vi "Lab Panel V4.3.vi"() -> ()   [LabVIEW 2013]
uses:
  <vilib>/Platform/TimedLoop/XDataNode/timing_clust.ctl
  <vilib>/Platform/TimedLoop/XDataNode/nitl_modes.ctl
  <vilib>/Platform/TimedLoop/XDataNode/wakeup.ctl
  Global 1.vi
  <vilib>/platform/TimedLoop/XDataNode/XDataNode.xnode
  <vilib>/Platform/TimedLoop/XDataNode/XDNodeRunTimeDep.lvlib
panel:
  out "TEMP update":bool
  out "AI update":bool
  in  "stop":bool
  in  "Tab Control 2":T1(tab)
  out "SIG LAB05-2":T2 {"PF" format="%.2f"; "AMPS" format="%.1f"}
  out "SIG LAB05-1":T2 {"PF" format="%.2f"; "AMPS" format="%.1f"}
  out "SIG LAB04-2":T2 {"PF" format="%.2f"; "AMPS" format="%.1f"}
  out "SIG LAB04-1":T2 {"PF" format="%.2f"; "AMPS" format="%.1f"}
  out "SIG LAB03-2":T2 {"PF" format="%.2f"; "AMPS" format="%.1f"}
  out "SIG LAB03-1":T2 {"PF" format="%.2f"; "AMPS" format="%.1f"}
  out "SIG LAB02-2":T2 {"PF" format="%.2f"; "AMPS" format="%.1f"}
  in  "RUN LAB01-1":bool
  in  "O/I  LAB05-1":bool
  in  "O/I  LAB05-2":bool
  in  "O/I  LAB04-1":bool
  in  "O/I  LAB04-2":bool
  in  "O/I  LAB02-1":bool
  in  "O/I  LAB02-2":bool
  in  "O/I  LAB01-2":bool
  in  "O/I  LAB01-1":bool
  in  "O/I  LAB03-1":bool
  in  "RUN LAB05-2":bool
  in  "RUN LAB05-1":bool
  in  "RUN LAB04-2":bool
  in  "RUN LAB04-1":bool
  in  "RUN LAB03-2":bool
  in  "RUN LAB03-1":bool
  in  "RUN LAB02-2":bool
  in  "RUN LAB02-1":bool
  in  "RUN LAB01-2":bool
  in  "SELECT LAB05-2":T3(radio)
  in  "SELECT LAB05-1":T3(radio)
  in  "SELECT LAB04-2":T3(radio)
  in  "SELECT LAB04-1":T3(radio)
  in  "SELECT LAB03-2":T3(radio)
  in  "SELECT LAB03-1":T3(radio)
  in  "SELECT LAB02-2":T3(radio)
  in  "SELECT LAB02-1":T3(radio)
  in  "SELECT LAB01-2":T3(radio)
  in  "SELECT LAB01-1":T3(radio)
  in  "O/I  LAB03-2":bool
  out "SIG LAB01-1":T2 {"PF" format="%.2f"; "AMPS" format="%.1f"}
  out "SIG LAB01-2":T2 {"PF" format="%.2f"; "AMPS" format="%.1f"}
  out "SIG LAB02-1":T2 {"PF" format="%.2f"; "AMPS" format="%.1f"}
  out "DISP LAB05-2":T4 {"MINS" format="%.2g"}
  out "DISP LAB05-1":T4 {"MINS" format="%.2g"}
  out "DISP LAB04-2":T4 {"MINS" format="%.2g"}
  out "DISP LAB04-1":T4 {"MINS" format="%.2g"}
  out "DISP LAB03-2":T4 {"MINS" format="%.2g"}
  out "DISP LAB03-1":T4 {"MINS" format="%.2g"}
  in  "SET LAB05-2":T5={"NAME"="", "DESCRIPTION"="", "CYCLES"=5.0, "T-RISE mins"=0.0, "T-RISE deg C"=0.0} {"CYCLES" min=5.0 step=1.0}
  in  "SET LAB05-1":T5={"NAME"="", "DESCRIPTION"="", "CYCLES"=5.0, "T-RISE mins"=0.0, "T-RISE deg C"=0.0} {"CYCLES" min=5.0 step=1.0}
  in  "SET LAB04-2":T5={"NAME"="", "DESCRIPTION"="", "CYCLES"=5.0, "T-RISE mins"=0.0, "T-RISE deg C"=0.0} {"CYCLES" min=5.0 step=1.0}
  in  "SET LAB04-1":T5={"NAME"="", "DESCRIPTION"="", "CYCLES"=5.0, "T-RISE mins"=0.0, "T-RISE deg C"=0.0} {"CYCLES" min=5.0 step=1.0}
  in  "SET LAB03-2":T5={"NAME"="", "DESCRIPTION"="", "CYCLES"=5.0, "T-RISE mins"=0.0, "T-RISE deg C"=0.0} {"CYCLES" min=5.0 step=1.0}
  in  "SET LAB03-1":T5={"NAME"="", "DESCRIPTION"="", "CYCLES"=5.0, "T-RISE mins"=0.0, "T-RISE deg C"=0.0} {"CYCLES" min=5.0 step=1.0}
  out "DISP LAB02-2":T4 {"MINS" format="%.2g"}
  out "DISP LAB02-1":T4 {"MINS" format="%.2g"}
  in  "SET LAB02-2":T5={"NAME"="", "DESCRIPTION"="", "CYCLES"=5.0, "T-RISE mins"=0.0, "T-RISE deg C"=0.0} {"CYCLES" min=5.0 step=1.0}
  in  "SET LAB02-1":T5={"NAME"="", "DESCRIPTION"="", "CYCLES"=5.0, "T-RISE mins"=0.0, "T-RISE deg C"=0.0} {"CYCLES" min=5.0 step=1.0}
  out "RESULT LAB05-2":bool
  out "RESULT LAB05-1":bool
  out "RESULT LAB04-2":bool
  out "RESULT LAB04-1":bool
  out "RESULT LAB03-2":bool
  out "RESULT LAB03-1":bool
  out "RESULT LAB02-2":bool
  out "RESULT LAB02-1":bool
  out "RESULT LAB01-2":bool
  out "RESULT LAB01-1":bool
  in  "SET LAB01-1":T5={"NAME"="", "DESCRIPTION"="", "CYCLES"=5.0, "T-RISE mins"=0.0, "T-RISE deg C"=0.0} {"CYCLES" min=5.0 step=1.0}
  in  "SET LAB01-2":T5={"NAME"="", "DESCRIPTION"="", "CYCLES"=5.0, "T-RISE mins"=0.0, "T-RISE deg C"=0.0} {"CYCLES" min=5.0 step=1.0}
  out "DISP LAB01-1":T4 {"MINS" format="%.2g"}
  out "DISP LAB01-2":T4 {"MINS" format="%.2f"}
  out "TEMP RISE LAB05-2":cluster{"TL":dbl, "TN":dbl}
  out "TEMP RISE LAB05-1":cluster{"TL":dbl, "TN":dbl}
  out "TEMP RISE LAB04-2":cluster{"TL":dbl, "TN":dbl}
  out "TEMP RISE LAB04-1":cluster{"TL":dbl, "TN":dbl}
  out "TEMP RISE LAB03-2":cluster{"TL":dbl, "TN":dbl}
  out "TEMP RISE LAB03-1":cluster{"TL":dbl, "TN":dbl}
  out "TEMP RISE LAB02-2":cluster{"TL":dbl, "TN":dbl}
  out "TEMP RISE LAB02-1":cluster{"TL":dbl, "TN":dbl}
  out "TEMP RISE LAB01-2":cluster{"TL":dbl, "TN":dbl}
  out "TEMP RISE LAB01-1":cluster{"TL":dbl, "TN":dbl}
  in  "JIG OFF TIME (S)":dbl=2.0 min=2.0 max=10.0 step=0.5 format="%.1g"
  in  "JIG ON TIME (S)":dbl=1.0 min=1.0 max=10.0 step=0.5 format="%.1g"
  out "JIG LAB05-2":bool
  out "JIG LAB05-1":bool
  out "JIG LAB04-2":bool
  out "JIG LAB04-1":bool
  out "JIG LAB03-2":bool
  out "JIG LAB03-1":bool
  out "JIG LAB02-2":bool
  out "JIG LAB02-1":bool
  out "JIG LAB01-2":bool
  out "JIG LAB01-1":bool
  out "TEMP START LAB01-1":cluster{"TL":dbl, "TN":dbl}
  out "TEMP START LAB02-1":cluster{"TL":dbl, "TN":dbl}
  out "TEMP START LAB03-1":cluster{"TL":dbl, "TN":dbl}
  out "TEMP START LAB04-1":cluster{"TL":dbl, "TN":dbl}
  out "TEMP START LAB01-2":cluster{"TL":dbl, "TN":dbl}
  out "TEMP START LAB02-2":cluster{"TL":dbl, "TN":dbl}
  out "TEMP START LAB03-2":cluster{"TL":dbl, "TN":dbl}
  out "TEMP START LAB04-2":cluster{"TL":dbl, "TN":dbl}
  out "TEMP START LAB05-2":cluster{"TL":dbl, "TN":dbl}
  out "TEMP START LAB05-1":cluster{"TL":dbl, "TN":dbl}
  in  "MAIL SETTINGS":T6
  out "MAIL REPORT":string
  in  "TO (string):":string
  in  "Send Mail Now":bool
  in  "Auto Mail Send":bool
  in  "Network Directory":path
  out "CAL LAB01":T7 {"2 (TN) cal" min=0.0 step=0.01 format="%.2f"; "2 (TL) cal" min=0.0 step=0.01 format="%.2f"; "2 (PF) cal" min=0.0 step=0.01 format="%.2f"; "2 (V) cal" min=0.0 step=0.01 format="%.2f"; "2 (A) cal" min=0.0 step=0.01 format="%.2f"; "1 (TN) cal" min=0.0 step=0.01 format="%.2f"; "1 (TL) cal" min=0.0 step=0.01 format="%.2f"; "1 (PF) cal" min=0.0 step=0.01 format="%.2f"; "1 (V) cal" min=0.0 step=0.01 format="%.2f"; "1  (A) cal" min=0.0 step=0.01 format="%.2f"}
  out "CAL LAB03":T7 {"2 (TN) cal" min=0.0 step=0.01 format="%.2f"; "2 (TL) cal" min=0.0 step=0.01 format="%.2f"; "2 (PF) cal" min=0.0 step=0.01 format="%.2f"; "2 (V) cal" min=0.0 step=0.01 format="%.2f"; "2 (A) cal" min=0.0 step=0.01 format="%.2f"; "1 (TN) cal" min=0.0 step=0.01 format="%.2f"; "1 (TL) cal" min=0.0 step=0.01 format="%.2f"; "1 (PF) cal" min=0.0 step=0.01 format="%.2f"; "1 (V) cal" min=0.0 step=0.01 format="%.2f"; "1  (A) cal" min=0.0 step=0.01 format="%.2f"}
  out "CAL LAB02":T8 {"2 (TN) cal" min=0.0 step=0.01 format="%.2f"; "2 (TL) cal" min=0.0 step=0.01 format="%.2f"; "2 (PF) cal" min=0.0 step=0.01 format="%.2f"; "2 (V) cal" min=0.0 step=0.01 format="%.2f"; "2 (A) cal" min=0.0 step=0.01 format="%.2f"; "1 (TN) cal" min=0.0 step=0.01 format="%.2f"; "1 (TL) cal" min=0.0 step=0.01 format="%.2f"; "1 (PF) cal" min=0.0 step=0.01 format="%.2f"; "1 (V) cal" min=0.0 step=0.01 format="%.2f"; "1 (A) cal" min=0.0 step=0.01 format="%.2f"}
  out "CAL LAB05":T7 {"2 (TN) cal" min=0.0 step=0.01 format="%.2f"; "2 (TL) cal" min=0.0 step=0.01 format="%.2f"; "2 (PF) cal" min=0.0 step=0.01 format="%.2f"; "2 (V) cal" min=0.0 step=0.01 format="%.2f"; "2 (A) cal" min=0.0 step=0.01 format="%.2f"; "1 (TN) cal" min=0.0 step=0.01 format="%.2f"; "1 (TL) cal" min=0.0 step=0.01 format="%.2f"; "1 (PF) cal" min=0.0 step=0.01 format="%.2f"; "1 (V) cal" min=0.0 step=0.01 format="%.2f"; "1  (A) cal" min=0.0 step=0.01 format="%.2f"}
  out "CAL LAB04":T7 {"2 (TN) cal" min=0.0 step=0.01 format="%.2f"; "2 (TL) cal" min=0.0 step=0.01 format="%.2f"; "2 (PF) cal" min=0.0 step=0.01 format="%.2f"; "2 (V) cal" min=0.0 step=0.01 format="%.2f"; "2 (A) cal" min=0.0 step=0.01 format="%.2f"; "1 (TN) cal" min=0.0 step=0.01 format="%.2f"; "1 (TL) cal" min=0.0 step=0.01 format="%.2f"; "1 (PF) cal" min=0.0 step=0.01 format="%.2f"; "1 (V) cal" min=0.0 step=0.01 format="%.2f"; "1  (A) cal" min=0.0 step=0.01 format="%.2f"}
  out "calibration file error out":errorcluster
  in  "CALIBRATE":bool
  in  "SHOW ADMIN PAGE":bool
  out "ON L05-2":cluster{"amps":dbl, "volts":dbl, "pf":dbl}
  out "ON L05-1":cluster{"amps":dbl, "volts":dbl, "pf":dbl}
  out "FAIL LAB05-2":cluster{"LO":dbl, "HI":dbl}
  out "FAIL LAB05-1":cluster{"LO":dbl, "HI":dbl}
  out "FAIL LAB04-2":cluster{"LO":dbl, "HI":dbl}
  out "FAIL LAB04-1":cluster{"LO":dbl, "HI":dbl}
  out "FAIL LAB03-2":cluster{"LO":dbl, "HI":dbl}
  out "FAIL LAB03-1":cluster{"LO":dbl, "HI":dbl}
  out "FAIL LAB02-2":cluster{"LO":dbl, "HI":dbl}
  out "FAIL LAB02-1":cluster{"LO":dbl, "HI":dbl}
  out "FAIL LAB01-2":cluster{"LO":dbl, "HI":dbl}
  out "FAIL LAB01-1":cluster{"LO":dbl, "HI":dbl}
  out "ON L01-1":cluster{"amps":dbl, "volts":dbl, "pf":dbl}
  out "ON L01-2":cluster{"amps":dbl, "volts":dbl, "pf":dbl}
  out "ON L02-1":cluster{"amps":dbl, "volts":dbl, "pf":dbl}
  out "ON L02-2":cluster{"amps":dbl, "volts":dbl, "pf":dbl}
  out "ON L03-1":cluster{"amps":dbl, "volts":dbl, "pf":dbl}
  out "ON L03-2":cluster{"amps":dbl, "volts":dbl, "pf":dbl}
  out "ON L04-1":cluster{"amps":dbl, "volts":dbl, "pf":dbl}
  out "ON L04-2":cluster{"amps":dbl, "volts":dbl, "pf":dbl}
  in  "JIG TEST":T9
  in  "C drive data root dir":path
  out "run lab05-2":bool
  out "run lab05-1":bool
  out "run lab04-2":bool
  out "run lab04-1":bool
  out "run lab03-2":bool
  out "run lab03-1":bool
  out "run lab02-2":bool
  out "run lab02-1":bool
  out "run lab01-2":bool
  out "run lab01-1":bool
  out "stop2":bool
  in  "Tab Control":T10(tab)
  out "LAB01-2 (GRAPH)":dynamicdata(graph)
  out "LAB01-1 (GRAPH)":dynamicdata(graph)
  out "LAB02-2 (GRAPH)":dynamicdata(graph)
  out "LAB02-1 (GRAPH)":dynamicdata(graph)
  out "LAB03-2 (GRAPH)":dynamicdata(graph)
  out "LAB03-1 (GRAPH)":dynamicdata(graph)
  out "LAB04-2 (GRAPH)":dynamicdata(graph)
  out "LAB04-1 (GRAPH)":dynamicdata(graph)
  out "LAB05-2 (GRAPH)":dynamicdata(graph)
  out "LAB05-1 (GRAPH)":dynamicdata(graph)
  out "LAB05 TEMP":T11
  out "LAB04 TEMP":T11
  out "LAB02 TEMP":T11
  out "LAB01 TEMP":T11
  out "LAB03 TEMP":T11
  out "Analog Error Array":errorcluster[](array[cluster])
  out "AI loop time":dbl format="%.6g"
  out "loops":dbl
  in  "loop  delay(mS)":dbl
  out "on loops":dbl
  out "off loops":dbl
  out "jig cycle":dbl
  out "TDMS LAB01-1":refnum<k34>
  out "data file error":errorcluster
  out "TDMS LAB02-1":refnum<k34>
  out "TDMS LAB01-2":refnum<k34>
  out "TDMS LAB02-2":refnum<k34>
  out "TDMS LAB03-1":refnum<k34>
  out "TDMS LAB03-2":refnum<k34>
  out "TDMS LAB04-1":refnum<k34>
  out "TDMS LAB04-2":refnum<k34>
  out "TDMS LAB05-1":refnum<k34>
  out "TDMS LAB05-2":refnum<k34>
  out "mail control":string
  # "LAB01"
  # "LAB02"
  # "LAB05"
  # "LAB03"
  # "LAB04"
  # "LAB01"
  # "LAB02"
  # "LAB03"
  # "LAB04"
  # "LAB05"
  # "JIG SET"
  # "(Enter recipients address seperated by comma)"
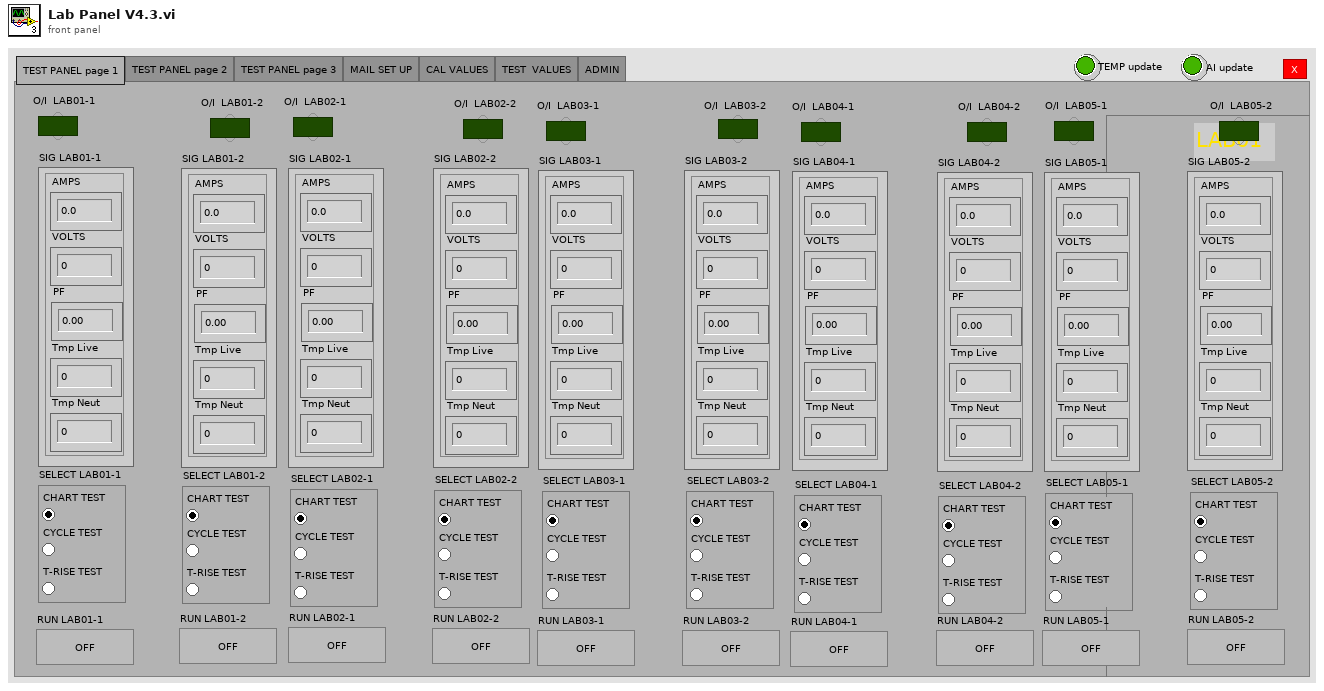
[diagram p1: front panel]
types:
  T1 = enum32{"TEST PANEL page 1", "TEST PANEL page 2", "TEST PANEL page 3", "MAIL SET UP", "CAL VALUES", "TEST  VALUES", "ADMIN"}
  T2 = cluster{"AMPS":dbl, "VOLTS":dbl, "PF":dbl, "Tmp Live":dbl, "Tmp Neut":dbl}
  T3 = enum32{"CHART TEST", "CYCLE TEST", "T-RISE TEST"}
  T4 = cluster{"CYCLE":dbl, "MINS":dbl, "STATUS":string}
  T5 = cluster{"NAME":string, "DESCRIPTION":string, "CYCLES":dbl, "T-RISE mins":dbl, "T-RISE deg C":dbl}
  T6 = cluster{"OUT SERVER ADDRESS":string, "FROM ACCOUNT":string, "USER NAME":string, "PASSWORD":string, "TEST MAIL":bool, "TEST MAIL STATUS":string, "mail error":errorcluster}
  T7 = cluster{"1  (A) cal":dbl, "1 (V) cal":dbl, "1 (PF) cal":dbl, "1 (TL) cal":dbl, "1 (TN) cal":dbl, "2 (A) cal":dbl, "2 (V) cal":dbl, "2 (PF) cal":dbl, "2 (TL) cal":dbl, "2 (TN) cal":dbl}
  T8 = cluster{"1 (A) cal":dbl, "1 (V) cal":dbl, "1 (PF) cal":dbl, "1 (TL) cal":dbl, "1 (TN) cal":dbl, "2 (A) cal":dbl, "2 (V) cal":dbl, "2 (PF) cal":dbl, "2 (TL) cal":dbl, "2 (TN) cal":dbl}
  T9 = cluster{" LAB01-1":bool, " LAB01-2":bool, "LAB02-1":bool, " LAB02-2":bool, "LAB03-1":bool, "LAB03-2":bool, "LAB04-1":bool, "LAB04-2":bool, "LAB05-1":bool, "LAB05-2":bool}
  T10 = enum32{"LAB01", "LAB02", "LAB03", "LAB04", "LAB05", "TEMPERATURE", "ERROR"}
  T11 = cluster{"T1 Live":dbl, "T1 Neut":dbl, "T2 Live":dbl, "T2 Neut":dbl, "ID":dbl, "ER":dbl}
  T12 = enum8{"Enabled", "Disabled", "Disabled and Grayed Out"}
  T13 = typedef "XDNodeRunTimeDep.lvlib/timing_clust.ctl" = cluster{"Expected End [f-1]":u64, "Actual End [f-1]":u64, "Finished Late? [f-1]":bool, "Expected End [i-1]":u64, "Actual End [i-1]":u64, "Finished Late? [i-1]":bool, "Expected Start [i]":u64, "Actual Start [i]":u64, "Expected Start [f]":u64, "Actual Start [f]":u64, "Source Name":string, "Structure Name":string, "Period":i64, "Deadline":i64, "Offset":i64, "Start":i64, "Priority":i32, "Timeout":i32, "Mode":T14, "Wakeup Reason":T15, "Error":errorcluster, "Source Type":string, "Secondary Source Type":string, "Global End Time":u64, "Global Start Time":u64, "Frame Duration":u64, "Iteration Duration":u64, "Assigned CPU":i32, "I/O Scan Engine Mode":u32}
  T14 = typedef "XDNodeRunTimeDep.lvlib/nitl_modes.ctl" = enum32{"No Change", "Process missed periods, maintain original phase", "Discard missed periods, maintain original phase", "Process missed periods, ignore original phase", "Discard missed periods, ignore original phase"}
  T15 = typedef "XDNodeRunTimeDep.lvlib/wakeup.ctl" = enum32{"Normal", "Aborted", "Asynchronous wakeup", "Timing source error", "Timed loop error", "Timeout"}
  T16 = enum16{"open", "open or create", "create or replace", "create", "open (read-only)"}
  T17 = enum16{"open", "replace", "create", "open or create", "replace or create", "replace or create with confirmation"}
  T18 = cluster{"SET LAB01-1":cluster{"NAME":string, "DESCRIPTION":string, "CYCLES":dbl, "T-RISE mins":dbl, "T-RISE deg C":dbl}, "SET LAB01-2":cluster{"NAME":string, "DESCRIPTION":string, "CYCLES":dbl, "T-RISE mins":dbl, "T-RISE deg C":dbl}, "SET LAB02-1":cluster{"NAME":string, "DESCRIPTION":string, "CYCLES":dbl, "T-RISE mins":dbl, "T-RISE deg C":dbl}, "SET LAB02-2":cluster{"NAME":string, "DESCRIPTION":string, "CYCLES":dbl, "T-RISE mins":dbl, "T-RISE deg C":dbl}, "SET LAB03-1":cluster{"NAME":string, "DESCRIPTION":string, "CYCLES":dbl, "T-RISE mins":dbl, "T-RISE deg C":dbl}, "SET LAB03-2":cluster{"NAME":string, "DESCRIPTION":string, "CYCLES":dbl, "T-RISE mins":dbl, "T-RISE deg C":dbl}, "SET LAB04-1":cluster{"NAME":string, "DESCRIPTION":string, "CYCLES":dbl, "T-RISE mins":dbl, "T-RISE deg C":dbl}, "SET LAB04-2":cluster{"NAME":string, "DESCRIPTION":string, "CYCLES":dbl, "T-RISE mins":dbl, "T-RISE deg C":dbl}, "SET LAB05-1":cluster{"NAME":string, "DESCRIPTION":string, "CYCLES":dbl, "T-RISE mins":dbl, "T-RISE deg C":dbl}, "SET LAB05-2":cluster{"NAME":string, "DESCRIPTION":string, "CYCLES":dbl, "T-RISE mins":dbl, "T-RISE deg C":dbl}, "Network Directory":path, "C drive data root dir":path}
  T19 = cluster{"MAIL SETTINGS":cluster{"OUT SERVER ADDRESS":string, "FROM ACCOUNT":string, "USER NAME":string, "PASSWORD":string, "TEST MAIL":bool, "TEST MAIL STATUS":string, "mail error":errorcluster}, "Auto Mail Send":bool, string}
  T20 = cluster{"T1":dbl, "T2":dbl, "T3":dbl, "T4":dbl, "ID":dbl, "ER":dbl}
  T21 = cluster{"LAB01-1 (A)":dbl, "LAB01-1 (V)":dbl, "LAB01-1 (PF)":dbl, "LAB01-2 (A)":dbl, "LAB01-2 (V)":dbl, "LAB01-2 (PF)":dbl}
  T22 = cluster{"LAB02-1 (A)":dbl, "LAB02-1 (V)":dbl, "LAB02-1 (PF)":dbl, "LAB02-2 (A)":dbl, "LAB02-2 (V)":dbl, "LAB02-2 (PF)":dbl}
  T23 = cluster{"LAB03-1 (A)":dbl, "LAB03-1 (V)":dbl, "LAB03-1 (PF)":dbl, "LAB03-2 (A)":dbl, "LAB03-2 (V)":dbl, "LAB03-2 (PF)":dbl}
  T24 = cluster{"LAB04-1 (A)":dbl, "LAB04-1 (V)":dbl, "LAB04-1 (PF)":dbl, "LAB04-2 (A)":dbl, "LAB04-2 (V)":dbl, "LAB04-2 (PF)":dbl}
  T25 = cluster{"LAB05-1 (A)":dbl, "LAB05-1 (V)":dbl, "LAB05-1 (PF)":dbl, "LAB05-2 (A)":dbl, "LAB05-2 (V)":dbl, "LAB05-2 (PF)":dbl}
  T26 = cluster{"FAIL LAB01-1":cluster{"LO":dbl, "HI":dbl}, "SIG LAB01-1":cluster{"AMPS":dbl, "VOLTS":dbl, "PF":dbl, "Tmp Live":dbl, "Tmp Neut":dbl}, "TEMP START LAB01-1":cluster{"TL":dbl, "TN":dbl}, "DISP LAB01-1":cluster{"CYCLE":dbl, "MINS":dbl, "STATUS":string}, "SET LAB01-1":cluster{"NAME":string, "DESCRIPTION":string, "CYCLES":dbl, "T-RISE mins":dbl, "T-RISE deg C":dbl}, "TDMS LAB01-1":refnum<k34>}
  T27 = cluster{"FAIL LAB01-2":cluster{"LO":dbl, "HI":dbl}, "SIG LAB01-2":cluster{"AMPS":dbl, "VOLTS":dbl, "PF":dbl, "Tmp Live":dbl, "Tmp Neut":dbl}, "TEMP START LAB01-2":cluster{"TL":dbl, "TN":dbl}, "DISP LAB01-2":cluster{"CYCLE":dbl, "MINS":dbl, "STATUS":string}, "SET LAB01-2":cluster{"NAME":string, "DESCRIPTION":string, "CYCLES":dbl, "T-RISE mins":dbl, "T-RISE deg C":dbl}, "TDMS LAB01-2":refnum<k34>}
  T28 = cluster{"FAIL LAB02-1":cluster{"LO":dbl, "HI":dbl}, "SIG LAB02-1":cluster{"AMPS":dbl, "VOLTS":dbl, "PF":dbl, "Tmp Live":dbl, "Tmp Neut":dbl}, "TEMP START LAB02-1":cluster{"TL":dbl, "TN":dbl}, "DISP LAB02-1":cluster{"CYCLE":dbl, "MINS":dbl, "STATUS":string}, "SET LAB02-1":cluster{"NAME":string, "DESCRIPTION":string, "CYCLES":dbl, "T-RISE mins":dbl, "T-RISE deg C":dbl}, "TDMS LAB02-1":refnum<k34>}
  T29 = cluster{"FAIL LAB02-2":cluster{"LO":dbl, "HI":dbl}, "SIG LAB02-2":cluster{"AMPS":dbl, "VOLTS":dbl, "PF":dbl, "Tmp Live":dbl, "Tmp Neut":dbl}, "TEMP START LAB02-2":cluster{"TL":dbl, "TN":dbl}, "DISP LAB02-2":cluster{"CYCLE":dbl, "MINS":dbl, "STATUS":string}, "SET LAB02-2":cluster{"NAME":string, "DESCRIPTION":string, "CYCLES":dbl, "T-RISE mins":dbl, "T-RISE deg C":dbl}, "TDMS LAB02-2":refnum<k34>}
  T30 = cluster{"FAIL LAB03-1":cluster{"LO":dbl, "HI":dbl}, "SIG LAB03-1":cluster{"AMPS":dbl, "VOLTS":dbl, "PF":dbl, "Tmp Live":dbl, "Tmp Neut":dbl}, "TEMP START LAB03-1":cluster{"TL":dbl, "TN":dbl}, "DISP LAB03-1":cluster{"CYCLE":dbl, "MINS":dbl, "STATUS":string}, "SET LAB03-1":cluster{"NAME":string, "DESCRIPTION":string, "CYCLES":dbl, "T-RISE mins":dbl, "T-RISE deg C":dbl}, "TDMS LAB03-1":refnum<k34>}
  T31 = cluster{"FAIL LAB03-2":cluster{"LO":dbl, "HI":dbl}, "SIG LAB03-2":cluster{"AMPS":dbl, "VOLTS":dbl, "PF":dbl, "Tmp Live":dbl, "Tmp Neut":dbl}, "TEMP START LAB03-2":cluster{"TL":dbl, "TN":dbl}, "DISP LAB03-2":cluster{"CYCLE":dbl, "MINS":dbl, "STATUS":string}, "SET LAB03-2":cluster{"NAME":string, "DESCRIPTION":string, "CYCLES":dbl, "T-RISE mins":dbl, "T-RISE deg C":dbl}, "TDMS LAB03-2":refnum<k34>}
  T32 = cluster{"FAIL LAB04-1":cluster{"LO":dbl, "HI":dbl}, "SIG LAB04-1":cluster{"AMPS":dbl, "VOLTS":dbl, "PF":dbl, "Tmp Live":dbl, "Tmp Neut":dbl}, "TEMP START LAB04-1":cluster{"TL":dbl, "TN":dbl}, "DISP LAB04-1":cluster{"CYCLE":dbl, "MINS":dbl, "STATUS":string}, "SET LAB04-1":cluster{"NAME":string, "DESCRIPTION":string, "CYCLES":dbl, "T-RISE mins":dbl, "T-RISE deg C":dbl}, "TDMS LAB04-1":refnum<k34>}
  T33 = cluster{"FAIL LAB04-2":cluster{"LO":dbl, "HI":dbl}, "SIG LAB04-2":cluster{"AMPS":dbl, "VOLTS":dbl, "PF":dbl, "Tmp Live":dbl, "Tmp Neut":dbl}, "TEMP START LAB04-2":cluster{"TL":dbl, "TN":dbl}, "DISP LAB04-2":cluster{"CYCLE":dbl, "MINS":dbl, "STATUS":string}, "SET LAB04-2":cluster{"NAME":string, "DESCRIPTION":string, "CYCLES":dbl, "T-RISE mins":dbl, "T-RISE deg C":dbl}, "TDMS LAB04-2":refnum<k34>}
  T34 = cluster{"FAIL LAB05-1":cluster{"LO":dbl, "HI":dbl}, "SIG LAB05-1":cluster{"AMPS":dbl, "VOLTS":dbl, "PF":dbl, "Tmp Live":dbl, "Tmp Neut":dbl}, "TEMP START LAB05-1":cluster{"TL":dbl, "TN":dbl}, "DISP LAB05-1":cluster{"CYCLE":dbl, "MINS":dbl, "STATUS":string}, "SET LAB05-1":cluster{"NAME":string, "DESCRIPTION":string, "CYCLES":dbl, "T-RISE mins":dbl, "T-RISE deg C":dbl}, "TDMS LAB05-1":refnum<k34>}
  T35 = cluster{"FAIL LAB05-2":cluster{"LO":dbl, "HI":dbl}, "SIG LAB05-2":cluster{"AMPS":dbl, "VOLTS":dbl, "PF":dbl, "Tmp Live":dbl, "Tmp Neut":dbl}, "TEMP START LAB05-2":cluster{"TL":dbl, "TN":dbl}, "DISP LAB05-2":cluster{"CYCLE":dbl, "MINS":dbl, "STATUS":string}, "SET LAB05-2":cluster{"NAME":string, "DESCRIPTION":string, "CYCLES":dbl, "T-RISE mins":dbl, "T-RISE deg C":dbl}, "TDMS LAB05-2":refnum<k34>}
  T36 = cluster{"MAIL SETTINGS":cluster{"OUT SERVER ADDRESS":string, "FROM ACCOUNT":string, "USER NAME":string, "PASSWORD":string, "TEST MAIL":bool, "TEST MAIL STATUS":string, "mail error":errorcluster}, "Auto Mail Send":bool, "TO (string):":string}
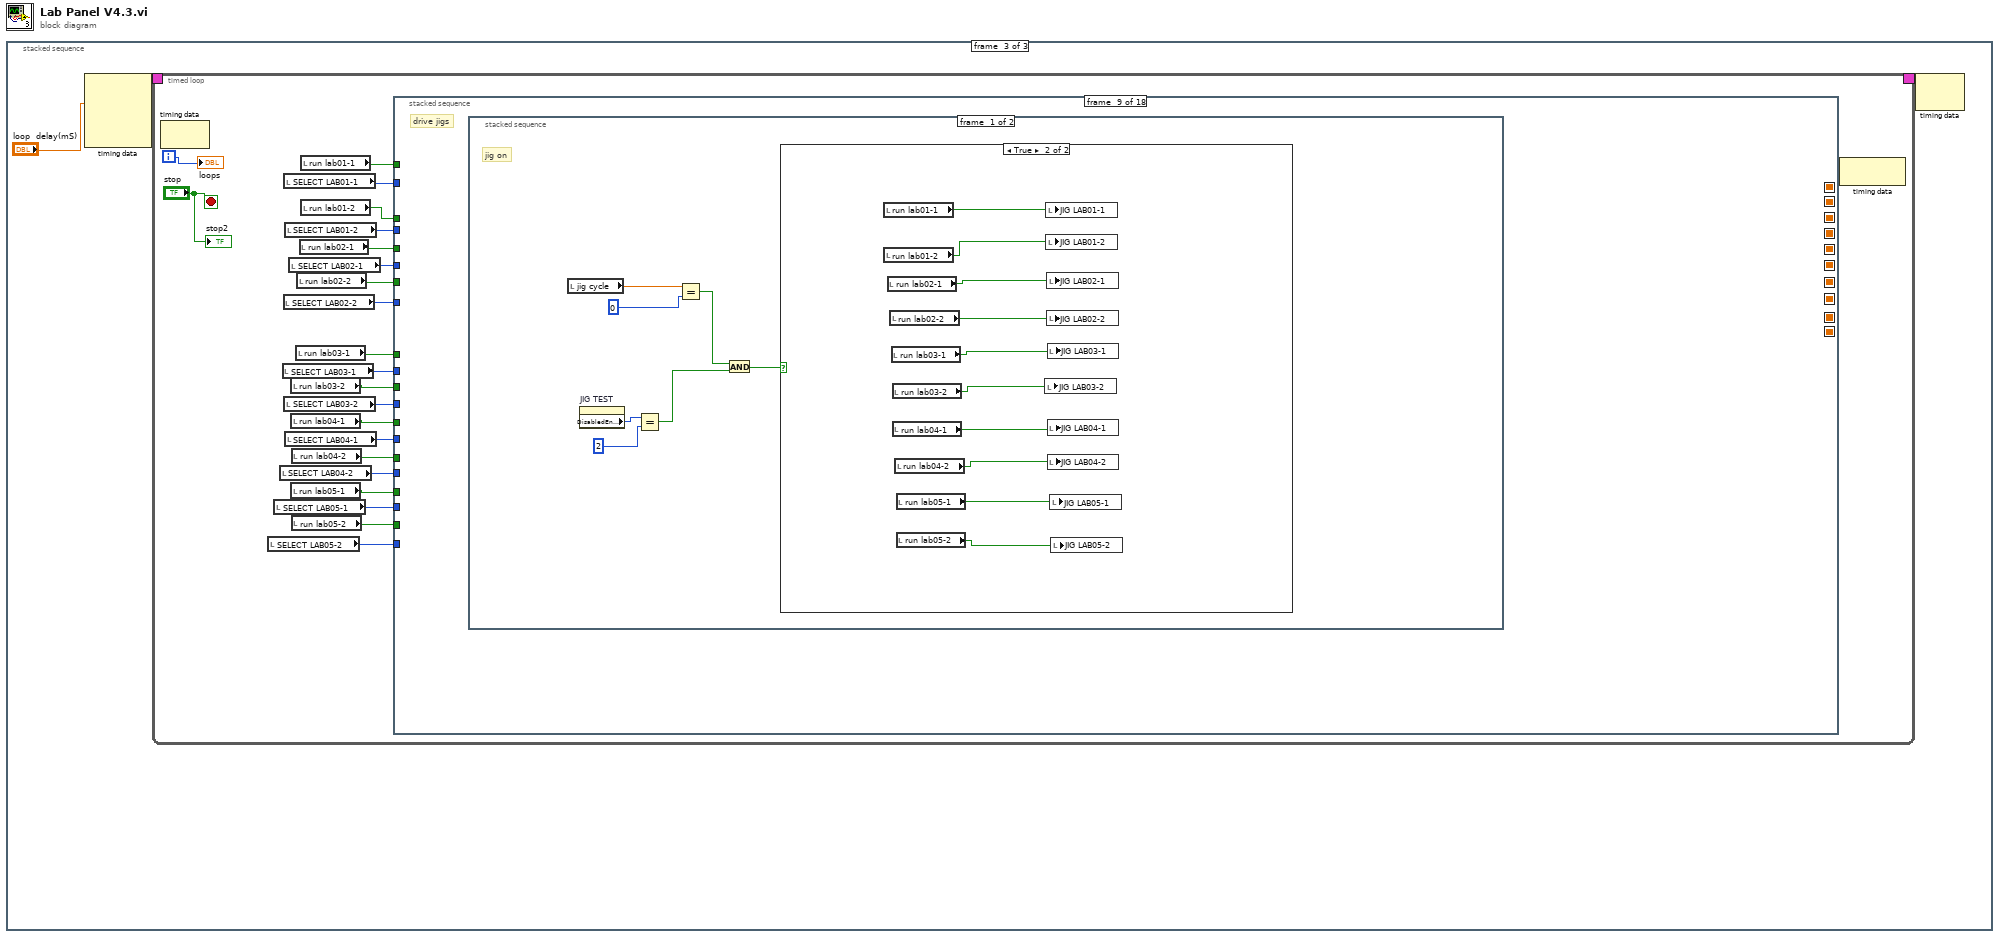
[diagram p0: block diagram]
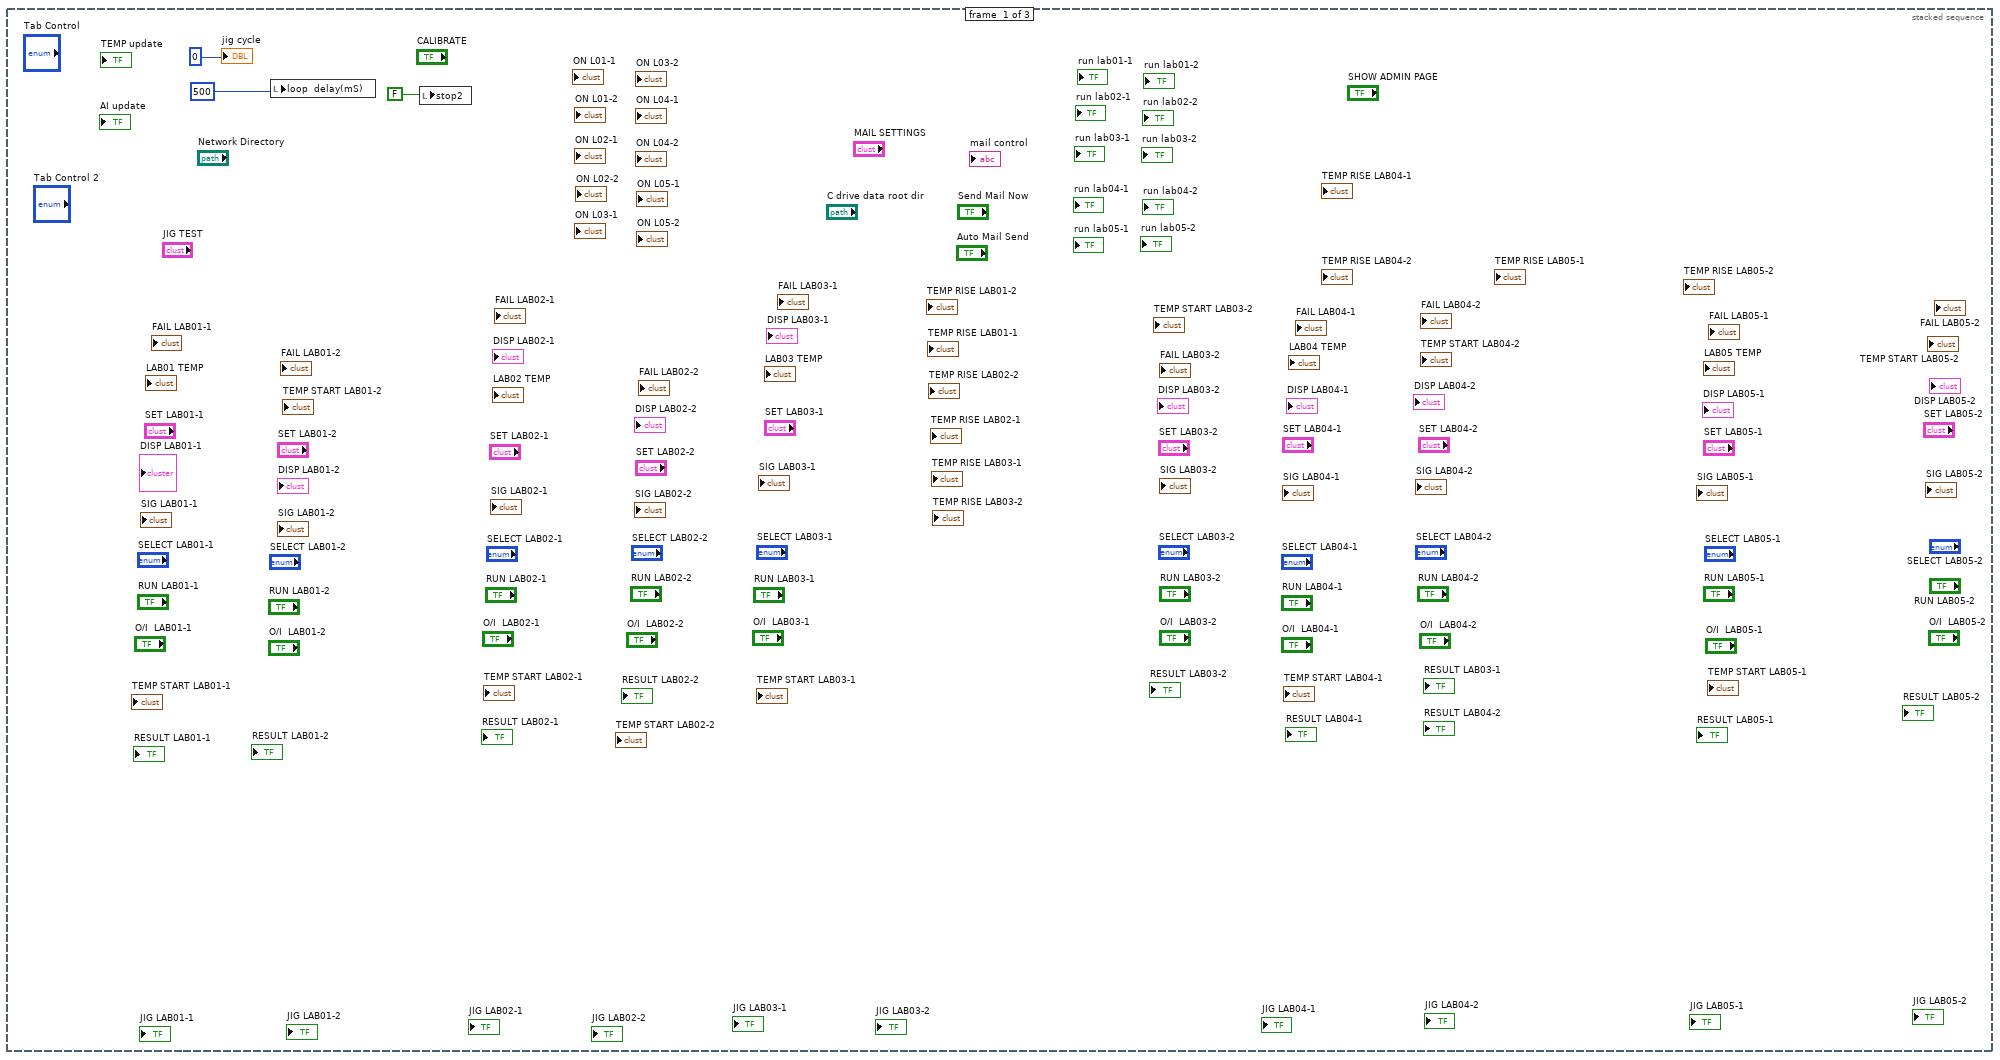
[diagram p2: hidden frame]
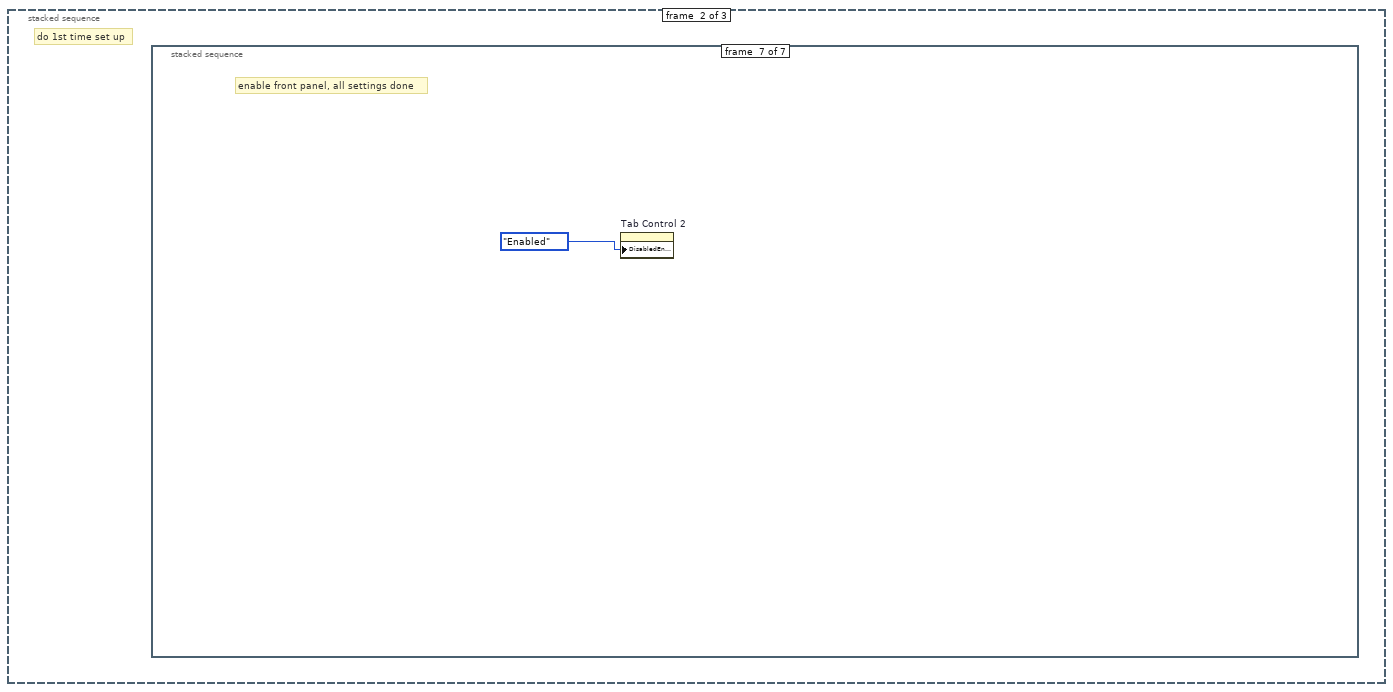
[diagram p3: hidden frame]
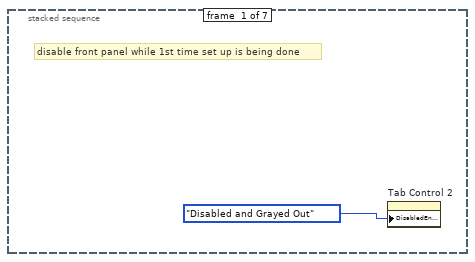
[diagram p4: hidden frame]
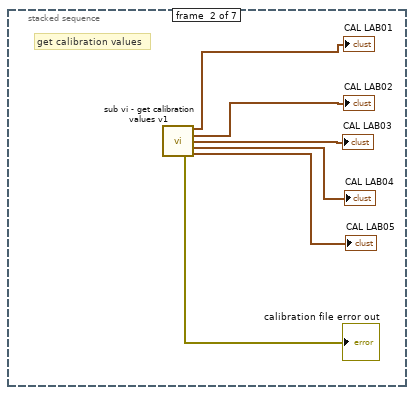
[diagram p5: hidden frame]
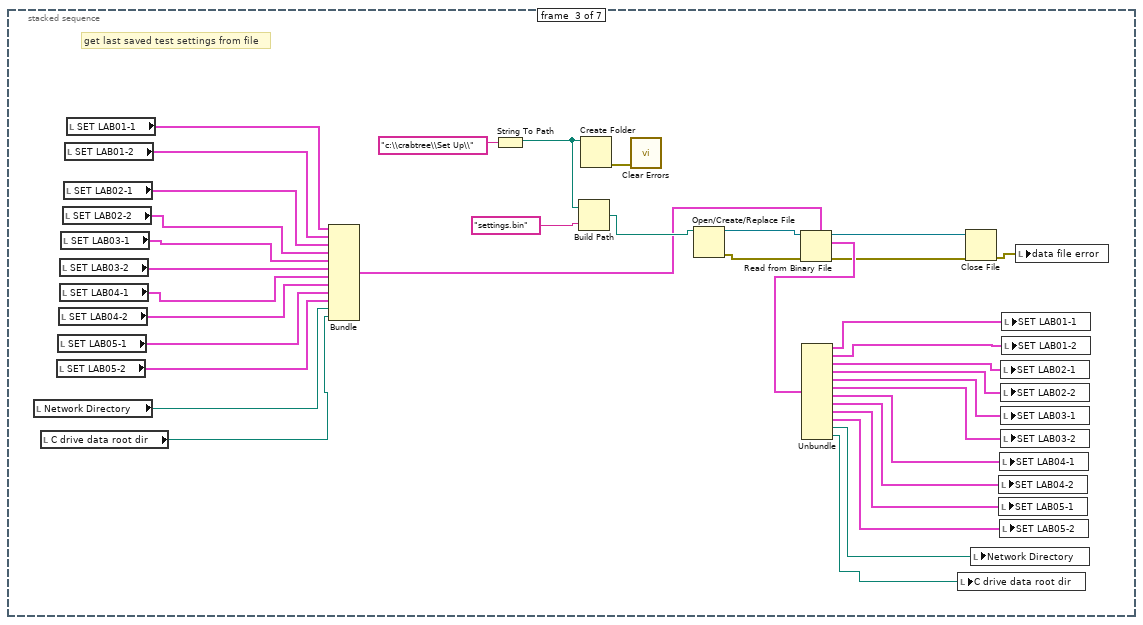
[diagram p6: hidden frame]
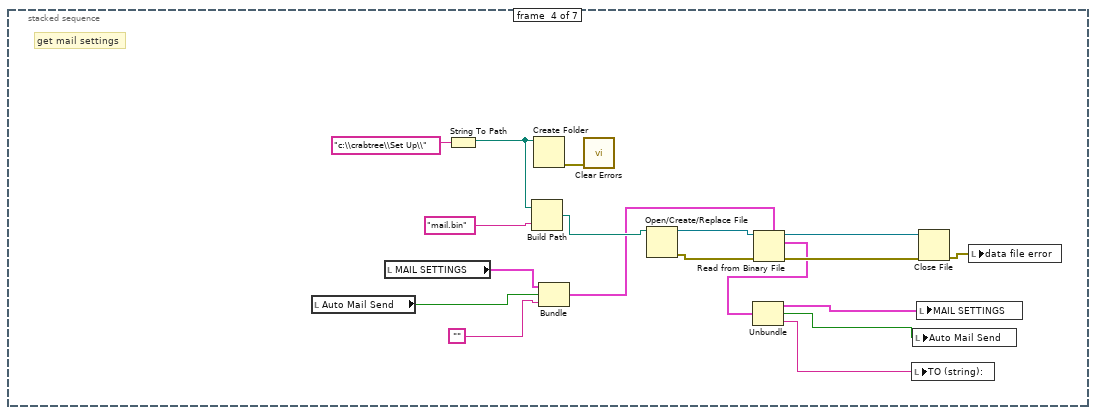
[diagram p7: hidden frame]
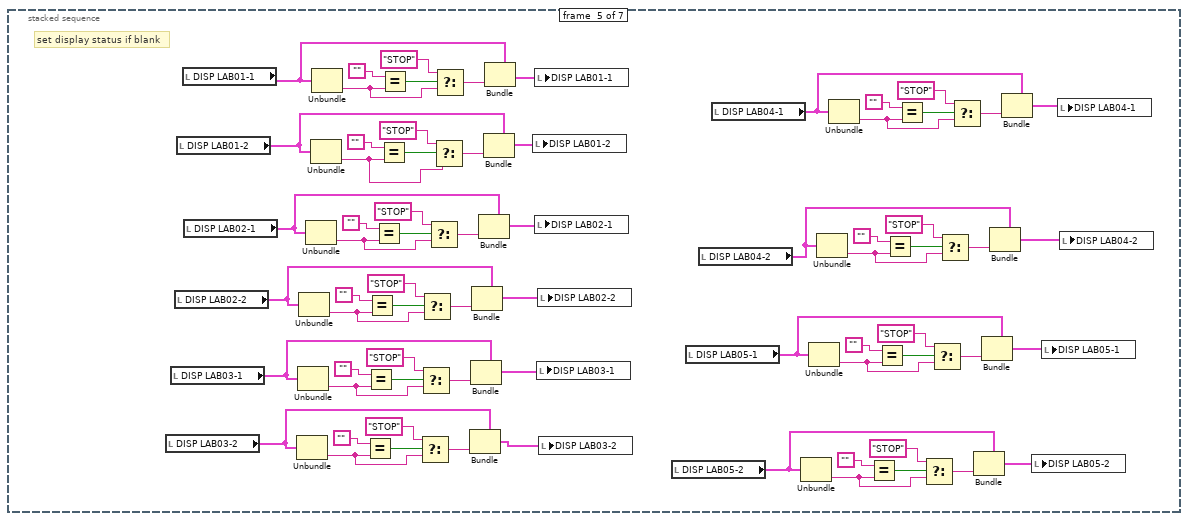
[diagram p8: hidden frame]
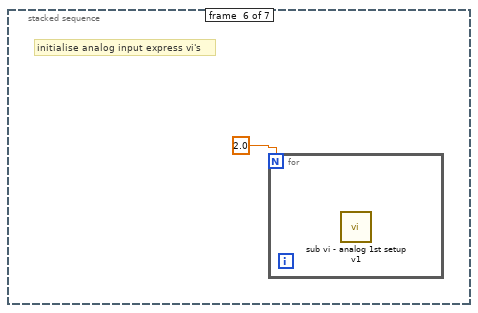
[diagram p9: hidden frame]
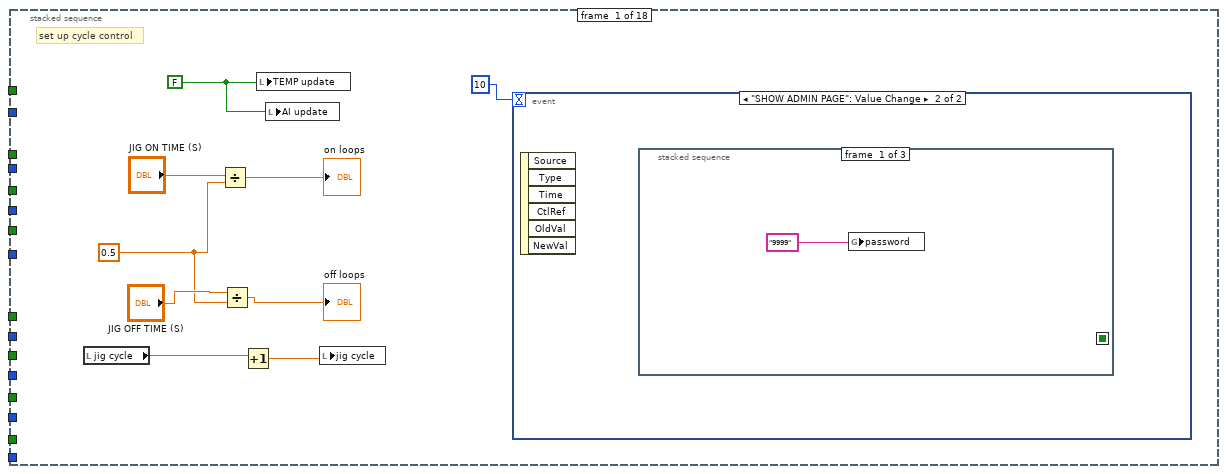
[diagram p10: hidden frame]
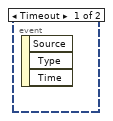
[diagram p11: hidden frame]
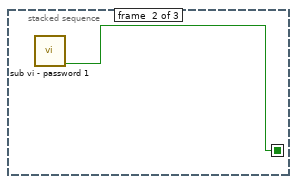
[diagram p12: hidden frame]
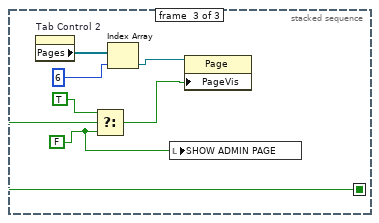
[diagram p13: hidden frame]
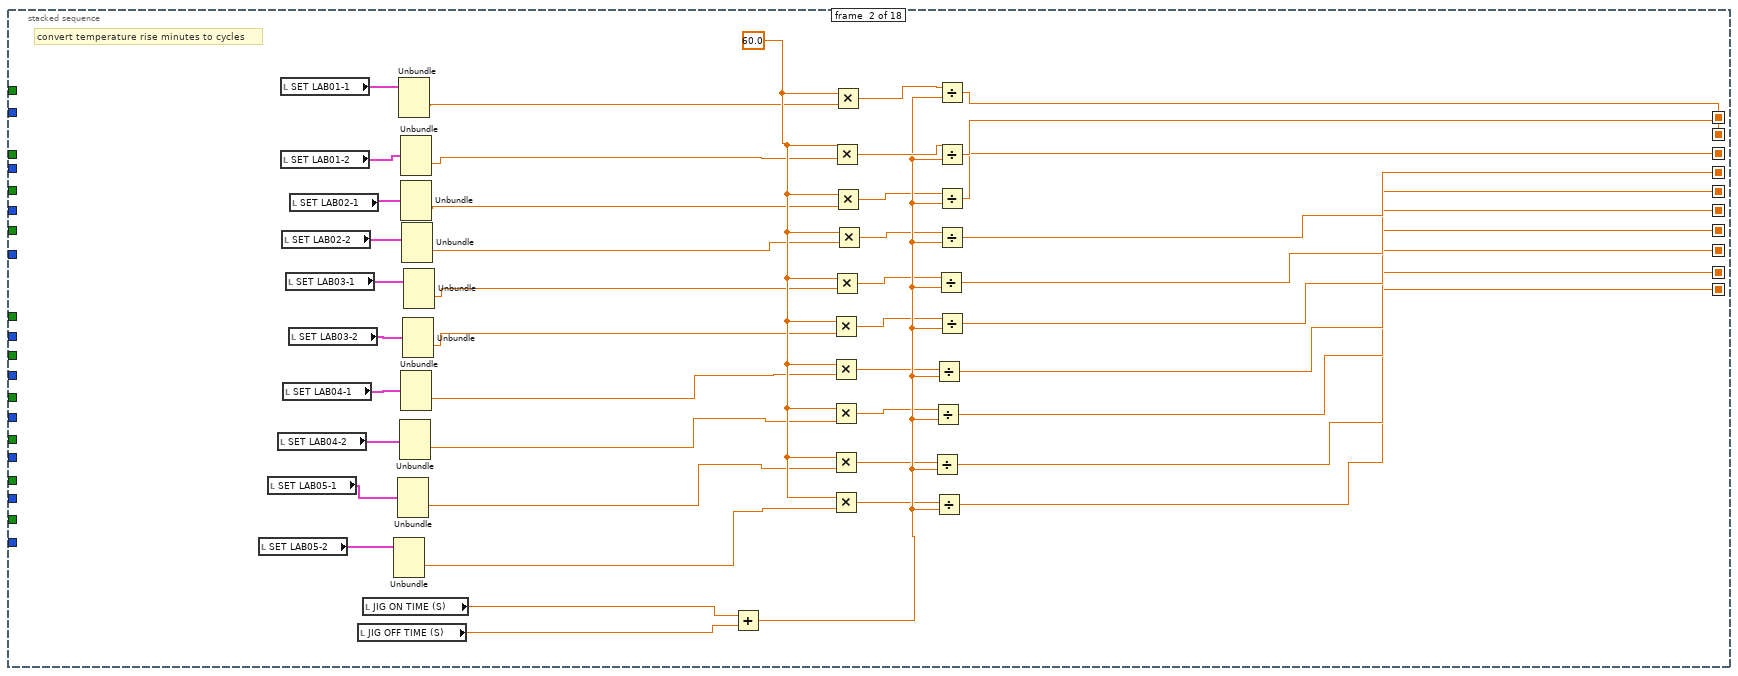
[diagram p14: hidden frame]
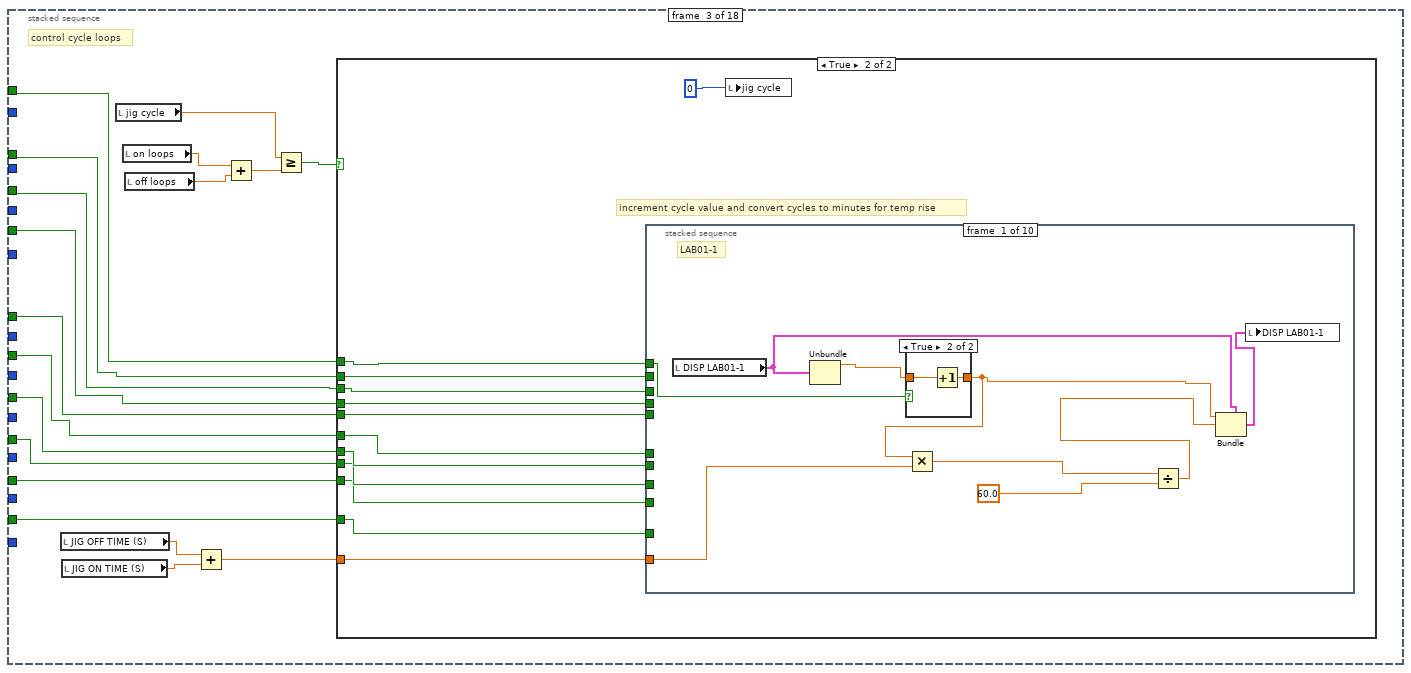
[diagram p15: hidden frame]
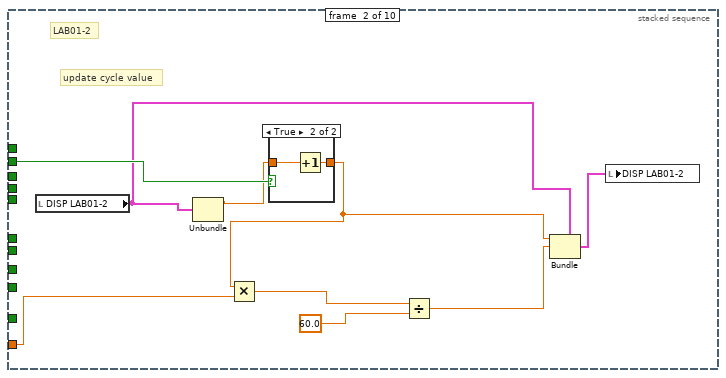
[diagram p18: hidden frame]
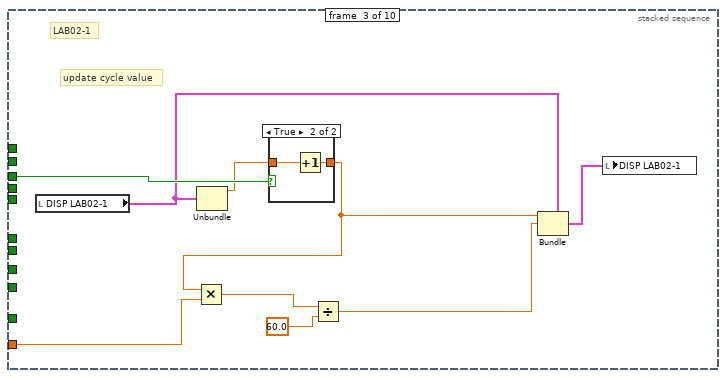
[diagram p20: hidden frame]
diagram:
  n1 = stacked-sequence {
    frame #0 {
      n2 = local write "loop  delay(mS)"(500) -> ()
      n3 = local write "stop2"(FALSE) -> ()
      "jig cycle" <- 0
    }
    frame #1 {
      # "do 1st time set up"
      n4 = stacked-sequence {
        frame #0 {
          # "disable front panel while 1st time set up is being done"
          n5 = property on="Tab Control 2" class="TabCtl (strict)"("DisabledEnum"=T12."Disabled and Grayed Out" ("Disabled")) -> ()  [unwired: 2 in, 2 out]
        }
        frame #1 {
          # "get calibration values"
          n6 = call "sub vi - get calibration values v1.vi"() -> ("LAB01 (CAL)"=→"CAL LAB01":T7, "LAB02 (CAL)"=→"CAL LAB02":T8, "LAB03 (CAL)"=→"CAL LAB03":T7, "LAB04 (CAL)"=→"CAL LAB04":T7, "calibration file error out"=→"calibration file error out":errorcluster, "LAB05 (CAL)"=→"CAL LAB05":T7)  [unwired: 10 in]
        }
        frame #2 {
          # "get last saved test settings from file"
          n7 = local read "Network Directory"() -> (w13:path)
          n8 = local read "C drive data root dir"() -> (w11:path)
          n9 = local read "SET LAB05-2"() -> (w43:T5)
          n10 = local read "SET LAB05-1"() -> (w44:T5)
          n11 = local read "SET LAB04-2"() -> (w45:T5)
          n12 = local read "SET LAB03-2"() -> (w42:T5)
          n13 = local read "SET LAB04-1"() -> (w46:T5)
          n14 = local read "SET LAB03-1"() -> (w41:T5)
          n15 = local read "SET LAB02-2"() -> (w40:T5)
          n16 = local read "SET LAB02-1"() -> (w39:T5)
          n17 = local read "SET LAB01-2"() -> (w38:T5)
          n18 = local read "SET LAB01-1"() -> (w37:T5)
          n19 = Bundle("SET LAB01-1"=w37, "SET LAB01-2"=w38, "SET LAB02-1"=w39, "SET LAB02-2"=w40, "SET LAB03-1"=w41, "SET LAB03-2"=w42, "SET LAB04-1"=w46, "SET LAB04-2"=w45, "SET LAB05-1"=w44, "SET LAB05-2"=w43, "Network Directory"=w13, "C drive data root dir"=w11) -> (w30:T18)  [unwired: 1 in]
          n20 = String To Path(string="c:\\crabtree\\Set Up\\") -> (path=w34:path)
          n21 = Build Path(base path=w34, name or relative path="settings.bin") -> (appended path=w32:path)
          n22 = Create Folder(path (use dialog)=w34) -> (error out=w36:errorcluster)  [unwired: 2 in, 2 out]
          n23 = call <vilib>:"Clear Errors.vi"("error in (no error)"=w36) -> ()  [unwired: 6 in, 1 out]
          n24 = Open/Create/Replace File(file path (use dialog)=w32) -> (refnum out=w29:refnum<file>, error out=w31:errorcluster)  [unwired: 5 in, 1 out]
          n25 = Read from Binary File(5:w30, 8:w31, 11:w29) -> (0:w26:errorcluster, 2:w28:T18, 3:w27:refnum<file>)  [unwired: 3 in, 1 out]
          n26 = Unbundle(w28) -> ("SET LAB01-1"=w24:T5, "SET LAB01-2"=w23:T5, "SET LAB02-1"=w22:T5, "SET LAB02-2"=w21:T5, "SET LAB03-1"=w20:T5, "SET LAB03-2"=w19:T5, "SET LAB04-1"=w18:T5, "SET LAB04-2"=w17:T5, "SET LAB05-1"=w16:T5, "SET LAB05-2"=w15:T5, "Network Directory"=w14:path, "C drive data root dir"=w12:path)
          n27 = local write "C drive data root dir"(w12) -> ()
          n28 = Close File(refnum=w27, error in=w26) -> (error out=w25:errorcluster)  [unwired: 1 out]
          n29 = local write "Network Directory"(w14) -> ()
          n30 = local write "SET LAB04-2"(w17) -> ()
          n31 = local write "SET LAB05-1"(w16) -> ()
          n32 = local write "SET LAB04-1"(w18) -> ()
          n33 = local write "SET LAB05-2"(w15) -> ()
          n34 = local write "SET LAB02-1"(w22) -> ()
          n35 = local write "SET LAB02-2"(w21) -> ()
          n36 = local write "SET LAB03-1"(w20) -> ()
          n37 = local write "SET LAB03-2"(w19) -> ()
          n38 = local write "SET LAB01-1"(w24) -> ()
          n39 = local write "SET LAB01-2"(w23) -> ()
          n40 = local write "data file error"(w25) -> ()
        }
        frame #3 {
          # "get mail settings"
          n41 = local read "Auto Mail Send"() -> (w50:bool)
          n42 = local read "MAIL SETTINGS"() -> (w54:T6)
          n43 = String To Path(string="c:\\crabtree\\Set Up\\") -> (path=w62:path)
          n44 = Build Path(base path=w62, name or relative path="mail.bin") -> (appended path=w60:path)
          n45 = Create Folder(path (use dialog)=w62) -> (error out=w64:errorcluster)  [unwired: 2 in, 2 out]
          n46 = Bundle("MAIL SETTINGS"=w54, "Auto Mail Send"=w50, "") -> (w53:T19)  [unwired: 1 in]
          n47 = call <vilib>:"Clear Errors.vi"("error in (no error)"=w64) -> ()  [unwired: 6 in, 1 out]
          n48 = Open/Create/Replace File(file path (use dialog)=w60) -> (refnum out=w58:refnum<file>, error out=w59:errorcluster)  [unwired: 5 in, 1 out]
          n49 = Read from Binary File(5:w53, 8:w59, 11:w58) -> (0:w56:errorcluster, 2:w52:T19, 3:w57:refnum<file>)  [unwired: 3 in, 1 out]
          n50 = Unbundle(w52) -> ("MAIL SETTINGS"=w51:T6, "Auto Mail Send"=w49:bool, w48:string)
          n51 = local write "TO (string):"(w48) -> ()
          n52 = local write "Auto Mail Send"(w49) -> ()
          n53 = local write "MAIL SETTINGS"(w51) -> ()
          n54 = Close File(refnum=w57, error in=w56) -> (error out=w55:errorcluster)  [unwired: 1 out]
          n55 = local write "data file error"(w55) -> ()
        }
        frame #4 {
          # "set display status if blank"
          n56 = local read "DISP LAB03-2"() -> (w94:T4)
          n57 = local read "DISP LAB03-1"() -> (w101:T4)
          n58 = local read "DISP LAB02-2"() -> (w108:T4)
          n59 = local read "DISP LAB01-2"() -> (w121:T4)
          n60 = local read "DISP LAB01-1"() -> (w130:T4)
          n61 = local read "DISP LAB02-1"() -> (w115:T4)
          n62 = Unbundle(w94) -> ("STATUS"=w96:string)  [unwired: 2 out]
          n63 = Unbundle(w101) -> ("STATUS"=w103:string)  [unwired: 2 out]
          n64 = Unbundle(w108) -> ("STATUS"=w110:string)  [unwired: 2 out]
          n65 = Unbundle(w115) -> ("STATUS"=w117:string)  [unwired: 2 out]
          n66 = Unbundle(w121) -> ("STATUS"=w124:string)  [unwired: 2 out]
          n67 = Unbundle(w130) -> ("STATUS"=w131:string)  [unwired: 2 out]
          n68 = Equal?(x="", y=w96) -> (x = y?=w98:bool)
          n69 = Equal?(x="", y=w103) -> (x = y?=w105:bool)
          n70 = Equal?(x="", y=w110) -> (x = y?=w112:bool)
          n71 = Equal?(x="", y=w117) -> (x = y?=w119:bool)
          n72 = Equal?(x="", y=w124) -> (x = y?=w126:bool)
          n73 = Equal?(x="", y=w131) -> (x = y?=w133:bool)
          n74 = Select(t="STOP", s=w98, f=w96) -> (s? t:f=w95:string)
          n75 = Select(t="STOP", s=w105, f=w103) -> (s? t:f=w102:string)
          n76 = Select(t="STOP", s=w112, f=w110) -> (s? t:f=w109:string)
          n77 = Select(t="STOP", s=w119, f=w117) -> (s? t:f=w116:string)
          n78 = Select(t="STOP", s=w126, f=w124) -> (s? t:f=w123:string)
          n79 = Select(t="STOP", s=w133, f=w131) -> (s? t:f=w129:string)
          n80 = Bundle(cluster=w94, "STATUS"=w95) -> (w93:T4)  [unwired: 2 in]
          n81 = Bundle(cluster=w101, "STATUS"=w102) -> (w100:T4)  [unwired: 2 in]
          n82 = Bundle(cluster=w108, "STATUS"=w109) -> (w107:T4)  [unwired: 2 in]
          n83 = Bundle(cluster=w115, "STATUS"=w116) -> (w114:T4)  [unwired: 2 in]
          n84 = Bundle(cluster=w121, "STATUS"=w123) -> (w122:T4)  [unwired: 2 in]
          n85 = Bundle(cluster=w130, "STATUS"=w129) -> (w128:T4)  [unwired: 2 in]
          n86 = local write "DISP LAB01-2"(w122) -> ()
          n87 = local write "DISP LAB01-1"(w128) -> ()
          n88 = local write "DISP LAB02-1"(w114) -> ()
          n89 = local write "DISP LAB03-1"(w100) -> ()
          n90 = local write "DISP LAB02-2"(w107) -> ()
          n91 = local write "DISP LAB03-2"(w93) -> ()
          n92 = local read "DISP LAB05-2"() -> (w66:T4)
          n93 = local read "DISP LAB05-1"() -> (w73:T4)
          n94 = local read "DISP LAB04-2"() -> (w75:T4)
          n95 = local read "DISP LAB04-1"() -> (w77:T4)
          n96 = Unbundle(w66) -> ("STATUS"=w68:string)  [unwired: 2 out]
          n97 = Unbundle(w73) -> ("STATUS"=w79:string)  [unwired: 2 out]
          n98 = Unbundle(w75) -> ("STATUS"=w84:string)  [unwired: 2 out]
          n99 = Unbundle(w77) -> ("STATUS"=w89:string)  [unwired: 2 out]
          n100 = Equal?(x="", y=w68) -> (x = y?=w70:bool)
          n101 = Equal?(x="", y=w79) -> (x = y?=w81:bool)
          n102 = Equal?(x="", y=w84) -> (x = y?=w86:bool)
          n103 = Equal?(x="", y=w89) -> (x = y?=w91:bool)
          n104 = Select(t="STOP", s=w70, f=w68) -> (s? t:f=w67:string)
          n105 = Select(t="STOP", s=w81, f=w79) -> (s? t:f=w78:string)
          n106 = Select(t="STOP", s=w86, f=w84) -> (s? t:f=w83:string)
          n107 = Select(t="STOP", s=w91, f=w89) -> (s? t:f=w88:string)
          n108 = Bundle(cluster=w66, "STATUS"=w67) -> (w65:T4)  [unwired: 2 in]
          n109 = Bundle(cluster=w73, "STATUS"=w78) -> (w72:T4)  [unwired: 2 in]
          n110 = Bundle(cluster=w75, "STATUS"=w83) -> (w74:T4)  [unwired: 2 in]
          n111 = Bundle(cluster=w77, "STATUS"=w88) -> (w76:T4)  [unwired: 2 in]
          n112 = local write "DISP LAB05-2"(w65) -> ()
          n113 = local write "DISP LAB05-1"(w72) -> ()
          n114 = local write "DISP LAB04-1"(w76) -> ()
          n115 = local write "DISP LAB04-2"(w74) -> ()
        }
        frame #5 {
          # "initialise analog input express vi's"
          n116 = for {
            N: 2.0 -> [_]
            n117 = call "sub vi - analog 1st setup v1.vi"() -> ()  [unwired: 11 in, 5 out]
          }
        }
        frame #6 {
          # "enable front panel, all settings done"
          n118 = property on="Tab Control 2" class="TabCtl (strict)"("DisabledEnum"=T12."Enabled" ("Disabled")) -> ()  [unwired: 2 in, 2 out]
        }
      }
    }
    frame #2 {
      n119 = node-c288("loop  delay(mS)") -> (w139:T13)  [unwired: 3 in]
      n120 = timed-loop {
        timing: w139 -> [_]
        timing-out: [_] -> w138
        i -> [w161]
        stop <- "stop" stop-if-true
        n121 = node-c288() -> ()  [unwired: 1 in, 1 out]
        n122 = local read "SELECT LAB05-2"() -> (w141:T3)
        n123 = local read "SELECT LAB05-1"() -> (w142:T3)
        n124 = local read "SELECT LAB04-2"() -> (w143:T3)
        n125 = local read "SELECT LAB03-1"() -> (w146:T3)
        n126 = local read "SELECT LAB02-2"() -> (w147:T3)
        n127 = local read "SELECT LAB01-1"() -> (w150:T3)
        n128 = local read "SELECT LAB03-2"() -> (w145:T3)
        n129 = local read "SELECT LAB01-2"() -> (w149:T3)
        n130 = local read "SELECT LAB04-1"() -> (w144:T3)
        n131 = local read "SELECT LAB02-1"() -> (w148:T3)
        n132 = local read "run lab03-2"() -> (w155:bool)
        n133 = local read "run lab04-1"() -> (w154:bool)
        n134 = local read "run lab05-1"() -> (w152:bool)
        n135 = local read "run lab04-2"() -> (w153:bool)
        n136 = local read "run lab05-2"() -> (w151:bool)
        n137 = local read "run lab03-1"() -> (w156:bool)
        n138 = local read "run lab02-2"() -> (w157:bool)
        n139 = local read "run lab02-1"() -> (w158:bool)
        n140 = local read "run lab01-1"() -> (w160:bool)
        n141 = local read "run lab01-2"() -> (w159:bool)
        n142 = stacked-sequence {
          seq-local: [_ w223 _ _ _ _ _ _ _ _ _ _ _ _ _ _ _ _] -> [_ _ _ _ _ w1758 _ _ _ _ _ _ _ _ _ _ _ _]
          seq-local: [_ w222 _ _ _ _ _ _ _ _ _ _ _ _ _ _ _ _] -> [_ _ _ _ _ w1757 _ _ _ _ _ _ _ _ _ _ _ _]
          seq-local: [_ w209 _ _ _ _ _ _ _ _ _ _ _ _ _ _ _ _] -> [_ _ _ _ _ w1756 _ _ _ _ _ _ _ _ _ _ _ _]
          seq-local: [_ w208 _ _ _ _ _ _ _ _ _ _ _ _ _ _ _ _] -> [_ _ _ _ _ w1755 _ _ _ _ _ _ _ _ _ _ _ _]
          seq-local: [_ w207 _ _ _ _ _ _ _ _ _ _ _ _ _ _ _ _] -> [_ _ _ _ _ w1754 _ _ _ _ _ _ _ _ _ _ _ _]
          seq-local: [_ w206 _ _ _ _ _ _ _ _ _ _ _ _ _ _ _ _] -> [_ _ _ _ _ w1753 _ _ _ _ _ _ _ _ _ _ _ _]
          seq-local: [_ w205 _ _ _ _ _ _ _ _ _ _ _ _ _ _ _ _] -> [_ _ _ _ _ w1752 _ _ _ _ _ _ _ _ _ _ _ _]
          seq-local: [_ w204 _ _ _ _ _ _ _ _ _ _ _ _ _ _ _ _] -> [_ _ _ _ _ w1751 _ _ _ _ _ _ _ _ _ _ _ _]
          seq-local: [_ w203 _ _ _ _ _ _ _ _ _ _ _ _ _ _ _ _] -> [_ _ _ _ _ w1750 _ _ _ _ _ _ _ _ _ _ _ _]
          seq-local: [_ w202 _ _ _ _ _ _ _ _ _ _ _ _ _ _ _ _] -> [_ _ _ _ _ w1749 _ _ _ _ _ _ _ _ _ _ _ _]
          tunnel: w160 -> [_ _ w239 w404 w1348 w1778 w2088 w2333 _ _ _ _ _ w2806 w3751 _ _ w4026]
          tunnel: w159 -> [_ _ w238 w402 w1347 w1777 w2089 w2332 _ _ _ _ _ w2805 w3749 _ _ w4025]
          tunnel: w158 -> [_ _ w237 w400 w1346 w1776 w2087 w2331 _ _ _ _ _ w2804 w3747 _ _ w4024]
          tunnel: w157 -> [_ _ w236 w398 w1345 w1775 w2086 w2330 _ _ _ _ _ w2803 w3745 _ _ w4023]
          tunnel: w156 -> [_ _ w235 w396 w1344 w1774 w2085 w2329 _ _ _ _ _ w2802 w3743 _ _ w4022]
          tunnel: w155 -> [_ _ w234 w394 w1343 w1773 w2084 w2328 _ _ _ _ _ w2801 w3741 _ _ w4021]
          tunnel: w154 -> [_ _ w233 w392 w1342 w1772 w2083 w2327 _ _ _ _ _ w2800 w3739 _ _ w4020]
          tunnel: w153 -> [_ _ w232 w390 w1341 w1771 w2082 w2326 _ _ _ _ _ w2799 w3737 _ _ w4019]
          tunnel: w152 -> [_ _ w231 w388 w1340 w1770 w2081 w2325 _ _ _ _ _ w2798 w3735 _ _ w4018]
          tunnel: w151 -> [_ _ w230 w386 w1339 w1769 w2080 w2324 _ _ _ _ _ w2797 w3733 _ _ w4017]
          tunnel: w150 -> [_ _ _ w403 w1338 w1768 _ _ _ _ _ _ _ _ w3753 _ _ _]
          tunnel: w149 -> [_ _ _ w401 w1337 w1767 _ _ _ _ _ _ _ _ w3748 _ _ _]
          tunnel: w148 -> [_ _ _ w399 w1336 w1766 _ _ _ _ _ _ _ _ w3746 _ _ _]
          tunnel: w147 -> [_ _ _ w397 w1335 w1765 _ _ _ _ _ _ _ _ w3744 _ _ _]
          tunnel: w146 -> [_ _ _ w395 w1334 w1764 _ _ _ _ _ _ _ _ w3742 _ _ _]
          tunnel: w145 -> [_ _ _ w393 w1333 w1763 _ _ _ _ _ _ _ _ w3740 _ _ _]
          tunnel: w144 -> [_ _ _ w391 w1332 w1762 _ _ _ _ _ _ _ _ w3738 _ _ _]
          tunnel: w143 -> [_ _ _ w389 w1331 w1761 _ _ _ _ _ _ _ _ w3736 _ _ _]
          tunnel: w142 -> [_ _ _ w387 w1330 w1760 _ _ _ _ _ _ _ _ w3734 _ _ _]
          tunnel: w141 -> [_ _ _ w385 w1329 w1759 _ _ _ _ _ _ _ _ w3732 _ _ _]
          frame #0 {
            w165 = FALSE
            w170 = 0.5
            # "set up cycle control"
            n143 = local read "jig cycle"() -> (w169:dbl)
            n144 = Divide(x="JIG ON TIME (S)", y=w170) -> (x/y=→"on loops":dbl)
            n145 = Divide(x="JIG OFF TIME (S)", y=w170) -> (x/y=→"off loops":dbl)
            n146 = Increment(x=w169) -> (x+1=w168:dbl)
            n147 = local write "TEMP update"(w165) -> ()
            n148 = local write "AI update"(w165) -> ()
            n149 = local write "jig cycle"(w168) -> ()
            n150 = event shown="[1] \"SHOW ADMIN PAGE\": Value Change" {
              selector: _ -> [_ _]
              dyn-events: _ -> [_ _]
              timeout: 10 -> [_ _]
              event Timeout {
                n151 = event-data() -> ()  [unwired: 1 in, 3 out]
              }
              event "SHOW ADMIN PAGE": Value Change {
                n152 = event-data() -> ()  [unwired: 1 in, 6 out]
                n153 = stacked-sequence {
                  seq-local: [_ w174 _] -> [_ _ w175]
                  frame #0 {
                    n154 = global write "Global 1.vi" "password"("9999") -> ()
                  }
                  frame #1 {
                    n155 = call "sub vi - password 1.vi"() -> ("RESULT"=w174:bool)  [unwired: 11 in]
                  }
                  frame #2 {
                    w177 = FALSE
                    n156 = property on="Tab Control 2" class="TabCtl (strict)"() -> ("Pages"=w181:refnum<vi>[])  [unwired: 2 in, 2 out]
                    n157 = Select(t=TRUE, s=w175, f=w177) -> (s? t:f=w176:bool)
                    n158 = Index Array(array=w181, index=6) -> (element=w179:refnum<vi>)
                    n159 = local write "SHOW ADMIN PAGE"(w177) -> ()
                    n160 = property class="Page"(reference=w179, "PageVis"=w176) -> ()  [unwired: 1 in, 2 out]
                  }
                }
              }
            }
          }
          frame #1 {
            w219 = 60.0
            # "convert temperature rise minutes to cycles"
            n161 = local read "SET LAB05-2"() -> (w183:T5)
            n162 = local read "SET LAB05-1"() -> (w185:T5)
            n163 = local read "SET LAB04-2"() -> (w187:T5)
            n164 = local read "SET LAB01-1"() -> (w201:T5)
            n165 = local read "SET LAB01-2"() -> (w199:T5)
            n166 = local read "SET LAB02-2"() -> (w195:T5)
            n167 = local read "SET LAB04-1"() -> (w189:T5)
            n168 = local read "SET LAB03-1"() -> (w193:T5)
            n169 = local read "SET LAB03-2"() -> (w191:T5)
            n170 = local read "SET LAB02-1"() -> (w197:T5)
            n171 = local read "JIG OFF TIME (S)"() -> (w224:dbl)
            n172 = local read "JIG ON TIME (S)"() -> (w225:dbl)
            n173 = Unbundle(w183) -> ("T-RISE mins"=w182:dbl)  [unwired: 4 out]
            n174 = Unbundle(w185) -> ("T-RISE mins"=w184:dbl)  [unwired: 4 out]
            n175 = Unbundle(w201) -> ("T-RISE mins"=w200:dbl)  [unwired: 4 out]
            n176 = Unbundle(w187) -> ("T-RISE mins"=w186:dbl)  [unwired: 4 out]
            n177 = Unbundle(w199) -> ("T-RISE mins"=w198:dbl)  [unwired: 4 out]
            n178 = Unbundle(w197) -> ("T-RISE mins"=w196:dbl)  [unwired: 4 out]
            n179 = Unbundle(w189) -> ("T-RISE mins"=w188:dbl)  [unwired: 4 out]
            n180 = Unbundle(w195) -> ("T-RISE mins"=w194:dbl)  [unwired: 4 out]
            n181 = Unbundle(w191) -> ("T-RISE mins"=w190:dbl)  [unwired: 4 out]
            n182 = Unbundle(w193) -> ("T-RISE mins"=w192:dbl)  [unwired: 4 out]
            n183 = Add(x=w225, y=w224) -> (x+y=w218:dbl)
            n184 = Multiply(x=w219, y=w190) -> (x*y=w214:dbl)
            n185 = Multiply(x=w219, y=w188) -> (x*y=w213:dbl)
            n186 = Multiply(x=w219, y=w186) -> (x*y=w212:dbl)
            n187 = Multiply(x=w219, y=w184) -> (x*y=w211:dbl)
            n188 = Multiply(x=w219, y=w182) -> (x*y=w210:dbl)
            n189 = Multiply(x=w219, y=w198) -> (x*y=w220:dbl)
            n190 = Multiply(x=w219, y=w192) -> (x*y=w215:dbl)
            n191 = Multiply(x=w219, y=w200) -> (x*y=w221:dbl)
            n192 = Multiply(x=w219, y=w196) -> (x*y=w217:dbl)
            n193 = Multiply(x=w219, y=w194) -> (x*y=w216:dbl)
            n194 = Divide(x=w211, y=w218) -> (x/y=w203:dbl)
            n195 = Divide(x=w212, y=w218) -> (x/y=w204:dbl)
            n196 = Divide(x=w213, y=w218) -> (x/y=w205:dbl)
            n197 = Divide(x=w210, y=w218) -> (x/y=w202:dbl)
            n198 = Divide(x=w215, y=w218) -> (x/y=w207:dbl)
            n199 = Divide(x=w221, y=w218) -> (x/y=w223:dbl)
            n200 = Divide(x=w220, y=w218) -> (x/y=w222:dbl)
            n201 = Divide(x=w217, y=w218) -> (x/y=w209:dbl)
            n202 = Divide(x=w216, y=w218) -> (x/y=w208:dbl)
            n203 = Divide(x=w214, y=w218) -> (x/y=w206:dbl)
          }
          frame #2 {
            # "control cycle loops"
            n204 = local read "JIG OFF TIME (S)"() -> (w228:dbl)
            n205 = local read "JIG ON TIME (S)"() -> (w227:dbl)
            n206 = local read "jig cycle"() -> (w241:dbl)
            n207 = local read "on loops"() -> (w243:dbl)
            n208 = local read "off loops"() -> (w242:dbl)
            n209 = Add(x=w228, y=w227) -> (x+y=w226:dbl)
            n210 = Add(x=w243, y=w242) -> (x+y=w229:dbl)
            n211 = Greater Or Equal?(x=w241, y=w229) -> (x >= y?=w240:bool)
            n212 = case shown="True" w240 {
              tunnel: w239 -> [_ w254]
              tunnel: w238 -> [_ w253]
              tunnel: w237 -> [_ w252]
              tunnel: w236 -> [_ w251]
              tunnel: w235 -> [_ w250]
              tunnel: w234 -> [_ w249]
              tunnel: w233 -> [_ w248]
              tunnel: w232 -> [_ w247]
              tunnel: w231 -> [_ w246]
              tunnel: w230 -> [_ w245]
              tunnel: w226 -> [_ w244]
              frame False {
              }
              frame True {
                # "increment cycle value and convert cycles to minutes for temp rise"
                n213 = stacked-sequence {
                  tunnel: w254 -> [w264 _ _ _ _ _ _ _ _ _]
                  tunnel: w253 -> [_ w276 _ _ _ _ _ _ _ _]
                  tunnel: w252 -> [_ _ w288 _ _ _ _ _ _ _]
                  tunnel: w251 -> [_ _ _ w300 _ _ _ _ _ _]
                  tunnel: w250 -> [_ _ _ _ w312 _ _ _ _ _]
                  tunnel: w249 -> [_ _ _ _ _ w324 _ _ _ _]
                  tunnel: w248 -> [_ _ _ _ _ _ w336 _ _ _]
                  tunnel: w247 -> [_ _ _ _ _ _ _ w348 _ _]
                  tunnel: w246 -> [_ _ _ _ _ _ _ _ w360 _]
                  tunnel: w245 -> [_ _ _ _ _ _ _ _ _ w372]
                  tunnel: w244 -> [w261 w273 w285 w297 w309 w321 w333 w345 w357 w369]
                  frame #0 {
                    # "LAB01-1"
                    n214 = local read "DISP LAB01-1"() -> (w259:T4)
                    n215 = Unbundle(w259) -> ("CYCLE"=w260:dbl)  [unwired: 2 out]
                    n216 = case shown="True" w264 {
                      tunnel: w260 -> [w265 w267]
                      tunnel: [w265 w266] -> w258
                      frame False {
                      }
                      frame True {
                        n217 = Increment(x=w267) -> (x+1=w266:dbl)
                      }
                    }
                    n218 = Multiply(x=w258, y=w261) -> (x*y=w262:dbl)
                    n219 = Divide(x=w262, y=60.0) -> (x/y=w257:dbl)
                    n220 = Bundle(cluster=w259, "CYCLE"=w258, "MINS"=w257) -> (w256:T4)  [unwired: 1 in]
                    n221 = local write "DISP LAB01-1"(w256) -> ()
                  }
                  frame #1 {
                    # "update cycle value"
                    # "LAB01-2"
                    n222 = local read "DISP LAB01-2"() -> (w271:T4)
                    n223 = Unbundle(w271) -> ("CYCLE"=w272:dbl)  [unwired: 2 out]
                    n224 = case shown="True" w276 {
                      tunnel: w272 -> [w277 w279]
                      tunnel: [w277 w278] -> w269
                      frame False {
                      }
                      frame True {
                        n225 = Increment(x=w279) -> (x+1=w278:dbl)
                      }
                    }
                    n226 = Multiply(x=w269, y=w273) -> (x*y=w274:dbl)
                    n227 = Divide(x=w274, y=60.0) -> (x/y=w268:dbl)
                    n228 = Bundle(cluster=w271, "CYCLE"=w269, "MINS"=w268) -> (w270:T4)  [unwired: 1 in]
                    n229 = local write "DISP LAB01-2"(w270) -> ()
                  }
                  frame #2 {
                    # "update cycle value"
                    # "LAB02-1"
                    n230 = local read "DISP LAB02-1"() -> (w283:T4)
                    n231 = Unbundle(w283) -> ("CYCLE"=w284:dbl)  [unwired: 2 out]
                    n232 = case shown="True" w288 {
                      tunnel: [w289 w291] -> w281
                      tunnel: w284 -> [w289 w290]
                      frame False {
                      }
                      frame True {
                        n233 = Increment(x=w290) -> (x+1=w291:dbl)
                      }
                    }
                    n234 = Multiply(x=w281, y=w285) -> (x*y=w286:dbl)
                    n235 = Divide(x=w286, y=60.0) -> (x/y=w280:dbl)
                    n236 = Bundle(cluster=w283, "CYCLE"=w281, "MINS"=w280) -> (w282:T4)  [unwired: 1 in]
                    n237 = local write "DISP LAB02-1"(w282) -> ()
                  }
                  frame #3 {
                    # "update cycle value"
                    # "LAB02-2"
                    n238 = local read "DISP LAB02-2"() -> (w295:T4)
                    n239 = Unbundle(w295) -> ("CYCLE"=w296:dbl)  [unwired: 2 out]
                    n240 = case shown="True" w300 {
                      tunnel: [w301 w303] -> w294
                      tunnel: w296 -> [w301 w302]
                      frame False {
                      }
                      frame True {
                        n241 = Increment(x=w302) -> (x+1=w303:dbl)
                      }
                    }
                    n242 = Multiply(x=w294, y=w297) -> (x*y=w298:dbl)
                    n243 = Divide(x=w298, y=60.0) -> (x/y=w293:dbl)
                    n244 = Bundle(cluster=w295, "CYCLE"=w294, "MINS"=w293) -> (w292:T4)  [unwired: 1 in]
                    n245 = local write "DISP LAB02-2"(w292) -> ()
                  }
                  frame #4 {
                    # "update cycle value"
                    # "LAB03-1"
                    n246 = local read "DISP LAB03-1"() -> (w307:T4)
                    n247 = Unbundle(w307) -> ("CYCLE"=w308:dbl)  [unwired: 2 out]
                    n248 = case shown="True" w312 {
                      tunnel: [w313 w315] -> w304
                      tunnel: w308 -> [w313 w314]
                      frame False {
                      }
                      frame True {
                        n249 = Increment(x=w314) -> (x+1=w315:dbl)
                      }
                    }
                    n250 = Multiply(x=w304, y=w309) -> (x*y=w310:dbl)
                    n251 = Divide(x=w310, y=60.0) -> (x/y=w305:dbl)
                    n252 = Bundle(cluster=w307, "CYCLE"=w304, "MINS"=w305) -> (w306:T4)  [unwired: 1 in]
                    n253 = local write "DISP LAB03-1"(w306) -> ()
                  }
                  frame #5 {
                    # "update cycle value"
                    # "LAB03-2"
                    n254 = local read "DISP LAB03-2"() -> (w319:T4)
                    n255 = Unbundle(w319) -> ("CYCLE"=w320:dbl)  [unwired: 2 out]
                    n256 = case shown="False" w324 {
                      tunnel: [w325 w327] -> w318
                      tunnel: w320 -> [w325 w326]
                      frame False {
                      }
                      frame True {
                        n257 = Increment(x=w326) -> (x+1=w327:dbl)
                      }
                    }
                    n258 = Multiply(x=w318, y=w321) -> (x*y=w322:dbl)
                    n259 = Divide(x=w322, y=60.0) -> (x/y=w317:dbl)
                    n260 = Bundle(cluster=w319, "CYCLE"=w318, "MINS"=w317) -> (w316:T4)  [unwired: 1 in]
                    n261 = local write "DISP LAB03-2"(w316) -> ()
                  }
                  frame #6 {
                    # "update cycle value"
                    # "LAB04-1"
                    n262 = local read "DISP LAB04-1"() -> (w331:T4)
                    n263 = Unbundle(w331) -> ("CYCLE"=w332:dbl)  [unwired: 2 out]
                    n264 = case shown="True" w336 {
                      tunnel: [w337 w339] -> w329
                      tunnel: w332 -> [w337 w338]
                      frame False {
                      }
                      frame True {
                        n265 = Increment(x=w338) -> (x+1=w339:dbl)
                      }
                    }
                    n266 = Multiply(x=w329, y=w333) -> (x*y=w334:dbl)
                    n267 = Divide(x=w334, y=60.0) -> (x/y=w328:dbl)
                    n268 = Bundle(cluster=w331, "CYCLE"=w329, "MINS"=w328) -> (w330:T4)  [unwired: 1 in]
                    n269 = local write "DISP LAB04-1"(w330) -> ()
                  }
                  frame #7 {
                    # "update cycle value"
                    # "LAB04-2"
                    n270 = local read "DISP LAB04-2"() -> (w343:T4)
                    n271 = Unbundle(w343) -> ("CYCLE"=w344:dbl)  [unwired: 2 out]
                    n272 = case shown="True" w348 {
                      tunnel: [w349 w351] -> w341
                      tunnel: w344 -> [w349 w350]
                      frame False {
                      }
                      frame True {
                        n273 = Increment(x=w350) -> (x+1=w351:dbl)
                      }
                    }
                    n274 = Multiply(x=w341, y=w345) -> (x*y=w347:dbl)
                    n275 = Divide(x=w347, y=60.0) -> (x/y=w340:dbl)
                    n276 = Bundle(cluster=w343, "CYCLE"=w341, "MINS"=w340) -> (w342:T4)  [unwired: 1 in]
                    n277 = local write "DISP LAB04-2"(w342) -> ()
                  }
                  frame #8 {
                    # "update cycle value"
                    # "LAB05-1"
                    n278 = local read "DISP LAB05-1"() -> (w355:T4)
                    n279 = Unbundle(w355) -> ("CYCLE"=w356:dbl)  [unwired: 2 out]
                    n280 = case shown="True" w360 {
                      tunnel: [w361 w363] -> w353
                      tunnel: w356 -> [w361 w362]
                      frame False {
                      }
                      frame True {
                        n281 = Increment(x=w362) -> (x+1=w363:dbl)
                      }
                    }
                    n282 = Multiply(x=w353, y=w357) -> (x*y=w358:dbl)
                    n283 = Divide(x=w358, y=60.0) -> (x/y=w352:dbl)
                    n284 = Bundle(cluster=w355, "CYCLE"=w353, "MINS"=w352) -> (w354:T4)  [unwired: 1 in]
                    n285 = local write "DISP LAB05-1"(w354) -> ()
                  }
                  frame #9 {
                    # "update cycle value"
                    # "LAB05-2"
                    n286 = local read "DISP LAB05-2"() -> (w368:T4)
                    n287 = Unbundle(w368) -> ("CYCLE"=w367:dbl)  [unwired: 2 out]
                    n288 = case shown="True" w372 {
                      tunnel: [w373 w375] -> w366
                      tunnel: w367 -> [w373 w374]
                      frame False {
                      }
                      frame True {
                        n289 = Increment(x=w374) -> (x+1=w375:dbl)
                      }
                    }
                    n290 = Multiply(x=w366, y=w369) -> (x*y=w370:dbl)
                    n291 = Divide(x=w370, y=60.0) -> (x/y=w365:dbl)
                    n292 = Bundle(cluster=w368, "CYCLE"=w366, "MINS"=w365) -> (w364:T4)  [unwired: 1 in]
                    n293 = local write "DISP LAB05-2"(w364) -> ()
                  }
                }
                n294 = local write "jig cycle"(0) -> ()
              }
            }
          }
          frame #3 {
            # "START & STOP test RUN switch change, start test if true and stop test if false"
            n295 = Get Date/Time In Seconds() -> (seconds since 1Jan1904=w383:timestamp)
            n296 = local read "C drive data root dir"() -> (w376:path)
            n297 = Format Date/Time String(time format string (%c)="%b\\%a%d", seconds (now)=w383) -> (date/time string=w407:string)  [unwired: 1 in]
            n298 = Format Date/Time String(time format string (%c)="%H%M", seconds (now)=w383) -> (date/time string=w405:string)  [unwired: 1 in]
            n299 = Format Date/Time String(time format string (%c)="LabPanel%Y", seconds (now)=w383) -> (date/time string=w382:string)  [unwired: 1 in]
            n300 = Path To String(path=w376) -> (string=w379:string)
            n301 = global write "Global 1.vi" "C drive root path"(w376) -> ()
            n302 = Concatenate Strings(w379, "\\") -> (w377:string)
            n303 = event shown="[2] \"RUN LAB01-2\": Value Change" {
              selector: _ -> [_ _ _ _ _ _ _ _ _ _ _]
              dyn-events: _ -> [_ _ _ _ _ _ _ _ _ _ _]
              timeout: 10 -> [_ _ _ _ _ _ _ _ _ _ _]
              tunnel: w377 -> [_ w415 w507 w599 w691 w783 w875 w967 w1059 w1151 w1243]
              tunnel: w407 -> [_ w414 w506 w598 w690 w782 w874 w966 w1058 w1150 w1242]
              tunnel: w405 -> [_ w412 w505 w597 w689 w781 w873 w965 w1057 w1149 w1241]
              tunnel: w403 -> [_ w413 _ _ _ _ _ _ _ _ _]
              tunnel: w404 -> [_ _ _ _ _ _ _ _ _ _ _]
              tunnel: w402 -> [_ _ _ _ _ _ _ _ _ _ _]
              tunnel: w401 -> [_ _ w504 _ _ _ _ _ _ _ _]
              tunnel: w400 -> [_ _ _ _ _ _ _ _ _ _ _]
              tunnel: w399 -> [_ _ _ w596 _ _ _ _ _ _ _]
              tunnel: w398 -> [_ _ _ _ _ _ _ _ _ _ _]
              tunnel: w397 -> [_ _ _ _ w688 _ _ _ _ _ _]
              tunnel: w396 -> [_ _ _ _ _ _ _ _ _ _ _]
              tunnel: w395 -> [_ _ _ _ _ w780 _ _ _ _ _]
              tunnel: w394 -> [_ _ _ _ _ _ _ _ _ _ _]
              tunnel: w393 -> [_ _ _ _ _ _ w872 _ _ _ _]
              tunnel: w392 -> [_ _ _ _ _ _ _ _ _ _ _]
              tunnel: w391 -> [_ _ _ _ _ _ _ w964 _ _ _]
              tunnel: w390 -> [_ _ _ _ _ _ _ _ _ _ _]
              tunnel: w389 -> [_ _ _ _ _ _ _ _ w1056 _ _]
              tunnel: w388 -> [_ _ _ _ _ _ _ _ _ _ _]
              tunnel: w387 -> [_ _ _ _ _ _ _ _ _ w1148 _]
              tunnel: w386 -> [_ _ _ _ _ _ _ _ _ _ _]
              tunnel: w385 -> [_ _ _ _ _ _ _ _ _ _ w1240]
              tunnel: w382 -> [_ w411 w503 w595 w687 w779 w871 w963 w1055 w1147 w1239]
              tunnel: [_ w410 w502 w594 w686 w778 w870 w962 w1054 w1146 w1238] -> w380
              event Timeout {
                n304 = event-data() -> ()  [unwired: 1 in, 3 out]
              }
              event "RUN LAB01-1": Value Change {
                n305 = event-data() -> ("NewVal"=w409:bool)  [unwired: 1 in, 5 out]
                n306 = local write "run lab01-1"(w409) -> ()
                n307 = case shown="True" w409 {
                  tunnel: w415 -> [_ w448]
                  tunnel: w414 -> [_ w447]
                  tunnel: w413 -> [w417 w446]
                  tunnel: w412 -> [_ w445]
                  tunnel: w411 -> [_ w444]
                  tunnel: [w416 w443] -> w410
                  frame False {
                    # "stop test"
                    n308 = stacked-sequence {
                      tunnel: w417 -> [_ w429 _ _]
                      tunnel: [_ w421 _ _] -> w416
                      frame #0 {
                        n309 = local read "DISP LAB01-1"() -> (w420:T4)
                        n310 = Bundle(cluster=w420, "STATUS"="STOP") -> (w418:T4)  [unwired: 2 in]
                        n311 = local write "DISP LAB01-1"(w418) -> ()
                      }
                      frame #1 {
                        n312 = local read "DISP LAB01-1"() -> (w428:T4)
                        n313 = Unbundle(w428) -> ("CYCLE"=w426:dbl, "MINS"=w427:dbl)  [unwired: 1 out]
                        n314 = case shown="\"CYCLE TEST\"" w429 {
                          tunnel: w427 -> [_ _ w436]
                          tunnel: w426 -> [w434 w435 _]
                          tunnel: [w434 w435 w436] -> w425
                          frame "CHART TEST", Default {
                          }
                          frame "CYCLE TEST" {
                          }
                          frame "T-RISE TEST" {
                          }
                        }
                        n315 = local read "TDMS LAB01-1"() -> (w433:refnum<k34>)
                        n316 = Build Array("STOPPED") -> (w430:string[])
                        n317 = Build Array(w425) -> (w424:dbl[])
                        n318 = TDMS Write(0:w433, 5:"TEST RESULT", 7:w430, 9:w424) -> (4:w422:refnum<k34>, 15:w423:errorcluster)  [unwired: 2 in, 2 out]
                        n319 = TDMS Close(8:w423, 11:w422) -> (0:w421:errorcluster)  [unwired: 1 out]
                      }
                      frame #2 {
                        n320 = stacked-sequence {
                          tunnel: "LAB01-1" -> [w439 w441]
                          frame #0 {
                            n321 = call "sub vi - defrag tdms v1.vi"("panel id"=w439) -> ("error out"=w438:errorcluster)  [unwired: 10 in]
                            n322 = local write "data file error"(w438) -> ()
                          }
                          frame #1 {
                            n323 = call "Save data file to network drive v1.vi"("panel id"=w441) -> ("network file save error"=w440:errorcluster)  [unwired: 9 in, 1 out]
                            n324 = local write "RESULT LAB01-1"(FALSE) -> ()
                            n325 = local write "data file error"(w440) -> ()
                          }
                        }
                      }
                      frame #3 {
                      }
                    }
                  }
                  frame True {
                    # "start new test and create test file"
                    n326 = stacked-sequence {
                      seq-local: [w449 _ _ _ _] -> [_ w470 _ _ _]
                      tunnel: w448 -> [w454 _ _ _ _]
                      tunnel: w447 -> [w450 _ _ _ _]
                      tunnel: w446 -> [w464 _ _ _ _]
                      tunnel: w445 -> [w457 _ _ _ _]
                      tunnel: w444 -> [w452 _ _ _ _]
                      tunnel: [_ w471 _ _ _] -> w443
                      frame #0 {
                        w451 = "\\"
                        n327 = case shown="\"CHART TEST\", Default" w464 {
                          tunnel: ["L01-1-CHART TEST-" "L01-1-CYCLE TEST-" "L01-1-T-RISE TEST-"] -> w460
                          frame "CHART TEST", Default {
                          }
                          frame "CYCLE TEST" {
                          }
                          frame "T-RISE TEST" {
                          }
                        }
                        n328 = local read "SET LAB01-1"() -> (w459:T5)
                        n329 = Unbundle(w459) -> ("DESCRIPTION"=w458:string)  [unwired: 4 out]
                        n330 = Concatenate Strings(w454, "\\", w452, w451, w450, w451) -> (w461:string)
                        n331 = String To Path(string=w461) -> (path=w463:path)
                        n332 = Concatenate Strings(w461, w460, w458, "-", w457, ".tdms") -> (w449:string)
                        n333 = Create Folder(path (use dialog)=w463) -> (error out=w462:errorcluster)  [unwired: 2 in, 2 out]
                        n334 = call <vilib>:"Clear Errors.vi"("error in (no error)"=w462) -> ()  [unwired: 6 in, 1 out]
                        n335 = global write "Global 1.vi" "LAB01-1 FILE"(w449) -> ()
                      }
                      frame #1 {
                        n336 = String To Path(string=w470) -> (path=w468:path)
                        n337 = TDMS Open(5:FALSE, 6:FALSE, 10:T16."create or replace" ("operation (0:open)"), 11:w468) -> (0:w471:errorcluster, 3:→"TDMS LAB01-1":refnum<k34>)  [unwired: 3 in]
                      }
                      frame #2 {
                        n338 = local read "TDMS LAB01-1"() -> (w491:refnum<k34>)
                        n339 = local read "SET LAB01-1"() -> (w480:T5)
                        n340 = Build Array("Testers Name", "Description", "Set Test Cycles", "T-Rise minutes", "T-Rise Deg C") -> (w481:string[])
                        n341 = Unbundle(w480) -> ("NAME"=w479:string, "DESCRIPTION"=w478:string, "CYCLES"=w477:dbl, "T-RISE mins"=w476:dbl, "T-RISE deg C"=w475:dbl)
                        n342 = Number To Decimal String(number=w477) -> (decimal integer string=w490:string)  [unwired: 1 in]
                        n343 = Number To Decimal String(number=w476) -> (decimal integer string=w489:string)  [unwired: 1 in]
                        n344 = Number To Decimal String(number=w475) -> (decimal integer string=w488:string)  [unwired: 1 in]
                        n345 = Build Array(w479, w478, w490, w489, w488) -> (w487:string[])
                        n346 = TDMS Set Properties(5:w487, 7:w481, 11:w491) -> ()  [unwired: 3 in, 4 out]
                      }
                      frame #3 {
                        w492 = 0.0
                        n347 = local read "DISP LAB01-1"() -> (w495:T4)
                        n348 = Bundle(cluster=w495, "CYCLE"=w492, "MINS"=w492, "STATUS"="RUN") -> (w494:T4)
                        n349 = local write "DISP LAB01-1"(w494) -> ()
                      }
                      frame #4 {
                        n350 = local read "SIG LAB01-1"() -> (w498:T2)
                        n351 = local read "TEMP START LAB01-1"() -> (w500:cluster{"TL":dbl, "TN":dbl})
                        n352 = Unbundle(w498) -> ("Tmp Live"=w497:dbl, "Tmp Neut"=w496:dbl)  [unwired: 3 out]
                        n353 = Bundle(cluster=w500, "TL"=w497, "TN"=w496) -> (w499:cluster{"TL":dbl, "TN":dbl})
                        n354 = local write "TEMP START LAB01-1"(w499) -> ()
                      }
                    }
                  }
                }
              }
              event "RUN LAB01-2": Value Change {
                n355 = event-data() -> ("NewVal"=w501:bool)  [unwired: 1 in, 5 out]
                n356 = local write "run lab01-2"(w501) -> ()
                n357 = case shown="True" w501 {
                  tunnel: w507 -> [_ w540]
                  tunnel: w506 -> [_ w539]
                  tunnel: w504 -> [w509 w538]
                  tunnel: w505 -> [_ w537]
                  tunnel: w503 -> [_ w536]
                  tunnel: [w508 w535] -> w502
                  frame False {
                    # "stop test"
                    n358 = stacked-sequence {
                      tunnel: w509 -> [w518 _]
                      tunnel: [w510 _] -> w508
                      frame #0 {
                        n359 = local read "DISP LAB01-2"() -> (w517:T4)
                        n360 = Unbundle(w517) -> ("CYCLE"=w515:dbl, "MINS"=w516:dbl)  [unwired: 1 out]
                        n361 = case shown="\"CHART TEST\", Default" w518 {
                          tunnel: w516 -> [_ _ w525]
                          tunnel: w515 -> [w523 w524 _]
                          tunnel: [w523 w524 w525] -> w514
                          frame "CHART TEST", Default {
                          }
                          frame "CYCLE TEST" {
                          }
                          frame "T-RISE TEST" {
                          }
                        }
                        n362 = local read "TDMS LAB01-2"() -> (w522:refnum<k34>)
                        n363 = Build Array("STOPPED") -> (w519:string[])
                        n364 = Build Array(w514) -> (w513:dbl[])
                        n365 = TDMS Write(0:w522, 5:"TEST RESULT", 7:w519, 9:w513) -> (4:w511:refnum<k34>, 15:w512:errorcluster)  [unwired: 2 in, 2 out]
                        n366 = TDMS Close(8:w512, 11:w511) -> (0:w510:errorcluster)  [unwired: 1 out]
                      }
                      frame #1 {
                        n367 = local read "DISP LAB01-2"() -> (w529:T4)
                        n368 = stacked-sequence {
                          tunnel: "LAB01-2" -> [w531 w533]
                          frame #0 {
                            n369 = call "sub vi - defrag tdms v1.vi"("panel id"=w531) -> ("error out"=w530:errorcluster)  [unwired: 10 in]
                            n370 = local write "data file error"(w530) -> ()
                          }
                          frame #1 {
                            n371 = call "Save data file to network drive v1.vi"("panel id"=w533) -> ("network file save error"=w532:errorcluster)  [unwired: 9 in, 1 out]
                            n372 = local write "RESULT LAB01-2"(FALSE) -> ()
                            n373 = local write "data file error"(w532) -> ()
                          }
                        }
                        n374 = Bundle(cluster=w529, "STATUS"="STOP") -> (w527:T4)  [unwired: 2 in]
                        n375 = local write "DISP LAB01-2"(w527) -> ()
                      }
                    }
                  }
                  frame True {
                    # "start new test and create test file"
                    n376 = stacked-sequence {
                      seq-local: [w541 _ _ _ _] -> [_ w566 _ _ _]
                      tunnel: w540 -> [w546 _ _ _ _]
                      tunnel: w539 -> [w543 _ _ _ _]
                      tunnel: w538 -> [w556 _ _ _ _]
                      tunnel: w537 -> [w549 _ _ _ _]
                      tunnel: w536 -> [w544 _ _ _ _]
                      tunnel: [_ w560 _ _ _] -> w535
                      frame #0 {
                        w542 = "\\"
                        n377 = local read "SET LAB01-2"() -> (w551:T5)
                        n378 = case shown="\"CYCLE TEST\"" w556 {
                          tunnel: ["L01-2-CHART TEST-" "L01-2-CYCLE TEST-" "L01-2-T-RISE TEST-"] -> w552
                          frame "CHART TEST", Default {
                          }
                          frame "CYCLE TEST" {
                          }
                          frame "T-RISE TEST" {
                          }
                        }
                        n379 = Unbundle(w551) -> ("DESCRIPTION"=w550:string)  [unwired: 4 out]
                        n380 = Concatenate Strings(w546, "\\", w544, w542, w543, w542) -> (w553:string)
                        n381 = String To Path(string=w553) -> (path=w555:path)
                        n382 = Concatenate Strings(w553, w552, w550, "-", w549, ".tdms") -> (w541:string)
                        n383 = Create Folder(path (use dialog)=w555) -> (error out=w554:errorcluster)  [unwired: 2 in, 2 out]
                        n384 = global write "Global 1.vi" "LAB01-2 FILE"(w541) -> ()
                        n385 = call <vilib>:"Clear Errors.vi"("error in (no error)"=w554) -> ()  [unwired: 6 in, 1 out]
                      }
                      frame #1 {
                        n386 = String To Path(string=w566) -> (path=w561:path)
                        n387 = TDMS Open(5:FALSE, 6:FALSE, 10:T16."create or replace" ("operation (0:open)"), 11:w561) -> (0:w560:errorcluster, 3:→"TDMS LAB01-2":refnum<k34>)  [unwired: 3 in]
                      }
                      frame #2 {
                        n388 = local read "SET LAB01-2"() -> (w572:T5)
                        n389 = local read "TDMS LAB01-2"() -> (w583:refnum<k34>)
                        n390 = Build Array("Testers Name", "Description", "Set Test Cycles", "T-Rise minutes", "T-Rise Deg C") -> (w573:string[])
                        n391 = Unbundle(w572) -> ("NAME"=w571:string, "DESCRIPTION"=w570:string, "CYCLES"=w569:dbl, "T-RISE mins"=w568:dbl, "T-RISE deg C"=w567:dbl)
                        n392 = Number To Decimal String(number=w569) -> (decimal integer string=w582:string)  [unwired: 1 in]
                        n393 = Number To Decimal String(number=w568) -> (decimal integer string=w581:string)  [unwired: 1 in]
                        n394 = Number To Decimal String(number=w567) -> (decimal integer string=w580:string)  [unwired: 1 in]
                        n395 = Build Array(w571, w570, w582, w581, w580) -> (w579:string[])
                        n396 = TDMS Set Properties(5:w579, 7:w573, 11:w583) -> ()  [unwired: 3 in, 4 out]
                      }
                      frame #3 {
                        w585 = 0.0
                        n397 = local read "DISP LAB01-2"() -> (w587:T4)
                        n398 = Bundle(cluster=w587, "CYCLE"=w585, "MINS"=w585, "STATUS"="RUN") -> (w586:T4)
                        n399 = local write "DISP LAB01-2"(w586) -> ()
                      }
                      frame #4 {
                        n400 = local read "SIG LAB01-2"() -> (w590:T2)
                        n401 = local read "TEMP START LAB01-2"() -> (w592:cluster{"TL":dbl, "TN":dbl})
                        n402 = Unbundle(w590) -> ("Tmp Live"=w589:dbl, "Tmp Neut"=w588:dbl)  [unwired: 3 out]
                        n403 = Bundle(cluster=w592, "TL"=w589, "TN"=w588) -> (w591:cluster{"TL":dbl, "TN":dbl})
                        n404 = local write "TEMP START LAB01-2"(w591) -> ()
                      }
                    }
                  }
                }
              }
              event "RUN LAB02-1": Value Change {
                n405 = event-data() -> ("NewVal"=w593:bool)  [unwired: 1 in, 5 out]
                n406 = local write "run lab02-1"(w593) -> ()
                n407 = case shown="True" w593 {
                  tunnel: w599 -> [_ w632]
                  tunnel: w598 -> [_ w631]
                  tunnel: w596 -> [w601 w630]
                  tunnel: w597 -> [_ w629]
                  tunnel: w595 -> [_ w628]
                  tunnel: [w600 w627] -> w594
                  frame False {
                    # "stop test"
                    n408 = stacked-sequence {
                      tunnel: w601 -> [w610 _]
                      tunnel: [w602 _] -> w600
                      frame #0 {
                        n409 = local read "DISP LAB02-1"() -> (w609:T4)
                        n410 = Unbundle(w609) -> ("CYCLE"=w607:dbl, "MINS"=w608:dbl)  [unwired: 1 out]
                        n411 = case shown="\"CYCLE TEST\"" w610 {
                          tunnel: w608 -> [_ _ w617]
                          tunnel: w607 -> [w615 w616 _]
                          tunnel: [w615 w616 w617] -> w606
                          frame "CHART TEST", Default {
                          }
                          frame "CYCLE TEST" {
                          }
                          frame "T-RISE TEST" {
                          }
                        }
                        n412 = local read "TDMS LAB02-1"() -> (w614:refnum<k34>)
                        n413 = Build Array("STOPPED") -> (w611:string[])
                        n414 = Build Array(w606) -> (w605:dbl[])
                        n415 = TDMS Write(0:w614, 5:"TEST RESULT", 7:w611, 9:w605) -> (4:w603:refnum<k34>, 15:w604:errorcluster)  [unwired: 2 in, 2 out]
                        n416 = TDMS Close(8:w604, 11:w603) -> (0:w602:errorcluster)  [unwired: 1 out]
                      }
                      frame #1 {
                        n417 = local read "DISP LAB02-1"() -> (w621:T4)
                        n418 = stacked-sequence {
                          tunnel: "LAB02-1" -> [w623 w625]
                          frame #0 {
                            n419 = call "sub vi - defrag tdms v1.vi"("panel id"=w623) -> ("error out"=w622:errorcluster)  [unwired: 10 in]
                            n420 = local write "data file error"(w622) -> ()
                          }
                          frame #1 {
                            n421 = local write "RESULT LAB02-1"(FALSE) -> ()
                            n422 = call "Save data file to network drive v1.vi"("panel id"=w625) -> ("network file save error"=w624:errorcluster)  [unwired: 9 in, 1 out]
                            n423 = local write "data file error"(w624) -> ()
                          }
                        }
                        n424 = Bundle(cluster=w621, "STATUS"="STOP") -> (w619:T4)  [unwired: 2 in]
                        n425 = local write "DISP LAB02-1"(w619) -> ()
                      }
                    }
                  }
                  frame True {
                    # "start new test and create test file"
                    n426 = stacked-sequence {
                      seq-local: [w633 _ _ _ _] -> [_ w658 _ _ _]
                      tunnel: w632 -> [w638 _ _ _ _]
                      tunnel: w631 -> [w635 _ _ _ _]
                      tunnel: w630 -> [w648 _ _ _ _]
                      tunnel: w629 -> [w641 _ _ _ _]
                      tunnel: w628 -> [w636 _ _ _ _]
                      tunnel: [_ w652 _ _ _] -> w627
                      frame #0 {
                        w634 = "\\"
                        n427 = local read "SET LAB02-1"() -> (w643:T5)
                        n428 = case shown="\"CYCLE TEST\"" w648 {
                          tunnel: ["L02-1-CHART TEST-" "L02-1-CYCLE TEST-" "L02-1-T-RISE TEST-"] -> w644
                          frame "CHART TEST", Default {
                          }
                          frame "CYCLE TEST" {
                          }
                          frame "T-RISE TEST" {
                          }
                        }
                        n429 = Unbundle(w643) -> ("DESCRIPTION"=w642:string)  [unwired: 4 out]
                        n430 = Concatenate Strings(w638, "\\", w636, w634, w635, w634) -> (w645:string)
                        n431 = String To Path(string=w645) -> (path=w647:path)
                        n432 = Concatenate Strings(w645, w644, w642, "-", w641, ".tdms") -> (w633:string)
                        n433 = Create Folder(path (use dialog)=w647) -> (error out=w646:errorcluster)  [unwired: 2 in, 2 out]
                        n434 = global write "Global 1.vi" "LAB02-1 FILE"(w633) -> ()
                        n435 = call <vilib>:"Clear Errors.vi"("error in (no error)"=w646) -> ()  [unwired: 6 in, 1 out]
                      }
                      frame #1 {
                        n436 = String To Path(string=w658) -> (path=w653:path)
                        n437 = TDMS Open(5:FALSE, 6:FALSE, 10:T16."create or replace" ("operation (0:open)"), 11:w653) -> (0:w652:errorcluster, 3:→"TDMS LAB02-1":refnum<k34>)  [unwired: 3 in]
                      }
                      frame #2 {
                        n438 = local read "SET LAB02-1"() -> (w664:T5)
                        n439 = local read "TDMS LAB02-1"() -> (w675:refnum<k34>)
                        n440 = Build Array("Testers Name", "Description", "Set Test Cycles", "T-Rise minutes", "T-Rise Deg C") -> (w665:string[])
                        n441 = Unbundle(w664) -> ("NAME"=w663:string, "DESCRIPTION"=w662:string, "CYCLES"=w661:dbl, "T-RISE mins"=w660:dbl, "T-RISE deg C"=w659:dbl)
                        n442 = Number To Decimal String(number=w661) -> (decimal integer string=w674:string)  [unwired: 1 in]
                        n443 = Number To Decimal String(number=w660) -> (decimal integer string=w673:string)  [unwired: 1 in]
                        n444 = Number To Decimal String(number=w659) -> (decimal integer string=w672:string)  [unwired: 1 in]
                        n445 = Build Array(w663, w662, w674, w673, w672) -> (w671:string[])
                        n446 = TDMS Set Properties(5:w671, 7:w665, 11:w675) -> ()  [unwired: 3 in, 4 out]
                      }
                      frame #3 {
                        w677 = 0.0
                        n447 = local read "DISP LAB02-1"() -> (w679:T4)
                        n448 = Bundle(cluster=w679, "CYCLE"=w677, "MINS"=w677, "STATUS"="RUN") -> (w678:T4)
                        n449 = local write "DISP LAB02-1"(w678) -> ()
                      }
                      frame #4 {
                        n450 = local read "SIG LAB02-1"() -> (w682:T2)
                        n451 = local read "TEMP START LAB02-1"() -> (w684:cluster{"TL":dbl, "TN":dbl})
                        n452 = Unbundle(w682) -> ("Tmp Live"=w681:dbl, "Tmp Neut"=w680:dbl)  [unwired: 3 out]
                        n453 = Bundle(cluster=w684, "TL"=w681, "TN"=w680) -> (w683:cluster{"TL":dbl, "TN":dbl})
                        n454 = local write "TEMP START LAB02-1"(w683) -> ()
                      }
                    }
                  }
                }
              }
              event "RUN LAB02-2": Value Change {
                n455 = event-data() -> ("NewVal"=w685:bool)  [unwired: 1 in, 5 out]
                n456 = local write "run lab02-2"(w685) -> ()
                n457 = case shown="True" w685 {
                  tunnel: w691 -> [_ w724]
                  tunnel: w690 -> [_ w723]
                  tunnel: w688 -> [w693 w722]
                  tunnel: w689 -> [_ w721]
                  tunnel: w687 -> [_ w720]
                  tunnel: [w692 w719] -> w686
                  frame False {
                    # "stop test"
                    n458 = stacked-sequence {
                      tunnel: w693 -> [w702 _]
                      tunnel: [w694 _] -> w692
                      frame #0 {
                        n459 = local read "DISP LAB02-2"() -> (w701:T4)
                        n460 = Unbundle(w701) -> ("CYCLE"=w699:dbl, "MINS"=w700:dbl)  [unwired: 1 out]
                        n461 = case shown="\"CYCLE TEST\"" w702 {
                          tunnel: w700 -> [_ _ w709]
                          tunnel: w699 -> [w707 w708 _]
                          tunnel: [w707 w708 w709] -> w698
                          frame "CHART TEST", Default {
                          }
                          frame "CYCLE TEST" {
                          }
                          frame "T-RISE TEST" {
                          }
                        }
                        n462 = local read "TDMS LAB02-2"() -> (w706:refnum<k34>)
                        n463 = Build Array("STOPPED") -> (w703:string[])
                        n464 = Build Array(w698) -> (w697:dbl[])
                        n465 = TDMS Write(0:w706, 5:"TEST RESULT", 7:w703, 9:w697) -> (4:w695:refnum<k34>, 15:w696:errorcluster)  [unwired: 2 in, 2 out]
                        n466 = TDMS Close(8:w696, 11:w695) -> (0:w694:errorcluster)  [unwired: 1 out]
                      }
                      frame #1 {
                        n467 = local read "DISP LAB02-2"() -> (w713:T4)
                        n468 = stacked-sequence {
                          tunnel: "LAB02-2" -> [w715 w717]
                          frame #0 {
                            n469 = call "sub vi - defrag tdms v1.vi"("panel id"=w715) -> ("error out"=w714:errorcluster)  [unwired: 10 in]
                            n470 = local write "data file error"(w714) -> ()
                          }
                          frame #1 {
                            n471 = call "Save data file to network drive v1.vi"("panel id"=w717) -> ("network file save error"=w716:errorcluster)  [unwired: 9 in, 1 out]
                            n472 = local write "RESULT LAB02-2"(FALSE) -> ()
                            n473 = local write "data file error"(w716) -> ()
                          }
                        }
                        n474 = Bundle(cluster=w713, "STATUS"="STOP") -> (w711:T4)  [unwired: 2 in]
                        n475 = local write "DISP LAB02-2"(w711) -> ()
                      }
                    }
                  }
                  frame True {
                    # "start new test and create test file"
                    n476 = stacked-sequence {
                      seq-local: [w725 _ _ _ _] -> [_ w750 _ _ _]
                      tunnel: w724 -> [w730 _ _ _ _]
                      tunnel: w723 -> [w727 _ _ _ _]
                      tunnel: w722 -> [w740 _ _ _ _]
                      tunnel: w721 -> [w733 _ _ _ _]
                      tunnel: w720 -> [w728 _ _ _ _]
                      tunnel: [_ w744 _ _ _] -> w719
                      frame #0 {
                        w726 = "\\"
                        n477 = local read "SET LAB02-2"() -> (w735:T5)
                        n478 = case shown="\"CYCLE TEST\"" w740 {
                          tunnel: ["L02-2-CHART TEST-" "L02-2-CYCLE TEST-" "L02-2-T-RISE TEST-"] -> w736
                          frame "CHART TEST", Default {
                          }
                          frame "CYCLE TEST" {
                          }
                          frame "T-RISE TEST" {
                          }
                        }
                        n479 = Unbundle(w735) -> ("DESCRIPTION"=w734:string)  [unwired: 4 out]
                        n480 = Concatenate Strings(w730, "\\", w728, w726, w727, w726) -> (w737:string)
                        n481 = String To Path(string=w737) -> (path=w739:path)
                        n482 = Concatenate Strings(w737, w736, w734, "-", w733, ".tdms") -> (w725:string)
                        n483 = Create Folder(path (use dialog)=w739) -> (error out=w738:errorcluster)  [unwired: 2 in, 2 out]
                        n484 = global write "Global 1.vi" "LAB02-2 FILE"(w725) -> ()
                        n485 = call <vilib>:"Clear Errors.vi"("error in (no error)"=w738) -> ()  [unwired: 6 in, 1 out]
                      }
                      frame #1 {
                        n486 = String To Path(string=w750) -> (path=w745:path)
                        n487 = TDMS Open(5:FALSE, 6:FALSE, 10:T16."create or replace" ("operation (0:open)"), 11:w745) -> (0:w744:errorcluster, 3:→"TDMS LAB02-2":refnum<k34>)  [unwired: 3 in]
                      }
                      frame #2 {
                        n488 = local read "SET LAB02-2"() -> (w756:T5)
                        n489 = local read "TDMS LAB02-2"() -> (w767:refnum<k34>)
                        n490 = Build Array("Testers Name", "Description", "Set Test Cycles", "T-Rise minutes", "T-Rise Deg C") -> (w757:string[])
                        n491 = Unbundle(w756) -> ("NAME"=w755:string, "DESCRIPTION"=w754:string, "CYCLES"=w753:dbl, "T-RISE mins"=w752:dbl, "T-RISE deg C"=w751:dbl)
                        n492 = Number To Decimal String(number=w753) -> (decimal integer string=w766:string)  [unwired: 1 in]
                        n493 = Number To Decimal String(number=w752) -> (decimal integer string=w765:string)  [unwired: 1 in]
                        n494 = Number To Decimal String(number=w751) -> (decimal integer string=w764:string)  [unwired: 1 in]
                        n495 = Build Array(w755, w754, w766, w765, w764) -> (w763:string[])
                        n496 = TDMS Set Properties(5:w763, 7:w757, 11:w767) -> ()  [unwired: 3 in, 4 out]
                      }
                      frame #3 {
                        w769 = 0.0
                        n497 = local read "DISP LAB02-2"() -> (w771:T4)
                        n498 = Bundle(cluster=w771, "CYCLE"=w769, "MINS"=w769, "STATUS"="RUN") -> (w770:T4)
                        n499 = local write "DISP LAB02-2"(w770) -> ()
                      }
                      frame #4 {
                        n500 = local read "SIG LAB02-2"() -> (w774:T2)
                        n501 = local read "TEMP START LAB02-2"() -> (w776:cluster{"TL":dbl, "TN":dbl})
                        n502 = Unbundle(w774) -> ("Tmp Live"=w773:dbl, "Tmp Neut"=w772:dbl)  [unwired: 3 out]
                        n503 = Bundle(cluster=w776, "TL"=w773, "TN"=w772) -> (w775:cluster{"TL":dbl, "TN":dbl})
                        n504 = local write "TEMP START LAB02-2"(w775) -> ()
                      }
                    }
                  }
                }
              }
              event "RUN LAB03-1": Value Change {
                n505 = event-data() -> ("NewVal"=w777:bool)  [unwired: 1 in, 5 out]
                n506 = local write "run lab03-1"(w777) -> ()
                n507 = case shown="True" w777 {
                  tunnel: w783 -> [_ w816]
                  tunnel: w782 -> [_ w815]
                  tunnel: w780 -> [w785 w814]
                  tunnel: w781 -> [_ w813]
                  tunnel: w779 -> [_ w812]
                  tunnel: [w784 w811] -> w778
                  frame False {
                    # "stop test"
                    n508 = stacked-sequence {
                      tunnel: w785 -> [w794 _]
                      tunnel: [w786 _] -> w784
                      frame #0 {
                        n509 = local read "DISP LAB03-1"() -> (w793:T4)
                        n510 = Unbundle(w793) -> ("CYCLE"=w791:dbl, "MINS"=w792:dbl)  [unwired: 1 out]
                        n511 = case shown="\"CYCLE TEST\"" w794 {
                          tunnel: w792 -> [_ _ w801]
                          tunnel: w791 -> [w799 w800 _]
                          tunnel: [w799 w800 w801] -> w790
                          frame "CHART TEST", Default {
                          }
                          frame "CYCLE TEST" {
                          }
                          frame "T-RISE TEST" {
                          }
                        }
                        n512 = local read "TDMS LAB03-1"() -> (w798:refnum<k34>)
                        n513 = Build Array("STOPPED") -> (w795:string[])
                        n514 = Build Array(w790) -> (w789:dbl[])
                        n515 = TDMS Write(0:w798, 5:"TEST RESULT", 7:w795, 9:w789) -> (4:w787:refnum<k34>, 15:w788:errorcluster)  [unwired: 2 in, 2 out]
                        n516 = TDMS Close(8:w788, 11:w787) -> (0:w786:errorcluster)  [unwired: 1 out]
                      }
                      frame #1 {
                        n517 = local read "DISP LAB03-1"() -> (w805:T4)
                        n518 = stacked-sequence {
                          tunnel: "LAB03-1" -> [w807 w809]
                          frame #0 {
                            n519 = call "sub vi - defrag tdms v1.vi"("panel id"=w807) -> ("error out"=w806:errorcluster)  [unwired: 10 in]
                            n520 = local write "data file error"(w806) -> ()
                          }
                          frame #1 {
                            n521 = call "Save data file to network drive v1.vi"("panel id"=w809) -> ("network file save error"=w808:errorcluster)  [unwired: 9 in, 1 out]
                            n522 = local write "RESULT LAB03-1"(FALSE) -> ()
                            n523 = local write "data file error"(w808) -> ()
                          }
                        }
                        n524 = Bundle(cluster=w805, "STATUS"="STOP") -> (w803:T4)  [unwired: 2 in]
                        n525 = local write "DISP LAB03-1"(w803) -> ()
                      }
                    }
                  }
                  frame True {
                    # "start new test and create test file"
                    n526 = stacked-sequence {
                      seq-local: [w817 _ _ _ _] -> [_ w842 _ _ _]
                      tunnel: w816 -> [w822 _ _ _ _]
                      tunnel: w815 -> [w819 _ _ _ _]
                      tunnel: w814 -> [w832 _ _ _ _]
                      tunnel: w813 -> [w825 _ _ _ _]
                      tunnel: w812 -> [w820 _ _ _ _]
                      tunnel: [_ w836 _ _ _] -> w811
                      frame #0 {
                        w818 = "\\"
                        n527 = local read "SET LAB03-1"() -> (w827:T5)
                        n528 = case shown="\"T-RISE TEST\"" w832 {
                          tunnel: ["L03-1-CHART TEST-" "L03-1-CYCLE TEST-" "L03-1-T-RISE TEST-"] -> w828
                          frame "CHART TEST", Default {
                          }
                          frame "CYCLE TEST" {
                          }
                          frame "T-RISE TEST" {
                          }
                        }
                        n529 = Unbundle(w827) -> ("DESCRIPTION"=w826:string)  [unwired: 4 out]
                        n530 = Concatenate Strings(w822, "\\", w820, w818, w819, w818) -> (w829:string)
                        n531 = String To Path(string=w829) -> (path=w831:path)
                        n532 = Concatenate Strings(w829, w828, w826, "-", w825, ".tdms") -> (w817:string)
                        n533 = Create Folder(path (use dialog)=w831) -> (error out=w830:errorcluster)  [unwired: 2 in, 2 out]
                        n534 = global write "Global 1.vi" "LAB03-1 FILE"(w817) -> ()
                        n535 = call <vilib>:"Clear Errors.vi"("error in (no error)"=w830) -> ()  [unwired: 6 in, 1 out]
                      }
                      frame #1 {
                        n536 = String To Path(string=w842) -> (path=w837:path)
                        n537 = TDMS Open(5:FALSE, 6:FALSE, 10:T16."create or replace" ("operation (0:open)"), 11:w837) -> (0:w836:errorcluster, 3:→"TDMS LAB03-1":refnum<k34>)  [unwired: 3 in]
                      }
                      frame #2 {
                        n538 = local read "SET LAB03-1"() -> (w848:T5)
                        n539 = local read "TDMS LAB03-1"() -> (w859:refnum<k34>)
                        n540 = Build Array("Testers Name", "Description", "Set Test Cycles", "T-Rise minutes", "T-Rise Deg C") -> (w849:string[])
                        n541 = Unbundle(w848) -> ("NAME"=w847:string, "DESCRIPTION"=w846:string, "CYCLES"=w845:dbl, "T-RISE mins"=w844:dbl, "T-RISE deg C"=w843:dbl)
                        n542 = Number To Decimal String(number=w845) -> (decimal integer string=w858:string)  [unwired: 1 in]
                        n543 = Number To Decimal String(number=w844) -> (decimal integer string=w857:string)  [unwired: 1 in]
                        n544 = Number To Decimal String(number=w843) -> (decimal integer string=w856:string)  [unwired: 1 in]
                        n545 = Build Array(w847, w846, w858, w857, w856) -> (w855:string[])
                        n546 = TDMS Set Properties(5:w855, 7:w849, 11:w859) -> ()  [unwired: 3 in, 4 out]
                      }
                      frame #3 {
                        w861 = 0.0
                        n547 = local read "DISP LAB03-1"() -> (w863:T4)
                        n548 = Bundle(cluster=w863, "CYCLE"=w861, "MINS"=w861, "STATUS"="RUN") -> (w862:T4)
                        n549 = local write "DISP LAB03-1"(w862) -> ()
                      }
                      frame #4 {
                        n550 = local read "SIG LAB03-1"() -> (w866:T2)
                        n551 = local read "TEMP START LAB03-1"() -> (w868:cluster{"TL":dbl, "TN":dbl})
                        n552 = Unbundle(w866) -> ("Tmp Live"=w865:dbl, "Tmp Neut"=w864:dbl)  [unwired: 3 out]
                        n553 = Bundle(cluster=w868, "TL"=w865, "TN"=w864) -> (w867:cluster{"TL":dbl, "TN":dbl})
                        n554 = local write "TEMP START LAB03-1"(w867) -> ()
                      }
                    }
                  }
                }
              }
              event "RUN LAB03-2": Value Change {
                n555 = event-data() -> ("NewVal"=w869:bool)  [unwired: 1 in, 5 out]
                n556 = local write "run lab03-2"(w869) -> ()
                n557 = case shown="True" w869 {
                  tunnel: w875 -> [_ w908]
                  tunnel: w874 -> [_ w907]
                  tunnel: w872 -> [w877 w906]
                  tunnel: w873 -> [_ w905]
                  tunnel: w871 -> [_ w904]
                  tunnel: [w876 w903] -> w870
                  frame False {
                    # "stop test"
                    n558 = stacked-sequence {
                      tunnel: w877 -> [w886 _]
                      tunnel: [w878 _] -> w876
                      frame #0 {
                        n559 = local read "DISP LAB03-2"() -> (w885:T4)
                        n560 = Unbundle(w885) -> ("CYCLE"=w883:dbl, "MINS"=w884:dbl)  [unwired: 1 out]
                        n561 = case shown="\"CYCLE TEST\"" w886 {
                          tunnel: w884 -> [_ _ w893]
                          tunnel: w883 -> [w891 w892 _]
                          tunnel: [w891 w892 w893] -> w882
                          frame "CHART TEST", Default {
                          }
                          frame "CYCLE TEST" {
                          }
                          frame "T-RISE TEST" {
                          }
                        }
                        n562 = local read "TDMS LAB03-2"() -> (w890:refnum<k34>)
                        n563 = Build Array("STOPPED") -> (w887:string[])
                        n564 = Build Array(w882) -> (w881:dbl[])
                        n565 = TDMS Write(0:w890, 5:"TEST RESULT", 7:w887, 9:w881) -> (4:w879:refnum<k34>, 15:w880:errorcluster)  [unwired: 2 in, 2 out]
                        n566 = TDMS Close(8:w880, 11:w879) -> (0:w878:errorcluster)  [unwired: 1 out]
                      }
                      frame #1 {
                        n567 = local read "DISP LAB03-2"() -> (w897:T4)
                        n568 = stacked-sequence {
                          tunnel: "LAB03-2" -> [w899 w901]
                          frame #0 {
                            n569 = call "sub vi - defrag tdms v1.vi"("panel id"=w899) -> ("error out"=w898:errorcluster)  [unwired: 10 in]
                            n570 = local write "data file error"(w898) -> ()
                          }
                          frame #1 {
                            n571 = call "Save data file to network drive v1.vi"("panel id"=w901) -> ("network file save error"=w900:errorcluster)  [unwired: 9 in, 1 out]
                            n572 = local write "RESULT LAB03-2"(FALSE) -> ()
                            n573 = local write "data file error"(w900) -> ()
                          }
                        }
                        n574 = Bundle(cluster=w897, "STATUS"="STOP") -> (w895:T4)  [unwired: 2 in]
                        n575 = local write "DISP LAB03-2"(w895) -> ()
                      }
                    }
                  }
                  frame True {
                    # "start new test and create test file"
                    n576 = stacked-sequence {
                      seq-local: [w909 _ _ _ _] -> [_ w934 _ _ _]
                      tunnel: w908 -> [w914 _ _ _ _]
                      tunnel: w907 -> [w911 _ _ _ _]
                      tunnel: w906 -> [w924 _ _ _ _]
                      tunnel: w905 -> [w917 _ _ _ _]
                      tunnel: w904 -> [w912 _ _ _ _]
                      tunnel: [_ w928 _ _ _] -> w903
                      frame #0 {
                        w910 = "\\"
                        n577 = local read "SET LAB03-2"() -> (w919:T5)
                        n578 = case shown="\"T-RISE TEST\"" w924 {
                          tunnel: ["L03-2-CHART TEST-" "L03-2-CYCLE TEST-" "L03-2-T-RISE TEST-"] -> w920
                          frame "CHART TEST", Default {
                          }
                          frame "CYCLE TEST" {
                          }
                          frame "T-RISE TEST" {
                          }
                        }
                        n579 = Unbundle(w919) -> ("DESCRIPTION"=w918:string)  [unwired: 4 out]
                        n580 = Concatenate Strings(w914, "\\", w912, w910, w911, w910) -> (w921:string)
                        n581 = String To Path(string=w921) -> (path=w923:path)
                        n582 = Concatenate Strings(w921, w920, w918, "-", w917, ".tdms") -> (w909:string)
                        n583 = Create Folder(path (use dialog)=w923) -> (error out=w922:errorcluster)  [unwired: 2 in, 2 out]
                        n584 = global write "Global 1.vi" "LAB03-2 FILE"(w909) -> ()
                        n585 = call <vilib>:"Clear Errors.vi"("error in (no error)"=w922) -> ()  [unwired: 6 in, 1 out]
                      }
                      frame #1 {
                        n586 = String To Path(string=w934) -> (path=w929:path)
                        n587 = TDMS Open(5:FALSE, 6:FALSE, 10:T16."create or replace" ("operation (0:open)"), 11:w929) -> (0:w928:errorcluster, 3:→"TDMS LAB03-2":refnum<k34>)  [unwired: 3 in]
                      }
                      frame #2 {
                        n588 = local read "SET LAB03-2"() -> (w940:T5)
                        n589 = local read "TDMS LAB03-2"() -> (w951:refnum<k34>)
                        n590 = Build Array("Testers Name", "Description", "Set Test Cycles", "T-Rise minutes", "T-Rise Deg C") -> (w941:string[])
                        n591 = Unbundle(w940) -> ("NAME"=w939:string, "DESCRIPTION"=w938:string, "CYCLES"=w937:dbl, "T-RISE mins"=w936:dbl, "T-RISE deg C"=w935:dbl)
                        n592 = Number To Decimal String(number=w937) -> (decimal integer string=w950:string)  [unwired: 1 in]
                        n593 = Number To Decimal String(number=w936) -> (decimal integer string=w949:string)  [unwired: 1 in]
                        n594 = Number To Decimal String(number=w935) -> (decimal integer string=w948:string)  [unwired: 1 in]
                        n595 = Build Array(w939, w938, w950, w949, w948) -> (w947:string[])
                        n596 = TDMS Set Properties(5:w947, 7:w941, 11:w951) -> ()  [unwired: 3 in, 4 out]
                      }
                      frame #3 {
                        w953 = 0.0
                        n597 = local read "DISP LAB03-2"() -> (w955:T4)
                        n598 = Bundle(cluster=w955, "CYCLE"=w953, "MINS"=w953, "STATUS"="RUN") -> (w954:T4)
                        n599 = local write "DISP LAB03-2"(w954) -> ()
                      }
                      frame #4 {
                        n600 = local read "SIG LAB03-2"() -> (w958:T2)
                        n601 = local read "TEMP START LAB03-2"() -> (w960:cluster{"TL":dbl, "TN":dbl})
                        n602 = Unbundle(w958) -> ("Tmp Live"=w957:dbl, "Tmp Neut"=w956:dbl)  [unwired: 3 out]
                        n603 = Bundle(cluster=w960, "TL"=w957, "TN"=w956) -> (w959:cluster{"TL":dbl, "TN":dbl})
                        n604 = local write "TEMP START LAB03-2"(w959) -> ()
                      }
                    }
                  }
                }
              }
              event "RUN LAB04-1": Value Change {
                n605 = event-data() -> ("NewVal"=w961:bool)  [unwired: 1 in, 5 out]
                n606 = local write "run lab04-1"(w961) -> ()
                n607 = case shown="True" w961 {
                  tunnel: w967 -> [_ w1000]
                  tunnel: w966 -> [_ w999]
                  tunnel: w964 -> [w969 w998]
                  tunnel: w965 -> [_ w997]
                  tunnel: w963 -> [_ w996]
                  tunnel: [w968 w995] -> w962
                  frame False {
                    # "stop test"
                    n608 = stacked-sequence {
                      tunnel: w969 -> [w978 _]
                      tunnel: [w970 _] -> w968
                      frame #0 {
                        n609 = local read "DISP LAB04-1"() -> (w977:T4)
                        n610 = Unbundle(w977) -> ("CYCLE"=w975:dbl, "MINS"=w976:dbl)  [unwired: 1 out]
                        n611 = case shown="\"CYCLE TEST\"" w978 {
                          tunnel: w976 -> [_ _ w985]
                          tunnel: w975 -> [w983 w984 _]
                          tunnel: [w983 w984 w985] -> w974
                          frame "CHART TEST", Default {
                          }
                          frame "CYCLE TEST" {
                          }
                          frame "T-RISE TEST" {
                          }
                        }
                        n612 = local read "TDMS LAB04-1"() -> (w982:refnum<k34>)
                        n613 = Build Array("STOPPED") -> (w979:string[])
                        n614 = Build Array(w974) -> (w973:dbl[])
                        n615 = TDMS Write(0:w982, 5:"TEST RESULT", 7:w979, 9:w973) -> (4:w971:refnum<k34>, 15:w972:errorcluster)  [unwired: 2 in, 2 out]
                        n616 = TDMS Close(8:w972, 11:w971) -> (0:w970:errorcluster)  [unwired: 1 out]
                      }
                      frame #1 {
                        n617 = local read "DISP LAB04-1"() -> (w989:T4)
                        n618 = stacked-sequence {
                          tunnel: "LAB04-1" -> [w991 w993]
                          frame #0 {
                            n619 = call "sub vi - defrag tdms v1.vi"("panel id"=w991) -> ("error out"=w990:errorcluster)  [unwired: 10 in]
                            n620 = local write "data file error"(w990) -> ()
                          }
                          frame #1 {
                            n621 = call "Save data file to network drive v1.vi"("panel id"=w993) -> ("network file save error"=w992:errorcluster)  [unwired: 9 in, 1 out]
                            n622 = local write "RESULT LAB04-1"(FALSE) -> ()
                            n623 = local write "data file error"(w992) -> ()
                          }
                        }
                        n624 = Bundle(cluster=w989, "STATUS"="STOP") -> (w987:T4)  [unwired: 2 in]
                        n625 = local write "DISP LAB04-1"(w987) -> ()
                      }
                    }
                  }
                  frame True {
                    # "start new test and create test file"
                    n626 = stacked-sequence {
                      seq-local: [w1001 _ _ _ _] -> [_ w1026 _ _ _]
                      tunnel: w1000 -> [w1006 _ _ _ _]
                      tunnel: w999 -> [w1002 _ _ _ _]
                      tunnel: w998 -> [w1016 _ _ _ _]
                      tunnel: w997 -> [w1009 _ _ _ _]
                      tunnel: w996 -> [w1004 _ _ _ _]
                      tunnel: [_ w1020 _ _ _] -> w995
                      frame #0 {
                        w1003 = "\\"
                        n627 = local read "SET LAB04-1"() -> (w1011:T5)
                        n628 = case shown="\"CYCLE TEST\"" w1016 {
                          tunnel: ["L04-1-CHART TEST-" "L04-1-CYCLE TEST-" "L04-1-T-RISE TEST-"] -> w1012
                          frame "CHART TEST", Default {
                          }
                          frame "CYCLE TEST" {
                          }
                          frame "T-RISE TEST" {
                          }
                        }
                        n629 = Unbundle(w1011) -> ("DESCRIPTION"=w1010:string)  [unwired: 4 out]
                        n630 = Concatenate Strings(w1006, "\\", w1004, w1003, w1002, w1003) -> (w1013:string)
                        n631 = String To Path(string=w1013) -> (path=w1015:path)
                        n632 = Concatenate Strings(w1013, w1012, w1010, "-", w1009, ".tdms") -> (w1001:string)
                        n633 = Create Folder(path (use dialog)=w1015) -> (error out=w1014:errorcluster)  [unwired: 2 in, 2 out]
                        n634 = global write "Global 1.vi" "LAB04-1 FILE"(w1001) -> ()
                        n635 = call <vilib>:"Clear Errors.vi"("error in (no error)"=w1014) -> ()  [unwired: 6 in, 1 out]
                      }
                      frame #1 {
                        n636 = String To Path(string=w1026) -> (path=w1021:path)
                        n637 = TDMS Open(5:FALSE, 6:FALSE, 10:T16."create or replace" ("operation (0:open)"), 11:w1021) -> (0:w1020:errorcluster, 3:→"TDMS LAB04-1":refnum<k34>)  [unwired: 3 in]
                      }
                      frame #2 {
                        n638 = local read "SET LAB04-1"() -> (w1032:T5)
                        n639 = local read "TDMS LAB04-1"() -> (w1043:refnum<k34>)
                        n640 = Build Array("Testers Name", "Description", "Set Test Cycles", "T-Rise minutes", "T-Rise Deg C") -> (w1033:string[])
                        n641 = Unbundle(w1032) -> ("NAME"=w1031:string, "DESCRIPTION"=w1030:string, "CYCLES"=w1029:dbl, "T-RISE mins"=w1028:dbl, "T-RISE deg C"=w1027:dbl)
                        n642 = Number To Decimal String(number=w1029) -> (decimal integer string=w1042:string)  [unwired: 1 in]
                        n643 = Number To Decimal String(number=w1028) -> (decimal integer string=w1041:string)  [unwired: 1 in]
                        n644 = Number To Decimal String(number=w1027) -> (decimal integer string=w1040:string)  [unwired: 1 in]
                        n645 = Build Array(w1031, w1030, w1042, w1041, w1040) -> (w1039:string[])
                        n646 = TDMS Set Properties(5:w1039, 7:w1033, 11:w1043) -> ()  [unwired: 3 in, 4 out]
                      }
                      frame #3 {
                        w1045 = 0.0
                        n647 = local read "DISP LAB04-1"() -> (w1047:T4)
                        n648 = Bundle(cluster=w1047, "CYCLE"=w1045, "MINS"=w1045, "STATUS"="RUN") -> (w1046:T4)
                        n649 = local write "DISP LAB04-1"(w1046) -> ()
                      }
                      frame #4 {
                        n650 = local read "SIG LAB04-1"() -> (w1050:T2)
                        n651 = local read "TEMP START LAB04-1"() -> (w1052:cluster{"TL":dbl, "TN":dbl})
                        n652 = Unbundle(w1050) -> ("Tmp Live"=w1049:dbl, "Tmp Neut"=w1048:dbl)  [unwired: 3 out]
                        n653 = Bundle(cluster=w1052, "TL"=w1049, "TN"=w1048) -> (w1051:cluster{"TL":dbl, "TN":dbl})
                        n654 = local write "TEMP START LAB04-1"(w1051) -> ()
                      }
                    }
                  }
                }
              }
              event "RUN LAB04-2": Value Change {
                n655 = event-data() -> ("NewVal"=w1053:bool)  [unwired: 1 in, 5 out]
                n656 = local write "run lab04-2"(w1053) -> ()
                n657 = case shown="True" w1053 {
                  tunnel: w1059 -> [_ w1092]
                  tunnel: w1058 -> [_ w1091]
                  tunnel: w1056 -> [w1061 w1090]
                  tunnel: w1057 -> [_ w1089]
                  tunnel: w1055 -> [_ w1088]
                  tunnel: [w1060 w1087] -> w1054
                  frame False {
                    # "stop test"
                    n658 = stacked-sequence {
                      tunnel: w1061 -> [w1070 _]
                      tunnel: [w1062 _] -> w1060
                      frame #0 {
                        n659 = local read "DISP LAB04-2"() -> (w1069:T4)
                        n660 = Unbundle(w1069) -> ("CYCLE"=w1067:dbl, "MINS"=w1068:dbl)  [unwired: 1 out]
                        n661 = case shown="\"CYCLE TEST\"" w1070 {
                          tunnel: w1068 -> [_ _ w1077]
                          tunnel: w1067 -> [w1075 w1076 _]
                          tunnel: [w1075 w1076 w1077] -> w1066
                          frame "CHART TEST", Default {
                          }
                          frame "CYCLE TEST" {
                          }
                          frame "T-RISE TEST" {
                          }
                        }
                        n662 = local read "TDMS LAB04-2"() -> (w1074:refnum<k34>)
                        n663 = Build Array("STOPPED") -> (w1071:string[])
                        n664 = Build Array(w1066) -> (w1065:dbl[])
                        n665 = TDMS Write(0:w1074, 5:"TEST RESULT", 7:w1071, 9:w1065) -> (4:w1063:refnum<k34>, 15:w1064:errorcluster)  [unwired: 2 in, 2 out]
                        n666 = TDMS Close(8:w1064, 11:w1063) -> (0:w1062:errorcluster)  [unwired: 1 out]
                      }
                      frame #1 {
                        n667 = local read "DISP LAB04-2"() -> (w1081:T4)
                        n668 = stacked-sequence {
                          tunnel: "LAB04-2" -> [w1083 w1085]
                          frame #0 {
                            n669 = call "sub vi - defrag tdms v1.vi"("panel id"=w1083) -> ("error out"=w1082:errorcluster)  [unwired: 10 in]
                            n670 = local write "data file error"(w1082) -> ()
                          }
                          frame #1 {
                            n671 = call "Save data file to network drive v1.vi"("panel id"=w1085) -> ("network file save error"=w1084:errorcluster)  [unwired: 9 in, 1 out]
                            n672 = local write "RESULT LAB04-2"(FALSE) -> ()
                            n673 = local write "data file error"(w1084) -> ()
                          }
                        }
                        n674 = Bundle(cluster=w1081, "STATUS"="STOP") -> (w1079:T4)  [unwired: 2 in]
                        n675 = local write "DISP LAB04-2"(w1079) -> ()
                      }
                    }
                  }
                  frame True {
                    # "start new test and create test file"
                    n676 = stacked-sequence {
                      seq-local: [w1093 _ _ _ _] -> [_ w1118 _ _ _]
                      tunnel: w1092 -> [w1098 _ _ _ _]
                      tunnel: w1091 -> [w1094 _ _ _ _]
                      tunnel: w1090 -> [w1108 _ _ _ _]
                      tunnel: w1089 -> [w1101 _ _ _ _]
                      tunnel: w1088 -> [w1096 _ _ _ _]
                      tunnel: [_ w1112 _ _ _] -> w1087
                      frame #0 {
                        w1095 = "\\"
                        n677 = local read "SET LAB04-2"() -> (w1103:T5)
                        n678 = case shown="\"CHART TEST\", Default" w1108 {
                          tunnel: ["L04-2-CHART TEST-" "L04-2-CYCLE TEST-" "L04-2-T-RISE TEST-"] -> w1104
                          frame "CHART TEST", Default {
                          }
                          frame "CYCLE TEST" {
                          }
                          frame "T-RISE TEST" {
                          }
                        }
                        n679 = Unbundle(w1103) -> ("DESCRIPTION"=w1102:string)  [unwired: 4 out]
                        n680 = Concatenate Strings(w1098, "\\", w1096, w1095, w1094, w1095) -> (w1105:string)
                        n681 = String To Path(string=w1105) -> (path=w1107:path)
                        n682 = Concatenate Strings(w1105, w1104, w1102, "-", w1101, ".tdms") -> (w1093:string)
                        n683 = Create Folder(path (use dialog)=w1107) -> (error out=w1106:errorcluster)  [unwired: 2 in, 2 out]
                        n684 = global write "Global 1.vi" "LAB04-2 FILE"(w1093) -> ()
                        n685 = call <vilib>:"Clear Errors.vi"("error in (no error)"=w1106) -> ()  [unwired: 6 in, 1 out]
                      }
                      frame #1 {
                        n686 = String To Path(string=w1118) -> (path=w1113:path)
                        n687 = TDMS Open(5:FALSE, 6:FALSE, 10:T16."create or replace" ("operation (0:open)"), 11:w1113) -> (0:w1112:errorcluster, 3:→"TDMS LAB04-2":refnum<k34>)  [unwired: 3 in]
                      }
                      frame #2 {
                        n688 = local read "SET LAB04-2"() -> (w1124:T5)
                        n689 = local read "TDMS LAB04-2"() -> (w1135:refnum<k34>)
                        n690 = Build Array("Testers Name", "Description", "Set Test Cycles", "T-Rise minutes", "T-Rise Deg C") -> (w1125:string[])
                        n691 = Unbundle(w1124) -> ("NAME"=w1123:string, "DESCRIPTION"=w1122:string, "CYCLES"=w1121:dbl, "T-RISE mins"=w1120:dbl, "T-RISE deg C"=w1119:dbl)
                        n692 = Number To Decimal String(number=w1121) -> (decimal integer string=w1134:string)  [unwired: 1 in]
                        n693 = Number To Decimal String(number=w1120) -> (decimal integer string=w1133:string)  [unwired: 1 in]
                        n694 = Number To Decimal String(number=w1119) -> (decimal integer string=w1132:string)  [unwired: 1 in]
                        n695 = Build Array(w1123, w1122, w1134, w1133, w1132) -> (w1131:string[])
                        n696 = TDMS Set Properties(5:w1131, 7:w1125, 11:w1135) -> ()  [unwired: 3 in, 4 out]
                      }
                      frame #3 {
                        w1137 = 0.0
                        n697 = local read "DISP LAB04-2"() -> (w1139:T4)
                        n698 = Bundle(cluster=w1139, "CYCLE"=w1137, "MINS"=w1137, "STATUS"="RUN") -> (w1138:T4)
                        n699 = local write "DISP LAB04-2"(w1138) -> ()
                      }
                      frame #4 {
                        n700 = local read "SIG LAB04-2"() -> (w1142:T2)
                        n701 = local read "TEMP START LAB04-2"() -> (w1144:cluster{"TL":dbl, "TN":dbl})
                        n702 = Unbundle(w1142) -> ("Tmp Live"=w1141:dbl, "Tmp Neut"=w1140:dbl)  [unwired: 3 out]
                        n703 = Bundle(cluster=w1144, "TL"=w1141, "TN"=w1140) -> (w1143:cluster{"TL":dbl, "TN":dbl})
                        n704 = local write "TEMP START LAB04-2"(w1143) -> ()
                      }
                    }
                  }
                }
              }
              event "RUN LAB05-1": Value Change {
                n705 = event-data() -> ("NewVal"=w1145:bool)  [unwired: 1 in, 5 out]
                n706 = local write "run lab05-1"(w1145) -> ()
                n707 = case shown="True" w1145 {
                  tunnel: w1151 -> [_ w1184]
                  tunnel: w1150 -> [_ w1183]
                  tunnel: w1148 -> [w1153 w1182]
                  tunnel: w1149 -> [_ w1181]
                  tunnel: w1147 -> [_ w1180]
                  tunnel: [w1152 w1179] -> w1146
                  frame False {
                    # "stop test"
                    n708 = stacked-sequence {
                      tunnel: w1153 -> [w1162 _]
                      tunnel: [w1154 _] -> w1152
                      frame #0 {
                        n709 = local read "DISP LAB05-1"() -> (w1161:T4)
                        n710 = Unbundle(w1161) -> ("CYCLE"=w1159:dbl, "MINS"=w1160:dbl)  [unwired: 1 out]
                        n711 = case shown="\"CYCLE TEST\"" w1162 {
                          tunnel: w1160 -> [_ _ w1169]
                          tunnel: w1159 -> [w1167 w1168 _]
                          tunnel: [w1167 w1168 w1169] -> w1158
                          frame "CHART TEST", Default {
                          }
                          frame "CYCLE TEST" {
                          }
                          frame "T-RISE TEST" {
                          }
                        }
                        n712 = local read "TDMS LAB05-1"() -> (w1166:refnum<k34>)
                        n713 = Build Array("STOPPED") -> (w1163:string[])
                        n714 = Build Array(w1158) -> (w1157:dbl[])
                        n715 = TDMS Write(0:w1166, 5:"TEST RESULT", 7:w1163, 9:w1157) -> (4:w1155:refnum<k34>, 15:w1156:errorcluster)  [unwired: 2 in, 2 out]
                        n716 = TDMS Close(8:w1156, 11:w1155) -> (0:w1154:errorcluster)  [unwired: 1 out]
                      }
                      frame #1 {
                        n717 = local read "DISP LAB05-1"() -> (w1173:T4)
                        n718 = stacked-sequence {
                          tunnel: "LAB05-1" -> [w1175 w1177]
                          frame #0 {
                            n719 = call "sub vi - defrag tdms v1.vi"("panel id"=w1175) -> ("error out"=w1174:errorcluster)  [unwired: 10 in]
                            n720 = local write "data file error"(w1174) -> ()
                          }
                          frame #1 {
                            n721 = call "Save data file to network drive v1.vi"("panel id"=w1177) -> ("network file save error"=w1176:errorcluster)  [unwired: 9 in, 1 out]
                            n722 = local write "RESULT LAB05-1"(FALSE) -> ()
                            n723 = local write "data file error"(w1176) -> ()
                          }
                        }
                        n724 = Bundle(cluster=w1173, "STATUS"="STOP") -> (w1171:T4)  [unwired: 2 in]
                        n725 = local write "DISP LAB05-1"(w1171) -> ()
                      }
                    }
                  }
                  frame True {
                    # "start new test and create test file"
                    n726 = stacked-sequence {
                      seq-local: [w1185 _ _ _ _] -> [_ w1210 _ _ _]
                      tunnel: w1184 -> [w1190 _ _ _ _]
                      tunnel: w1183 -> [w1186 _ _ _ _]
                      tunnel: w1182 -> [w1200 _ _ _ _]
                      tunnel: w1181 -> [w1193 _ _ _ _]
                      tunnel: w1180 -> [w1188 _ _ _ _]
                      tunnel: [_ w1204 _ _ _] -> w1179
                      frame #0 {
                        w1187 = "\\"
                        n727 = local read "SET LAB05-1"() -> (w1195:T5)
                        n728 = case shown="\"CYCLE TEST\"" w1200 {
                          tunnel: ["L05-1-CHART TEST-" "L05-1-CYCLE TEST-" "L05-1-T-RISE TEST-"] -> w1196
                          frame "CHART TEST", Default {
                          }
                          frame "CYCLE TEST" {
                          }
                          frame "T-RISE TEST" {
                          }
                        }
                        n729 = Unbundle(w1195) -> ("DESCRIPTION"=w1194:string)  [unwired: 4 out]
                        n730 = Concatenate Strings(w1190, "\\", w1188, w1187, w1186, w1187) -> (w1197:string)
                        n731 = String To Path(string=w1197) -> (path=w1199:path)
                        n732 = Concatenate Strings(w1197, w1196, w1194, "-", w1193, ".tdms") -> (w1185:string)
                        n733 = Create Folder(path (use dialog)=w1199) -> (error out=w1198:errorcluster)  [unwired: 2 in, 2 out]
                        n734 = global write "Global 1.vi" "LAB05-1 FILE"(w1185) -> ()
                        n735 = call <vilib>:"Clear Errors.vi"("error in (no error)"=w1198) -> ()  [unwired: 6 in, 1 out]
                      }
                      frame #1 {
                        n736 = String To Path(string=w1210) -> (path=w1205:path)
                        n737 = TDMS Open(5:FALSE, 6:FALSE, 10:T16."create or replace" ("operation (0:open)"), 11:w1205) -> (0:w1204:errorcluster, 3:→"TDMS LAB05-1":refnum<k34>)  [unwired: 3 in]
                      }
                      frame #2 {
                        n738 = local read "SET LAB05-1"() -> (w1216:T5)
                        n739 = local read "TDMS LAB05-1"() -> (w1227:refnum<k34>)
                        n740 = Build Array("Testers Name", "Description", "Set Test Cycles", "T-Rise minutes", "T-Rise Deg C") -> (w1217:string[])
                        n741 = Unbundle(w1216) -> ("NAME"=w1215:string, "DESCRIPTION"=w1214:string, "CYCLES"=w1213:dbl, "T-RISE mins"=w1212:dbl, "T-RISE deg C"=w1211:dbl)
                        n742 = Number To Decimal String(number=w1213) -> (decimal integer string=w1226:string)  [unwired: 1 in]
                        n743 = Number To Decimal String(number=w1212) -> (decimal integer string=w1225:string)  [unwired: 1 in]
                        n744 = Number To Decimal String(number=w1211) -> (decimal integer string=w1224:string)  [unwired: 1 in]
                        n745 = Build Array(w1215, w1214, w1226, w1225, w1224) -> (w1223:string[])
                        n746 = TDMS Set Properties(5:w1223, 7:w1217, 11:w1227) -> ()  [unwired: 3 in, 4 out]
                      }
                      frame #3 {
                        w1229 = 0.0
                        n747 = local read "DISP LAB05-1"() -> (w1231:T4)
                        n748 = Bundle(cluster=w1231, "CYCLE"=w1229, "MINS"=w1229, "STATUS"="RUN") -> (w1230:T4)
                        n749 = local write "DISP LAB05-1"(w1230) -> ()
                      }
                      frame #4 {
                        n750 = local read "SIG LAB05-1"() -> (w1234:T2)
                        n751 = local read "TEMP START LAB05-1"() -> (w1236:cluster{"TL":dbl, "TN":dbl})
                        n752 = Unbundle(w1234) -> ("Tmp Live"=w1233:dbl, "Tmp Neut"=w1232:dbl)  [unwired: 3 out]
                        n753 = Bundle(cluster=w1236, "TL"=w1233, "TN"=w1232) -> (w1235:cluster{"TL":dbl, "TN":dbl})
                        n754 = local write "TEMP START LAB05-1"(w1235) -> ()
                      }
                    }
                  }
                }
              }
              event "RUN LAB05-2": Value Change {
                n755 = event-data() -> ("NewVal"=w1237:bool)  [unwired: 1 in, 5 out]
                n756 = local write "run lab05-2"(w1237) -> ()
                n757 = case shown="True" w1237 {
                  tunnel: w1243 -> [_ w1276]
                  tunnel: w1242 -> [_ w1275]
                  tunnel: w1240 -> [w1245 w1274]
                  tunnel: w1241 -> [_ w1273]
                  tunnel: w1239 -> [_ w1272]
                  tunnel: [w1244 w1271] -> w1238
                  frame False {
                    # "stop test"
                    n758 = stacked-sequence {
                      tunnel: w1245 -> [w1254 _]
                      tunnel: [w1246 _] -> w1244
                      frame #0 {
                        n759 = local read "DISP LAB05-2"() -> (w1253:T4)
                        n760 = Unbundle(w1253) -> ("CYCLE"=w1251:dbl, "MINS"=w1252:dbl)  [unwired: 1 out]
                        n761 = case shown="\"CYCLE TEST\"" w1254 {
                          tunnel: w1252 -> [_ _ w1261]
                          tunnel: w1251 -> [w1259 w1260 _]
                          tunnel: [w1259 w1260 w1261] -> w1250
                          frame "CHART TEST", Default {
                          }
                          frame "CYCLE TEST" {
                          }
                          frame "T-RISE TEST" {
                          }
                        }
                        n762 = local read "TDMS LAB05-2"() -> (w1258:refnum<k34>)
                        n763 = Build Array("STOPPED") -> (w1255:string[])
                        n764 = Build Array(w1250) -> (w1249:dbl[])
                        n765 = TDMS Write(0:w1258, 5:"TEST RESULT", 7:w1255, 9:w1249) -> (4:w1247:refnum<k34>, 15:w1248:errorcluster)  [unwired: 2 in, 2 out]
                        n766 = TDMS Close(8:w1248, 11:w1247) -> (0:w1246:errorcluster)  [unwired: 1 out]
                      }
                      frame #1 {
                        n767 = local read "DISP LAB05-2"() -> (w1265:T4)
                        n768 = stacked-sequence {
                          tunnel: "LAB05-2" -> [w1267 w1269]
                          frame #0 {
                            n769 = call "sub vi - defrag tdms v1.vi"("panel id"=w1267) -> ("error out"=w1266:errorcluster)  [unwired: 10 in]
                            n770 = local write "data file error"(w1266) -> ()
                          }
                          frame #1 {
                            n771 = local write "RESULT LAB05-2"(FALSE) -> ()
                            n772 = call "Save data file to network drive v1.vi"("panel id"=w1269) -> ("network file save error"=w1268:errorcluster)  [unwired: 9 in, 1 out]
                            n773 = local write "data file error"(w1268) -> ()
                          }
                        }
                        n774 = Bundle(cluster=w1265, "STATUS"="STOP") -> (w1263:T4)  [unwired: 2 in]
                        n775 = local write "DISP LAB05-2"(w1263) -> ()
                      }
                    }
                  }
                  frame True {
                    # "start new test and create test file"
                    n776 = stacked-sequence {
                      seq-local: [w1277 _ _ _ _] -> [_ w1302 _ _ _]
                      tunnel: w1276 -> [w1282 _ _ _ _]
                      tunnel: w1275 -> [w1278 _ _ _ _]
                      tunnel: w1274 -> [w1292 _ _ _ _]
                      tunnel: w1273 -> [w1285 _ _ _ _]
                      tunnel: w1272 -> [w1280 _ _ _ _]
                      tunnel: [_ w1296 _ _ _] -> w1271
                      frame #0 {
                        w1279 = "\\"
                        n777 = local read "SET LAB05-2"() -> (w1287:T5)
                        n778 = case shown="\"CYCLE TEST\"" w1292 {
                          tunnel: ["L05-2-CHART TEST-" "L05-2-CYCLE TEST-" "L05-2-T-RISE TEST-"] -> w1288
                          frame "CHART TEST", Default {
                          }
                          frame "CYCLE TEST" {
                          }
                          frame "T-RISE TEST" {
                          }
                        }
                        n779 = Unbundle(w1287) -> ("DESCRIPTION"=w1286:string)  [unwired: 4 out]
                        n780 = Concatenate Strings(w1282, "\\", w1280, w1279, w1278, w1279) -> (w1289:string)
                        n781 = String To Path(string=w1289) -> (path=w1291:path)
                        n782 = Concatenate Strings(w1289, w1288, w1286, "-", w1285, ".tdms") -> (w1277:string)
                        n783 = Create Folder(path (use dialog)=w1291) -> (error out=w1290:errorcluster)  [unwired: 2 in, 2 out]
                        n784 = global write "Global 1.vi" "LAB05-2 FILE"(w1277) -> ()
                        n785 = call <vilib>:"Clear Errors.vi"("error in (no error)"=w1290) -> ()  [unwired: 6 in, 1 out]
                      }
                      frame #1 {
                        n786 = String To Path(string=w1302) -> (path=w1297:path)
                        n787 = TDMS Open(5:FALSE, 6:FALSE, 10:T16."create or replace" ("operation (0:open)"), 11:w1297) -> (0:w1296:errorcluster, 3:→"TDMS LAB05-2":refnum<k34>)  [unwired: 3 in]
                      }
                      frame #2 {
                        n788 = local read "SET LAB05-2"() -> (w1308:T5)
                        n789 = local read "TDMS LAB05-2"() -> (w1319:refnum<k34>)
                        n790 = Build Array("Testers Name", "Description", "Set Test Cycles", "T-Rise minutes", "T-Rise Deg C") -> (w1309:string[])
                        n791 = Unbundle(w1308) -> ("NAME"=w1307:string, "DESCRIPTION"=w1306:string, "CYCLES"=w1305:dbl, "T-RISE mins"=w1304:dbl, "T-RISE deg C"=w1303:dbl)
                        n792 = Number To Decimal String(number=w1305) -> (decimal integer string=w1318:string)  [unwired: 1 in]
                        n793 = Number To Decimal String(number=w1304) -> (decimal integer string=w1317:string)  [unwired: 1 in]
                        n794 = Number To Decimal String(number=w1303) -> (decimal integer string=w1316:string)  [unwired: 1 in]
                        n795 = Build Array(w1307, w1306, w1318, w1317, w1316) -> (w1315:string[])
                        n796 = TDMS Set Properties(5:w1315, 7:w1309, 11:w1319) -> ()  [unwired: 3 in, 4 out]
                      }
                      frame #3 {
                        w1321 = 0.0
                        n797 = local read "DISP LAB05-2"() -> (w1323:T4)
                        n798 = Bundle(cluster=w1323, "CYCLE"=w1321, "MINS"=w1321, "STATUS"="RUN") -> (w1322:T4)
                        n799 = local write "DISP LAB05-2"(w1322) -> ()
                      }
                      frame #4 {
                        n800 = local read "SIG LAB05-2"() -> (w1326:T2)
                        n801 = local read "TEMP START LAB05-2"() -> (w1328:cluster{"TL":dbl, "TN":dbl})
                        n802 = Unbundle(w1326) -> ("Tmp Live"=w1325:dbl, "Tmp Neut"=w1324:dbl)  [unwired: 3 out]
                        n803 = Bundle(cluster=w1328, "TL"=w1325, "TN"=w1324) -> (w1327:cluster{"TL":dbl, "TN":dbl})
                        n804 = local write "TEMP START LAB05-2"(w1327) -> ()
                      }
                    }
                  }
                }
              }
            }
            n805 = local write "data file error"(w380) -> ()
          }
          frame #4 {
            # "check if test cycles reached for cycle tests, if so then test pass"
            n806 = stacked-sequence {
              tunnel: w1348 -> [_ _ _ _ _ _ _ _ _ _]
              tunnel: w1347 -> [_ _ _ _ _ _ _ _ _ _]
              tunnel: w1346 -> [_ _ _ _ _ _ _ _ _ _]
              tunnel: w1345 -> [_ _ _ _ _ _ _ _ _ _]
              tunnel: w1344 -> [_ _ _ _ _ _ _ _ _ _]
              tunnel: w1343 -> [_ _ _ _ _ _ _ _ _ _]
              tunnel: w1342 -> [_ _ _ _ _ _ _ _ _ _]
              tunnel: w1341 -> [_ _ _ _ _ _ _ _ _ _]
              tunnel: w1340 -> [_ _ _ _ _ _ _ _ _ _]
              tunnel: w1339 -> [_ _ _ _ _ _ _ _ _ _]
              tunnel: w1338 -> [w1354 _ _ _ _ _ _ _ _ _]
              tunnel: w1337 -> [_ w1389 _ _ _ _ _ _ _ _]
              tunnel: w1336 -> [_ _ w1429 _ _ _ _ _ _ _]
              tunnel: w1335 -> [_ _ _ w1469 _ _ _ _ _ _]
              tunnel: w1334 -> [_ _ _ _ w1509 _ _ _ _ _]
              tunnel: w1333 -> [_ _ _ _ _ w1549 _ _ _ _]
              tunnel: w1332 -> [_ _ _ _ _ _ w1589 _ _ _]
              tunnel: w1331 -> [_ _ _ _ _ _ _ w1629 _ _]
              tunnel: w1330 -> [_ _ _ _ _ _ _ _ w1669 _]
              tunnel: w1329 -> [_ _ _ _ _ _ _ _ _ w1709]
              frame #0 {
                # "LAB01-1"
                n807 = Less?(x=w1354, y=2) -> (x < y?=w1352:bool)
                n808 = local read "DISP LAB01-1"() -> (w1355:T4)
                n809 = Unbundle(w1355) -> ("STATUS"=w1349:string)  [unwired: 2 out]
                n810 = Equal?(x=w1349, y="RUN") -> (x = y?=w1351:bool)
                n811 = And(x=w1351, y=w1352) -> (x .and. y?=w1350:bool)
                n812 = case shown="True" w1350 {
                  tunnel: w1355 -> [_ w1360]
                  tunnel: w1354 -> [_ w1364]
                  frame False {
                  }
                  frame True {
                    n813 = local read "SET LAB01-1"() -> (w1366:T5)
                    n814 = local read "TDMS LAB01-1"() -> (w1359:refnum<k34>)
                    n815 = Unbundle(w1366) -> ("CYCLES"=w1357:dbl, "T-RISE mins"=w1363:dbl)  [unwired: 3 out]
                    n816 = case shown="\"CYCLE TEST\"" w1364 {
                      tunnel: w1363 -> [_ _ w1373]
                      tunnel: [w1368 w1370 w1373] -> w1362
                      tunnel: w1357 -> [w1368 w1370 _]
                      tunnel: ["CHART PASS" "CYCLE PASS" "T-RISE PASS"] -> w1361
                      frame "CHART TEST", Default {
                      }
                      frame "CYCLE TEST" {
                      }
                      frame "T-RISE TEST" {
                      }
                    }
                    n817 = Unbundle(w1360) -> ("CYCLE"=w1365:dbl)  [unwired: 2 out]
                    n818 = Increment(x=w1357) -> (x+1=w1358:dbl)
                    n819 = Greater Or Equal?(x=w1365, y=w1358) -> (x >= y?=w1367:bool)
                    n820 = case shown="True" w1367 {
                      tunnel: w1362 -> [w1377 _]
                      tunnel: w1361 -> [w1376 _]
                      tunnel: w1360 -> [w1375 _]
                      tunnel: w1359 -> [w1374 _]
                      frame True {
                        n821 = stacked-sequence {
                          tunnel: w1377 -> [w1381 _]
                          tunnel: w1376 -> [w1379 w1385]
                          tunnel: w1375 -> [_ w1388]
                          tunnel: w1374 -> [w1378 _]
                          frame #0 {
                            n822 = Build Array(w1379) -> (w1382:string[])
                            n823 = Build Array(w1381) -> (w1380:dbl[])
                            n824 = TDMS Write(0:w1378, 5:"TEST PASS", 7:w1382, 9:w1380) -> (15:w1384:errorcluster)  [unwired: 2 in, 3 out]
                            n825 = local write "data file error"(w1384) -> ()
                          }
                          frame #1 {
                            n826 = Bundle(cluster=w1388, "STATUS"=w1385) -> (w1386:T4)  [unwired: 2 in]
                            n827 = local write "RESULT LAB01-1"(TRUE) -> ()
                            n828 = local write "DISP LAB01-1"(w1386) -> ()
                          }
                        }
                      }
                      frame False {
                      }
                    }
                  }
                }
              }
              frame #1 {
                # "LAB01-2"
                n829 = Less?(x=w1389, y=2) -> (x < y?=w1392:bool)
                n830 = local read "DISP LAB01-2"() -> (w1394:T4)
                n831 = Unbundle(w1394) -> ("STATUS"=w1395:string)  [unwired: 2 out]
                n832 = Equal?(x=w1395, y="RUN") -> (x = y?=w1391:bool)
                n833 = And(x=w1391, y=w1392) -> (x .and. y?=w1390:bool)
                n834 = case shown="True" w1390 {
                  tunnel: w1394 -> [_ w1400]
                  tunnel: w1389 -> [_ w1404]
                  frame False {
                  }
                  frame True {
                    n835 = local read "SET LAB01-2"() -> (w1406:T5)
                    n836 = local read "TDMS LAB01-2"() -> (w1399:refnum<k34>)
                    n837 = Unbundle(w1406) -> ("CYCLES"=w1397:dbl, "T-RISE mins"=w1403:dbl)  [unwired: 3 out]
                    n838 = case shown="\"T-RISE TEST\"" w1404 {
                      tunnel: w1403 -> [_ _ w1413]
                      tunnel: [w1408 w1410 w1413] -> w1402
                      tunnel: w1397 -> [w1408 w1410 _]
                      tunnel: ["CHART PASS" "CYCLE PASS" "T-RISE PASS"] -> w1401
                      frame "CHART TEST", Default {
                      }
                      frame "CYCLE TEST" {
                      }
                      frame "T-RISE TEST" {
                      }
                    }
                    n839 = Unbundle(w1400) -> ("CYCLE"=w1405:dbl)  [unwired: 2 out]
                    n840 = Increment(x=w1397) -> (x+1=w1398:dbl)
                    n841 = Greater Or Equal?(x=w1405, y=w1398) -> (x >= y?=w1407:bool)
                    n842 = case shown="True" w1407 {
                      tunnel: w1402 -> [w1417 _]
                      tunnel: w1401 -> [w1416 _]
                      tunnel: w1400 -> [w1415 _]
                      tunnel: w1399 -> [w1414 _]
                      frame True {
                        n843 = stacked-sequence {
                          tunnel: w1417 -> [w1421 _]
                          tunnel: w1416 -> [w1419 w1425]
                          tunnel: w1415 -> [_ w1428]
                          tunnel: w1414 -> [w1418 _]
                          frame #0 {
                            n844 = Build Array(w1419) -> (w1422:string[])
                            n845 = Build Array(w1421) -> (w1420:dbl[])
                            n846 = TDMS Write(0:w1418, 5:"TEST PASS", 7:w1422, 9:w1420) -> (15:w1424:errorcluster)  [unwired: 2 in, 3 out]
                            n847 = local write "data file error"(w1424) -> ()
                          }
                          frame #1 {
                            n848 = Bundle(cluster=w1428, "STATUS"=w1425) -> (w1426:T4)  [unwired: 2 in]
                            n849 = local write "RESULT LAB01-2"(TRUE) -> ()
                            n850 = local write "DISP LAB01-2"(w1426) -> ()
                          }
                        }
                      }
                      frame False {
                      }
                    }
                  }
                }
              }
              frame #2 {
                # "LAB02-1"
                n851 = Less?(x=w1429, y=2) -> (x < y?=w1432:bool)
                n852 = local read "DISP LAB02-1"() -> (w1434:T4)
                n853 = Unbundle(w1434) -> ("STATUS"=w1435:string)  [unwired: 2 out]
                n854 = Equal?(x=w1435, y="RUN") -> (x = y?=w1431:bool)
                n855 = And(x=w1431, y=w1432) -> (x .and. y?=w1430:bool)
                n856 = case shown="True" w1430 {
                  tunnel: w1434 -> [_ w1440]
                  tunnel: w1429 -> [_ w1444]
                  frame False {
                  }
                  frame True {
                    n857 = local read "SET LAB02-1"() -> (w1446:T5)
                    n858 = local read "TDMS LAB02-1"() -> (w1439:refnum<k34>)
                    n859 = Unbundle(w1440) -> ("CYCLE"=w1445:dbl)  [unwired: 2 out]
                    n860 = Unbundle(w1446) -> ("CYCLES"=w1437:dbl, "T-RISE mins"=w1443:dbl)  [unwired: 3 out]
                    n861 = case shown="\"T-RISE TEST\"" w1444 {
                      tunnel: w1443 -> [_ _ w1453]
                      tunnel: [w1448 w1450 w1453] -> w1442
                      tunnel: w1437 -> [w1448 w1450 _]
                      tunnel: ["CHART PASS" "CYCLE PASS" "T-RISE PASS"] -> w1441
                      frame "CHART TEST", Default {
                      }
                      frame "CYCLE TEST" {
                      }
                      frame "T-RISE TEST" {
                      }
                    }
                    n862 = Increment(x=w1437) -> (x+1=w1438:dbl)
                    n863 = Greater Or Equal?(x=w1445, y=w1438) -> (x >= y?=w1447:bool)
                    n864 = case shown="True" w1447 {
                      tunnel: w1442 -> [w1457 _]
                      tunnel: w1441 -> [w1456 _]
                      tunnel: w1440 -> [w1455 _]
                      tunnel: w1439 -> [w1454 _]
                      frame True {
                        n865 = stacked-sequence {
                          tunnel: w1457 -> [w1461 _]
                          tunnel: w1456 -> [w1459 w1465]
                          tunnel: w1455 -> [_ w1468]
                          tunnel: w1454 -> [w1458 _]
                          frame #0 {
                            n866 = Build Array(w1459) -> (w1462:string[])
                            n867 = Build Array(w1461) -> (w1460:dbl[])
                            n868 = TDMS Write(0:w1458, 5:"TEST PASS", 7:w1462, 9:w1460) -> (15:w1464:errorcluster)  [unwired: 2 in, 3 out]
                            n869 = local write "data file error"(w1464) -> ()
                          }
                          frame #1 {
                            n870 = Bundle(cluster=w1468, "STATUS"=w1465) -> (w1466:T4)  [unwired: 2 in]
                            n871 = local write "RESULT LAB02-1"(TRUE) -> ()
                            n872 = local write "DISP LAB02-1"(w1466) -> ()
                          }
                        }
                      }
                      frame False {
                      }
                    }
                  }
                }
              }
              frame #3 {
                # "LAB02-2"
                n873 = Less?(x=w1469, y=2) -> (x < y?=w1472:bool)
                n874 = local read "DISP LAB02-2"() -> (w1474:T4)
                n875 = Unbundle(w1474) -> ("STATUS"=w1475:string)  [unwired: 2 out]
                n876 = Equal?(x=w1475, y="RUN") -> (x = y?=w1471:bool)
                n877 = And(x=w1471, y=w1472) -> (x .and. y?=w1470:bool)
                n878 = case shown="True" w1470 {
                  tunnel: w1474 -> [_ w1480]
                  tunnel: w1469 -> [_ w1484]
                  frame False {
                  }
                  frame True {
                    n879 = local read "SET LAB02-2"() -> (w1486:T5)
                    n880 = local read "TDMS LAB02-2"() -> (w1479:refnum<k34>)
                    n881 = Unbundle(w1480) -> ("CYCLE"=w1485:dbl)  [unwired: 2 out]
                    n882 = Unbundle(w1486) -> ("CYCLES"=w1477:dbl, "T-RISE mins"=w1483:dbl)  [unwired: 3 out]
                    n883 = case shown="\"T-RISE TEST\"" w1484 {
                      tunnel: w1483 -> [_ _ w1493]
                      tunnel: [w1488 w1490 w1493] -> w1482
                      tunnel: w1477 -> [w1488 w1490 _]
                      tunnel: ["CHART PASS" "CYCLE PASS" "T-RISE PASS"] -> w1481
                      frame "CHART TEST", Default {
                      }
                      frame "CYCLE TEST" {
                      }
                      frame "T-RISE TEST" {
                      }
                    }
                    n884 = Increment(x=w1477) -> (x+1=w1478:dbl)
                    n885 = Greater Or Equal?(x=w1485, y=w1478) -> (x >= y?=w1487:bool)
                    n886 = case shown="True" w1487 {
                      tunnel: w1482 -> [w1497 _]
                      tunnel: w1481 -> [w1496 _]
                      tunnel: w1480 -> [w1495 _]
                      tunnel: w1479 -> [w1494 _]
                      frame True {
                        n887 = stacked-sequence {
                          tunnel: w1497 -> [w1501 _]
                          tunnel: w1496 -> [w1499 w1505]
                          tunnel: w1495 -> [_ w1508]
                          tunnel: w1494 -> [w1498 _]
                          frame #0 {
                            n888 = Build Array(w1499) -> (w1502:string[])
                            n889 = Build Array(w1501) -> (w1500:dbl[])
                            n890 = TDMS Write(0:w1498, 5:"TEST PASS", 7:w1502, 9:w1500) -> (15:w1504:errorcluster)  [unwired: 2 in, 3 out]
                            n891 = local write "data file error"(w1504) -> ()
                          }
                          frame #1 {
                            n892 = Bundle(cluster=w1508, "STATUS"=w1505) -> (w1506:T4)  [unwired: 2 in]
                            n893 = local write "RESULT LAB02-2"(TRUE) -> ()
                            n894 = local write "DISP LAB02-2"(w1506) -> ()
                          }
                        }
                      }
                      frame False {
                      }
                    }
                  }
                }
              }
              frame #4 {
                # "LAB03-1"
                n895 = Less?(x=w1509, y=2) -> (x < y?=w1512:bool)
                n896 = local read "DISP LAB03-1"() -> (w1514:T4)
                n897 = Unbundle(w1514) -> ("STATUS"=w1515:string)  [unwired: 2 out]
                n898 = Equal?(x=w1515, y="RUN") -> (x = y?=w1511:bool)
                n899 = And(x=w1511, y=w1512) -> (x .and. y?=w1510:bool)
                n900 = case shown="True" w1510 {
                  tunnel: w1514 -> [_ w1520]
                  tunnel: w1509 -> [_ w1524]
                  frame False {
                  }
                  frame True {
                    n901 = local read "SET LAB03-1"() -> (w1526:T5)
                    n902 = local read "TDMS LAB03-1"() -> (w1519:refnum<k34>)
                    n903 = Unbundle(w1520) -> ("CYCLE"=w1525:dbl)  [unwired: 2 out]
                    n904 = Unbundle(w1526) -> ("CYCLES"=w1517:dbl, "T-RISE mins"=w1523:dbl)  [unwired: 3 out]
                    n905 = case shown="\"T-RISE TEST\"" w1524 {
                      tunnel: w1523 -> [_ _ w1533]
                      tunnel: [w1528 w1530 w1533] -> w1522
                      tunnel: w1517 -> [w1528 w1530 _]
                      tunnel: ["CHART PASS" "CYCLE PASS" "T-RISE PASS"] -> w1521
                      frame "CHART TEST", Default {
                      }
                      frame "CYCLE TEST" {
                      }
                      frame "T-RISE TEST" {
                      }
                    }
                    n906 = Increment(x=w1517) -> (x+1=w1518:dbl)
                    n907 = Greater Or Equal?(x=w1525, y=w1518) -> (x >= y?=w1527:bool)
                    n908 = case shown="True" w1527 {
                      tunnel: w1522 -> [w1537 _]
                      tunnel: w1521 -> [w1536 _]
                      tunnel: w1520 -> [w1535 _]
                      tunnel: w1519 -> [w1534 _]
                      frame True {
                        n909 = stacked-sequence {
                          tunnel: w1537 -> [w1541 _]
                          tunnel: w1536 -> [w1539 w1545]
                          tunnel: w1535 -> [_ w1548]
                          tunnel: w1534 -> [w1538 _]
                          frame #0 {
                            n910 = Build Array(w1539) -> (w1542:string[])
                            n911 = Build Array(w1541) -> (w1540:dbl[])
                            n912 = TDMS Write(0:w1538, 5:"TEST PASS", 7:w1542, 9:w1540) -> (15:w1544:errorcluster)  [unwired: 2 in, 3 out]
                            n913 = local write "data file error"(w1544) -> ()
                          }
                          frame #1 {
                            n914 = Bundle(cluster=w1548, "STATUS"=w1545) -> (w1546:T4)  [unwired: 2 in]
                            n915 = local write "RESULT LAB03-1"(TRUE) -> ()
                            n916 = local write "DISP LAB03-1"(w1546) -> ()
                          }
                        }
                      }
                      frame False {
                      }
                    }
                  }
                }
              }
              frame #5 {
                # "LAB03-2"
                n917 = Less?(x=w1549, y=2) -> (x < y?=w1552:bool)
                n918 = local read "DISP LAB03-2"() -> (w1554:T4)
                n919 = Unbundle(w1554) -> ("STATUS"=w1555:string)  [unwired: 2 out]
                n920 = Equal?(x=w1555, y="RUN") -> (x = y?=w1551:bool)
                n921 = And(x=w1551, y=w1552) -> (x .and. y?=w1550:bool)
                n922 = case shown="True" w1550 {
                  tunnel: w1554 -> [_ w1560]
                  tunnel: w1549 -> [_ w1564]
                  frame False {
                  }
                  frame True {
                    n923 = local read "SET LAB03-2"() -> (w1566:T5)
                    n924 = local read "TDMS LAB03-2"() -> (w1559:refnum<k34>)
                    n925 = Unbundle(w1560) -> ("CYCLE"=w1565:dbl)  [unwired: 2 out]
                    n926 = Unbundle(w1566) -> ("CYCLES"=w1557:dbl, "T-RISE mins"=w1563:dbl)  [unwired: 3 out]
                    n927 = case shown="\"T-RISE TEST\"" w1564 {
                      tunnel: w1563 -> [_ _ w1573]
                      tunnel: [w1568 w1570 w1573] -> w1562
                      tunnel: w1557 -> [w1568 w1570 _]
                      tunnel: ["CHART PASS" "CYCLE PASS" "T-RISE PASS"] -> w1561
                      frame "CHART TEST", Default {
                      }
                      frame "CYCLE TEST" {
                      }
                      frame "T-RISE TEST" {
                      }
                    }
                    n928 = Increment(x=w1557) -> (x+1=w1558:dbl)
                    n929 = Greater Or Equal?(x=w1565, y=w1558) -> (x >= y?=w1567:bool)
                    n930 = case shown="True" w1567 {
                      tunnel: w1562 -> [w1577 _]
                      tunnel: w1561 -> [w1576 _]
                      tunnel: w1560 -> [w1575 _]
                      tunnel: w1559 -> [w1574 _]
                      frame True {
                        n931 = stacked-sequence {
                          tunnel: w1577 -> [w1581 _]
                          tunnel: w1576 -> [w1579 w1585]
                          tunnel: w1575 -> [_ w1588]
                          tunnel: w1574 -> [w1578 _]
                          frame #0 {
                            n932 = Build Array(w1579) -> (w1582:string[])
                            n933 = Build Array(w1581) -> (w1580:dbl[])
                            n934 = TDMS Write(0:w1578, 5:"TEST PASS", 7:w1582, 9:w1580) -> (15:w1584:errorcluster)  [unwired: 2 in, 3 out]
                            n935 = local write "data file error"(w1584) -> ()
                          }
                          frame #1 {
                            n936 = Bundle(cluster=w1588, "STATUS"=w1585) -> (w1586:T4)  [unwired: 2 in]
                            n937 = local write "RESULT LAB03-2"(TRUE) -> ()
                            n938 = local write "DISP LAB03-2"(w1586) -> ()
                          }
                        }
                      }
                      frame False {
                      }
                    }
                  }
                }
              }
              frame #6 {
                # "LAB04-1"
                n939 = Less?(x=w1589, y=2) -> (x < y?=w1592:bool)
                n940 = local read "DISP LAB04-1"() -> (w1594:T4)
                n941 = Unbundle(w1594) -> ("STATUS"=w1595:string)  [unwired: 2 out]
                n942 = Equal?(x=w1595, y="RUN") -> (x = y?=w1591:bool)
                n943 = And(x=w1591, y=w1592) -> (x .and. y?=w1590:bool)
                n944 = case shown="True" w1590 {
                  tunnel: w1594 -> [_ w1600]
                  tunnel: w1589 -> [_ w1604]
                  frame False {
                  }
                  frame True {
                    n945 = local read "SET LAB04-1"() -> (w1606:T5)
                    n946 = local read "TDMS LAB04-1"() -> (w1599:refnum<k34>)
                    n947 = Unbundle(w1600) -> ("CYCLE"=w1605:dbl)  [unwired: 2 out]
                    n948 = Unbundle(w1606) -> ("CYCLES"=w1597:dbl, "T-RISE mins"=w1603:dbl)  [unwired: 3 out]
                    n949 = case shown="\"T-RISE TEST\"" w1604 {
                      tunnel: w1603 -> [_ _ w1613]
                      tunnel: [w1608 w1610 w1613] -> w1602
                      tunnel: w1597 -> [w1608 w1610 _]
                      tunnel: ["CHART PASS" "CYCLE PASS" "T-RISE PASS"] -> w1601
                      frame "CHART TEST", Default {
                      }
                      frame "CYCLE TEST" {
                      }
                      frame "T-RISE TEST" {
                      }
                    }
                    n950 = Increment(x=w1597) -> (x+1=w1598:dbl)
                    n951 = Greater Or Equal?(x=w1605, y=w1598) -> (x >= y?=w1607:bool)
                    n952 = case shown="True" w1607 {
                      tunnel: w1602 -> [w1617 _]
                      tunnel: w1601 -> [w1616 _]
                      tunnel: w1600 -> [w1615 _]
                      tunnel: w1599 -> [w1614 _]
                      frame True {
                        n953 = stacked-sequence {
                          tunnel: w1617 -> [w1621 _]
                          tunnel: w1616 -> [w1619 w1625]
                          tunnel: w1615 -> [_ w1628]
                          tunnel: w1614 -> [w1618 _]
                          frame #0 {
                            n954 = Build Array(w1619) -> (w1622:string[])
                            n955 = Build Array(w1621) -> (w1620:dbl[])
                            n956 = TDMS Write(0:w1618, 5:"TEST PASS", 7:w1622, 9:w1620) -> (15:w1624:errorcluster)  [unwired: 2 in, 3 out]
                            n957 = local write "data file error"(w1624) -> ()
                          }
                          frame #1 {
                            n958 = Bundle(cluster=w1628, "STATUS"=w1625) -> (w1626:T4)  [unwired: 2 in]
                            n959 = local write "RESULT LAB04-1"(TRUE) -> ()
                            n960 = local write "DISP LAB04-1"(w1626) -> ()
                          }
                        }
                      }
                      frame False {
                      }
                    }
                  }
                }
              }
              frame #7 {
                # "LAB04-2"
                n961 = Less?(x=w1629, y=2) -> (x < y?=w1632:bool)
                n962 = local read "DISP LAB04-2"() -> (w1634:T4)
                n963 = Unbundle(w1634) -> ("STATUS"=w1635:string)  [unwired: 2 out]
                n964 = Equal?(x=w1635, y="RUN") -> (x = y?=w1631:bool)
                n965 = And(x=w1631, y=w1632) -> (x .and. y?=w1630:bool)
                n966 = case shown="True" w1630 {
                  tunnel: w1634 -> [_ w1640]
                  tunnel: w1629 -> [_ w1644]
                  frame False {
                  }
                  frame True {
                    n967 = local read "SET LAB04-2"() -> (w1646:T5)
                    n968 = local read "TDMS LAB04-2"() -> (w1639:refnum<k34>)
                    n969 = Unbundle(w1640) -> ("CYCLE"=w1645:dbl)  [unwired: 2 out]
                    n970 = Unbundle(w1646) -> ("CYCLES"=w1637:dbl, "T-RISE mins"=w1643:dbl)  [unwired: 3 out]
                    n971 = case shown="\"T-RISE TEST\"" w1644 {
                      tunnel: w1643 -> [_ _ w1653]
                      tunnel: [w1648 w1650 w1653] -> w1642
                      tunnel: w1637 -> [w1648 w1650 _]
                      tunnel: ["CHART PASS" "CYCLE PASS" "T-RISE PASS"] -> w1641
                      frame "CHART TEST", Default {
                      }
                      frame "CYCLE TEST" {
                      }
                      frame "T-RISE TEST" {
                      }
                    }
                    n972 = Increment(x=w1637) -> (x+1=w1638:dbl)
                    n973 = Greater Or Equal?(x=w1645, y=w1638) -> (x >= y?=w1647:bool)
                    n974 = case shown="True" w1647 {
                      tunnel: w1642 -> [w1657 _]
                      tunnel: w1641 -> [w1656 _]
                      tunnel: w1640 -> [w1655 _]
                      tunnel: w1639 -> [w1654 _]
                      frame True {
                        n975 = stacked-sequence {
                          tunnel: w1657 -> [w1661 _]
                          tunnel: w1656 -> [w1659 w1665]
                          tunnel: w1655 -> [_ w1668]
                          tunnel: w1654 -> [w1658 _]
                          frame #0 {
                            n976 = Build Array(w1659) -> (w1662:string[])
                            n977 = Build Array(w1661) -> (w1660:dbl[])
                            n978 = TDMS Write(0:w1658, 5:"TEST PASS", 7:w1662, 9:w1660) -> (15:w1664:errorcluster)  [unwired: 2 in, 3 out]
                            n979 = local write "data file error"(w1664) -> ()
                          }
                          frame #1 {
                            n980 = Bundle(cluster=w1668, "STATUS"=w1665) -> (w1666:T4)  [unwired: 2 in]
                            n981 = local write "RESULT LAB04-2"(TRUE) -> ()
                            n982 = local write "DISP LAB04-2"(w1666) -> ()
                          }
                        }
                      }
                      frame False {
                      }
                    }
                  }
                }
              }
              frame #8 {
                # "LAB05-1"
                n983 = Less?(x=w1669, y=2) -> (x < y?=w1672:bool)
                n984 = local read "DISP LAB05-1"() -> (w1674:T4)
                n985 = Unbundle(w1674) -> ("STATUS"=w1675:string)  [unwired: 2 out]
                n986 = Equal?(x=w1675, y="RUN") -> (x = y?=w1671:bool)
                n987 = And(x=w1671, y=w1672) -> (x .and. y?=w1670:bool)
                n988 = case shown="True" w1670 {
                  tunnel: w1674 -> [_ w1680]
                  tunnel: w1669 -> [_ w1684]
                  frame False {
                  }
                  frame True {
                    n989 = local read "SET LAB05-1"() -> (w1686:T5)
                    n990 = local read "TDMS LAB05-1"() -> (w1679:refnum<k34>)
                    n991 = Unbundle(w1680) -> ("CYCLE"=w1685:dbl)  [unwired: 2 out]
                    n992 = Unbundle(w1686) -> ("CYCLES"=w1677:dbl, "T-RISE mins"=w1683:dbl)  [unwired: 3 out]
                    n993 = case shown="\"T-RISE TEST\"" w1684 {
                      tunnel: w1683 -> [_ _ w1693]
                      tunnel: [w1688 w1690 w1693] -> w1682
                      tunnel: w1677 -> [w1688 w1690 _]
                      tunnel: ["CHART PASS" "CYCLE PASS" "T-RISE PASS"] -> w1681
                      frame "CHART TEST", Default {
                      }
                      frame "CYCLE TEST" {
                      }
                      frame "T-RISE TEST" {
                      }
                    }
                    n994 = Increment(x=w1677) -> (x+1=w1678:dbl)
                    n995 = Greater Or Equal?(x=w1685, y=w1678) -> (x >= y?=w1687:bool)
                    n996 = case shown="True" w1687 {
                      tunnel: w1682 -> [w1697 _]
                      tunnel: w1681 -> [w1696 _]
                      tunnel: w1680 -> [w1695 _]
                      tunnel: w1679 -> [w1694 _]
                      frame True {
                        n997 = stacked-sequence {
                          tunnel: w1697 -> [w1701 _]
                          tunnel: w1696 -> [w1699 w1705]
                          tunnel: w1695 -> [_ w1708]
                          tunnel: w1694 -> [w1698 _]
                          frame #0 {
                            n998 = Build Array(w1699) -> (w1702:string[])
                            n999 = Build Array(w1701) -> (w1700:dbl[])
                            n1000 = TDMS Write(0:w1698, 5:"TEST PASS", 7:w1702, 9:w1700) -> (15:w1704:errorcluster)  [unwired: 2 in, 3 out]
                            n1001 = local write "data file error"(w1704) -> ()
                          }
                          frame #1 {
                            n1002 = Bundle(cluster=w1708, "STATUS"=w1705) -> (w1706:T4)  [unwired: 2 in]
                            n1003 = local write "RESULT LAB05-1"(TRUE) -> ()
                            n1004 = local write "DISP LAB05-1"(w1706) -> ()
                          }
                        }
                      }
                      frame False {
                      }
                    }
                  }
                }
              }
              frame #9 {
                # "LAB05-2"
                n1005 = Less?(x=w1709, y=2) -> (x < y?=w1712:bool)
                n1006 = local read "DISP LAB05-2"() -> (w1714:T4)
                n1007 = Unbundle(w1714) -> ("STATUS"=w1715:string)  [unwired: 2 out]
                n1008 = Equal?(x=w1715, y="RUN") -> (x = y?=w1711:bool)
                n1009 = And(x=w1711, y=w1712) -> (x .and. y?=w1710:bool)
                n1010 = case shown="True" w1710 {
                  tunnel: w1714 -> [_ w1720]
                  tunnel: w1709 -> [_ w1724]
                  frame False {
                  }
                  frame True {
                    n1011 = local read "SET LAB05-2"() -> (w1726:T5)
                    n1012 = local read "TDMS LAB05-2"() -> (w1719:refnum<k34>)
                    n1013 = Unbundle(w1720) -> ("CYCLE"=w1725:dbl)  [unwired: 2 out]
                    n1014 = Unbundle(w1726) -> ("CYCLES"=w1717:dbl, "T-RISE mins"=w1723:dbl)  [unwired: 3 out]
                    n1015 = case shown="\"T-RISE TEST\"" w1724 {
                      tunnel: w1723 -> [_ _ w1733]
                      tunnel: [w1728 w1730 w1733] -> w1722
                      tunnel: w1717 -> [w1728 w1730 _]
                      tunnel: ["CHART PASS" "CYCLE PASS" "T-RISE PASS"] -> w1721
                      frame "CHART TEST", Default {
                      }
                      frame "CYCLE TEST" {
                      }
                      frame "T-RISE TEST" {
                      }
                    }
                    n1016 = Increment(x=w1717) -> (x+1=w1718:dbl)
                    n1017 = Greater Or Equal?(x=w1725, y=w1718) -> (x >= y?=w1727:bool)
                    n1018 = case shown="True" w1727 {
                      tunnel: w1722 -> [w1737 _]
                      tunnel: w1721 -> [w1736 _]
                      tunnel: w1720 -> [w1735 _]
                      tunnel: w1719 -> [w1734 _]
                      frame True {
                        n1019 = stacked-sequence {
                          tunnel: w1737 -> [w1741 _]
                          tunnel: w1736 -> [w1739 w1745]
                          tunnel: w1735 -> [_ w1748]
                          tunnel: w1734 -> [w1738 _]
                          frame #0 {
                            n1020 = Build Array(w1739) -> (w1742:string[])
                            n1021 = Build Array(w1741) -> (w1740:dbl[])
                            n1022 = TDMS Write(0:w1738, 5:"TEST PASS", 7:w1742, 9:w1740) -> (15:w1744:errorcluster)  [unwired: 2 in, 3 out]
                            n1023 = local write "data file error"(w1744) -> ()
                          }
                          frame #1 {
                            n1024 = Bundle(cluster=w1748, "STATUS"=w1745) -> (w1746:T4)  [unwired: 2 in]
                            n1025 = local write "RESULT LAB05-2"(TRUE) -> ()
                            n1026 = local write "DISP LAB05-2"(w1746) -> ()
                          }
                        }
                      }
                      frame False {
                      }
                    }
                  }
                }
              }
            }
          }
          frame #5 {
            # "check if test cycles reached for temperature rise test"
            n1027 = stacked-sequence {
              tunnel: w1778 -> [_ _ _ _ _ _ _ _ _ _]
              tunnel: w1777 -> [_ _ _ _ _ _ _ _ _ _]
              tunnel: w1776 -> [_ _ _ _ _ _ _ _ _ _]
              tunnel: w1775 -> [_ _ _ _ _ _ _ _ _ _]
              tunnel: w1774 -> [_ _ _ _ _ _ _ _ _ _]
              tunnel: w1773 -> [_ _ _ _ _ _ _ _ _ _]
              tunnel: w1772 -> [_ _ _ _ _ _ _ _ _ _]
              tunnel: w1771 -> [_ _ _ _ _ _ _ _ _ _]
              tunnel: w1770 -> [_ _ _ _ _ _ _ _ _ _]
              tunnel: w1769 -> [_ _ _ _ _ _ _ _ _ _]
              tunnel: w1768 -> [w1784 _ _ _ _ _ _ _ _ _]
              tunnel: w1758 -> [w1779 _ _ _ _ _ _ _ _ _]
              tunnel: w1767 -> [_ w1810 _ _ _ _ _ _ _ _]
              tunnel: w1766 -> [_ _ w1840 _ _ _ _ _ _ _]
              tunnel: w1765 -> [_ _ _ w1870 _ _ _ _ _ _]
              tunnel: w1764 -> [_ _ _ _ w1900 _ _ _ _ _]
              tunnel: w1763 -> [_ _ _ _ _ w1930 _ _ _ _]
              tunnel: w1762 -> [_ _ _ _ _ _ w1960 _ _ _]
              tunnel: w1761 -> [_ _ _ _ _ _ _ w1990 _ _]
              tunnel: w1760 -> [_ _ _ _ _ _ _ _ w2020 _]
              tunnel: w1759 -> [_ _ _ _ _ _ _ _ _ w2050]
              tunnel: w1757 -> [_ w1809 _ _ _ _ _ _ _ _]
              tunnel: w1756 -> [_ _ w1839 _ _ _ _ _ _ _]
              tunnel: w1755 -> [_ _ _ w1869 _ _ _ _ _ _]
              tunnel: w1754 -> [_ _ _ _ w1899 _ _ _ _ _]
              tunnel: w1753 -> [_ _ _ _ _ w1929 _ _ _ _]
              tunnel: w1752 -> [_ _ _ _ _ _ w1959 _ _ _]
              tunnel: w1751 -> [_ _ _ _ _ _ _ w1989 _ _]
              tunnel: w1750 -> [_ _ _ _ _ _ _ _ w2019 _]
              tunnel: w1749 -> [_ _ _ _ _ _ _ _ _ w2049]
              frame #0 {
                # "LAB01-1"
                n1028 = Equal?(x=w1784, y=2) -> (x = y?=w1782:bool)
                n1029 = local read "DISP LAB01-1"() -> (w1785:T4)
                n1030 = Unbundle(w1785) -> ("STATUS"=w1786:string)  [unwired: 2 out]
                n1031 = Equal?(x=w1786, y="RUN") -> (x = y?=w1781:bool)
                n1032 = And(x=w1781, y=w1782) -> (x .and. y?=w1780:bool)
                n1033 = case shown="True" w1780 {
                  tunnel: w1785 -> [_ w1789]
                  tunnel: w1779 -> [_ w1792]
                  frame False {
                  }
                  frame True {
                    n1034 = local read "SET LAB01-1"() -> (w1791:T5)
                    n1035 = local read "TDMS LAB01-1"() -> (w1788:refnum<k34>)
                    n1036 = Unbundle(w1789) -> ("CYCLE"=w1793:dbl)  [unwired: 2 out]
                    n1037 = Unbundle(w1791) -> ("T-RISE mins"=w1790:dbl)  [unwired: 4 out]
                    n1038 = Greater Or Equal?(x=w1793, y=w1792) -> (x >= y?=w1794:bool)
                    n1039 = case shown="True" w1794 {
                      tunnel: w1790 -> [w1797 _]
                      tunnel: w1789 -> [w1796 _]
                      tunnel: w1788 -> [w1795 _]
                      frame True {
                        n1040 = stacked-sequence {
                          tunnel: w1797 -> [w1800 _]
                          tunnel: w1796 -> [_ w1805]
                          tunnel: w1795 -> [w1798 _]
                          frame #0 {
                            n1041 = Build Array("T-RISE") -> (w1802:string[])
                            n1042 = Build Array(w1800) -> (w1801:dbl[])
                            n1043 = TDMS Write(0:w1798, 5:"TEST PASS", 7:w1802, 9:w1801) -> (15:w1804:errorcluster)  [unwired: 2 in, 3 out]
                            n1044 = local write "data file error"(w1804) -> ()
                          }
                          frame #1 {
                            n1045 = Bundle(cluster=w1805, "STATUS"="T-RISE PASS") -> (w1807:T4)  [unwired: 2 in]
                            n1046 = local write "RESULT LAB01-1"(TRUE) -> ()
                            n1047 = local write "DISP LAB01-1"(w1807) -> ()
                          }
                        }
                      }
                      frame False {
                      }
                    }
                  }
                }
              }
              frame #1 {
                # "LAB01-2"
                n1048 = Equal?(x=w1810, y=2) -> (x = y?=w1813:bool)
                n1049 = local read "DISP LAB01-2"() -> (w1815:T4)
                n1050 = Unbundle(w1815) -> ("STATUS"=w1816:string)  [unwired: 2 out]
                n1051 = Equal?(x=w1816, y="RUN") -> (x = y?=w1812:bool)
                n1052 = And(x=w1812, y=w1813) -> (x .and. y?=w1811:bool)
                n1053 = case shown="True" w1811 {
                  tunnel: w1815 -> [_ w1819]
                  tunnel: w1809 -> [_ w1822]
                  frame False {
                  }
                  frame True {
                    n1054 = local read "SET LAB01-2"() -> (w1821:T5)
                    n1055 = local read "TDMS LAB01-2"() -> (w1818:refnum<k34>)
                    n1056 = Unbundle(w1819) -> ("CYCLE"=w1823:dbl)  [unwired: 2 out]
                    n1057 = Unbundle(w1821) -> ("T-RISE mins"=w1820:dbl)  [unwired: 4 out]
                    n1058 = Greater Or Equal?(x=w1823, y=w1822) -> (x >= y?=w1824:bool)
                    n1059 = case shown="True" w1824 {
                      tunnel: w1820 -> [w1827 _]
                      tunnel: w1819 -> [w1826 _]
                      tunnel: w1818 -> [w1825 _]
                      frame True {
                        n1060 = stacked-sequence {
                          tunnel: w1827 -> [w1830 _]
                          tunnel: w1826 -> [_ w1835]
                          tunnel: w1825 -> [w1828 _]
                          frame #0 {
                            n1061 = Build Array("T-RISE") -> (w1832:string[])
                            n1062 = Build Array(w1830) -> (w1831:dbl[])
                            n1063 = TDMS Write(0:w1828, 5:"TEST PASS", 7:w1832, 9:w1831) -> (15:w1834:errorcluster)  [unwired: 2 in, 3 out]
                            n1064 = local write "data file error"(w1834) -> ()
                          }
                          frame #1 {
                            n1065 = Bundle(cluster=w1835, "STATUS"="T-RISE PASS") -> (w1837:T4)  [unwired: 2 in]
                            n1066 = local write "RESULT LAB01-2"(TRUE) -> ()
                            n1067 = local write "DISP LAB01-2"(w1837) -> ()
                          }
                        }
                      }
                      frame False {
                      }
                    }
                  }
                }
              }
              frame #2 {
                # "LAB02-1"
                n1068 = Equal?(x=w1840, y=2) -> (x = y?=w1843:bool)
                n1069 = local read "DISP LAB02-1"() -> (w1845:T4)
                n1070 = Unbundle(w1845) -> ("STATUS"=w1846:string)  [unwired: 2 out]
                n1071 = Equal?(x=w1846, y="RUN") -> (x = y?=w1842:bool)
                n1072 = And(x=w1842, y=w1843) -> (x .and. y?=w1841:bool)
                n1073 = case shown="True" w1841 {
                  tunnel: w1845 -> [_ w1849]
                  tunnel: w1839 -> [_ w1852]
                  frame False {
                  }
                  frame True {
                    n1074 = local read "SET LAB02-1"() -> (w1851:T5)
                    n1075 = local read "TDMS LAB02-1"() -> (w1848:refnum<k34>)
                    n1076 = Unbundle(w1849) -> ("CYCLE"=w1853:dbl)  [unwired: 2 out]
                    n1077 = Unbundle(w1851) -> ("T-RISE mins"=w1850:dbl)  [unwired: 4 out]
                    n1078 = Greater Or Equal?(x=w1853, y=w1852) -> (x >= y?=w1854:bool)
                    n1079 = case shown="True" w1854 {
                      tunnel: w1850 -> [w1857 _]
                      tunnel: w1849 -> [w1856 _]
                      tunnel: w1848 -> [w1855 _]
                      frame True {
                        n1080 = stacked-sequence {
                          tunnel: w1857 -> [w1860 _]
                          tunnel: w1856 -> [_ w1865]
                          tunnel: w1855 -> [w1858 _]
                          frame #0 {
                            n1081 = Build Array("T-RISE") -> (w1862:string[])
                            n1082 = Build Array(w1860) -> (w1861:dbl[])
                            n1083 = TDMS Write(0:w1858, 5:"TEST PASS", 7:w1862, 9:w1861) -> (15:w1864:errorcluster)  [unwired: 2 in, 3 out]
                            n1084 = local write "data file error"(w1864) -> ()
                          }
                          frame #1 {
                            n1085 = Bundle(cluster=w1865, "STATUS"="T-RISE PASS") -> (w1867:T4)  [unwired: 2 in]
                            n1086 = local write "RESULT LAB02-1"(TRUE) -> ()
                            n1087 = local write "DISP LAB02-1"(w1867) -> ()
                          }
                        }
                      }
                      frame False {
                      }
                    }
                  }
                }
              }
              frame #3 {
                # "LAB02-2"
                n1088 = Equal?(x=w1870, y=2) -> (x = y?=w1873:bool)
                n1089 = local read "DISP LAB02-2"() -> (w1875:T4)
                n1090 = Unbundle(w1875) -> ("STATUS"=w1876:string)  [unwired: 2 out]
                n1091 = Equal?(x=w1876, y="RUN") -> (x = y?=w1872:bool)
                n1092 = And(x=w1872, y=w1873) -> (x .and. y?=w1871:bool)
                n1093 = case shown="True" w1871 {
                  tunnel: w1875 -> [_ w1879]
                  tunnel: w1869 -> [_ w1882]
                  frame False {
                  }
                  frame True {
                    n1094 = local read "SET LAB02-2"() -> (w1881:T5)
                    n1095 = local read "TDMS LAB02-2"() -> (w1878:refnum<k34>)
                    n1096 = Unbundle(w1879) -> ("CYCLE"=w1883:dbl)  [unwired: 2 out]
                    n1097 = Unbundle(w1881) -> ("T-RISE mins"=w1880:dbl)  [unwired: 4 out]
                    n1098 = Greater Or Equal?(x=w1883, y=w1882) -> (x >= y?=w1884:bool)
                    n1099 = case shown="True" w1884 {
                      tunnel: w1880 -> [w1887 _]
                      tunnel: w1879 -> [w1886 _]
                      tunnel: w1878 -> [w1885 _]
                      frame True {
                        n1100 = stacked-sequence {
                          tunnel: w1887 -> [w1890 _]
                          tunnel: w1886 -> [_ w1895]
                          tunnel: w1885 -> [w1888 _]
                          frame #0 {
                            n1101 = Build Array("T-RISE") -> (w1892:string[])
                            n1102 = Build Array(w1890) -> (w1891:dbl[])
                            n1103 = TDMS Write(0:w1888, 5:"TEST PASS", 7:w1892, 9:w1891) -> (15:w1894:errorcluster)  [unwired: 2 in, 3 out]
                            n1104 = local write "data file error"(w1894) -> ()
                          }
                          frame #1 {
                            n1105 = Bundle(cluster=w1895, "STATUS"="T-RISE PASS") -> (w1897:T4)  [unwired: 2 in]
                            n1106 = local write "RESULT LAB02-2"(TRUE) -> ()
                            n1107 = local write "DISP LAB02-2"(w1897) -> ()
                          }
                        }
                      }
                      frame False {
                      }
                    }
                  }
                }
              }
              frame #4 {
                # "LAB03-1"
                n1108 = Equal?(x=w1900, y=2) -> (x = y?=w1903:bool)
                n1109 = local read "DISP LAB03-1"() -> (w1905:T4)
                n1110 = Unbundle(w1905) -> ("STATUS"=w1906:string)  [unwired: 2 out]
                n1111 = Equal?(x=w1906, y="RUN") -> (x = y?=w1902:bool)
                n1112 = And(x=w1902, y=w1903) -> (x .and. y?=w1901:bool)
                n1113 = case shown="True" w1901 {
                  tunnel: w1905 -> [_ w1909]
                  tunnel: w1899 -> [_ w1912]
                  frame False {
                  }
                  frame True {
                    n1114 = local read "SET LAB03-1"() -> (w1911:T5)
                    n1115 = local read "TDMS LAB03-1"() -> (w1908:refnum<k34>)
                    n1116 = Unbundle(w1909) -> ("CYCLE"=w1913:dbl)  [unwired: 2 out]
                    n1117 = Unbundle(w1911) -> ("T-RISE mins"=w1910:dbl)  [unwired: 4 out]
                    n1118 = Greater Or Equal?(x=w1913, y=w1912) -> (x >= y?=w1914:bool)
                    n1119 = case shown="True" w1914 {
                      tunnel: w1910 -> [w1917 _]
                      tunnel: w1909 -> [w1916 _]
                      tunnel: w1908 -> [w1915 _]
                      frame True {
                        n1120 = stacked-sequence {
                          tunnel: w1917 -> [w1920 _]
                          tunnel: w1916 -> [_ w1925]
                          tunnel: w1915 -> [w1918 _]
                          frame #0 {
                            n1121 = Build Array("T-RISE") -> (w1922:string[])
                            n1122 = Build Array(w1920) -> (w1921:dbl[])
                            n1123 = TDMS Write(0:w1918, 5:"TEST PASS", 7:w1922, 9:w1921) -> (15:w1924:errorcluster)  [unwired: 2 in, 3 out]
                            n1124 = local write "data file error"(w1924) -> ()
                          }
                          frame #1 {
                            n1125 = Bundle(cluster=w1925, "STATUS"="T-RISE PASS") -> (w1927:T4)  [unwired: 2 in]
                            n1126 = local write "RESULT LAB03-1"(TRUE) -> ()
                            n1127 = local write "DISP LAB03-1"(w1927) -> ()
                          }
                        }
                      }
                      frame False {
                      }
                    }
                  }
                }
              }
              frame #5 {
                # "LAB03-2"
                n1128 = Equal?(x=w1930, y=2) -> (x = y?=w1933:bool)
                n1129 = local read "DISP LAB03-2"() -> (w1935:T4)
                n1130 = Unbundle(w1935) -> ("STATUS"=w1936:string)  [unwired: 2 out]
                n1131 = Equal?(x=w1936, y="RUN") -> (x = y?=w1932:bool)
                n1132 = And(x=w1932, y=w1933) -> (x .and. y?=w1931:bool)
                n1133 = case shown="True" w1931 {
                  tunnel: w1935 -> [_ w1939]
                  tunnel: w1929 -> [_ w1942]
                  frame False {
                  }
                  frame True {
                    n1134 = local read "SET LAB03-2"() -> (w1941:T5)
                    n1135 = local read "TDMS LAB03-2"() -> (w1938:refnum<k34>)
                    n1136 = Unbundle(w1939) -> ("CYCLE"=w1943:dbl)  [unwired: 2 out]
                    n1137 = Unbundle(w1941) -> ("T-RISE mins"=w1940:dbl)  [unwired: 4 out]
                    n1138 = Greater Or Equal?(x=w1943, y=w1942) -> (x >= y?=w1944:bool)
                    n1139 = case shown="True" w1944 {
                      tunnel: w1940 -> [w1947 _]
                      tunnel: w1939 -> [w1946 _]
                      tunnel: w1938 -> [w1945 _]
                      frame True {
                        n1140 = stacked-sequence {
                          tunnel: w1947 -> [w1950 _]
                          tunnel: w1946 -> [_ w1955]
                          tunnel: w1945 -> [w1948 _]
                          frame #0 {
                            n1141 = Build Array("T-RISE") -> (w1952:string[])
                            n1142 = Build Array(w1950) -> (w1951:dbl[])
                            n1143 = TDMS Write(0:w1948, 5:"TEST PASS", 7:w1952, 9:w1951) -> (15:w1954:errorcluster)  [unwired: 2 in, 3 out]
                            n1144 = local write "data file error"(w1954) -> ()
                          }
                          frame #1 {
                            n1145 = Bundle(cluster=w1955, "STATUS"="T-RISE PASS") -> (w1957:T4)  [unwired: 2 in]
                            n1146 = local write "RESULT LAB03-2"(TRUE) -> ()
                            n1147 = local write "DISP LAB03-2"(w1957) -> ()
                          }
                        }
                      }
                      frame False {
                      }
                    }
                  }
                }
              }
              frame #6 {
                # "LAB04-1"
                n1148 = Equal?(x=w1960, y=2) -> (x = y?=w1963:bool)
                n1149 = local read "DISP LAB04-1"() -> (w1965:T4)
                n1150 = Unbundle(w1965) -> ("STATUS"=w1966:string)  [unwired: 2 out]
                n1151 = Equal?(x=w1966, y="RUN") -> (x = y?=w1962:bool)
                n1152 = And(x=w1962, y=w1963) -> (x .and. y?=w1961:bool)
                n1153 = case shown="True" w1961 {
                  tunnel: w1965 -> [_ w1969]
                  tunnel: w1959 -> [_ w1972]
                  frame False {
                  }
                  frame True {
                    n1154 = local read "SET LAB04-1"() -> (w1971:T5)
                    n1155 = local read "TDMS LAB04-1"() -> (w1968:refnum<k34>)
                    n1156 = Unbundle(w1969) -> ("CYCLE"=w1973:dbl)  [unwired: 2 out]
                    n1157 = Unbundle(w1971) -> ("T-RISE mins"=w1970:dbl)  [unwired: 4 out]
                    n1158 = Greater Or Equal?(x=w1973, y=w1972) -> (x >= y?=w1974:bool)
                    n1159 = case shown="True" w1974 {
                      tunnel: w1970 -> [w1977 _]
                      tunnel: w1969 -> [w1976 _]
                      tunnel: w1968 -> [w1975 _]
                      frame True {
                        n1160 = stacked-sequence {
                          tunnel: w1977 -> [w1980 _]
                          tunnel: w1976 -> [_ w1985]
                          tunnel: w1975 -> [w1978 _]
                          frame #0 {
                            n1161 = Build Array("T-RISE") -> (w1982:string[])
                            n1162 = Build Array(w1980) -> (w1981:dbl[])
                            n1163 = TDMS Write(0:w1978, 5:"TEST PASS", 7:w1982, 9:w1981) -> (15:w1984:errorcluster)  [unwired: 2 in, 3 out]
                            n1164 = local write "data file error"(w1984) -> ()
                          }
                          frame #1 {
                            n1165 = Bundle(cluster=w1985, "STATUS"="T-RISE PASS") -> (w1987:T4)  [unwired: 2 in]
                            n1166 = local write "RESULT LAB04-1"(TRUE) -> ()
                            n1167 = local write "DISP LAB04-1"(w1987) -> ()
                          }
                        }
                      }
                      frame False {
                      }
                    }
                  }
                }
              }
              frame #7 {
                # "LAB04-2"
                n1168 = Equal?(x=w1990, y=2) -> (x = y?=w1993:bool)
                n1169 = local read "DISP LAB04-2"() -> (w1995:T4)
                n1170 = Unbundle(w1995) -> ("STATUS"=w1996:string)  [unwired: 2 out]
                n1171 = Equal?(x=w1996, y="RUN") -> (x = y?=w1992:bool)
                n1172 = And(x=w1992, y=w1993) -> (x .and. y?=w1991:bool)
                n1173 = case shown="True" w1991 {
                  tunnel: w1995 -> [_ w1999]
                  tunnel: w1989 -> [_ w2002]
                  frame False {
                  }
                  frame True {
                    n1174 = local read "SET LAB04-2"() -> (w2001:T5)
                    n1175 = local read "TDMS LAB04-2"() -> (w1998:refnum<k34>)
                    n1176 = Unbundle(w1999) -> ("CYCLE"=w2003:dbl)  [unwired: 2 out]
                    n1177 = Unbundle(w2001) -> ("T-RISE mins"=w2000:dbl)  [unwired: 4 out]
                    n1178 = Greater Or Equal?(x=w2003, y=w2002) -> (x >= y?=w2004:bool)
                    n1179 = case shown="True" w2004 {
                      tunnel: w2000 -> [w2007 _]
                      tunnel: w1999 -> [w2006 _]
                      tunnel: w1998 -> [w2005 _]
                      frame True {
                        n1180 = stacked-sequence {
                          tunnel: w2007 -> [w2010 _]
                          tunnel: w2006 -> [_ w2015]
                          tunnel: w2005 -> [w2008 _]
                          frame #0 {
                            n1181 = Build Array("T-RISE") -> (w2012:string[])
                            n1182 = Build Array(w2010) -> (w2011:dbl[])
                            n1183 = TDMS Write(0:w2008, 5:"TEST PASS", 7:w2012, 9:w2011) -> (15:w2014:errorcluster)  [unwired: 2 in, 3 out]
                            n1184 = local write "data file error"(w2014) -> ()
                          }
                          frame #1 {
                            n1185 = Bundle(cluster=w2015, "STATUS"="T-RISE PASS") -> (w2017:T4)  [unwired: 2 in]
                            n1186 = local write "RESULT LAB04-2"(TRUE) -> ()
                            n1187 = local write "DISP LAB04-2"(w2017) -> ()
                          }
                        }
                      }
                      frame False {
                      }
                    }
                  }
                }
              }
              frame #8 {
                # "LAB05-1"
                n1188 = Equal?(x=w2020, y=2) -> (x = y?=w2023:bool)
                n1189 = local read "DISP LAB05-1"() -> (w2025:T4)
                n1190 = Unbundle(w2025) -> ("STATUS"=w2026:string)  [unwired: 2 out]
                n1191 = Equal?(x=w2026, y="RUN") -> (x = y?=w2022:bool)
                n1192 = And(x=w2022, y=w2023) -> (x .and. y?=w2021:bool)
                n1193 = case shown="True" w2021 {
                  tunnel: w2025 -> [_ w2029]
                  tunnel: w2019 -> [_ w2032]
                  frame False {
                  }
                  frame True {
                    n1194 = local read "SET LAB05-1"() -> (w2031:T5)
                    n1195 = local read "TDMS LAB05-1"() -> (w2028:refnum<k34>)
                    n1196 = Unbundle(w2029) -> ("CYCLE"=w2033:dbl)  [unwired: 2 out]
                    n1197 = Unbundle(w2031) -> ("T-RISE mins"=w2030:dbl)  [unwired: 4 out]
                    n1198 = Greater Or Equal?(x=w2033, y=w2032) -> (x >= y?=w2034:bool)
                    n1199 = case shown="True" w2034 {
                      tunnel: w2030 -> [w2037 _]
                      tunnel: w2029 -> [w2036 _]
                      tunnel: w2028 -> [w2035 _]
                      frame True {
                        n1200 = stacked-sequence {
                          tunnel: w2037 -> [w2040 _]
                          tunnel: w2036 -> [_ w2045]
                          tunnel: w2035 -> [w2038 _]
                          frame #0 {
                            n1201 = Build Array("T-RISE") -> (w2042:string[])
                            n1202 = Build Array(w2040) -> (w2041:dbl[])
                            n1203 = TDMS Write(0:w2038, 5:"TEST PASS", 7:w2042, 9:w2041) -> (15:w2044:errorcluster)  [unwired: 2 in, 3 out]
                            n1204 = local write "data file error"(w2044) -> ()
                          }
                          frame #1 {
                            n1205 = Bundle(cluster=w2045, "STATUS"="T-RISE PASS") -> (w2047:T4)  [unwired: 2 in]
                            n1206 = local write "RESULT LAB05-1"(TRUE) -> ()
                            n1207 = local write "DISP LAB05-1"(w2047) -> ()
                          }
                        }
                      }
                      frame False {
                      }
                    }
                  }
                }
              }
              frame #9 {
                # "LAB05-2"
                n1208 = Equal?(x=w2050, y=2) -> (x = y?=w2053:bool)
                n1209 = local read "DISP LAB05-2"() -> (w2055:T4)
                n1210 = Unbundle(w2055) -> ("STATUS"=w2056:string)  [unwired: 2 out]
                n1211 = Equal?(x=w2056, y="RUN") -> (x = y?=w2052:bool)
                n1212 = And(x=w2052, y=w2053) -> (x .and. y?=w2051:bool)
                n1213 = case shown="True" w2051 {
                  tunnel: w2055 -> [_ w2059]
                  tunnel: w2049 -> [_ w2062]
                  frame False {
                  }
                  frame True {
                    n1214 = local read "SET LAB05-2"() -> (w2061:T5)
                    n1215 = local read "TDMS LAB05-2"() -> (w2058:refnum<k34>)
                    n1216 = Unbundle(w2059) -> ("CYCLE"=w2063:dbl)  [unwired: 2 out]
                    n1217 = Unbundle(w2061) -> ("T-RISE mins"=w2060:dbl)  [unwired: 4 out]
                    n1218 = Greater Or Equal?(x=w2063, y=w2062) -> (x >= y?=w2064:bool)
                    n1219 = case shown="True" w2064 {
                      tunnel: w2060 -> [w2067 _]
                      tunnel: w2059 -> [w2066 _]
                      tunnel: w2058 -> [w2065 _]
                      frame True {
                        n1220 = stacked-sequence {
                          tunnel: w2067 -> [w2070 _]
                          tunnel: w2066 -> [_ w2075]
                          tunnel: w2065 -> [w2068 _]
                          frame #0 {
                            n1221 = Build Array("T-RISE") -> (w2072:string[])
                            n1222 = Build Array(w2070) -> (w2071:dbl[])
                            n1223 = TDMS Write(0:w2068, 5:"TEST PASS", 7:w2072, 9:w2071) -> (15:w2074:errorcluster)  [unwired: 2 in, 3 out]
                            n1224 = local write "data file error"(w2074) -> ()
                          }
                          frame #1 {
                            n1225 = Bundle(cluster=w2075, "STATUS"="T-RISE PASS") -> (w2077:T4)  [unwired: 2 in]
                            n1226 = local write "RESULT LAB05-2"(TRUE) -> ()
                            n1227 = local write "DISP LAB05-2"(w2077) -> ()
                          }
                        }
                      }
                      frame False {
                      }
                    }
                  }
                }
              }
            }
          }
          frame #6 {
            # "end test & close test files"
            n1228 = stacked-sequence {
              tunnel: w2088 -> [_ _ _ _ _ _ _ _ _ _]
              tunnel: w2089 -> [_ _ _ _ _ _ _ _ _ _]
              tunnel: w2087 -> [_ _ _ _ _ _ _ _ _ _]
              tunnel: w2086 -> [_ _ _ _ _ _ _ _ _ _]
              tunnel: w2085 -> [_ _ _ _ _ _ _ _ _ _]
              tunnel: w2084 -> [_ _ _ _ _ _ _ _ _ _]
              tunnel: w2083 -> [_ _ _ _ _ _ _ _ _ _]
              tunnel: w2082 -> [_ _ _ _ _ _ _ _ _ _]
              tunnel: w2081 -> [_ _ _ _ _ _ _ _ _ _]
              tunnel: w2080 -> [_ _ _ _ _ _ _ _ _ _]
              frame #0 {
                # "LAB01-1"
                n1229 = local read "DISP LAB01-1"() -> (w2093:T4)
                n1230 = local read "run lab01-1"() -> (w2090:bool)
                n1231 = local read "TDMS LAB01-1"() -> (w2091:refnum<k34>)
                n1232 = Unbundle(w2093) -> ("CYCLE"=w2094:dbl, "STATUS"=w2092:string)  [unwired: 1 out]
                n1233 = case shown="True" w2090 {
                  tunnel: w2094 -> [_ w2098]
                  tunnel: w2093 -> [_ w2097]
                  tunnel: w2092 -> [_ w2096]
                  tunnel: w2091 -> [_ w2095]
                  frame False {
                  }
                  frame True {
                    n1234 = Not Equal?(x=w2096, y="RUN") -> (x != y?=w2099:bool)
                    n1235 = Greater?(x=w2098, y=2.0) -> (0:w2101:bool)
                    n1236 = And(x=w2101, y=w2099) -> (x .and. y?=w2100:bool)
                    n1237 = case shown="True" w2100 {
                      tunnel: w2097 -> [_ w2105]
                      tunnel: w2095 -> [_ w2104]
                      frame False {
                      }
                      frame True {
                        n1238 = stacked-sequence {
                          tunnel: w2105 -> [w2109 _ _]
                          tunnel: w2104 -> [_ w2111 _]
                          frame #0 {
                            w2106 = FALSE
                            n1239 = local write "mail control"("END") -> ()
                            n1240 = Bundle(cluster=w2109) -> (w2108:T4)  [unwired: 3 in]
                            n1241 = local write "DISP LAB01-1"(w2108) -> ()
                            n1242 = local write "O/I  LAB01-1"(w2106) -> ()
                            n1243 = local write "run lab01-1"(w2106) -> ()
                            n1244 = local write "RUN LAB01-1"(w2106) -> ()
                          }
                          frame #1 {
                            n1245 = TDMS Close(11:w2111) -> (0:w2110:errorcluster)  [unwired: 1 in, 1 out]
                            n1246 = local write "data file error"(w2110) -> ()
                          }
                          frame #2 {
                            n1247 = stacked-sequence {
                              tunnel: "LAB01-1" -> [w2114 w2116]
                              frame #0 {
                                n1248 = call "sub vi - defrag tdms v1.vi"("panel id"=w2114) -> ("error out"=w2113:errorcluster)  [unwired: 10 in]
                                n1249 = local write "data file error"(w2113) -> ()
                              }
                              frame #1 {
                                n1250 = call "Save data file to network drive v1.vi"("panel id"=w2116) -> ("network file save error"=w2115:errorcluster)  [unwired: 9 in, 1 out]
                                n1251 = local write "data file error"(w2115) -> ()
                              }
                            }
                          }
                        }
                      }
                    }
                  }
                }
              }
              frame #1 {
                # "LAB01-2"
                n1252 = local read "run lab01-2"() -> (w2117:bool)
                n1253 = case shown="True" w2117 {
                  frame False {
                  }
                  frame True {
                    n1254 = local read "DISP LAB01-2"() -> (w2124:T4)
                    n1255 = local read "TDMS LAB01-2"() -> (w2123:refnum<k34>)
                    n1256 = Unbundle(w2124) -> ("CYCLE"=w2120:dbl, "STATUS"=w2125:string)  [unwired: 1 out]
                    n1257 = Not Equal?(x=w2125, y="RUN") -> (x != y?=w2119:bool)
                    n1258 = Greater?(x=w2120, y=2.0) -> (0:w2121:bool)
                    n1259 = And(x=w2121, y=w2119) -> (x .and. y?=w2118:bool)
                    n1260 = case shown="True" w2118 {
                      tunnel: w2124 -> [_ w2128]
                      tunnel: w2123 -> [_ w2127]
                      frame False {
                      }
                      frame True {
                        n1261 = stacked-sequence {
                          tunnel: w2128 -> [w2131 _ _]
                          tunnel: w2127 -> [_ w2133 _]
                          frame #0 {
                            w2129 = FALSE
                            n1262 = local write "mail control"("END") -> ()
                            n1263 = Bundle(cluster=w2131) -> (w2132:T4)  [unwired: 3 in]
                            n1264 = local write "RUN LAB01-2"(w2129) -> ()
                            n1265 = local write "run lab01-2"(w2129) -> ()
                            n1266 = local write "O/I  LAB01-2"(w2129) -> ()
                            n1267 = local write "DISP LAB01-2"(w2132) -> ()
                          }
                          frame #1 {
                            n1268 = TDMS Close(11:w2133) -> (0:w2134:errorcluster)  [unwired: 1 in, 1 out]
                            n1269 = local write "data file error"(w2134) -> ()
                          }
                          frame #2 {
                            n1270 = stacked-sequence {
                              tunnel: "LAB01-2" -> [w2137 w2139]
                              frame #0 {
                                n1271 = call "sub vi - defrag tdms v1.vi"("panel id"=w2137) -> ("error out"=w2136:errorcluster)  [unwired: 10 in]
                                n1272 = local write "data file error"(w2136) -> ()
                              }
                              frame #1 {
                                n1273 = call "Save data file to network drive v1.vi"("panel id"=w2139) -> ("network file save error"=w2138:errorcluster)  [unwired: 9 in, 1 out]
                                n1274 = local write "data file error"(w2138) -> ()
                              }
                            }
                          }
                        }
                      }
                    }
                  }
                }
              }
              frame #2 {
                # "LAB02-1"
                n1275 = local read "run lab02-1"() -> (w2140:bool)
                n1276 = case shown="True" w2140 {
                  frame False {
                  }
                  frame True {
                    n1277 = local read "DISP LAB02-1"() -> (w2147:T4)
                    n1278 = Unbundle(w2147) -> ("CYCLE"=w2143:dbl, "STATUS"=w2148:string)  [unwired: 1 out]
                    n1279 = local read "TDMS LAB02-1"() -> (w2146:refnum<k34>)
                    n1280 = Not Equal?(x=w2148, y="RUN") -> (x != y?=w2142:bool)
                    n1281 = Greater?(x=w2143, y=2.0) -> (0:w2144:bool)
                    n1282 = And(x=w2144, y=w2142) -> (x .and. y?=w2141:bool)
                    n1283 = case shown="True" w2141 {
                      tunnel: w2147 -> [_ w2151]
                      tunnel: w2146 -> [_ w2150]
                      frame False {
                      }
                      frame True {
                        n1284 = stacked-sequence {
                          tunnel: w2151 -> [w2154 _ _]
                          tunnel: w2150 -> [_ w2156 _]
                          frame #0 {
                            w2152 = FALSE
                            n1285 = local write "mail control"("END") -> ()
                            n1286 = Bundle(cluster=w2154) -> (w2155:T4)  [unwired: 3 in]
                            n1287 = local write "O/I  LAB02-1"(w2152) -> ()
                            n1288 = local write "RUN LAB02-1"(w2152) -> ()
                            n1289 = local write "run lab02-1"(w2152) -> ()
                            n1290 = local write "DISP LAB02-1"(w2155) -> ()
                          }
                          frame #1 {
                            n1291 = TDMS Close(11:w2156) -> (0:w2157:errorcluster)  [unwired: 1 in, 1 out]
                            n1292 = local write "data file error"(w2157) -> ()
                          }
                          frame #2 {
                            n1293 = stacked-sequence {
                              tunnel: "LAB02-1" -> [w2160 w2162]
                              frame #0 {
                                n1294 = call "sub vi - defrag tdms v1.vi"("panel id"=w2160) -> ("error out"=w2159:errorcluster)  [unwired: 10 in]
                                n1295 = local write "data file error"(w2159) -> ()
                              }
                              frame #1 {
                                n1296 = call "Save data file to network drive v1.vi"("panel id"=w2162) -> ("network file save error"=w2161:errorcluster)  [unwired: 9 in, 1 out]
                                n1297 = local write "data file error"(w2161) -> ()
                              }
                            }
                          }
                        }
                      }
                    }
                  }
                }
              }
              frame #3 {
                # "LAB02-2"
                n1298 = local read "run lab02-2"() -> (w2163:bool)
                n1299 = case shown="True" w2163 {
                  frame False {
                  }
                  frame True {
                    n1300 = local read "DISP LAB02-2"() -> (w2170:T4)
                    n1301 = local read "TDMS LAB02-2"() -> (w2169:refnum<k34>)
                    n1302 = Unbundle(w2170) -> ("CYCLE"=w2166:dbl, "STATUS"=w2171:string)  [unwired: 1 out]
                    n1303 = Not Equal?(x=w2171, y="RUN") -> (x != y?=w2165:bool)
                    n1304 = Greater?(x=w2166, y=2.0) -> (0:w2167:bool)
                    n1305 = And(x=w2167, y=w2165) -> (x .and. y?=w2164:bool)
                    n1306 = case shown="True" w2164 {
                      tunnel: w2170 -> [_ w2174]
                      tunnel: w2169 -> [_ w2173]
                      frame False {
                      }
                      frame True {
                        n1307 = stacked-sequence {
                          tunnel: w2174 -> [w2177 _ _]
                          tunnel: w2173 -> [_ w2179 _]
                          frame #0 {
                            w2175 = FALSE
                            n1308 = local write "mail control"("END") -> ()
                            n1309 = Bundle(cluster=w2177) -> (w2178:T4)  [unwired: 3 in]
                            n1310 = local write "O/I  LAB02-2"(w2175) -> ()
                            n1311 = local write "run lab02-2"(w2175) -> ()
                            n1312 = local write "RUN LAB02-2"(w2175) -> ()
                            n1313 = local write "DISP LAB02-2"(w2178) -> ()
                          }
                          frame #1 {
                            n1314 = TDMS Close(11:w2179) -> (0:w2180:errorcluster)  [unwired: 1 in, 1 out]
                            n1315 = local write "data file error"(w2180) -> ()
                          }
                          frame #2 {
                            n1316 = stacked-sequence {
                              tunnel: "LAB02-2" -> [w2183 w2185]
                              frame #0 {
                                n1317 = call "sub vi - defrag tdms v1.vi"("panel id"=w2183) -> ("error out"=w2182:errorcluster)  [unwired: 10 in]
                                n1318 = local write "data file error"(w2182) -> ()
                              }
                              frame #1 {
                                n1319 = call "Save data file to network drive v1.vi"("panel id"=w2185) -> ("network file save error"=w2184:errorcluster)  [unwired: 9 in, 1 out]
                                n1320 = local write "data file error"(w2184) -> ()
                              }
                            }
                          }
                        }
                      }
                    }
                  }
                }
              }
              frame #4 {
                # "LAB03-1"
                n1321 = local read "run lab03-1"() -> (w2186:bool)
                n1322 = case shown="True" w2186 {
                  frame False {
                  }
                  frame True {
                    n1323 = local read "DISP LAB03-1"() -> (w2193:T4)
                    n1324 = local read "TDMS LAB03-1"() -> (w2192:refnum<k34>)
                    n1325 = Unbundle(w2193) -> ("CYCLE"=w2189:dbl, "STATUS"=w2194:string)  [unwired: 1 out]
                    n1326 = Not Equal?(x=w2194, y="RUN") -> (x != y?=w2188:bool)
                    n1327 = Greater?(x=w2189, y=2.0) -> (0:w2190:bool)
                    n1328 = And(x=w2190, y=w2188) -> (x .and. y?=w2187:bool)
                    n1329 = case shown="True" w2187 {
                      tunnel: w2193 -> [_ w2197]
                      tunnel: w2192 -> [_ w2196]
                      frame False {
                      }
                      frame True {
                        n1330 = stacked-sequence {
                          tunnel: w2197 -> [w2200 _ _]
                          tunnel: w2196 -> [_ w2202 _]
                          frame #0 {
                            w2198 = FALSE
                            n1331 = local write "mail control"("END") -> ()
                            n1332 = Bundle(cluster=w2200) -> (w2201:T4)  [unwired: 3 in]
                            n1333 = local write "O/I  LAB03-1"(w2198) -> ()
                            n1334 = local write "run lab03-1"(w2198) -> ()
                            n1335 = local write "RUN LAB03-1"(w2198) -> ()
                            n1336 = local write "DISP LAB03-1"(w2201) -> ()
                          }
                          frame #1 {
                            n1337 = TDMS Close(11:w2202) -> (0:w2203:errorcluster)  [unwired: 1 in, 1 out]
                            n1338 = local write "data file error"(w2203) -> ()
                          }
                          frame #2 {
                            n1339 = stacked-sequence {
                              tunnel: "LAB03-1" -> [w2206 w2208]
                              frame #0 {
                                n1340 = call "sub vi - defrag tdms v1.vi"("panel id"=w2206) -> ("error out"=w2205:errorcluster)  [unwired: 10 in]
                                n1341 = local write "data file error"(w2205) -> ()
                              }
                              frame #1 {
                                n1342 = call "Save data file to network drive v1.vi"("panel id"=w2208) -> ("network file save error"=w2207:errorcluster)  [unwired: 9 in, 1 out]
                                n1343 = local write "data file error"(w2207) -> ()
                              }
                            }
                          }
                        }
                      }
                    }
                  }
                }
              }
              frame #5 {
                # "LAB03-2"
                n1344 = local read "run lab03-2"() -> (w2209:bool)
                n1345 = case shown="True" w2209 {
                  frame False {
                  }
                  frame True {
                    n1346 = local read "DISP LAB03-2"() -> (w2216:T4)
                    n1347 = Unbundle(w2216) -> ("CYCLE"=w2212:dbl, "STATUS"=w2217:string)  [unwired: 1 out]
                    n1348 = local read "TDMS LAB03-2"() -> (w2215:refnum<k34>)
                    n1349 = Not Equal?(x=w2217, y="RUN") -> (x != y?=w2211:bool)
                    n1350 = Greater?(x=w2212, y=2.0) -> (0:w2213:bool)
                    n1351 = And(x=w2213, y=w2211) -> (x .and. y?=w2210:bool)
                    n1352 = case shown="True" w2210 {
                      tunnel: w2216 -> [_ w2220]
                      tunnel: w2215 -> [_ w2219]
                      frame False {
                      }
                      frame True {
                        n1353 = stacked-sequence {
                          tunnel: w2220 -> [w2223 _ _]
                          tunnel: w2219 -> [_ w2225 _]
                          frame #0 {
                            w2221 = FALSE
                            n1354 = local write "mail control"("END") -> ()
                            n1355 = Bundle(cluster=w2223) -> (w2224:T4)  [unwired: 3 in]
                            n1356 = local write "RUN LAB03-2"(w2221) -> ()
                            n1357 = local write "O/I  LAB03-2"(w2221) -> ()
                            n1358 = local write "DISP LAB03-2"(w2224) -> ()
                            n1359 = local write "run lab03-2"(w2221) -> ()
                          }
                          frame #1 {
                            n1360 = TDMS Close(11:w2225) -> (0:w2226:errorcluster)  [unwired: 1 in, 1 out]
                            n1361 = local write "data file error"(w2226) -> ()
                          }
                          frame #2 {
                            n1362 = stacked-sequence {
                              tunnel: "LAB03-2" -> [w2229 w2231]
                              frame #0 {
                                n1363 = call "sub vi - defrag tdms v1.vi"("panel id"=w2229) -> ("error out"=w2228:errorcluster)  [unwired: 10 in]
                                n1364 = local write "data file error"(w2228) -> ()
                              }
                              frame #1 {
                                n1365 = call "Save data file to network drive v1.vi"("panel id"=w2231) -> ("network file save error"=w2230:errorcluster)  [unwired: 9 in, 1 out]
                                n1366 = local write "data file error"(w2230) -> ()
                              }
                            }
                          }
                        }
                      }
                    }
                  }
                }
              }
              frame #6 {
                # "LAB04-1"
                n1367 = local read "run lab04-1"() -> (w2232:bool)
                n1368 = case shown="True" w2232 {
                  frame False {
                  }
                  frame True {
                    n1369 = local read "DISP LAB04-1"() -> (w2239:T4)
                    n1370 = Unbundle(w2239) -> ("CYCLE"=w2235:dbl, "STATUS"=w2240:string)  [unwired: 1 out]
                    n1371 = local read "TDMS LAB04-1"() -> (w2238:refnum<k34>)
                    n1372 = Not Equal?(x=w2240, y="RUN") -> (x != y?=w2234:bool)
                    n1373 = Greater?(x=w2235, y=2.0) -> (0:w2236:bool)
                    n1374 = And(x=w2236, y=w2234) -> (x .and. y?=w2233:bool)
                    n1375 = case shown="True" w2233 {
                      tunnel: w2239 -> [_ w2243]
                      tunnel: w2238 -> [_ w2242]
                      frame False {
                      }
                      frame True {
                        n1376 = stacked-sequence {
                          tunnel: w2243 -> [w2246 _ _]
                          tunnel: w2242 -> [_ w2248 _]
                          frame #0 {
                            w2244 = FALSE
                            n1377 = local write "mail control"("END") -> ()
                            n1378 = Bundle(cluster=w2246) -> (w2247:T4)  [unwired: 3 in]
                            n1379 = local write "RUN LAB04-1"(w2244) -> ()
                            n1380 = local write "O/I  LAB04-1"(w2244) -> ()
                            n1381 = local write "run lab04-1"(w2244) -> ()
                            n1382 = local write "DISP LAB04-1"(w2247) -> ()
                          }
                          frame #1 {
                            n1383 = TDMS Close(11:w2248) -> (0:w2249:errorcluster)  [unwired: 1 in, 1 out]
                            n1384 = local write "data file error"(w2249) -> ()
                          }
                          frame #2 {
                            n1385 = stacked-sequence {
                              tunnel: "LAB04-1" -> [w2252 w2254]
                              frame #0 {
                                n1386 = call "sub vi - defrag tdms v1.vi"("panel id"=w2252) -> ("error out"=w2251:errorcluster)  [unwired: 10 in]
                                n1387 = local write "data file error"(w2251) -> ()
                              }
                              frame #1 {
                                n1388 = call "Save data file to network drive v1.vi"("panel id"=w2254) -> ("network file save error"=w2253:errorcluster)  [unwired: 9 in, 1 out]
                                n1389 = local write "data file error"(w2253) -> ()
                              }
                            }
                          }
                        }
                      }
                    }
                  }
                }
              }
              frame #7 {
                # "LAB04-2"
                n1390 = local read "run lab04-2"() -> (w2255:bool)
                n1391 = case shown="True" w2255 {
                  frame False {
                  }
                  frame True {
                    n1392 = local read "DISP LAB04-2"() -> (w2262:T4)
                    n1393 = Unbundle(w2262) -> ("CYCLE"=w2258:dbl, "STATUS"=w2263:string)  [unwired: 1 out]
                    n1394 = Not Equal?(x=w2263, y="RUN") -> (x != y?=w2257:bool)
                    n1395 = local read "TDMS LAB04-2"() -> (w2261:refnum<k34>)
                    n1396 = Greater?(x=w2258, y=2.0) -> (0:w2259:bool)
                    n1397 = And(x=w2259, y=w2257) -> (x .and. y?=w2256:bool)
                    n1398 = case shown="True" w2256 {
                      tunnel: w2262 -> [_ w2266]
                      tunnel: w2261 -> [_ w2265]
                      frame False {
                      }
                      frame True {
                        n1399 = stacked-sequence {
                          tunnel: w2266 -> [w2269 _ _]
                          tunnel: w2265 -> [_ w2271 _]
                          frame #0 {
                            w2267 = FALSE
                            n1400 = local write "mail control"("END") -> ()
                            n1401 = Bundle(cluster=w2269) -> (w2270:T4)  [unwired: 3 in]
                            n1402 = local write "O/I  LAB04-2"(w2267) -> ()
                            n1403 = local write "RUN LAB04-2"(w2267) -> ()
                            n1404 = local write "run lab04-2"(w2267) -> ()
                            n1405 = local write "DISP LAB04-2"(w2270) -> ()
                          }
                          frame #1 {
                            n1406 = TDMS Close(11:w2271) -> (0:w2272:errorcluster)  [unwired: 1 in, 1 out]
                            n1407 = local write "data file error"(w2272) -> ()
                          }
                          frame #2 {
                            n1408 = stacked-sequence {
                              tunnel: "LAB04-2" -> [w2275 w2277]
                              frame #0 {
                                n1409 = call "sub vi - defrag tdms v1.vi"("panel id"=w2275) -> ("error out"=w2274:errorcluster)  [unwired: 10 in]
                                n1410 = local write "data file error"(w2274) -> ()
                              }
                              frame #1 {
                                n1411 = call "Save data file to network drive v1.vi"("panel id"=w2277) -> ("network file save error"=w2276:errorcluster)  [unwired: 9 in, 1 out]
                                n1412 = local write "data file error"(w2276) -> ()
                              }
                            }
                          }
                        }
                      }
                    }
                  }
                }
              }
              frame #8 {
                # "LAB05-1"
                n1413 = local read "run lab05-1"() -> (w2278:bool)
                n1414 = case shown="True" w2278 {
                  frame False {
                  }
                  frame True {
                    n1415 = local read "DISP LAB05-1"() -> (w2285:T4)
                    n1416 = Unbundle(w2285) -> ("CYCLE"=w2281:dbl, "STATUS"=w2286:string)  [unwired: 1 out]
                    n1417 = Not Equal?(x=w2286, y="RUN") -> (x != y?=w2280:bool)
                    n1418 = local read "TDMS LAB05-1"() -> (w2284:refnum<k34>)
                    n1419 = Greater?(x=w2281, y=2.0) -> (0:w2282:bool)
                    n1420 = And(x=w2282, y=w2280) -> (x .and. y?=w2279:bool)
                    n1421 = case shown="True" w2279 {
                      tunnel: w2285 -> [_ w2289]
                      tunnel: w2284 -> [_ w2288]
                      frame False {
                      }
                      frame True {
                        n1422 = stacked-sequence {
                          tunnel: w2289 -> [w2292 _ _]
                          tunnel: w2288 -> [_ w2294 _]
                          frame #0 {
                            w2290 = FALSE
                            n1423 = local write "mail control"("END") -> ()
                            n1424 = Bundle(cluster=w2292) -> (w2293:T4)  [unwired: 3 in]
                            n1425 = local write "O/I  LAB05-1"(w2290) -> ()
                            n1426 = local write "RUN LAB05-1"(w2290) -> ()
                            n1427 = local write "run lab05-1"(w2290) -> ()
                            n1428 = local write "DISP LAB05-1"(w2293) -> ()
                          }
                          frame #1 {
                            n1429 = TDMS Close(11:w2294) -> (0:w2295:errorcluster)  [unwired: 1 in, 1 out]
                            n1430 = local write "data file error"(w2295) -> ()
                          }
                          frame #2 {
                            n1431 = stacked-sequence {
                              tunnel: "LAB05-1" -> [w2298 w2300]
                              frame #0 {
                                n1432 = call "sub vi - defrag tdms v1.vi"("panel id"=w2298) -> ("error out"=w2297:errorcluster)  [unwired: 10 in]
                                n1433 = local write "data file error"(w2297) -> ()
                              }
                              frame #1 {
                                n1434 = call "Save data file to network drive v1.vi"("panel id"=w2300) -> ("network file save error"=w2299:errorcluster)  [unwired: 9 in, 1 out]
                                n1435 = local write "data file error"(w2299) -> ()
                              }
                            }
                          }
                        }
                      }
                    }
                  }
                }
              }
              frame #9 {
                # "LAB05-2"
                n1436 = local read "run lab05-2"() -> (w2301:bool)
                n1437 = case shown="True" w2301 {
                  frame False {
                  }
                  frame True {
                    n1438 = local read "DISP LAB05-2"() -> (w2308:T4)
                    n1439 = Unbundle(w2308) -> ("CYCLE"=w2304:dbl, "STATUS"=w2309:string)  [unwired: 1 out]
                    n1440 = Not Equal?(x=w2309, y="RUN") -> (x != y?=w2303:bool)
                    n1441 = local read "TDMS LAB05-2"() -> (w2307:refnum<k34>)
                    n1442 = Greater?(x=w2304, y=2.0) -> (0:w2305:bool)
                    n1443 = And(x=w2305, y=w2303) -> (x .and. y?=w2302:bool)
                    n1444 = case shown="True" w2302 {
                      tunnel: w2308 -> [_ w2312]
                      tunnel: w2307 -> [_ w2311]
                      frame False {
                      }
                      frame True {
                        n1445 = stacked-sequence {
                          tunnel: w2312 -> [w2315 _ _]
                          tunnel: w2311 -> [_ w2317 _]
                          frame #0 {
                            w2313 = FALSE
                            n1446 = local write "mail control"("END") -> ()
                            n1447 = Bundle(cluster=w2315) -> (w2316:T4)  [unwired: 3 in]
                            n1448 = local write "RUN LAB05-2"(w2313) -> ()
                            n1449 = local write "O/I  LAB05-2"(w2313) -> ()
                            n1450 = local write "run lab05-2"(w2313) -> ()
                            n1451 = local write "DISP LAB05-2"(w2316) -> ()
                          }
                          frame #1 {
                            n1452 = TDMS Close(11:w2317) -> (0:w2318:errorcluster)  [unwired: 1 in, 1 out]
                            n1453 = local write "data file error"(w2318) -> ()
                          }
                          frame #2 {
                            n1454 = stacked-sequence {
                              tunnel: "LAB05-2" -> [w2321 w2323]
                              frame #0 {
                                n1455 = call "sub vi - defrag tdms v1.vi"("panel id"=w2321) -> ("error out"=w2320:errorcluster)  [unwired: 10 in]
                                n1456 = local write "data file error"(w2320) -> ()
                              }
                              frame #1 {
                                n1457 = call "Save data file to network drive v1.vi"("panel id"=w2323) -> ("network file save error"=w2322:errorcluster)  [unwired: 9 in, 1 out]
                                n1458 = local write "data file error"(w2322) -> ()
                              }
                            }
                          }
                        }
                      }
                    }
                  }
                }
              }
            }
            n1459 = local read "Network Directory"() -> (w2079:path)
            n1460 = global write "Global 1.vi" "Network Drive"(w2079) -> ()
          }
          frame #7 {
            # "disable functions"
            n1461 = stacked-sequence {
              tunnel: w2333 -> [w2347 _ w2403]
              tunnel: w2332 -> [w2342 _ w2402]
              tunnel: w2331 -> [w2341 _ w2401]
              tunnel: w2330 -> [w2339 _ w2400]
              tunnel: w2329 -> [w2340 _ w2399]
              tunnel: w2328 -> [_ w2364 w2398]
              tunnel: w2327 -> [_ w2365 w2397]
              tunnel: w2326 -> [_ w2366 w2396]
              tunnel: w2325 -> [_ w2367 w2395]
              tunnel: w2324 -> [_ w2368 w2394]
              frame #0 {
                n1462 = Select(t=2, s=w2339, f=0) -> (s? t:f=w2335:i32)
                n1463 = Select(t=2, s=w2341, f=0) -> (s? t:f=w2336:i32)
                n1464 = Select(t=2, s=w2340, f=0) -> (s? t:f=w2334:i32)
                n1465 = Select(t=2, s=w2347, f=0) -> (s? t:f=w2338:i32)
                n1466 = Select(t=2, s=w2342, f=0) -> (s? t:f=w2337:i32)
                n1467 = property on="SELECT LAB02-2" class="RadioBtnsControl (strict)"("DisabledEnum"=w2335) -> ()  [unwired: 2 in, 2 out]
                n1468 = property on="SELECT LAB02-1" class="RadioBtnsControl (strict)"("DisabledEnum"=w2336) -> ()  [unwired: 2 in, 2 out]
                n1469 = property on="SELECT LAB03-1" class="RadioBtnsControl (strict)"("DisabledEnum"=w2334) -> ()  [unwired: 2 in, 2 out]
                n1470 = property on="SELECT LAB01-1" class="RadioBtnsControl (strict)"("DisabledEnum"=w2338) -> ()  [unwired: 2 in, 2 out]
                n1471 = property on="SELECT LAB01-2" class="RadioBtnsControl (strict)"("DisabledEnum"=w2337) -> ()  [unwired: 2 in, 2 out]
                n1472 = Not(x=w2347) -> (.not. x?=w2348:bool)
                n1473 = property on="RESULT LAB01-1" class="Bool (strict)"("Visible"=w2348) -> ()  [unwired: 2 in, 2 out]
                n1474 = Not(x=w2342) -> (.not. x?=w2346:bool)
                n1475 = Not(x=w2341) -> (.not. x?=w2345:bool)
                n1476 = Not(x=w2339) -> (.not. x?=w2344:bool)
                n1477 = property on="RESULT LAB01-2" class="Bool (strict)"("Visible"=w2346) -> ()  [unwired: 2 in, 2 out]
                n1478 = Not(x=w2340) -> (.not. x?=w2343:bool)
                n1479 = property on="RESULT LAB02-1" class="Bool (strict)"("Visible"=w2345) -> ()  [unwired: 2 in, 2 out]
                n1480 = property on="RESULT LAB02-2" class="Bool (strict)"("Visible"=w2344) -> ()  [unwired: 2 in, 2 out]
                n1481 = property on="RESULT LAB03-1" class="Bool (strict)"("Visible"=w2343) -> ()  [unwired: 2 in, 2 out]
                n1482 = property on="SET LAB01-1" class="Clust (strict)"("DisabledEnum"=w2338) -> ()  [unwired: 2 in, 2 out]
                n1483 = property on="SET LAB01-2" class="Clust (strict)"("DisabledEnum"=w2337) -> ()  [unwired: 2 in, 2 out]
                n1484 = property on="SET LAB02-1" class="Clust (strict)"("DisabledEnum"=w2336) -> ()  [unwired: 2 in, 2 out]
                n1485 = property on="SET LAB02-2" class="Clust (strict)"("DisabledEnum"=w2335) -> ()  [unwired: 2 in, 2 out]
                n1486 = property on="SET LAB03-1" class="Clust (strict)"("DisabledEnum"=w2334) -> ()  [unwired: 2 in, 2 out]
                n1487 = property on="O/I  LAB01-1" class="Bool (strict)"("DisabledEnum"=w2338) -> ()  [unwired: 2 in, 2 out]
                n1488 = property on="O/I  LAB01-2" class="Bool (strict)"("DisabledEnum"=w2337) -> ()  [unwired: 2 in, 2 out]
                n1489 = property on="O/I  LAB02-1" class="Bool (strict)"("DisabledEnum"=w2336) -> ()  [unwired: 2 in, 2 out]
                n1490 = property on="O/I  LAB02-2" class="Bool (strict)"("DisabledEnum"=w2335) -> ()  [unwired: 2 in, 2 out]
                n1491 = property on="O/I  LAB03-1" class="Bool (strict)"("DisabledEnum"=w2334) -> ()  [unwired: 2 in, 2 out]
              }
              frame #1 {
                n1492 = Select(t=2, s=w2368, f=0) -> (s? t:f=w2359:i32)
                n1493 = Select(t=2, s=w2367, f=0) -> (s? t:f=w2360:i32)
                n1494 = Select(t=2, s=w2364, f=0) -> (s? t:f=w2363:i32)
                n1495 = Select(t=2, s=w2365, f=0) -> (s? t:f=w2362:i32)
                n1496 = Select(t=2, s=w2366, f=0) -> (s? t:f=w2361:i32)
                n1497 = property on="SELECT LAB05-2" class="RadioBtnsControl (strict)"("DisabledEnum"=w2359) -> ()  [unwired: 2 in, 2 out]
                n1498 = property on="SELECT LAB05-1" class="RadioBtnsControl (strict)"("DisabledEnum"=w2360) -> ()  [unwired: 2 in, 2 out]
                n1499 = property on="SELECT LAB03-2" class="RadioBtnsControl (strict)"("DisabledEnum"=w2363) -> ()  [unwired: 2 in, 2 out]
                n1500 = property on="SELECT LAB04-1" class="RadioBtnsControl (strict)"("DisabledEnum"=w2362) -> ()  [unwired: 2 in, 2 out]
                n1501 = property on="SELECT LAB04-2" class="RadioBtnsControl (strict)"("DisabledEnum"=w2361) -> ()  [unwired: 2 in, 2 out]
                n1502 = property on="SET LAB05-2" class="Clust (strict)"("DisabledEnum"=w2359) -> ()  [unwired: 2 in, 2 out]
                n1503 = property on="SET LAB05-1" class="Clust (strict)"("DisabledEnum"=w2360) -> ()  [unwired: 2 in, 2 out]
                n1504 = property on="SET LAB03-2" class="Clust (strict)"("DisabledEnum"=w2363) -> ()  [unwired: 2 in, 2 out]
                n1505 = property on="SET LAB04-1" class="Clust (strict)"("DisabledEnum"=w2362) -> ()  [unwired: 2 in, 2 out]
                n1506 = property on="SET LAB04-2" class="Clust (strict)"("DisabledEnum"=w2361) -> ()  [unwired: 2 in, 2 out]
                n1507 = property on="O/I  LAB05-2" class="Bool (strict)"("DisabledEnum"=w2359) -> ()  [unwired: 2 in, 2 out]
                n1508 = property on="O/I  LAB05-1" class="Bool (strict)"("DisabledEnum"=w2360) -> ()  [unwired: 2 in, 2 out]
                n1509 = property on="O/I  LAB04-1" class="Bool (strict)"("DisabledEnum"=w2362) -> ()  [unwired: 2 in, 2 out]
                n1510 = property on="O/I  LAB04-2" class="Bool (strict)"("DisabledEnum"=w2361) -> ()  [unwired: 2 in, 2 out]
                n1511 = property on="O/I  LAB03-2" class="Bool (strict)"("DisabledEnum"=w2363) -> ()  [unwired: 2 in, 2 out]
                n1512 = Not(x=w2368) -> (.not. x?=w2369:bool)
                n1513 = Not(x=w2367) -> (.not. x?=w2370:bool)
                n1514 = Not(x=w2366) -> (.not. x?=w2371:bool)
                n1515 = property on="RESULT LAB05-2" class="Bool (strict)"("Visible"=w2369) -> ()  [unwired: 2 in, 2 out]
                n1516 = property on="RESULT LAB05-1" class="Bool (strict)"("Visible"=w2370) -> ()  [unwired: 2 in, 2 out]
                n1517 = Not(x=w2365) -> (.not. x?=w2372:bool)
                n1518 = property on="RESULT LAB04-2" class="Bool (strict)"("Visible"=w2371) -> ()  [unwired: 2 in, 2 out]
                n1519 = Not(x=w2364) -> (.not. x?=w2373:bool)
                n1520 = property on="RESULT LAB04-1" class="Bool (strict)"("Visible"=w2372) -> ()  [unwired: 2 in, 2 out]
                n1521 = property on="RESULT LAB03-2" class="Bool (strict)"("Visible"=w2373) -> ()  [unwired: 2 in, 2 out]
              }
              frame #2 {
                # "disable calibrate if any test running"
                n1522 = Or(x=w2395, y=w2394) -> (x .or. y?=w2388:bool)
                n1523 = Or(x=w2397, y=w2396) -> (x .or. y?=w2390:bool)
                n1524 = Or(x=w2401, y=w2400) -> (x .or. y?=w2392:bool)
                n1525 = Or(x=w2399, y=w2398) -> (x .or. y?=w2391:bool)
                n1526 = Or(x=w2403, y=w2402) -> (x .or. y?=w2393:bool)
                n1527 = Or(x=w2391, y=w2390) -> (x .or. y?=w2389:bool)
                n1528 = Or(x=w2393, y=w2392) -> (x .or. y?=w2387:bool)
                n1529 = Or(x=w2389, y=w2388) -> (x .or. y?=w2386:bool)
                n1530 = Or(x=w2387, y=w2386) -> (x .or. y?=w2385:bool)
                n1531 = case shown="True" w2385 {
                  tunnel: [0 2] -> w2384
                  frame False {
                  }
                  frame True {
                  }
                }
                n1532 = property on="JIG TEST" class="Clust (strict)"("DisabledEnum"=w2384) -> ()  [unwired: 2 in, 2 out]
                n1533 = property on="Network Directory" class="Path"("DisabledEnum"=w2384) -> ()  [unwired: 2 in, 2 out]
                n1534 = property on="MAIL SETTINGS" class="Clust (strict)"("DisabledEnum"=w2384) -> ()  [unwired: 2 in, 2 out]
                n1535 = property on="CALIBRATE" class="Bool (strict)"("DisabledEnum"=w2384) -> ()  [unwired: 2 in, 2 out]
                n1536 = property on="SHOW ADMIN PAGE" class="Bool (strict)"("DisabledEnum"=w2384) -> ()  [unwired: 2 in, 2 out]
              }
            }
          }
          frame #8 {
            # "drive jigs"
            n1537 = stacked-sequence {
              frame #0 {
                # "jig on"
                n1538 = local read "jig cycle"() -> (w2411:dbl)
                n1539 = property on="JIG TEST" class="Clust (strict)"() -> ("DisabledEnum"=w2408:T12)  [unwired: 2 in, 2 out]
                n1540 = Equal?(x=w2408, y=2) -> (x = y?=w2407:bool)
                n1541 = Equal?(x=w2411, y=0) -> (x = y?=w2409:bool)
                n1542 = And(x=w2409, y=w2407) -> (x .and. y?=w2406:bool)
                n1543 = case shown="True" w2406 {
                  frame False {
                  }
                  frame True {
                    n1544 = local read "run lab01-1"() -> (w2422:bool)
                    n1545 = local read "run lab01-2"() -> (w2421:bool)
                    n1546 = local read "run lab02-1"() -> (w2420:bool)
                    n1547 = local read "run lab02-2"() -> (w2419:bool)
                    n1548 = local read "run lab03-1"() -> (w2418:bool)
                    n1549 = local read "run lab03-2"() -> (w2417:bool)
                    n1550 = local read "run lab04-1"() -> (w2416:bool)
                    n1551 = local read "run lab04-2"() -> (w2415:bool)
                    n1552 = local read "run lab05-1"() -> (w2414:bool)
                    n1553 = local read "run lab05-2"() -> (w2413:bool)
                    n1554 = local write "JIG LAB03-2"(w2417) -> ()
                    n1555 = local write "JIG LAB01-1"(w2422) -> ()
                    n1556 = local write "JIG LAB01-2"(w2421) -> ()
                    n1557 = local write "JIG LAB02-1"(w2420) -> ()
                    n1558 = local write "JIG LAB02-2"(w2419) -> ()
                    n1559 = local write "JIG LAB03-1"(w2418) -> ()
                    n1560 = local write "JIG LAB04-1"(w2416) -> ()
                    n1561 = local write "JIG LAB04-2"(w2415) -> ()
                    n1562 = local write "JIG LAB05-1"(w2414) -> ()
                    n1563 = local write "JIG LAB05-2"(w2413) -> ()
                  }
                }
              }
              frame #1 {
                # "jig off"
                n1564 = local read "jig cycle"() -> (w2429:dbl)
                n1565 = local read "on loops"() -> (w2428:dbl)
                n1566 = property on="JIG TEST" class="Clust (strict)"() -> ("DisabledEnum"=w2427:T12)  [unwired: 2 in, 2 out]
                n1567 = Equal?(x=w2427, y=2) -> (x = y?=w2425:bool)
                n1568 = Equal?(x=w2429, y=w2428) -> (x = y?=w2424:bool)
                n1569 = And(x=w2424, y=w2425) -> (x .and. y?=w2423:bool)
                n1570 = case shown="True" w2423 {
                  frame False {
                  }
                  frame True {
                    w2480 = FALSE
                    w2481 = TRUE
                    w2479 = 2
                    n1571 = local read "SELECT LAB05-2"() -> (w2470:T3)
                    n1572 = local read "SELECT LAB04-2"() -> (w2472:T3)
                    n1573 = local read "SELECT LAB04-1"() -> (w2473:T3)
                    n1574 = local read "SELECT LAB05-1"() -> (w2471:T3)
                    n1575 = local read "SELECT LAB03-2"() -> (w2474:T3)
                    n1576 = local read "SELECT LAB02-1"() -> (w2477:T3)
                    n1577 = local read "SELECT LAB03-1"() -> (w2475:T3)
                    n1578 = local read "SELECT LAB02-2"() -> (w2476:T3)
                    n1579 = local read "SELECT LAB01-2"() -> (w2478:T3)
                    n1580 = local read "run lab05-1"() -> (w2440:bool)
                    n1581 = local read "run lab05-2"() -> (w2439:bool)
                    n1582 = local read "SELECT LAB01-1"() -> (w2482:T3)
                    n1583 = local read "run lab04-2"() -> (w2441:bool)
                    n1584 = local read "run lab04-1"() -> (w2442:bool)
                    n1585 = local read "run lab01-1"() -> (w2458:bool)
                    n1586 = local read "run lab01-2"() -> (w2447:bool)
                    n1587 = local read "run lab03-2"() -> (w2443:bool)
                    n1588 = local read "run lab03-1"() -> (w2444:bool)
                    n1589 = local read "run lab02-1"() -> (w2446:bool)
                    n1590 = local read "run lab02-2"() -> (w2445:bool)
                    n1591 = Equal?(x=w2479, y=w2475) -> (x = y?=w2453:bool)
                    n1592 = Equal?(x=w2479, y=w2474) -> (x = y?=w2452:bool)
                    n1593 = Equal?(x=w2479, y=w2473) -> (x = y?=w2451:bool)
                    n1594 = Equal?(x=w2479, y=w2472) -> (x = y?=w2450:bool)
                    n1595 = Equal?(x=w2479, y=w2471) -> (x = y?=w2449:bool)
                    n1596 = Equal?(x=w2479, y=w2470) -> (x = y?=w2448:bool)
                    n1597 = Equal?(x=w2479, y=w2482) -> (x = y?=w2459:bool)
                    n1598 = Equal?(x=w2479, y=w2477) -> (x = y?=w2455:bool)
                    n1599 = Equal?(x=w2479, y=w2476) -> (x = y?=w2454:bool)
                    n1600 = Equal?(x=w2479, y=w2478) -> (x = y?=w2456:bool)
                    n1601 = And(x=w2450, y=w2441) -> (x .and. y?=w2432:bool)
                    n1602 = And(x=w2453, y=w2444) -> (x .and. y?=w2435:bool)
                    n1603 = And(x=w2451, y=w2442) -> (x .and. y?=w2433:bool)
                    n1604 = And(x=w2448, y=w2439) -> (x .and. y?=w2430:bool)
                    n1605 = And(x=w2454, y=w2445) -> (x .and. y?=w2436:bool)
                    n1606 = And(x=w2452, y=w2443) -> (x .and. y?=w2434:bool)
                    n1607 = And(x=w2449, y=w2440) -> (x .and. y?=w2431:bool)
                    n1608 = And(x=w2456, y=w2447) -> (x .and. y?=w2438:bool)
                    n1609 = And(x=w2459, y=w2458) -> (x .and. y?=w2457:bool)
                    n1610 = And(x=w2455, y=w2446) -> (x .and. y?=w2437:bool)
                    n1611 = Select(t=w2481, s=w2457, f=w2480) -> (s? t:f=w2460:bool)
                    n1612 = Select(t=w2481, s=w2438, f=w2480) -> (s? t:f=w2461:bool)
                    n1613 = Select(t=w2481, s=w2437, f=w2480) -> (s? t:f=w2462:bool)
                    n1614 = Select(t=w2481, s=w2436, f=w2480) -> (s? t:f=w2463:bool)
                    n1615 = Select(t=w2481, s=w2435, f=w2480) -> (s? t:f=w2464:bool)
                    n1616 = Select(t=w2481, s=w2434, f=w2480) -> (s? t:f=w2465:bool)
                    n1617 = Select(t=w2481, s=w2433, f=w2480) -> (s? t:f=w2466:bool)
                    n1618 = Select(t=w2481, s=w2432, f=w2480) -> (s? t:f=w2467:bool)
                    n1619 = Select(t=w2481, s=w2431, f=w2480) -> (s? t:f=w2468:bool)
                    n1620 = Select(t=w2481, s=w2430, f=w2480) -> (s? t:f=w2469:bool)
                    n1621 = local write "JIG LAB03-2"(w2465) -> ()
                    n1622 = local write "JIG LAB02-1"(w2462) -> ()
                    n1623 = local write "JIG LAB02-2"(w2463) -> ()
                    n1624 = local write "JIG LAB01-2"(w2461) -> ()
                    n1625 = local write "JIG LAB03-1"(w2464) -> ()
                    n1626 = local write "JIG LAB01-1"(w2460) -> ()
                    n1627 = local write "JIG LAB05-2"(w2469) -> ()
                    n1628 = local write "JIG LAB04-1"(w2466) -> ()
                    n1629 = local write "JIG LAB05-1"(w2468) -> ()
                    n1630 = local write "JIG LAB04-2"(w2467) -> ()
                  }
                }
              }
            }
          }
          frame #9 {
            # "enable  jig test output if no test busy"
            n1631 = property on="JIG TEST" class="Clust (strict)"() -> ("DisabledEnum"=w2485:T12)  [unwired: 2 in, 2 out]
            n1632 = Equal?(x=w2485, y=0) -> (x = y?=w2483:bool)
            n1633 = case shown="True" w2483 {
              frame False {
              }
              frame True {
                n1634 = local read "JIG TEST"() -> (w2496:T9)
                n1635 = Unbundle(w2496) -> ("LAB01-1"=w2495:bool, "LAB01-2"=w2494:bool, "LAB02-1"=w2493:bool, "LAB02-2"=w2492:bool, "LAB03-1"=w2491:bool, "LAB03-2"=w2490:bool, "LAB04-1"=w2489:bool, "LAB04-2"=w2488:bool, "LAB05-1"=w2487:bool, "LAB05-2"=w2486:bool)
                n1636 = local write "JIG LAB05-1"(w2487) -> ()
                n1637 = local write "JIG LAB05-2"(w2486) -> ()
                n1638 = local write "JIG LAB04-1"(w2489) -> ()
                n1639 = local write "JIG LAB04-2"(w2488) -> ()
                n1640 = local write "JIG LAB03-2"(w2490) -> ()
                n1641 = local write "JIG LAB01-1"(w2495) -> ()
                n1642 = local write "JIG LAB02-1"(w2493) -> ()
                n1643 = local write "JIG LAB03-1"(w2491) -> ()
                n1644 = local write "JIG LAB01-2"(w2494) -> ()
                n1645 = local write "JIG LAB02-2"(w2492) -> ()
              }
            }
          }
          frame #10 {
            # "drive digital output"
            n1646 = local read "O/I  LAB05-2"() -> (w2502:bool)
            n1647 = local read "O/I  LAB05-1"() -> (w2504:bool)
            n1648 = local read "JIG LAB05-2"() -> (w2501:bool)
            n1649 = local read "O/I  LAB04-2"() -> (w2506:bool)
            n1650 = local read "JIG LAB05-1"() -> (w2503:bool)
            n1651 = local read "JIG LAB04-2"() -> (w2505:bool)
            n1652 = local read "O/I  LAB03-1"() -> (w2511:bool)
            n1653 = local read "O/I  LAB04-1"() -> (w2507:bool)
            n1654 = local read "O/I  LAB02-1"() -> (w2515:bool)
            n1655 = local read "O/I  LAB02-2"() -> (w2513:bool)
            n1656 = local read "O/I  LAB03-2"() -> (w2509:bool)
            n1657 = local read "JIG LAB04-1"() -> (w2500:bool)
            n1658 = local read "JIG LAB03-2"() -> (w2508:bool)
            n1659 = local read "O/I  LAB01-2"() -> (w2517:bool)
            n1660 = local read "JIG LAB02-1"() -> (w2514:bool)
            n1661 = local read "JIG LAB02-2"() -> (w2512:bool)
            n1662 = local read "JIG LAB03-1"() -> (w2510:bool)
            n1663 = local read "O/I  LAB01-1"() -> (w2519:bool)
            n1664 = local read "JIG LAB01-2"() -> (w2516:bool)
            n1665 = local read "JIG LAB01-1"() -> (w2518:bool)
            n1666 = Build Array(w2506, w2505, w2504, w2503, w2502, w2501) -> (w2497:bool[])
            n1667 = Build Array(w2512, w2511, w2510, w2509, w2508, w2507, w2500) -> (w2498:bool[])
            n1668 = Build Array(w2519, w2518, w2517, w2516, w2515, w2514, w2513) -> (w2499:bool[])
            n1669 = call "sub vi - Drive Relays All v6.vi"("Array #2"=w2497, "Array #1"=w2498, "Array #0"=w2499) -> ()  [unwired: 8 in, 1 out]
          }
          frame #11 {
            # "get temperature values"
            n1670 = stacked-sequence {
              frame #0 {
                n1671 = local read "jig cycle"() -> (w2520:dbl)
                n1672 = local read "on loops"() -> (w2523:dbl)
                n1673 = local read "jig cycle"() -> (w2525:dbl)
                n1674 = Add(x=w2523, y=2) -> (x+y=w2524:dbl)
                n1675 = Equal?(x=w2525, y=0) -> (x = y?=w2526:bool)
                n1676 = Equal?(x=w2520, y=w2524) -> (x = y?=w2521:bool)
                n1677 = case shown="True" w2526 {
                  frame False {
                  }
                  frame True {
                    w2538 = FALSE
                    w2539 = TRUE
                    n1678 = local write "TEMP update"(TRUE) -> ()
                    n1679 = call "sub vi - GET ALL TEMP v3.vi"("LA01-EN"=w2539, "LA02-EN"=w2539, "LA03-EN"=w2539, "LA04-EN"=w2538, "LA05-EN"=w2538, "Gen Cal Value"=1.0) -> ("LA01 TEMP"=w2537:T20, "LA02 TEMP"=w2535:T20, "LA03 TEMP"=w2534:T20)  [unwired: 4 in, 3 out]
                    n1680 = local write "LAB03 TEMP"(w2534) -> ()
                    n1681 = local write "LAB02 TEMP"(w2535) -> ()
                    n1682 = local write "LAB01 TEMP"(w2537) -> ()
                  }
                }
                n1683 = case shown="True" w2521 {
                  frame False {
                  }
                  frame True {
                    w2531 = TRUE
                    w2532 = FALSE
                    n1684 = local write "TEMP update"(TRUE) -> ()
                    n1685 = call "sub vi - GET ALL TEMP v3.vi"("LA01-EN"=w2532, "LA02-EN"=w2532, "LA03-EN"=w2532, "LA04-EN"=w2531, "LA05-EN"=w2531, "Gen Cal Value"=1.0) -> ("LA04 TEMP"=w2529:T20, "LA05 TEMP"=w2528:T20)  [unwired: 4 in, 4 out]
                    n1686 = local write "LAB04 TEMP"(w2529) -> ()
                    n1687 = local write "LAB05 TEMP"(w2528) -> ()
                  }
                }
              }
              frame #1 {
                n1688 = local read "CAL LAB01"() -> (w2557:T7)
                n1689 = local read "LAB01 TEMP"() -> (w2558:T11)
                n1690 = Unbundle By Name(w2558) -> ("T1 Live"=w2548:dbl, "T1 Neut"=w2547:dbl, "T2 Live"=w2546:dbl, "T2 Neut"=w2545:dbl)  [unwired: 2 out]
                n1691 = Unbundle By Name(w2557) -> ("1 (TL) cal"=w2544:dbl, "1 (TN) cal"=w2543:dbl, "2 (TL) cal"=w2542:dbl, "2 (TN) cal"=w2541:dbl)  [unwired: 6 out]
                n1692 = Multiply(x=w2548, y=w2544) -> (x*y=w2554:dbl)
                n1693 = Multiply(x=w2547, y=w2543) -> (x*y=w2553:dbl)
                n1694 = Multiply(x=w2546, y=w2542) -> (x*y=w2550:dbl)
                n1695 = Multiply(x=w2545, y=w2541) -> (x*y=w2549:dbl)
                n1696 = local read "SIG LAB01-2"() -> (w2552:T2)
                n1697 = local read "SIG LAB01-1"() -> (w2556:T2)
                n1698 = Bundle By Name(cluster=w2556, "Tmp Live"=w2554, "Tmp Neut"=w2553) -> (w2555:T2)
                n1699 = Bundle By Name(cluster=w2552, "Tmp Live"=w2550, "Tmp Neut"=w2549) -> (w2551:T2)
                n1700 = local write "SIG LAB01-1"(w2555) -> ()
                n1701 = local write "SIG LAB01-2"(w2551) -> ()
              }
              frame #2 {
                n1702 = local read "CAL LAB02"() -> (w2575:T8)
                n1703 = local read "LAB02 TEMP"() -> (w2576:T11)
                n1704 = Unbundle By Name(w2576) -> ("T1 Live"=w2566:dbl, "T1 Neut"=w2565:dbl, "T2 Live"=w2564:dbl, "T2 Neut"=w2563:dbl)  [unwired: 2 out]
                n1705 = Unbundle By Name(w2575) -> ("1 (TL) cal"=w2562:dbl, "1 (TN) cal"=w2561:dbl, "2 (TL) cal"=w2560:dbl, "2 (TN) cal"=w2559:dbl)  [unwired: 6 out]
                n1706 = Multiply(x=w2566, y=w2562) -> (x*y=w2572:dbl)
                n1707 = Multiply(x=w2565, y=w2561) -> (x*y=w2571:dbl)
                n1708 = Multiply(x=w2564, y=w2560) -> (x*y=w2568:dbl)
                n1709 = Multiply(x=w2563, y=w2559) -> (x*y=w2567:dbl)
                n1710 = local read "SIG LAB02-2"() -> (w2570:T2)
                n1711 = local read "SIG LAB02-1"() -> (w2574:T2)
                n1712 = Bundle By Name(cluster=w2574, "Tmp Live"=w2572, "Tmp Neut"=w2571) -> (w2573:T2)
                n1713 = Bundle By Name(cluster=w2570, "Tmp Live"=w2568, "Tmp Neut"=w2567) -> (w2569:T2)
                n1714 = local write "SIG LAB02-1"(w2573) -> ()
                n1715 = local write "SIG LAB02-2"(w2569) -> ()
              }
              frame #3 {
                n1716 = local read "CAL LAB03"() -> (w2593:T7)
                n1717 = local read "LAB03 TEMP"() -> (w2594:T11)
                n1718 = Unbundle By Name(w2594) -> ("T1 Live"=w2584:dbl, "T1 Neut"=w2583:dbl, "T2 Live"=w2582:dbl, "T2 Neut"=w2581:dbl)  [unwired: 2 out]
                n1719 = Unbundle By Name(w2593) -> ("1 (TL) cal"=w2580:dbl, "1 (TN) cal"=w2579:dbl, "2 (TL) cal"=w2578:dbl, "2 (TN) cal"=w2577:dbl)  [unwired: 6 out]
                n1720 = Multiply(x=w2584, y=w2580) -> (x*y=w2590:dbl)
                n1721 = Multiply(x=w2583, y=w2579) -> (x*y=w2589:dbl)
                n1722 = Multiply(x=w2582, y=w2578) -> (x*y=w2586:dbl)
                n1723 = Multiply(x=w2581, y=w2577) -> (x*y=w2585:dbl)
                n1724 = local read "SIG LAB03-2"() -> (w2588:T2)
                n1725 = local read "SIG LAB03-1"() -> (w2592:T2)
                n1726 = Bundle By Name(cluster=w2592, "Tmp Live"=w2590, "Tmp Neut"=w2589) -> (w2591:T2)
                n1727 = Bundle By Name(cluster=w2588, "Tmp Live"=w2586, "Tmp Neut"=w2585) -> (w2587:T2)
                n1728 = local write "SIG LAB03-1"(w2591) -> ()
                n1729 = local write "SIG LAB03-2"(w2587) -> ()
              }
              frame #4 {
                n1730 = local read "CAL LAB04"() -> (w2611:T7)
                n1731 = local read "LAB04 TEMP"() -> (w2612:T11)
                n1732 = Unbundle By Name(w2612) -> ("T1 Live"=w2602:dbl, "T1 Neut"=w2601:dbl, "T2 Live"=w2600:dbl, "T2 Neut"=w2599:dbl)  [unwired: 2 out]
                n1733 = Unbundle By Name(w2611) -> ("1 (TL) cal"=w2598:dbl, "1 (TN) cal"=w2597:dbl, "2 (TL) cal"=w2596:dbl, "2 (TN) cal"=w2595:dbl)  [unwired: 6 out]
                n1734 = Multiply(x=w2602, y=w2598) -> (x*y=w2608:dbl)
                n1735 = Multiply(x=w2601, y=w2597) -> (x*y=w2607:dbl)
                n1736 = Multiply(x=w2600, y=w2596) -> (x*y=w2604:dbl)
                n1737 = Multiply(x=w2599, y=w2595) -> (x*y=w2603:dbl)
                n1738 = local read "SIG LAB04-2"() -> (w2606:T2)
                n1739 = local read "SIG LAB04-1"() -> (w2610:T2)
                n1740 = Bundle By Name(cluster=w2610, "Tmp Live"=w2608, "Tmp Neut"=w2607) -> (w2609:T2)
                n1741 = Bundle By Name(cluster=w2606, "Tmp Live"=w2604, "Tmp Neut"=w2603) -> (w2605:T2)
                n1742 = local write "SIG LAB04-1"(w2609) -> ()
                n1743 = local write "SIG LAB04-2"(w2605) -> ()
              }
              frame #5 {
                n1744 = local read "CAL LAB05"() -> (w2629:T7)
                n1745 = local read "LAB05 TEMP"() -> (w2630:T11)
                n1746 = Unbundle By Name(w2630) -> ("T1 Live"=w2620:dbl, "T1 Neut"=w2619:dbl, "T2 Live"=w2618:dbl, "T2 Neut"=w2617:dbl)  [unwired: 2 out]
                n1747 = Unbundle By Name(w2629) -> ("1 (TL) cal"=w2616:dbl, "1 (TN) cal"=w2615:dbl, "2 (TL) cal"=w2614:dbl, "2 (TN) cal"=w2613:dbl)  [unwired: 6 out]
                n1748 = Multiply(x=w2620, y=w2616) -> (x*y=w2626:dbl)
                n1749 = Multiply(x=w2619, y=w2615) -> (x*y=w2625:dbl)
                n1750 = Multiply(x=w2618, y=w2614) -> (x*y=w2622:dbl)
                n1751 = Multiply(x=w2617, y=w2613) -> (x*y=w2621:dbl)
                n1752 = local read "SIG LAB05-2"() -> (w2624:T2)
                n1753 = local read "SIG LAB05-1"() -> (w2628:T2)
                n1754 = Bundle By Name(cluster=w2628, "Tmp Live"=w2626, "Tmp Neut"=w2625) -> (w2627:T2)
                n1755 = Bundle By Name(cluster=w2624, "Tmp Live"=w2622, "Tmp Neut"=w2621) -> (w2623:T2)
                n1756 = local write "SIG LAB05-1"(w2627) -> ()
                n1757 = local write "SIG LAB05-2"(w2623) -> ()
              }
            }
          }
          frame #12 {
            # "get analog values"
            n1758 = local read "on loops"() -> (w2637:dbl)
            n1759 = local read "jig cycle"() -> (w2634:dbl)
            n1760 = Add(x=w2637, y=1) -> (x+y=w2635:dbl)
            n1761 = Equal?(x=w2634, y=1) -> (x = y?=w2632:bool)
            n1762 = Equal?(x=w2634, y=w2635) -> (x = y?=w2633:bool)
            n1763 = Or(x=w2632, y=w2633) -> (x .or. y?=w2631:bool)
            n1764 = case shown="True" w2631 {
              frame False {
              }
              frame True {
                n1765 = call "sub vi - Read Analog All v8.vi"() -> ("Analog loop time"=w2645:dbl, "array GRAPH"=w2644:dynamicdata[], "LAB01"=w2643:T21, "LAB02"=w2642:T22, "LAB03"=w2641:T23, "LAB04"=w2640:T24, "array ERROR"=w2646:errorcluster[], "LAB05"=w2639:T25)  [unwired: 8 in]
                n1766 = stacked-sequence {
                  tunnel: w2646 -> [w2649 _ _ _ _ _]
                  tunnel: w2645 -> [w2648 _ _ _ _ _]
                  tunnel: w2644 -> [w2647 _ _ _ _ _]
                  tunnel: w2643 -> [_ w2694 _ _ _ _]
                  tunnel: w2642 -> [_ _ w2695 _ _ _]
                  tunnel: w2641 -> [_ _ _ w2720 _ _]
                  tunnel: w2640 -> [_ _ _ _ w2743 _]
                  tunnel: w2639 -> [_ _ _ _ _ w2768]
                  frame #0 {
                    n1767 = local write "AI update"(TRUE) -> ()
                    n1768 = Index Array(array=w2647, index=6) -> (element=→"LAB04-1 (GRAPH)":dynamicdata)
                    n1769 = Index Array(array=w2647, index=7) -> (element=→"LAB04-2 (GRAPH)":dynamicdata)
                    n1770 = Index Array(array=w2647, index=9) -> (element=→"LAB05-2 (GRAPH)":dynamicdata)
                    n1771 = Index Array(array=w2647, index=8) -> (element=→"LAB05-1 (GRAPH)":dynamicdata)
                    n1772 = Index Array(array=w2647, index=5) -> (element=→"LAB03-2 (GRAPH)":dynamicdata)
                    n1773 = Index Array(array=w2647, index=0) -> (element=→"LAB01-1 (GRAPH)":dynamicdata)
                    n1774 = Index Array(array=w2647, index=1) -> (element=→"LAB01-2 (GRAPH)":dynamicdata)
                    n1775 = Index Array(array=w2647, index=2) -> (element=→"LAB02-1 (GRAPH)":dynamicdata)
                    n1776 = Index Array(array=w2647, index=3) -> (element=→"LAB02-2 (GRAPH)":dynamicdata)
                    n1777 = Index Array(array=w2647, index=4) -> (element=→"LAB03-1 (GRAPH)":dynamicdata)
                    "AI loop time" <- w2648
                    "Analog Error Array" <- w2649
                  }
                  frame #1 {
                    n1778 = local read "CAL LAB01"() -> (w2693:T7)
                    n1779 = Unbundle By Name(w2694) -> ("LAB01-1 (A)"=w2692:dbl, "LAB01-1 (V)"=w2691:dbl, "LAB01-1 (PF)"=w2690:dbl, "LAB01-2 (A)"=w2689:dbl, "LAB01-2 (V)"=w2688:dbl, "LAB01-2 (PF)"=w2687:dbl)
                    n1780 = Unbundle By Name(w2693) -> ("1  (A) cal"=w2686:dbl, "1 (V) cal"=w2685:dbl, "1 (PF) cal"=w2684:dbl, "2 (A) cal"=w2683:dbl, "2 (V) cal"=w2682:dbl, "2 (PF) cal"=w2681:dbl)  [unwired: 4 out]
                    n1781 = Multiply(x=w2692, y=w2686) -> (x*y=w2679:dbl)
                    n1782 = Multiply(x=w2691, y=w2685) -> (x*y=w2678:dbl)
                    n1783 = Multiply(x=w2690, y=w2684) -> (x*y=w2677:dbl)
                    n1784 = Multiply(x=w2689, y=w2683) -> (x*y=w2673:dbl)
                    n1785 = Multiply(x=w2688, y=w2682) -> (x*y=w2672:dbl)
                    n1786 = Multiply(x=w2687, y=w2681) -> (x*y=w2671:dbl)
                    n1787 = local read "SIG LAB01-1"() -> (w2680:T2)
                    n1788 = local read "SIG LAB01-2"() -> (w2675:T2)
                    n1789 = Bundle By Name(cluster=w2680, "AMPS"=w2679, "VOLTS"=w2678, "PF"=w2677) -> (w2676:T2)
                    n1790 = Bundle By Name(cluster=w2675, "AMPS"=w2673, "VOLTS"=w2672, "PF"=w2671) -> (w2674:T2)
                    n1791 = local write "SIG LAB01-2"(w2674) -> ()
                    n1792 = local write "SIG LAB01-1"(w2676) -> ()
                  }
                  frame #2 {
                    n1793 = local read "CAL LAB02"() -> (w2718:T8)
                    n1794 = Unbundle By Name(w2695) -> ("LAB02-1 (A)"=w2717:dbl, "LAB02-1 (V)"=w2716:dbl, "LAB02-1 (PF)"=w2715:dbl, "LAB02-2 (A)"=w2714:dbl, "LAB02-2 (V)"=w2713:dbl, "LAB02-2 (PF)"=w2712:dbl)
                    n1795 = Unbundle By Name(w2718) -> ("1 (A) cal"=w2711:dbl, "1 (V) cal"=w2710:dbl, "1 (PF) cal"=w2709:dbl, "2 (A) cal"=w2708:dbl, "2 (V) cal"=w2707:dbl, "2 (PF) cal"=w2706:dbl)  [unwired: 4 out]
                    n1796 = Multiply(x=w2717, y=w2711) -> (x*y=w2704:dbl)
                    n1797 = Multiply(x=w2716, y=w2710) -> (x*y=w2703:dbl)
                    n1798 = Multiply(x=w2715, y=w2709) -> (x*y=w2702:dbl)
                    n1799 = Multiply(x=w2714, y=w2708) -> (x*y=w2698:dbl)
                    n1800 = Multiply(x=w2713, y=w2707) -> (x*y=w2697:dbl)
                    n1801 = Multiply(x=w2712, y=w2706) -> (x*y=w2696:dbl)
                    n1802 = local read "SIG LAB02-1"() -> (w2705:T2)
                    n1803 = local read "SIG LAB02-2"() -> (w2700:T2)
                    n1804 = Bundle By Name(cluster=w2705, "AMPS"=w2704, "VOLTS"=w2703, "PF"=w2702) -> (w2701:T2)
                    n1805 = Bundle By Name(cluster=w2700, "AMPS"=w2698, "VOLTS"=w2697, "PF"=w2696) -> (w2699:T2)
                    n1806 = local write "SIG LAB02-2"(w2699) -> ()
                    n1807 = local write "SIG LAB02-1"(w2701) -> ()
                  }
                  frame #3 {
                    n1808 = local read "CAL LAB03"() -> (w2742:T7)
                    n1809 = Unbundle By Name(w2720) -> ("LAB03-1 (A)"=w2741:dbl, "LAB03-1 (V)"=w2740:dbl, "LAB03-1 (PF)"=w2739:dbl, "LAB03-2 (A)"=w2738:dbl, "LAB03-2 (V)"=w2737:dbl, "LAB03-2 (PF)"=w2736:dbl)
                    n1810 = Unbundle By Name(w2742) -> ("1  (A) cal"=w2735:dbl, "1 (V) cal"=w2734:dbl, "1 (PF) cal"=w2733:dbl, "2 (A) cal"=w2732:dbl, "2 (V) cal"=w2731:dbl, "2 (PF) cal"=w2730:dbl)  [unwired: 4 out]
                    n1811 = Multiply(x=w2741, y=w2735) -> (x*y=w2728:dbl)
                    n1812 = Multiply(x=w2740, y=w2734) -> (x*y=w2719:dbl)
                    n1813 = Multiply(x=w2739, y=w2733) -> (x*y=w2727:dbl)
                    n1814 = Multiply(x=w2738, y=w2732) -> (x*y=w2723:dbl)
                    n1815 = Multiply(x=w2737, y=w2731) -> (x*y=w2722:dbl)
                    n1816 = Multiply(x=w2736, y=w2730) -> (x*y=w2721:dbl)
                    n1817 = local read "SIG LAB03-1"() -> (w2729:T2)
                    n1818 = local read "SIG LAB03-2"() -> (w2725:T2)
                    n1819 = Bundle By Name(cluster=w2729, "AMPS"=w2728, "VOLTS"=w2719, "PF"=w2727) -> (w2726:T2)
                    n1820 = Bundle By Name(cluster=w2725, "AMPS"=w2723, "VOLTS"=w2722, "PF"=w2721) -> (w2724:T2)
                    n1821 = local write "SIG LAB03-2"(w2724) -> ()
                    n1822 = local write "SIG LAB03-1"(w2726) -> ()
                  }
                  frame #4 {
                    n1823 = local read "CAL LAB04"() -> (w2766:T7)
                    n1824 = Unbundle By Name(w2743) -> ("LAB04-1 (A)"=w2765:dbl, "LAB04-1 (V)"=w2764:dbl, "LAB04-1 (PF)"=w2763:dbl, "LAB04-2 (A)"=w2762:dbl, "LAB04-2 (V)"=w2761:dbl, "LAB04-2 (PF)"=w2760:dbl)
                    n1825 = Unbundle By Name(w2766) -> ("1  (A) cal"=w2759:dbl, "1 (V) cal"=w2758:dbl, "1 (PF) cal"=w2757:dbl, "2 (A) cal"=w2756:dbl, "2 (V) cal"=w2755:dbl, "2 (PF) cal"=w2754:dbl)  [unwired: 4 out]
                    n1826 = Multiply(x=w2765, y=w2759) -> (x*y=w2752:dbl)
                    n1827 = Multiply(x=w2764, y=w2758) -> (x*y=w2751:dbl)
                    n1828 = Multiply(x=w2763, y=w2757) -> (x*y=w2750:dbl)
                    n1829 = Multiply(x=w2762, y=w2756) -> (x*y=w2746:dbl)
                    n1830 = Multiply(x=w2761, y=w2755) -> (x*y=w2745:dbl)
                    n1831 = Multiply(x=w2760, y=w2754) -> (x*y=w2744:dbl)
                    n1832 = local read "SIG LAB04-1"() -> (w2753:T2)
                    n1833 = local read "SIG LAB04-2"() -> (w2748:T2)
                    n1834 = Bundle By Name(cluster=w2753, "AMPS"=w2752, "VOLTS"=w2751, "PF"=w2750) -> (w2749:T2)
                    n1835 = Bundle By Name(cluster=w2748, "AMPS"=w2746, "VOLTS"=w2745, "PF"=w2744) -> (w2747:T2)
                    n1836 = local write "SIG LAB04-2"(w2747) -> ()
                    n1837 = local write "SIG LAB04-1"(w2749) -> ()
                  }
                  frame #5 {
                    n1838 = local read "CAL LAB05"() -> (w2790:T7)
                    n1839 = Unbundle By Name(w2768) -> ("LAB05-1 (A)"=w2789:dbl, "LAB05-1 (V)"=w2767:dbl, "LAB05-1 (PF)"=w2788:dbl, "LAB05-2 (A)"=w2787:dbl, "LAB05-2 (V)"=w2786:dbl, "LAB05-2 (PF)"=w2785:dbl)
                    n1840 = Unbundle By Name(w2790) -> ("1  (A) cal"=w2784:dbl, "1 (V) cal"=w2783:dbl, "1 (PF) cal"=w2782:dbl, "2 (A) cal"=w2781:dbl, "2 (V) cal"=w2780:dbl, "2 (PF) cal"=w2779:dbl)  [unwired: 4 out]
                    n1841 = Multiply(x=w2789, y=w2784) -> (x*y=w2777:dbl)
                    n1842 = Multiply(x=w2767, y=w2783) -> (x*y=w2776:dbl)
                    n1843 = Multiply(x=w2788, y=w2782) -> (x*y=w2775:dbl)
                    n1844 = Multiply(x=w2787, y=w2781) -> (x*y=w2771:dbl)
                    n1845 = Multiply(x=w2786, y=w2780) -> (x*y=w2770:dbl)
                    n1846 = Multiply(x=w2785, y=w2779) -> (x*y=w2769:dbl)
                    n1847 = local read "SIG LAB05-1"() -> (w2778:T2)
                    n1848 = local read "SIG LAB05-2"() -> (w2773:T2)
                    n1849 = Bundle By Name(cluster=w2778, "AMPS"=w2777, "VOLTS"=w2776, "PF"=w2775) -> (w2774:T2)
                    n1850 = Bundle By Name(cluster=w2773, "AMPS"=w2771, "VOLTS"=w2770, "PF"=w2769) -> (w2772:T2)
                    n1851 = local write "SIG LAB05-2"(w2772) -> ()
                    n1852 = local write "SIG LAB05-1"(w2774) -> ()
                  }
                }
              }
            }
          }
          frame #13 {
            # "save test data to file"
            n1853 = Get Date/Time In Seconds() -> (seconds since 1Jan1904=w2795:timestamp)
            n1854 = local read "on loops"() -> (w2810:dbl)
            n1855 = local read "jig cycle"() -> (w2807:dbl)
            n1856 = Format Date/Time String(time format string (%c)="%H:%M%:%S", seconds (now)=w2795) -> (date/time string=w2794:string)  [unwired: 1 in]
            n1857 = Add(x=w2810, y=2) -> (x+y=w2808:dbl)
            n1858 = Build Array(w2794) -> (w2793:string[])
            n1859 = Equal?(x=w2807, y=1) -> (x = y?=w2792:bool)
            n1860 = Equal?(x=w2807, y=w2808) -> (x = y?=w2791:bool)
            n1861 = stacked-sequence {
              tunnel: w2806 -> [w2815 _ _ _ _ _ _ _ _ _]
              tunnel: w2805 -> [_ w2904 _ _ _ _ _ _ _ _]
              tunnel: w2804 -> [_ _ w2996 _ _ _ _ _ _ _]
              tunnel: w2803 -> [_ _ _ w3088 _ _ _ _ _ _]
              tunnel: w2802 -> [_ _ _ _ w3180 _ _ _ _ _]
              tunnel: w2801 -> [_ _ _ _ _ w3272 _ _ _ _]
              tunnel: w2800 -> [_ _ _ _ _ _ w3364 _ _ _]
              tunnel: w2799 -> [_ _ _ _ _ _ _ w3456 _ _]
              tunnel: w2798 -> [_ _ _ _ _ _ _ _ w3548 _]
              tunnel: w2797 -> [_ _ _ _ _ _ _ _ _ w3640]
              tunnel: w2793 -> [w2814 w2907 w2999 w3091 w3183 w3275 w3367 w3459 w3551 w3643]
              tunnel: w2792 -> [w2813 w2906 w2998 w3090 w3182 w3274 w3366 w3458 w3550 w3642]
              tunnel: w2791 -> [w2812 w2905 w2997 w3089 w3181 w3273 w3365 w3457 w3549 w3641]
              frame #0 {
                n1862 = case shown="True" w2815 {
                  tunnel: w2814 -> [_ w2819]
                  tunnel: w2813 -> [_ w2818]
                  tunnel: w2812 -> [_ w2816]
                  frame False {
                  }
                  frame True {
                    n1863 = local read "DISP LAB01-1"() -> (w2820:T4)
                    n1864 = local read "SIG LAB01-1"() -> (w2821:T2)
                    n1865 = local read "ON L01-1"() -> (w2817:cluster{"amps":dbl, "volts":dbl, "pf":dbl})
                    n1866 = Unbundle(w2821) -> ("AMPS"=w2827:dbl, "VOLTS"=w2825:dbl, "PF"=w2824:dbl, "Tmp Live"=w2823:dbl, "Tmp Neut"=w2826:dbl)
                    n1867 = Unbundle(w2820) -> ("CYCLE"=w2822:dbl)  [unwired: 2 out]
                    n1868 = stacked-sequence {
                      tunnel: w2827 -> [w2831 w2849]
                      tunnel: w2826 -> [_ w2848]
                      tunnel: w2825 -> [w2830 w2847]
                      tunnel: w2824 -> [w2829 w2846]
                      tunnel: w2823 -> [_ w2845]
                      tunnel: w2822 -> [_ w2844]
                      tunnel: w2819 -> [_ w2843]
                      tunnel: w2818 -> [w2832 _]
                      tunnel: w2817 -> [w2828 w2841]
                      tunnel: w2816 -> [_ w2842]
                      frame #0 {
                        n1869 = case shown="True" w2832 {
                          tunnel: w2831 -> [_ w2837]
                          tunnel: w2830 -> [_ w2836]
                          tunnel: w2829 -> [_ w2835]
                          tunnel: w2828 -> [_ w2833]
                          frame False {
                          }
                          frame True {
                            n1870 = Bundle(cluster=w2833, "amps"=w2837, "volts"=w2836, "pf"=w2835) -> (w2834:cluster{"amps":dbl, "volts":dbl, "pf":dbl})
                            n1871 = local write "ON L01-1"(w2834) -> ()
                          }
                        }
                      }
                      frame #1 {
                        n1872 = Unbundle(w2841) -> ("amps"=w2840:dbl, "volts"=w2839:dbl, "pf"=w2838:dbl)
                        n1873 = case shown="True" w2842 {
                          tunnel: w2849 -> [_ w2854]
                          tunnel: w2848 -> [_ w2903]
                          tunnel: w2847 -> [_ _]
                          tunnel: w2846 -> [_ _]
                          tunnel: w2845 -> [_ w2902]
                          tunnel: w2844 -> [_ w2901]
                          tunnel: w2843 -> [_ w2897]
                          tunnel: w2840 -> [_ w2856]
                          tunnel: w2839 -> [_ w2855]
                          tunnel: w2838 -> [_ w2853]
                          frame False {
                          }
                          frame True {
                            n1874 = local read "TDMS LAB01-1"() -> (w2894:refnum<k34>)
                            n1875 = Build Array(w2855) -> (w2883:dbl[])
                            n1876 = Build Array(w2853) -> (w2878:dbl[])
                            n1877 = Build Array(w2902) -> (w2873:dbl[])
                            n1878 = Build Array(w2903) -> (w2868:dbl[])
                            n1879 = Build Array(w2856) -> (w2890:dbl[])
                            n1880 = Build Array(w2854) -> (w2852:dbl[])
                            n1881 = Build Array(w2901) -> (w2863:dbl[])
                            n1882 = Build Array("TEMP Neut") -> (w2869:string[])
                            n1883 = Build Array("CYCLE") -> (w2864:string[])
                            n1884 = Build Array("TEMP Live") -> (w2874:string[])
                            n1885 = Build Array("PF") -> (w2879:string[])
                            n1886 = Build Array("AMPS OFF") -> (w2857:string[])
                            n1887 = Build Array("AMPS ON") -> (w2891:string[])
                            n1888 = Build Array("VOLTS") -> (w2885:string[])
                            n1889 = TDMS Write(0:w2894, 5:"LAB01-1 TEST VALUES", 7:w2891, 9:w2890) -> (4:w2862:refnum<k34>, 6:w2861:string, 15:w2851:errorcluster)  [unwired: 2 in, 1 out]
                            n1890 = TDMS Write(0:w2862, 5:w2861, 7:w2857, 9:w2852, 11:w2851) -> (4:w2860:refnum<k34>, 6:w2859:string, 15:w2850:errorcluster)  [unwired: 1 in, 1 out]
                            n1891 = TDMS Write(0:w2860, 5:w2859, 7:w2885, 9:w2883, 11:w2850) -> (4:w2882:refnum<k34>, 6:w2881:string, 15:w2880:errorcluster)  [unwired: 1 in, 1 out]
                            n1892 = TDMS Write(0:w2882, 5:w2881, 7:w2879, 9:w2878, 11:w2880) -> (4:w2877:refnum<k34>, 6:w2876:string, 15:w2875:errorcluster)  [unwired: 1 in, 1 out]
                            n1893 = TDMS Write(0:w2877, 5:w2876, 7:w2874, 9:w2873, 11:w2875) -> (4:w2872:refnum<k34>, 6:w2871:string, 15:w2870:errorcluster)  [unwired: 1 in, 1 out]
                            n1894 = TDMS Write(0:w2872, 5:w2871, 7:w2869, 9:w2868, 11:w2870) -> (4:w2867:refnum<k34>, 6:w2866:string, 15:w2865:errorcluster)  [unwired: 1 in, 1 out]
                            n1895 = TDMS Write(0:w2867, 5:w2866, 7:w2864, 9:w2863, 11:w2865) -> (4:w2895:refnum<k34>, 6:w2899:string, 15:w2900:errorcluster)  [unwired: 1 in, 1 out]
                            n1896 = TDMS Write(0:w2895, 5:w2899, 7:"TIME", 9:w2897, 11:w2900) -> (15:w2896:errorcluster)  [unwired: 1 in, 3 out]
                            n1897 = local write "data file error"(w2896) -> ()
                          }
                        }
                      }
                    }
                  }
                }
              }
              frame #1 {
                n1898 = case shown="True" w2904 {
                  tunnel: w2907 -> [_ w2911]
                  tunnel: w2906 -> [_ w2910]
                  tunnel: w2905 -> [_ w2908]
                  frame False {
                  }
                  frame True {
                    n1899 = local read "DISP LAB01-2"() -> (w2912:T4)
                    n1900 = local read "SIG LAB01-2"() -> (w2913:T2)
                    n1901 = local read "ON L01-2"() -> (w2909:cluster{"amps":dbl, "volts":dbl, "pf":dbl})
                    n1902 = Unbundle(w2913) -> ("AMPS"=w2919:dbl, "VOLTS"=w2917:dbl, "PF"=w2916:dbl, "Tmp Live"=w2915:dbl, "Tmp Neut"=w2918:dbl)
                    n1903 = Unbundle(w2912) -> ("CYCLE"=w2914:dbl)  [unwired: 2 out]
                    n1904 = stacked-sequence {
                      tunnel: w2919 -> [w2923 w2941]
                      tunnel: w2918 -> [_ w2940]
                      tunnel: w2917 -> [w2922 w2939]
                      tunnel: w2916 -> [w2921 w2938]
                      tunnel: w2915 -> [_ w2937]
                      tunnel: w2914 -> [_ w2936]
                      tunnel: w2911 -> [_ w2935]
                      tunnel: w2910 -> [w2924 _]
                      tunnel: w2909 -> [w2920 w2933]
                      tunnel: w2908 -> [_ w2934]
                      frame #0 {
                        n1905 = case shown="True" w2924 {
                          tunnel: w2923 -> [_ w2929]
                          tunnel: w2922 -> [_ w2928]
                          tunnel: w2921 -> [_ w2927]
                          tunnel: w2920 -> [_ w2925]
                          frame False {
                          }
                          frame True {
                            n1906 = Bundle(cluster=w2925, "amps"=w2929, "volts"=w2928, "pf"=w2927) -> (w2926:cluster{"amps":dbl, "volts":dbl, "pf":dbl})
                            n1907 = local write "ON L01-2"(w2926) -> ()
                          }
                        }
                      }
                      frame #1 {
                        n1908 = Unbundle(w2933) -> ("amps"=w2932:dbl, "volts"=w2931:dbl, "pf"=w2930:dbl)
                        n1909 = case shown="True" w2934 {
                          tunnel: w2941 -> [_ w2946]
                          tunnel: w2940 -> [_ w2995]
                          tunnel: w2939 -> [_ _]
                          tunnel: w2938 -> [_ _]
                          tunnel: w2937 -> [_ w2994]
                          tunnel: w2936 -> [_ w2993]
                          tunnel: w2935 -> [_ w2989]
                          tunnel: w2932 -> [_ w2948]
                          tunnel: w2931 -> [_ w2947]
                          tunnel: w2930 -> [_ w2945]
                          frame False {
                          }
                          frame True {
                            n1910 = local read "TDMS LAB01-2"() -> (w2986:refnum<k34>)
                            n1911 = Build Array(w2947) -> (w2975:dbl[])
                            n1912 = Build Array(w2945) -> (w2970:dbl[])
                            n1913 = Build Array(w2994) -> (w2965:dbl[])
                            n1914 = Build Array(w2995) -> (w2960:dbl[])
                            n1915 = Build Array(w2948) -> (w2982:dbl[])
                            n1916 = Build Array(w2946) -> (w2944:dbl[])
                            n1917 = Build Array(w2993) -> (w2955:dbl[])
                            n1918 = Build Array("TEMP Neut") -> (w2961:string[])
                            n1919 = Build Array("CYCLE") -> (w2956:string[])
                            n1920 = Build Array("TEMP Live") -> (w2966:string[])
                            n1921 = Build Array("PF") -> (w2971:string[])
                            n1922 = Build Array("AMPS OFF") -> (w2949:string[])
                            n1923 = Build Array("AMPS ON") -> (w2983:string[])
                            n1924 = Build Array("VOLTS") -> (w2977:string[])
                            n1925 = TDMS Write(0:w2986, 5:"LAB01-2 TEST VALUES", 7:w2983, 9:w2982) -> (4:w2954:refnum<k34>, 6:w2953:string, 15:w2943:errorcluster)  [unwired: 2 in, 1 out]
                            n1926 = TDMS Write(0:w2954, 5:w2953, 7:w2949, 9:w2944, 11:w2943) -> (4:w2952:refnum<k34>, 6:w2951:string, 15:w2942:errorcluster)  [unwired: 1 in, 1 out]
                            n1927 = TDMS Write(0:w2952, 5:w2951, 7:w2977, 9:w2975, 11:w2942) -> (4:w2974:refnum<k34>, 6:w2973:string, 15:w2972:errorcluster)  [unwired: 1 in, 1 out]
                            n1928 = TDMS Write(0:w2974, 5:w2973, 7:w2971, 9:w2970, 11:w2972) -> (4:w2969:refnum<k34>, 6:w2968:string, 15:w2967:errorcluster)  [unwired: 1 in, 1 out]
                            n1929 = TDMS Write(0:w2969, 5:w2968, 7:w2966, 9:w2965, 11:w2967) -> (4:w2964:refnum<k34>, 6:w2963:string, 15:w2962:errorcluster)  [unwired: 1 in, 1 out]
                            n1930 = TDMS Write(0:w2964, 5:w2963, 7:w2961, 9:w2960, 11:w2962) -> (4:w2959:refnum<k34>, 6:w2958:string, 15:w2957:errorcluster)  [unwired: 1 in, 1 out]
                            n1931 = TDMS Write(0:w2959, 5:w2958, 7:w2956, 9:w2955, 11:w2957) -> (4:w2987:refnum<k34>, 6:w2991:string, 15:w2992:errorcluster)  [unwired: 1 in, 1 out]
                            n1932 = TDMS Write(0:w2987, 5:w2991, 7:"TIME", 9:w2989, 11:w2992) -> (15:w2988:errorcluster)  [unwired: 1 in, 3 out]
                            n1933 = local write "data file error"(w2988) -> ()
                          }
                        }
                      }
                    }
                  }
                }
              }
              frame #2 {
                n1934 = case shown="True" w2996 {
                  tunnel: w2999 -> [_ w3003]
                  tunnel: w2998 -> [_ w3002]
                  tunnel: w2997 -> [_ w3000]
                  frame False {
                  }
                  frame True {
                    n1935 = local read "DISP LAB02-1"() -> (w3004:T4)
                    n1936 = local read "SIG LAB02-1"() -> (w3005:T2)
                    n1937 = local read "ON L02-1"() -> (w3001:cluster{"amps":dbl, "volts":dbl, "pf":dbl})
                    n1938 = Unbundle(w3005) -> ("AMPS"=w3011:dbl, "VOLTS"=w3009:dbl, "PF"=w3008:dbl, "Tmp Live"=w3007:dbl, "Tmp Neut"=w3010:dbl)
                    n1939 = Unbundle(w3004) -> ("CYCLE"=w3006:dbl)  [unwired: 2 out]
                    n1940 = stacked-sequence {
                      tunnel: w3011 -> [w3015 w3033]
                      tunnel: w3010 -> [_ w3032]
                      tunnel: w3009 -> [w3014 w3031]
                      tunnel: w3008 -> [w3013 w3030]
                      tunnel: w3007 -> [_ w3029]
                      tunnel: w3006 -> [_ w3028]
                      tunnel: w3003 -> [_ w3027]
                      tunnel: w3002 -> [w3016 _]
                      tunnel: w3001 -> [w3012 w3025]
                      tunnel: w3000 -> [_ w3026]
                      frame #0 {
                        n1941 = case shown="True" w3016 {
                          tunnel: w3015 -> [_ w3021]
                          tunnel: w3014 -> [_ w3020]
                          tunnel: w3013 -> [_ w3019]
                          tunnel: w3012 -> [_ w3017]
                          frame False {
                          }
                          frame True {
                            n1942 = Bundle(cluster=w3017, "amps"=w3021, "volts"=w3020, "pf"=w3019) -> (w3018:cluster{"amps":dbl, "volts":dbl, "pf":dbl})
                            n1943 = local write "ON L02-1"(w3018) -> ()
                          }
                        }
                      }
                      frame #1 {
                        n1944 = Unbundle(w3025) -> ("amps"=w3024:dbl, "volts"=w3023:dbl, "pf"=w3022:dbl)
                        n1945 = case shown="True" w3026 {
                          tunnel: w3033 -> [_ w3038]
                          tunnel: w3032 -> [_ w3087]
                          tunnel: w3031 -> [_ _]
                          tunnel: w3030 -> [_ _]
                          tunnel: w3029 -> [_ w3086]
                          tunnel: w3028 -> [_ w3085]
                          tunnel: w3027 -> [_ w3081]
                          tunnel: w3024 -> [_ w3040]
                          tunnel: w3023 -> [_ w3039]
                          tunnel: w3022 -> [_ w3037]
                          frame False {
                          }
                          frame True {
                            n1946 = local read "TDMS LAB02-1"() -> (w3078:refnum<k34>)
                            n1947 = Build Array(w3039) -> (w3067:dbl[])
                            n1948 = Build Array(w3037) -> (w3062:dbl[])
                            n1949 = Build Array(w3086) -> (w3057:dbl[])
                            n1950 = Build Array(w3087) -> (w3052:dbl[])
                            n1951 = Build Array(w3040) -> (w3074:dbl[])
                            n1952 = Build Array(w3038) -> (w3036:dbl[])
                            n1953 = Build Array(w3085) -> (w3047:dbl[])
                            n1954 = Build Array("TEMP Neut") -> (w3053:string[])
                            n1955 = Build Array("CYCLE") -> (w3048:string[])
                            n1956 = Build Array("TEMP Live") -> (w3058:string[])
                            n1957 = Build Array("PF") -> (w3063:string[])
                            n1958 = Build Array("AMPS OFF") -> (w3041:string[])
                            n1959 = Build Array("AMPS ON") -> (w3075:string[])
                            n1960 = Build Array("VOLTS") -> (w3069:string[])
                            n1961 = TDMS Write(0:w3078, 5:"LAB02-1 TEST VALUES", 7:w3075, 9:w3074) -> (4:w3046:refnum<k34>, 6:w3045:string, 15:w3035:errorcluster)  [unwired: 2 in, 1 out]
                            n1962 = TDMS Write(0:w3046, 5:w3045, 7:w3041, 9:w3036, 11:w3035) -> (4:w3044:refnum<k34>, 6:w3043:string, 15:w3034:errorcluster)  [unwired: 1 in, 1 out]
                            n1963 = TDMS Write(0:w3044, 5:w3043, 7:w3069, 9:w3067, 11:w3034) -> (4:w3066:refnum<k34>, 6:w3065:string, 15:w3064:errorcluster)  [unwired: 1 in, 1 out]
                            n1964 = TDMS Write(0:w3066, 5:w3065, 7:w3063, 9:w3062, 11:w3064) -> (4:w3061:refnum<k34>, 6:w3060:string, 15:w3059:errorcluster)  [unwired: 1 in, 1 out]
                            n1965 = TDMS Write(0:w3061, 5:w3060, 7:w3058, 9:w3057, 11:w3059) -> (4:w3056:refnum<k34>, 6:w3055:string, 15:w3054:errorcluster)  [unwired: 1 in, 1 out]
                            n1966 = TDMS Write(0:w3056, 5:w3055, 7:w3053, 9:w3052, 11:w3054) -> (4:w3051:refnum<k34>, 6:w3050:string, 15:w3049:errorcluster)  [unwired: 1 in, 1 out]
                            n1967 = TDMS Write(0:w3051, 5:w3050, 7:w3048, 9:w3047, 11:w3049) -> (4:w3079:refnum<k34>, 6:w3083:string, 15:w3084:errorcluster)  [unwired: 1 in, 1 out]
                            n1968 = TDMS Write(0:w3079, 5:w3083, 7:"TIME", 9:w3081, 11:w3084) -> (15:w3080:errorcluster)  [unwired: 1 in, 3 out]
                            n1969 = local write "data file error"(w3080) -> ()
                          }
                        }
                      }
                    }
                  }
                }
              }
              frame #3 {
                n1970 = case shown="True" w3088 {
                  tunnel: w3091 -> [_ w3095]
                  tunnel: w3090 -> [_ w3094]
                  tunnel: w3089 -> [_ w3092]
                  frame False {
                  }
                  frame True {
                    n1971 = local read "DISP LAB02-2"() -> (w3096:T4)
                    n1972 = local read "SIG LAB02-2"() -> (w3097:T2)
                    n1973 = local read "ON L02-2"() -> (w3093:cluster{"amps":dbl, "volts":dbl, "pf":dbl})
                    n1974 = Unbundle(w3097) -> ("AMPS"=w3103:dbl, "VOLTS"=w3101:dbl, "PF"=w3100:dbl, "Tmp Live"=w3099:dbl, "Tmp Neut"=w3102:dbl)
                    n1975 = Unbundle(w3096) -> ("CYCLE"=w3098:dbl)  [unwired: 2 out]
                    n1976 = stacked-sequence {
                      tunnel: w3103 -> [w3107 w3125]
                      tunnel: w3102 -> [_ w3124]
                      tunnel: w3101 -> [w3106 w3123]
                      tunnel: w3100 -> [w3105 w3122]
                      tunnel: w3099 -> [_ w3121]
                      tunnel: w3098 -> [_ w3120]
                      tunnel: w3095 -> [_ w3119]
                      tunnel: w3094 -> [w3108 _]
                      tunnel: w3093 -> [w3104 w3117]
                      tunnel: w3092 -> [_ w3118]
                      frame #0 {
                        n1977 = case shown="True" w3108 {
                          tunnel: w3107 -> [_ w3113]
                          tunnel: w3106 -> [_ w3112]
                          tunnel: w3105 -> [_ w3111]
                          tunnel: w3104 -> [_ w3109]
                          frame False {
                          }
                          frame True {
                            n1978 = Bundle(cluster=w3109, "amps"=w3113, "volts"=w3112, "pf"=w3111) -> (w3110:cluster{"amps":dbl, "volts":dbl, "pf":dbl})
                            n1979 = local write "ON L02-2"(w3110) -> ()
                          }
                        }
                      }
                      frame #1 {
                        n1980 = Unbundle(w3117) -> ("amps"=w3116:dbl, "volts"=w3115:dbl, "pf"=w3114:dbl)
                        n1981 = case shown="True" w3118 {
                          tunnel: w3125 -> [_ w3130]
                          tunnel: w3124 -> [_ w3179]
                          tunnel: w3123 -> [_ _]
                          tunnel: w3122 -> [_ _]
                          tunnel: w3121 -> [_ w3178]
                          tunnel: w3120 -> [_ w3177]
                          tunnel: w3119 -> [_ w3173]
                          tunnel: w3116 -> [_ w3132]
                          tunnel: w3115 -> [_ w3131]
                          tunnel: w3114 -> [_ w3129]
                          frame False {
                          }
                          frame True {
                            n1982 = local read "TDMS LAB02-2"() -> (w3170:refnum<k34>)
                            n1983 = Build Array(w3131) -> (w3159:dbl[])
                            n1984 = Build Array(w3129) -> (w3154:dbl[])
                            n1985 = Build Array(w3178) -> (w3149:dbl[])
                            n1986 = Build Array(w3179) -> (w3144:dbl[])
                            n1987 = Build Array(w3132) -> (w3166:dbl[])
                            n1988 = Build Array(w3130) -> (w3128:dbl[])
                            n1989 = Build Array(w3177) -> (w3139:dbl[])
                            n1990 = Build Array("TEMP Neut") -> (w3145:string[])
                            n1991 = Build Array("CYCLE") -> (w3140:string[])
                            n1992 = Build Array("TEMP Live") -> (w3150:string[])
                            n1993 = Build Array("PF") -> (w3155:string[])
                            n1994 = Build Array("AMPS OFF") -> (w3133:string[])
                            n1995 = Build Array("AMPS ON") -> (w3167:string[])
                            n1996 = Build Array("VOLTS") -> (w3161:string[])
                            n1997 = TDMS Write(0:w3170, 5:"LAB02-2 TEST VALUES", 7:w3167, 9:w3166) -> (4:w3138:refnum<k34>, 6:w3137:string, 15:w3127:errorcluster)  [unwired: 2 in, 1 out]
                            n1998 = TDMS Write(0:w3138, 5:w3137, 7:w3133, 9:w3128, 11:w3127) -> (4:w3136:refnum<k34>, 6:w3135:string, 15:w3126:errorcluster)  [unwired: 1 in, 1 out]
                            n1999 = TDMS Write(0:w3136, 5:w3135, 7:w3161, 9:w3159, 11:w3126) -> (4:w3158:refnum<k34>, 6:w3157:string, 15:w3156:errorcluster)  [unwired: 1 in, 1 out]
                            n2000 = TDMS Write(0:w3158, 5:w3157, 7:w3155, 9:w3154, 11:w3156) -> (4:w3153:refnum<k34>, 6:w3152:string, 15:w3151:errorcluster)  [unwired: 1 in, 1 out]
                            n2001 = TDMS Write(0:w3153, 5:w3152, 7:w3150, 9:w3149, 11:w3151) -> (4:w3148:refnum<k34>, 6:w3147:string, 15:w3146:errorcluster)  [unwired: 1 in, 1 out]
                            n2002 = TDMS Write(0:w3148, 5:w3147, 7:w3145, 9:w3144, 11:w3146) -> (4:w3143:refnum<k34>, 6:w3142:string, 15:w3141:errorcluster)  [unwired: 1 in, 1 out]
                            n2003 = TDMS Write(0:w3143, 5:w3142, 7:w3140, 9:w3139, 11:w3141) -> (4:w3171:refnum<k34>, 6:w3175:string, 15:w3176:errorcluster)  [unwired: 1 in, 1 out]
                            n2004 = TDMS Write(0:w3171, 5:w3175, 7:"TIME", 9:w3173, 11:w3176) -> (15:w3172:errorcluster)  [unwired: 1 in, 3 out]
                            n2005 = local write "data file error"(w3172) -> ()
                          }
                        }
                      }
                    }
                  }
                }
              }
              frame #4 {
                n2006 = case shown="True" w3180 {
                  tunnel: w3183 -> [_ w3187]
                  tunnel: w3182 -> [_ w3186]
                  tunnel: w3181 -> [_ w3184]
                  frame False {
                  }
                  frame True {
                    n2007 = local read "DISP LAB03-1"() -> (w3188:T4)
                    n2008 = local read "SIG LAB03-1"() -> (w3189:T2)
                    n2009 = local read "ON L03-1"() -> (w3185:cluster{"amps":dbl, "volts":dbl, "pf":dbl})
                    n2010 = Unbundle(w3189) -> ("AMPS"=w3195:dbl, "VOLTS"=w3193:dbl, "PF"=w3192:dbl, "Tmp Live"=w3191:dbl, "Tmp Neut"=w3194:dbl)
                    n2011 = Unbundle(w3188) -> ("CYCLE"=w3190:dbl)  [unwired: 2 out]
                    n2012 = stacked-sequence {
                      tunnel: w3195 -> [w3199 w3217]
                      tunnel: w3194 -> [_ w3216]
                      tunnel: w3193 -> [w3198 w3215]
                      tunnel: w3192 -> [w3197 w3214]
                      tunnel: w3191 -> [_ w3213]
                      tunnel: w3190 -> [_ w3212]
                      tunnel: w3187 -> [_ w3211]
                      tunnel: w3186 -> [w3200 _]
                      tunnel: w3185 -> [w3196 w3209]
                      tunnel: w3184 -> [_ w3210]
                      frame #0 {
                        n2013 = case shown="True" w3200 {
                          tunnel: w3199 -> [_ w3205]
                          tunnel: w3198 -> [_ w3204]
                          tunnel: w3197 -> [_ w3203]
                          tunnel: w3196 -> [_ w3201]
                          frame False {
                          }
                          frame True {
                            n2014 = Bundle(cluster=w3201, "amps"=w3205, "volts"=w3204, "pf"=w3203) -> (w3202:cluster{"amps":dbl, "volts":dbl, "pf":dbl})
                            n2015 = local write "ON L03-1"(w3202) -> ()
                          }
                        }
                      }
                      frame #1 {
                        n2016 = Unbundle(w3209) -> ("amps"=w3208:dbl, "volts"=w3207:dbl, "pf"=w3206:dbl)
                        n2017 = case shown="True" w3210 {
                          tunnel: w3217 -> [_ w3222]
                          tunnel: w3216 -> [_ w3271]
                          tunnel: w3215 -> [_ _]
                          tunnel: w3214 -> [_ _]
                          tunnel: w3213 -> [_ w3270]
                          tunnel: w3212 -> [_ w3269]
                          tunnel: w3211 -> [_ w3265]
                          tunnel: w3208 -> [_ w3224]
                          tunnel: w3207 -> [_ w3223]
                          tunnel: w3206 -> [_ w3221]
                          frame False {
                          }
                          frame True {
                            n2018 = local read "TDMS LAB03-1"() -> (w3262:refnum<k34>)
                            n2019 = Build Array(w3223) -> (w3251:dbl[])
                            n2020 = Build Array(w3221) -> (w3246:dbl[])
                            n2021 = Build Array(w3270) -> (w3241:dbl[])
                            n2022 = Build Array(w3271) -> (w3236:dbl[])
                            n2023 = Build Array(w3224) -> (w3258:dbl[])
                            n2024 = Build Array(w3222) -> (w3220:dbl[])
                            n2025 = Build Array(w3269) -> (w3231:dbl[])
                            n2026 = Build Array("TEMP Neut") -> (w3237:string[])
                            n2027 = Build Array("CYCLE") -> (w3232:string[])
                            n2028 = Build Array("TEMP Live") -> (w3242:string[])
                            n2029 = Build Array("PF") -> (w3247:string[])
                            n2030 = Build Array("AMPS OFF") -> (w3225:string[])
                            n2031 = Build Array("AMPS ON") -> (w3259:string[])
                            n2032 = Build Array("VOLTS") -> (w3253:string[])
                            n2033 = TDMS Write(0:w3262, 5:"LAB03-1 TEST VALUES", 7:w3259, 9:w3258) -> (4:w3230:refnum<k34>, 6:w3229:string, 15:w3219:errorcluster)  [unwired: 2 in, 1 out]
                            n2034 = TDMS Write(0:w3230, 5:w3229, 7:w3225, 9:w3220, 11:w3219) -> (4:w3228:refnum<k34>, 6:w3227:string, 15:w3218:errorcluster)  [unwired: 1 in, 1 out]
                            n2035 = TDMS Write(0:w3228, 5:w3227, 7:w3253, 9:w3251, 11:w3218) -> (4:w3250:refnum<k34>, 6:w3249:string, 15:w3248:errorcluster)  [unwired: 1 in, 1 out]
                            n2036 = TDMS Write(0:w3250, 5:w3249, 7:w3247, 9:w3246, 11:w3248) -> (4:w3245:refnum<k34>, 6:w3244:string, 15:w3243:errorcluster)  [unwired: 1 in, 1 out]
                            n2037 = TDMS Write(0:w3245, 5:w3244, 7:w3242, 9:w3241, 11:w3243) -> (4:w3240:refnum<k34>, 6:w3239:string, 15:w3238:errorcluster)  [unwired: 1 in, 1 out]
                            n2038 = TDMS Write(0:w3240, 5:w3239, 7:w3237, 9:w3236, 11:w3238) -> (4:w3235:refnum<k34>, 6:w3234:string, 15:w3233:errorcluster)  [unwired: 1 in, 1 out]
                            n2039 = TDMS Write(0:w3235, 5:w3234, 7:w3232, 9:w3231, 11:w3233) -> (4:w3263:refnum<k34>, 6:w3267:string, 15:w3268:errorcluster)  [unwired: 1 in, 1 out]
                            n2040 = TDMS Write(0:w3263, 5:w3267, 7:"TIME", 9:w3265, 11:w3268) -> (15:w3264:errorcluster)  [unwired: 1 in, 3 out]
                            n2041 = local write "data file error"(w3264) -> ()
                          }
                        }
                      }
                    }
                  }
                }
              }
              frame #5 {
                n2042 = case shown="True" w3272 {
                  tunnel: w3275 -> [_ w3279]
                  tunnel: w3274 -> [_ w3278]
                  tunnel: w3273 -> [_ w3276]
                  frame False {
                  }
                  frame True {
                    n2043 = local read "DISP LAB03-2"() -> (w3280:T4)
                    n2044 = local read "SIG LAB03-2"() -> (w3281:T2)
                    n2045 = local read "ON L03-2"() -> (w3277:cluster{"amps":dbl, "volts":dbl, "pf":dbl})
                    n2046 = Unbundle(w3281) -> ("AMPS"=w3287:dbl, "VOLTS"=w3285:dbl, "PF"=w3284:dbl, "Tmp Live"=w3283:dbl, "Tmp Neut"=w3286:dbl)
                    n2047 = Unbundle(w3280) -> ("CYCLE"=w3282:dbl)  [unwired: 2 out]
                    n2048 = stacked-sequence {
                      tunnel: w3287 -> [w3291 w3309]
                      tunnel: w3286 -> [_ w3308]
                      tunnel: w3285 -> [w3290 w3307]
                      tunnel: w3284 -> [w3289 w3306]
                      tunnel: w3283 -> [_ w3305]
                      tunnel: w3282 -> [_ w3304]
                      tunnel: w3279 -> [_ w3303]
                      tunnel: w3278 -> [w3292 _]
                      tunnel: w3277 -> [w3288 w3301]
                      tunnel: w3276 -> [_ w3302]
                      frame #0 {
                        n2049 = case shown="True" w3292 {
                          tunnel: w3291 -> [_ w3297]
                          tunnel: w3290 -> [_ w3296]
                          tunnel: w3289 -> [_ w3295]
                          tunnel: w3288 -> [_ w3293]
                          frame False {
                          }
                          frame True {
                            n2050 = Bundle(cluster=w3293, "amps"=w3297, "volts"=w3296, "pf"=w3295) -> (w3294:cluster{"amps":dbl, "volts":dbl, "pf":dbl})
                            n2051 = local write "ON L03-2"(w3294) -> ()
                          }
                        }
                      }
                      frame #1 {
                        n2052 = Unbundle(w3301) -> ("amps"=w3300:dbl, "volts"=w3299:dbl, "pf"=w3298:dbl)
                        n2053 = case shown="True" w3302 {
                          tunnel: w3309 -> [_ w3314]
                          tunnel: w3308 -> [_ w3363]
                          tunnel: w3307 -> [_ _]
                          tunnel: w3306 -> [_ _]
                          tunnel: w3305 -> [_ w3362]
                          tunnel: w3304 -> [_ w3361]
                          tunnel: w3303 -> [_ w3357]
                          tunnel: w3300 -> [_ w3316]
                          tunnel: w3299 -> [_ w3315]
                          tunnel: w3298 -> [_ w3313]
                          frame False {
                          }
                          frame True {
                            n2054 = local read "TDMS LAB03-2"() -> (w3354:refnum<k34>)
                            n2055 = Build Array(w3315) -> (w3343:dbl[])
                            n2056 = Build Array(w3313) -> (w3338:dbl[])
                            n2057 = Build Array(w3362) -> (w3333:dbl[])
                            n2058 = Build Array(w3363) -> (w3328:dbl[])
                            n2059 = Build Array(w3316) -> (w3350:dbl[])
                            n2060 = Build Array(w3314) -> (w3312:dbl[])
                            n2061 = Build Array(w3361) -> (w3323:dbl[])
                            n2062 = Build Array("TEMP Neut") -> (w3329:string[])
                            n2063 = Build Array("CYCLE") -> (w3324:string[])
                            n2064 = Build Array("TEMP Live") -> (w3334:string[])
                            n2065 = Build Array("PF") -> (w3339:string[])
                            n2066 = Build Array("AMPS OFF") -> (w3317:string[])
                            n2067 = Build Array("AMPS ON") -> (w3351:string[])
                            n2068 = Build Array("VOLTS") -> (w3345:string[])
                            n2069 = TDMS Write(0:w3354, 5:"LAB03-2 TEST VALUES", 7:w3351, 9:w3350) -> (4:w3322:refnum<k34>, 6:w3321:string, 15:w3311:errorcluster)  [unwired: 2 in, 1 out]
                            n2070 = TDMS Write(0:w3322, 5:w3321, 7:w3317, 9:w3312, 11:w3311) -> (4:w3320:refnum<k34>, 6:w3319:string, 15:w3310:errorcluster)  [unwired: 1 in, 1 out]
                            n2071 = TDMS Write(0:w3320, 5:w3319, 7:w3345, 9:w3343, 11:w3310) -> (4:w3342:refnum<k34>, 6:w3341:string, 15:w3340:errorcluster)  [unwired: 1 in, 1 out]
                            n2072 = TDMS Write(0:w3342, 5:w3341, 7:w3339, 9:w3338, 11:w3340) -> (4:w3337:refnum<k34>, 6:w3336:string, 15:w3335:errorcluster)  [unwired: 1 in, 1 out]
                            n2073 = TDMS Write(0:w3337, 5:w3336, 7:w3334, 9:w3333, 11:w3335) -> (4:w3332:refnum<k34>, 6:w3331:string, 15:w3330:errorcluster)  [unwired: 1 in, 1 out]
                            n2074 = TDMS Write(0:w3332, 5:w3331, 7:w3329, 9:w3328, 11:w3330) -> (4:w3327:refnum<k34>, 6:w3326:string, 15:w3325:errorcluster)  [unwired: 1 in, 1 out]
                            n2075 = TDMS Write(0:w3327, 5:w3326, 7:w3324, 9:w3323, 11:w3325) -> (4:w3355:refnum<k34>, 6:w3359:string, 15:w3360:errorcluster)  [unwired: 1 in, 1 out]
                            n2076 = TDMS Write(0:w3355, 5:w3359, 7:"TIME", 9:w3357, 11:w3360) -> (15:w3356:errorcluster)  [unwired: 1 in, 3 out]
                            n2077 = local write "data file error"(w3356) -> ()
                          }
                        }
                      }
                    }
                  }
                }
              }
              frame #6 {
                n2078 = case shown="True" w3364 {
                  tunnel: w3367 -> [_ w3371]
                  tunnel: w3366 -> [_ w3370]
                  tunnel: w3365 -> [_ w3368]
                  frame False {
                  }
                  frame True {
                    n2079 = local read "DISP LAB04-1"() -> (w3372:T4)
                    n2080 = local read "SIG LAB04-1"() -> (w3373:T2)
                    n2081 = local read "ON L04-1"() -> (w3369:cluster{"amps":dbl, "volts":dbl, "pf":dbl})
                    n2082 = Unbundle(w3373) -> ("AMPS"=w3379:dbl, "VOLTS"=w3377:dbl, "PF"=w3376:dbl, "Tmp Live"=w3375:dbl, "Tmp Neut"=w3378:dbl)
                    n2083 = Unbundle(w3372) -> ("CYCLE"=w3374:dbl)  [unwired: 2 out]
                    n2084 = stacked-sequence {
                      tunnel: w3379 -> [w3383 w3401]
                      tunnel: w3378 -> [_ w3400]
                      tunnel: w3377 -> [w3382 w3399]
                      tunnel: w3376 -> [w3381 w3398]
                      tunnel: w3375 -> [_ w3397]
                      tunnel: w3374 -> [_ w3396]
                      tunnel: w3371 -> [_ w3395]
                      tunnel: w3370 -> [w3384 _]
                      tunnel: w3369 -> [w3380 w3393]
                      tunnel: w3368 -> [_ w3394]
                      frame #0 {
                        n2085 = case shown="True" w3384 {
                          tunnel: w3383 -> [_ w3389]
                          tunnel: w3382 -> [_ w3388]
                          tunnel: w3381 -> [_ w3387]
                          tunnel: w3380 -> [_ w3385]
                          frame False {
                          }
                          frame True {
                            n2086 = Bundle(cluster=w3385, "amps"=w3389, "volts"=w3388, "pf"=w3387) -> (w3386:cluster{"amps":dbl, "volts":dbl, "pf":dbl})
                            n2087 = local write "ON L04-1"(w3386) -> ()
                          }
                        }
                      }
                      frame #1 {
                        n2088 = Unbundle(w3393) -> ("amps"=w3392:dbl, "volts"=w3391:dbl, "pf"=w3390:dbl)
                        n2089 = case shown="True" w3394 {
                          tunnel: w3401 -> [_ w3406]
                          tunnel: w3400 -> [_ w3455]
                          tunnel: w3399 -> [_ _]
                          tunnel: w3398 -> [_ _]
                          tunnel: w3397 -> [_ w3454]
                          tunnel: w3396 -> [_ w3453]
                          tunnel: w3395 -> [_ w3449]
                          tunnel: w3392 -> [_ w3408]
                          tunnel: w3391 -> [_ w3407]
                          tunnel: w3390 -> [_ w3405]
                          frame False {
                          }
                          frame True {
                            n2090 = local read "TDMS LAB04-1"() -> (w3446:refnum<k34>)
                            n2091 = Build Array(w3407) -> (w3435:dbl[])
                            n2092 = Build Array(w3405) -> (w3430:dbl[])
                            n2093 = Build Array(w3454) -> (w3425:dbl[])
                            n2094 = Build Array(w3455) -> (w3420:dbl[])
                            n2095 = Build Array(w3408) -> (w3442:dbl[])
                            n2096 = Build Array(w3406) -> (w3404:dbl[])
                            n2097 = Build Array(w3453) -> (w3415:dbl[])
                            n2098 = Build Array("TEMP Neut") -> (w3421:string[])
                            n2099 = Build Array("CYCLE") -> (w3416:string[])
                            n2100 = Build Array("TEMP Live") -> (w3426:string[])
                            n2101 = Build Array("PF") -> (w3431:string[])
                            n2102 = Build Array("AMPS OFF") -> (w3409:string[])
                            n2103 = Build Array("AMPS ON") -> (w3443:string[])
                            n2104 = Build Array("VOLTS") -> (w3437:string[])
                            n2105 = TDMS Write(0:w3446, 5:"LAB04-1 TEST VALUES", 7:w3443, 9:w3442) -> (4:w3414:refnum<k34>, 6:w3413:string, 15:w3403:errorcluster)  [unwired: 2 in, 1 out]
                            n2106 = TDMS Write(0:w3414, 5:w3413, 7:w3409, 9:w3404, 11:w3403) -> (4:w3412:refnum<k34>, 6:w3411:string, 15:w3402:errorcluster)  [unwired: 1 in, 1 out]
                            n2107 = TDMS Write(0:w3412, 5:w3411, 7:w3437, 9:w3435, 11:w3402) -> (4:w3434:refnum<k34>, 6:w3433:string, 15:w3432:errorcluster)  [unwired: 1 in, 1 out]
                            n2108 = TDMS Write(0:w3434, 5:w3433, 7:w3431, 9:w3430, 11:w3432) -> (4:w3429:refnum<k34>, 6:w3428:string, 15:w3427:errorcluster)  [unwired: 1 in, 1 out]
                            n2109 = TDMS Write(0:w3429, 5:w3428, 7:w3426, 9:w3425, 11:w3427) -> (4:w3424:refnum<k34>, 6:w3423:string, 15:w3422:errorcluster)  [unwired: 1 in, 1 out]
                            n2110 = TDMS Write(0:w3424, 5:w3423, 7:w3421, 9:w3420, 11:w3422) -> (4:w3419:refnum<k34>, 6:w3418:string, 15:w3417:errorcluster)  [unwired: 1 in, 1 out]
                            n2111 = TDMS Write(0:w3419, 5:w3418, 7:w3416, 9:w3415, 11:w3417) -> (4:w3447:refnum<k34>, 6:w3451:string, 15:w3452:errorcluster)  [unwired: 1 in, 1 out]
                            n2112 = TDMS Write(0:w3447, 5:w3451, 7:"TIME", 9:w3449, 11:w3452) -> (15:w3448:errorcluster)  [unwired: 1 in, 3 out]
                            n2113 = local write "data file error"(w3448) -> ()
                          }
                        }
                      }
                    }
                  }
                }
              }
              frame #7 {
                n2114 = case shown="True" w3456 {
                  tunnel: w3459 -> [_ w3463]
                  tunnel: w3458 -> [_ w3462]
                  tunnel: w3457 -> [_ w3460]
                  frame False {
                  }
                  frame True {
                    n2115 = local read "DISP LAB04-2"() -> (w3464:T4)
                    n2116 = local read "SIG LAB04-2"() -> (w3465:T2)
                    n2117 = local read "ON L04-2"() -> (w3461:cluster{"amps":dbl, "volts":dbl, "pf":dbl})
                    n2118 = Unbundle(w3465) -> ("AMPS"=w3471:dbl, "VOLTS"=w3469:dbl, "PF"=w3468:dbl, "Tmp Live"=w3467:dbl, "Tmp Neut"=w3470:dbl)
                    n2119 = Unbundle(w3464) -> ("CYCLE"=w3466:dbl)  [unwired: 2 out]
                    n2120 = stacked-sequence {
                      tunnel: w3471 -> [w3475 w3493]
                      tunnel: w3470 -> [_ w3492]
                      tunnel: w3469 -> [w3474 w3491]
                      tunnel: w3468 -> [w3473 w3490]
                      tunnel: w3467 -> [_ w3489]
                      tunnel: w3466 -> [_ w3488]
                      tunnel: w3463 -> [_ w3487]
                      tunnel: w3462 -> [w3476 _]
                      tunnel: w3461 -> [w3472 w3485]
                      tunnel: w3460 -> [_ w3486]
                      frame #0 {
                        n2121 = case shown="True" w3476 {
                          tunnel: w3475 -> [_ w3481]
                          tunnel: w3474 -> [_ w3480]
                          tunnel: w3473 -> [_ w3479]
                          tunnel: w3472 -> [_ w3477]
                          frame False {
                          }
                          frame True {
                            n2122 = Bundle(cluster=w3477, "amps"=w3481, "volts"=w3480, "pf"=w3479) -> (w3478:cluster{"amps":dbl, "volts":dbl, "pf":dbl})
                            n2123 = local write "ON L04-2"(w3478) -> ()
                          }
                        }
                      }
                      frame #1 {
                        n2124 = Unbundle(w3485) -> ("amps"=w3484:dbl, "volts"=w3483:dbl, "pf"=w3482:dbl)
                        n2125 = case shown="True" w3486 {
                          tunnel: w3493 -> [_ w3498]
                          tunnel: w3492 -> [_ w3547]
                          tunnel: w3491 -> [_ _]
                          tunnel: w3490 -> [_ _]
                          tunnel: w3489 -> [_ w3546]
                          tunnel: w3488 -> [_ w3545]
                          tunnel: w3487 -> [_ w3541]
                          tunnel: w3484 -> [_ w3500]
                          tunnel: w3483 -> [_ w3499]
                          tunnel: w3482 -> [_ w3497]
                          frame False {
                          }
                          frame True {
                            n2126 = local read "TDMS LAB04-2"() -> (w3538:refnum<k34>)
                            n2127 = Build Array(w3499) -> (w3527:dbl[])
                            n2128 = Build Array(w3497) -> (w3522:dbl[])
                            n2129 = Build Array(w3546) -> (w3517:dbl[])
                            n2130 = Build Array(w3547) -> (w3512:dbl[])
                            n2131 = Build Array(w3500) -> (w3534:dbl[])
                            n2132 = Build Array(w3498) -> (w3496:dbl[])
                            n2133 = Build Array(w3545) -> (w3507:dbl[])
                            n2134 = Build Array("TEMP Neut") -> (w3513:string[])
                            n2135 = Build Array("CYCLE") -> (w3508:string[])
                            n2136 = Build Array("TEMP Live") -> (w3518:string[])
                            n2137 = Build Array("PF") -> (w3523:string[])
                            n2138 = Build Array("AMPS OFF") -> (w3501:string[])
                            n2139 = Build Array("AMPS ON") -> (w3535:string[])
                            n2140 = Build Array("VOLTS") -> (w3529:string[])
                            n2141 = TDMS Write(0:w3538, 5:"LAB04-2 TEST VALUES", 7:w3535, 9:w3534) -> (4:w3506:refnum<k34>, 6:w3505:string, 15:w3495:errorcluster)  [unwired: 2 in, 1 out]
                            n2142 = TDMS Write(0:w3506, 5:w3505, 7:w3501, 9:w3496, 11:w3495) -> (4:w3504:refnum<k34>, 6:w3503:string, 15:w3494:errorcluster)  [unwired: 1 in, 1 out]
                            n2143 = TDMS Write(0:w3504, 5:w3503, 7:w3529, 9:w3527, 11:w3494) -> (4:w3526:refnum<k34>, 6:w3525:string, 15:w3524:errorcluster)  [unwired: 1 in, 1 out]
                            n2144 = TDMS Write(0:w3526, 5:w3525, 7:w3523, 9:w3522, 11:w3524) -> (4:w3521:refnum<k34>, 6:w3520:string, 15:w3519:errorcluster)  [unwired: 1 in, 1 out]
                            n2145 = TDMS Write(0:w3521, 5:w3520, 7:w3518, 9:w3517, 11:w3519) -> (4:w3516:refnum<k34>, 6:w3515:string, 15:w3514:errorcluster)  [unwired: 1 in, 1 out]
                            n2146 = TDMS Write(0:w3516, 5:w3515, 7:w3513, 9:w3512, 11:w3514) -> (4:w3511:refnum<k34>, 6:w3510:string, 15:w3509:errorcluster)  [unwired: 1 in, 1 out]
                            n2147 = TDMS Write(0:w3511, 5:w3510, 7:w3508, 9:w3507, 11:w3509) -> (4:w3539:refnum<k34>, 6:w3543:string, 15:w3544:errorcluster)  [unwired: 1 in, 1 out]
                            n2148 = TDMS Write(0:w3539, 5:w3543, 7:"TIME", 9:w3541, 11:w3544) -> (15:w3540:errorcluster)  [unwired: 1 in, 3 out]
                            n2149 = local write "data file error"(w3540) -> ()
                          }
                        }
                      }
                    }
                  }
                }
              }
              frame #8 {
                n2150 = case shown="True" w3548 {
                  tunnel: w3551 -> [_ w3555]
                  tunnel: w3550 -> [_ w3554]
                  tunnel: w3549 -> [_ w3552]
                  frame False {
                  }
                  frame True {
                    n2151 = local read "DISP LAB05-1"() -> (w3556:T4)
                    n2152 = local read "SIG LAB05-1"() -> (w3557:T2)
                    n2153 = local read "ON L05-1"() -> (w3553:cluster{"amps":dbl, "volts":dbl, "pf":dbl})
                    n2154 = Unbundle(w3557) -> ("AMPS"=w3563:dbl, "VOLTS"=w3561:dbl, "PF"=w3560:dbl, "Tmp Live"=w3559:dbl, "Tmp Neut"=w3562:dbl)
                    n2155 = Unbundle(w3556) -> ("CYCLE"=w3558:dbl)  [unwired: 2 out]
                    n2156 = stacked-sequence {
                      tunnel: w3563 -> [w3567 w3585]
                      tunnel: w3562 -> [_ w3584]
                      tunnel: w3561 -> [w3566 w3583]
                      tunnel: w3560 -> [w3565 w3582]
                      tunnel: w3559 -> [_ w3581]
                      tunnel: w3558 -> [_ w3580]
                      tunnel: w3555 -> [_ w3579]
                      tunnel: w3554 -> [w3568 _]
                      tunnel: w3553 -> [w3564 w3577]
                      tunnel: w3552 -> [_ w3578]
                      frame #0 {
                        n2157 = case shown="True" w3568 {
                          tunnel: w3567 -> [_ w3573]
                          tunnel: w3566 -> [_ w3572]
                          tunnel: w3565 -> [_ w3571]
                          tunnel: w3564 -> [_ w3569]
                          frame False {
                          }
                          frame True {
                            n2158 = Bundle(cluster=w3569, "amps"=w3573, "volts"=w3572, "pf"=w3571) -> (w3570:cluster{"amps":dbl, "volts":dbl, "pf":dbl})
                            n2159 = local write "ON L05-1"(w3570) -> ()
                          }
                        }
                      }
                      frame #1 {
                        n2160 = Unbundle(w3577) -> ("amps"=w3576:dbl, "volts"=w3575:dbl, "pf"=w3574:dbl)
                        n2161 = case shown="True" w3578 {
                          tunnel: w3585 -> [_ w3590]
                          tunnel: w3584 -> [_ w3639]
                          tunnel: w3583 -> [_ _]
                          tunnel: w3582 -> [_ _]
                          tunnel: w3581 -> [_ w3638]
                          tunnel: w3580 -> [_ w3637]
                          tunnel: w3579 -> [_ w3633]
                          tunnel: w3576 -> [_ w3592]
                          tunnel: w3575 -> [_ w3591]
                          tunnel: w3574 -> [_ w3589]
                          frame False {
                          }
                          frame True {
                            n2162 = local read "TDMS LAB05-1"() -> (w3630:refnum<k34>)
                            n2163 = Build Array(w3591) -> (w3619:dbl[])
                            n2164 = Build Array(w3589) -> (w3614:dbl[])
                            n2165 = Build Array(w3638) -> (w3609:dbl[])
                            n2166 = Build Array(w3639) -> (w3604:dbl[])
                            n2167 = Build Array(w3592) -> (w3626:dbl[])
                            n2168 = Build Array(w3590) -> (w3588:dbl[])
                            n2169 = Build Array(w3637) -> (w3599:dbl[])
                            n2170 = Build Array("TEMP Neut") -> (w3605:string[])
                            n2171 = Build Array("CYCLE") -> (w3600:string[])
                            n2172 = Build Array("TEMP Live") -> (w3610:string[])
                            n2173 = Build Array("PF") -> (w3615:string[])
                            n2174 = Build Array("AMPS OFF") -> (w3593:string[])
                            n2175 = Build Array("AMPS ON") -> (w3627:string[])
                            n2176 = Build Array("VOLTS") -> (w3621:string[])
                            n2177 = TDMS Write(0:w3630, 5:"LAB05-1 TEST VALUES", 7:w3627, 9:w3626) -> (4:w3598:refnum<k34>, 6:w3597:string, 15:w3587:errorcluster)  [unwired: 2 in, 1 out]
                            n2178 = TDMS Write(0:w3598, 5:w3597, 7:w3593, 9:w3588, 11:w3587) -> (4:w3596:refnum<k34>, 6:w3595:string, 15:w3586:errorcluster)  [unwired: 1 in, 1 out]
                            n2179 = TDMS Write(0:w3596, 5:w3595, 7:w3621, 9:w3619, 11:w3586) -> (4:w3618:refnum<k34>, 6:w3617:string, 15:w3616:errorcluster)  [unwired: 1 in, 1 out]
                            n2180 = TDMS Write(0:w3618, 5:w3617, 7:w3615, 9:w3614, 11:w3616) -> (4:w3613:refnum<k34>, 6:w3612:string, 15:w3611:errorcluster)  [unwired: 1 in, 1 out]
                            n2181 = TDMS Write(0:w3613, 5:w3612, 7:w3610, 9:w3609, 11:w3611) -> (4:w3608:refnum<k34>, 6:w3607:string, 15:w3606:errorcluster)  [unwired: 1 in, 1 out]
                            n2182 = TDMS Write(0:w3608, 5:w3607, 7:w3605, 9:w3604, 11:w3606) -> (4:w3603:refnum<k34>, 6:w3602:string, 15:w3601:errorcluster)  [unwired: 1 in, 1 out]
                            n2183 = TDMS Write(0:w3603, 5:w3602, 7:w3600, 9:w3599, 11:w3601) -> (4:w3631:refnum<k34>, 6:w3635:string, 15:w3636:errorcluster)  [unwired: 1 in, 1 out]
                            n2184 = TDMS Write(0:w3631, 5:w3635, 7:"TIME", 9:w3633, 11:w3636) -> (15:w3632:errorcluster)  [unwired: 1 in, 3 out]
                            n2185 = local write "data file error"(w3632) -> ()
                          }
                        }
                      }
                    }
                  }
                }
              }
              frame #9 {
                n2186 = case shown="True" w3640 {
                  tunnel: w3643 -> [_ w3647]
                  tunnel: w3642 -> [_ w3646]
                  tunnel: w3641 -> [_ w3644]
                  frame False {
                  }
                  frame True {
                    n2187 = local read "DISP LAB05-2"() -> (w3648:T4)
                    n2188 = local read "SIG LAB05-2"() -> (w3649:T2)
                    n2189 = local read "ON L05-2"() -> (w3645:cluster{"amps":dbl, "volts":dbl, "pf":dbl})
                    n2190 = Unbundle(w3649) -> ("AMPS"=w3655:dbl, "VOLTS"=w3653:dbl, "PF"=w3652:dbl, "Tmp Live"=w3651:dbl, "Tmp Neut"=w3654:dbl)
                    n2191 = Unbundle(w3648) -> ("CYCLE"=w3650:dbl)  [unwired: 2 out]
                    n2192 = stacked-sequence {
                      tunnel: w3655 -> [w3659 w3677]
                      tunnel: w3654 -> [_ w3676]
                      tunnel: w3653 -> [w3658 w3675]
                      tunnel: w3652 -> [w3657 w3674]
                      tunnel: w3651 -> [_ w3673]
                      tunnel: w3650 -> [_ w3672]
                      tunnel: w3647 -> [_ w3671]
                      tunnel: w3646 -> [w3660 _]
                      tunnel: w3645 -> [w3656 w3669]
                      tunnel: w3644 -> [_ w3670]
                      frame #0 {
                        n2193 = case shown="True" w3660 {
                          tunnel: w3659 -> [_ w3665]
                          tunnel: w3658 -> [_ w3664]
                          tunnel: w3657 -> [_ w3663]
                          tunnel: w3656 -> [_ w3661]
                          frame False {
                          }
                          frame True {
                            n2194 = Bundle(cluster=w3661, "amps"=w3665, "volts"=w3664, "pf"=w3663) -> (w3662:cluster{"amps":dbl, "volts":dbl, "pf":dbl})
                            n2195 = local write "ON L05-2"(w3662) -> ()
                          }
                        }
                      }
                      frame #1 {
                        n2196 = Unbundle(w3669) -> ("amps"=w3668:dbl, "volts"=w3667:dbl, "pf"=w3666:dbl)
                        n2197 = case shown="True" w3670 {
                          tunnel: w3677 -> [_ w3682]
                          tunnel: w3676 -> [_ w3731]
                          tunnel: w3675 -> [_ _]
                          tunnel: w3674 -> [_ _]
                          tunnel: w3673 -> [_ w3730]
                          tunnel: w3672 -> [_ w3729]
                          tunnel: w3671 -> [_ w3725]
                          tunnel: w3668 -> [_ w3684]
                          tunnel: w3667 -> [_ w3683]
                          tunnel: w3666 -> [_ w3681]
                          frame False {
                          }
                          frame True {
                            n2198 = local read "TDMS LAB05-2"() -> (w3722:refnum<k34>)
                            n2199 = Build Array(w3683) -> (w3711:dbl[])
                            n2200 = Build Array(w3681) -> (w3706:dbl[])
                            n2201 = Build Array(w3730) -> (w3701:dbl[])
                            n2202 = Build Array(w3731) -> (w3696:dbl[])
                            n2203 = Build Array(w3684) -> (w3718:dbl[])
                            n2204 = Build Array(w3682) -> (w3680:dbl[])
                            n2205 = Build Array(w3729) -> (w3691:dbl[])
                            n2206 = Build Array("TEMP Neut") -> (w3697:string[])
                            n2207 = Build Array("CYCLE") -> (w3692:string[])
                            n2208 = Build Array("TEMP Live") -> (w3702:string[])
                            n2209 = Build Array("PF") -> (w3707:string[])
                            n2210 = Build Array("AMPS OFF") -> (w3685:string[])
                            n2211 = Build Array("AMPS ON") -> (w3719:string[])
                            n2212 = Build Array("VOLTS") -> (w3713:string[])
                            n2213 = TDMS Write(0:w3722, 5:"LAB05-2 TEST VALUES", 7:w3719, 9:w3718) -> (4:w3690:refnum<k34>, 6:w3689:string, 15:w3679:errorcluster)  [unwired: 2 in, 1 out]
                            n2214 = TDMS Write(0:w3690, 5:w3689, 7:w3685, 9:w3680, 11:w3679) -> (4:w3688:refnum<k34>, 6:w3687:string, 15:w3678:errorcluster)  [unwired: 1 in, 1 out]
                            n2215 = TDMS Write(0:w3688, 5:w3687, 7:w3713, 9:w3711, 11:w3678) -> (4:w3710:refnum<k34>, 6:w3709:string, 15:w3708:errorcluster)  [unwired: 1 in, 1 out]
                            n2216 = TDMS Write(0:w3710, 5:w3709, 7:w3707, 9:w3706, 11:w3708) -> (4:w3705:refnum<k34>, 6:w3704:string, 15:w3703:errorcluster)  [unwired: 1 in, 1 out]
                            n2217 = TDMS Write(0:w3705, 5:w3704, 7:w3702, 9:w3701, 11:w3703) -> (4:w3700:refnum<k34>, 6:w3699:string, 15:w3698:errorcluster)  [unwired: 1 in, 1 out]
                            n2218 = TDMS Write(0:w3700, 5:w3699, 7:w3697, 9:w3696, 11:w3698) -> (4:w3695:refnum<k34>, 6:w3694:string, 15:w3693:errorcluster)  [unwired: 1 in, 1 out]
                            n2219 = TDMS Write(0:w3695, 5:w3694, 7:w3692, 9:w3691, 11:w3693) -> (4:w3723:refnum<k34>, 6:w3727:string, 15:w3728:errorcluster)  [unwired: 1 in, 1 out]
                            n2220 = TDMS Write(0:w3723, 5:w3727, 7:"TIME", 9:w3725, 11:w3728) -> (15:w3724:errorcluster)  [unwired: 1 in, 3 out]
                            n2221 = local write "data file error"(w3724) -> ()
                          }
                        }
                      }
                    }
                  }
                }
              }
            }
          }
          frame #14 {
            # "check for amps fail"
            # "check for cycle test & temperature rise fail conditions"
            n2222 = local read "on loops"() -> (w3757:dbl)
            n2223 = local read "jig cycle"() -> (w3754:dbl)
            n2224 = local read "jig cycle"() -> (w3759:dbl)
            n2225 = Add(x=w3757, y=3.0) -> (x+y=w3755:dbl)
            n2226 = Equal?(x=w3754, y=w3755) -> (x = y?=w3750:bool)
            n2227 = Equal?(x=w3759, y=1.0) -> (x = y?=w3752:bool)
            n2228 = stacked-sequence {
              tunnel: w3753 -> [w3762 _ _ _ _ _ _ _ _ _]
              tunnel: w3752 -> [w3763 w3783 w3803 w3823 w3843 w3863 w3883 w3903 w3923 w3943]
              tunnel: w3751 -> [w3760 _ _ _ _ _ _ _ _ _]
              tunnel: w3750 -> [w3761 w3782 w3802 w3822 w3842 w3862 w3882 w3902 w3922 w3942]
              tunnel: w3749 -> [_ w3781 _ _ _ _ _ _ _ _]
              tunnel: w3748 -> [_ w3780 _ _ _ _ _ _ _ _]
              tunnel: w3747 -> [_ _ w3801 _ _ _ _ _ _ _]
              tunnel: w3746 -> [_ _ w3800 _ _ _ _ _ _ _]
              tunnel: w3745 -> [_ _ _ w3821 _ _ _ _ _ _]
              tunnel: w3744 -> [_ _ _ w3820 _ _ _ _ _ _]
              tunnel: w3743 -> [_ _ _ _ w3841 _ _ _ _ _]
              tunnel: w3742 -> [_ _ _ _ w3840 _ _ _ _ _]
              tunnel: w3741 -> [_ _ _ _ _ w3861 _ _ _ _]
              tunnel: w3740 -> [_ _ _ _ _ w3860 _ _ _ _]
              tunnel: w3739 -> [_ _ _ _ _ _ w3881 _ _ _]
              tunnel: w3738 -> [_ _ _ _ _ _ w3880 _ _ _]
              tunnel: w3737 -> [_ _ _ _ _ _ _ w3901 _ _]
              tunnel: w3736 -> [_ _ _ _ _ _ _ w3900 _ _]
              tunnel: w3735 -> [_ _ _ _ _ _ _ _ w3921 _]
              tunnel: w3734 -> [_ _ _ _ _ _ _ _ w3920 _]
              tunnel: w3733 -> [_ _ _ _ _ _ _ _ _ w3941]
              tunnel: w3732 -> [_ _ _ _ _ _ _ _ _ w3940]
              frame #0 {
                # "LAB01-1"
                n2229 = case shown="True" w3760 {
                  tunnel: w3763 -> [_ w3776]
                  tunnel: w3762 -> [_ w3773]
                  tunnel: w3761 -> [_ w3772]
                  frame False {
                  }
                  frame True {
                    n2230 = local read "TEMP START LAB01-1"() -> (w3778:cluster{"TL":dbl, "TN":dbl})
                    n2231 = local read "RESULT LAB01-1"() -> (w3767:bool)
                    n2232 = local read "FAIL LAB01-1"() -> (w3770:cluster{"LO":dbl, "HI":dbl})
                    n2233 = local read "TDMS LAB01-1"() -> (w3777:refnum<k34>)
                    n2234 = local read "SET LAB01-1"() -> (w3774:T5)
                    n2235 = local read "DISP LAB01-1"() -> (w3775:T4)
                    n2236 = local read "SIG LAB01-1"() -> (w3779:T2)
                    n2237 = Bundle("FAIL LAB01-1"=w3770, "SIG LAB01-1"=w3779, "TEMP START LAB01-1"=w3778, "DISP LAB01-1"=w3775, "SET LAB01-1"=w3774, "TDMS LAB01-1"=w3777) -> (w3764:T26)  [unwired: 1 in]
                    n2238 = call "sub vi - cycle&temp fail v6.vi"("Amps Lo?"=w3776, "Input Cluster"=w3764, "SELECT"=w3773, "Amps Hi?"=w3772, "Result In"=w3767) -> ("(FAIL) out"=w3769:cluster{"FAIL LO":dbl, "FAIL HI":dbl}, "(DISP) out"=w3765:T4, "T-RISE"=w3766:cluster{"T-RISE (L)":dbl, "T-RISE (N)":dbl}, "Result Out"=w3768:bool, "file error"=w3771:errorcluster)  [unwired: 10 in]
                    n2239 = local write "TEMP RISE LAB01-1"(w3766) -> ()
                    n2240 = local write "FAIL LAB01-1"(w3769) -> ()
                    n2241 = local write "DISP LAB01-1"(w3765) -> ()
                    n2242 = local write "RESULT LAB01-1"(w3768) -> ()
                    n2243 = local write "data file error"(w3771) -> ()
                  }
                }
              }
              frame #1 {
                # "LAB01-2"
                n2244 = case shown="True" w3781 {
                  tunnel: w3783 -> [_ w3796]
                  tunnel: w3780 -> [_ w3793]
                  tunnel: w3782 -> [_ w3792]
                  frame False {
                  }
                  frame True {
                    n2245 = local read "TEMP START LAB01-2"() -> (w3798:cluster{"TL":dbl, "TN":dbl})
                    n2246 = local read "FAIL LAB01-2"() -> (w3789:cluster{"LO":dbl, "HI":dbl})
                    n2247 = local read "TDMS LAB01-2"() -> (w3797:refnum<k34>)
                    n2248 = local read "SET LAB01-2"() -> (w3794:T5)
                    n2249 = local read "DISP LAB01-2"() -> (w3795:T4)
                    n2250 = local read "RESULT LAB01-2"() -> (w3786:bool)
                    n2251 = local read "SIG LAB01-2"() -> (w3799:T2)
                    n2252 = Bundle("FAIL LAB01-2"=w3789, "SIG LAB01-2"=w3799, "TEMP START LAB01-2"=w3798, "DISP LAB01-2"=w3795, "SET LAB01-2"=w3794, "TDMS LAB01-2"=w3797) -> (w3784:T27)  [unwired: 1 in]
                    n2253 = call "sub vi - cycle&temp fail v6.vi"("Amps Lo?"=w3796, "Input Cluster"=w3784, "SELECT"=w3793, "Amps Hi?"=w3792, "Result In"=w3786) -> ("(FAIL) out"=w3788:cluster{"FAIL LO":dbl, "FAIL HI":dbl}, "(DISP) out"=w3791:T4, "T-RISE"=w3785:cluster{"T-RISE (L)":dbl, "T-RISE (N)":dbl}, "Result Out"=w3787:bool, "file error"=w3790:errorcluster)  [unwired: 10 in]
                    n2254 = local write "TEMP RISE LAB01-2"(w3785) -> ()
                    n2255 = local write "FAIL LAB01-2"(w3788) -> ()
                    n2256 = local write "DISP LAB01-2"(w3791) -> ()
                    n2257 = local write "RESULT LAB01-2"(w3787) -> ()
                    n2258 = local write "data file error"(w3790) -> ()
                  }
                }
              }
              frame #2 {
                # "LAB02-1"
                n2259 = case shown="True" w3801 {
                  tunnel: w3803 -> [_ w3816]
                  tunnel: w3800 -> [_ w3813]
                  tunnel: w3802 -> [_ w3812]
                  frame False {
                  }
                  frame True {
                    n2260 = local read "TEMP START LAB02-1"() -> (w3818:cluster{"TL":dbl, "TN":dbl})
                    n2261 = local read "FAIL LAB02-1"() -> (w3809:cluster{"LO":dbl, "HI":dbl})
                    n2262 = local read "TDMS LAB02-1"() -> (w3817:refnum<k34>)
                    n2263 = local read "SET LAB02-1"() -> (w3814:T5)
                    n2264 = local read "DISP LAB02-1"() -> (w3815:T4)
                    n2265 = local read "SIG LAB02-1"() -> (w3819:T2)
                    n2266 = local read "RESULT LAB02-1"() -> (w3806:bool)
                    n2267 = Bundle("FAIL LAB02-1"=w3809, "SIG LAB02-1"=w3819, "TEMP START LAB02-1"=w3818, "DISP LAB02-1"=w3815, "SET LAB02-1"=w3814, "TDMS LAB02-1"=w3817) -> (w3804:T28)  [unwired: 1 in]
                    n2268 = call "sub vi - cycle&temp fail v6.vi"("Amps Lo?"=w3816, "Input Cluster"=w3804, "SELECT"=w3813, "Amps Hi?"=w3812, "Result In"=w3806) -> ("(FAIL) out"=w3808:cluster{"FAIL LO":dbl, "FAIL HI":dbl}, "(DISP) out"=w3811:T4, "T-RISE"=w3805:cluster{"T-RISE (L)":dbl, "T-RISE (N)":dbl}, "Result Out"=w3807:bool, "file error"=w3810:errorcluster)  [unwired: 10 in]
                    n2269 = local write "TEMP RISE LAB02-1"(w3805) -> ()
                    n2270 = local write "FAIL LAB02-1"(w3808) -> ()
                    n2271 = local write "DISP LAB02-1"(w3811) -> ()
                    n2272 = local write "RESULT LAB02-1"(w3807) -> ()
                    n2273 = local write "data file error"(w3810) -> ()
                  }
                }
              }
              frame #3 {
                # "LAB02-2"
                n2274 = case shown="True" w3821 {
                  tunnel: w3823 -> [_ w3836]
                  tunnel: w3820 -> [_ w3833]
                  tunnel: w3822 -> [_ w3832]
                  frame False {
                  }
                  frame True {
                    n2275 = local read "TEMP START LAB02-2"() -> (w3838:cluster{"TL":dbl, "TN":dbl})
                    n2276 = local read "FAIL LAB02-2"() -> (w3829:cluster{"LO":dbl, "HI":dbl})
                    n2277 = local read "TDMS LAB02-2"() -> (w3837:refnum<k34>)
                    n2278 = local read "SET LAB02-2"() -> (w3834:T5)
                    n2279 = local read "DISP LAB02-2"() -> (w3835:T4)
                    n2280 = local read "SIG LAB02-2"() -> (w3839:T2)
                    n2281 = local read "RESULT LAB02-2"() -> (w3826:bool)
                    n2282 = Bundle("FAIL LAB02-2"=w3829, "SIG LAB02-2"=w3839, "TEMP START LAB02-2"=w3838, "DISP LAB02-2"=w3835, "SET LAB02-2"=w3834, "TDMS LAB02-2"=w3837) -> (w3824:T29)  [unwired: 1 in]
                    n2283 = call "sub vi - cycle&temp fail v6.vi"("Amps Lo?"=w3836, "Input Cluster"=w3824, "SELECT"=w3833, "Amps Hi?"=w3832, "Result In"=w3826) -> ("(FAIL) out"=w3828:cluster{"FAIL LO":dbl, "FAIL HI":dbl}, "(DISP) out"=w3831:T4, "T-RISE"=w3825:cluster{"T-RISE (L)":dbl, "T-RISE (N)":dbl}, "Result Out"=w3827:bool, "file error"=w3830:errorcluster)  [unwired: 10 in]
                    n2284 = local write "TEMP RISE LAB02-2"(w3825) -> ()
                    n2285 = local write "FAIL LAB02-2"(w3828) -> ()
                    n2286 = local write "DISP LAB02-2"(w3831) -> ()
                    n2287 = local write "RESULT LAB02-2"(w3827) -> ()
                    n2288 = local write "data file error"(w3830) -> ()
                  }
                }
              }
              frame #4 {
                # "LAB03-1"
                n2289 = case shown="True" w3841 {
                  tunnel: w3843 -> [_ w3856]
                  tunnel: w3840 -> [_ w3853]
                  tunnel: w3842 -> [_ w3852]
                  frame False {
                  }
                  frame True {
                    n2290 = local read "TEMP START LAB03-1"() -> (w3858:cluster{"TL":dbl, "TN":dbl})
                    n2291 = local read "FAIL LAB03-1"() -> (w3849:cluster{"LO":dbl, "HI":dbl})
                    n2292 = local read "TDMS LAB03-1"() -> (w3857:refnum<k34>)
                    n2293 = local read "SET LAB03-1"() -> (w3854:T5)
                    n2294 = local read "DISP LAB03-1"() -> (w3855:T4)
                    n2295 = local read "SIG LAB03-1"() -> (w3859:T2)
                    n2296 = local read "RESULT LAB03-1"() -> (w3846:bool)
                    n2297 = Bundle("FAIL LAB03-1"=w3849, "SIG LAB03-1"=w3859, "TEMP START LAB03-1"=w3858, "DISP LAB03-1"=w3855, "SET LAB03-1"=w3854, "TDMS LAB03-1"=w3857) -> (w3844:T30)  [unwired: 1 in]
                    n2298 = call "sub vi - cycle&temp fail v6.vi"("Amps Lo?"=w3856, "Input Cluster"=w3844, "SELECT"=w3853, "Amps Hi?"=w3852, "Result In"=w3846) -> ("(FAIL) out"=w3848:cluster{"FAIL LO":dbl, "FAIL HI":dbl}, "(DISP) out"=w3851:T4, "T-RISE"=w3845:cluster{"T-RISE (L)":dbl, "T-RISE (N)":dbl}, "Result Out"=w3847:bool, "file error"=w3850:errorcluster)  [unwired: 10 in]
                    n2299 = local write "TEMP RISE LAB03-1"(w3845) -> ()
                    n2300 = local write "FAIL LAB03-1"(w3848) -> ()
                    n2301 = local write "DISP LAB03-1"(w3851) -> ()
                    n2302 = local write "RESULT LAB03-1"(w3847) -> ()
                    n2303 = local write "data file error"(w3850) -> ()
                  }
                }
              }
              frame #5 {
                # "LAB03-2"
                n2304 = case shown="True" w3861 {
                  tunnel: w3863 -> [_ w3876]
                  tunnel: w3860 -> [_ w3873]
                  tunnel: w3862 -> [_ w3872]
                  frame False {
                  }
                  frame True {
                    n2305 = local read "TEMP START LAB03-2"() -> (w3878:cluster{"TL":dbl, "TN":dbl})
                    n2306 = local read "FAIL LAB03-2"() -> (w3869:cluster{"LO":dbl, "HI":dbl})
                    n2307 = local read "TDMS LAB03-2"() -> (w3877:refnum<k34>)
                    n2308 = local read "SET LAB03-2"() -> (w3874:T5)
                    n2309 = local read "DISP LAB03-2"() -> (w3875:T4)
                    n2310 = local read "RESULT LAB03-2"() -> (w3866:bool)
                    n2311 = local read "SIG LAB03-2"() -> (w3879:T2)
                    n2312 = Bundle("FAIL LAB03-2"=w3869, "SIG LAB03-2"=w3879, "TEMP START LAB03-2"=w3878, "DISP LAB03-2"=w3875, "SET LAB03-2"=w3874, "TDMS LAB03-2"=w3877) -> (w3864:T31)  [unwired: 1 in]
                    n2313 = call "sub vi - cycle&temp fail v6.vi"("Amps Lo?"=w3876, "Input Cluster"=w3864, "SELECT"=w3873, "Amps Hi?"=w3872, "Result In"=w3866) -> ("(FAIL) out"=w3868:cluster{"FAIL LO":dbl, "FAIL HI":dbl}, "(DISP) out"=w3871:T4, "T-RISE"=w3865:cluster{"T-RISE (L)":dbl, "T-RISE (N)":dbl}, "Result Out"=w3867:bool, "file error"=w3870:errorcluster)  [unwired: 10 in]
                    n2314 = local write "FAIL LAB03-2"(w3868) -> ()
                    n2315 = local write "TEMP RISE LAB03-2"(w3865) -> ()
                    n2316 = local write "DISP LAB03-2"(w3871) -> ()
                    n2317 = local write "RESULT LAB03-2"(w3867) -> ()
                    n2318 = local write "data file error"(w3870) -> ()
                  }
                }
              }
              frame #6 {
                # "LAB04-1"
                n2319 = case shown="True" w3881 {
                  tunnel: w3883 -> [_ w3896]
                  tunnel: w3880 -> [_ w3893]
                  tunnel: w3882 -> [_ w3892]
                  frame False {
                  }
                  frame True {
                    n2320 = local read "TEMP START LAB04-1"() -> (w3898:cluster{"TL":dbl, "TN":dbl})
                    n2321 = local read "FAIL LAB04-1"() -> (w3889:cluster{"LO":dbl, "HI":dbl})
                    n2322 = local read "TDMS LAB04-1"() -> (w3897:refnum<k34>)
                    n2323 = local read "SET LAB04-1"() -> (w3894:T5)
                    n2324 = local read "DISP LAB04-1"() -> (w3895:T4)
                    n2325 = local read "SIG LAB04-1"() -> (w3899:T2)
                    n2326 = local read "RESULT LAB04-1"() -> (w3886:bool)
                    n2327 = Bundle("FAIL LAB04-1"=w3889, "SIG LAB04-1"=w3899, "TEMP START LAB04-1"=w3898, "DISP LAB04-1"=w3895, "SET LAB04-1"=w3894, "TDMS LAB04-1"=w3897) -> (w3884:T32)  [unwired: 1 in]
                    n2328 = call "sub vi - cycle&temp fail v6.vi"("Amps Lo?"=w3896, "Input Cluster"=w3884, "SELECT"=w3893, "Amps Hi?"=w3892, "Result In"=w3886) -> ("(FAIL) out"=w3888:cluster{"FAIL LO":dbl, "FAIL HI":dbl}, "(DISP) out"=w3891:T4, "T-RISE"=w3885:cluster{"T-RISE (L)":dbl, "T-RISE (N)":dbl}, "Result Out"=w3887:bool, "file error"=w3890:errorcluster)  [unwired: 10 in]
                    n2329 = local write "TEMP RISE LAB04-1"(w3885) -> ()
                    n2330 = local write "FAIL LAB04-1"(w3888) -> ()
                    n2331 = local write "DISP LAB04-1"(w3891) -> ()
                    n2332 = local write "RESULT LAB04-1"(w3887) -> ()
                    n2333 = local write "data file error"(w3890) -> ()
                  }
                }
              }
              frame #7 {
                # "LAB04-2"
                n2334 = case shown="True" w3901 {
                  tunnel: w3903 -> [_ w3916]
                  tunnel: w3900 -> [_ w3913]
                  tunnel: w3902 -> [_ w3912]
                  frame False {
                  }
                  frame True {
                    n2335 = local read "TEMP START LAB04-2"() -> (w3918:cluster{"TL":dbl, "TN":dbl})
                    n2336 = local read "FAIL LAB04-2"() -> (w3909:cluster{"LO":dbl, "HI":dbl})
                    n2337 = local read "TDMS LAB04-2"() -> (w3917:refnum<k34>)
                    n2338 = local read "SET LAB04-2"() -> (w3914:T5)
                    n2339 = local read "DISP LAB04-2"() -> (w3915:T4)
                    n2340 = local read "SIG LAB04-2"() -> (w3919:T2)
                    n2341 = local read "RESULT LAB04-2"() -> (w3906:bool)
                    n2342 = Bundle("FAIL LAB04-2"=w3909, "SIG LAB04-2"=w3919, "TEMP START LAB04-2"=w3918, "DISP LAB04-2"=w3915, "SET LAB04-2"=w3914, "TDMS LAB04-2"=w3917) -> (w3904:T33)  [unwired: 1 in]
                    n2343 = call "sub vi - cycle&temp fail v6.vi"("Amps Lo?"=w3916, "Input Cluster"=w3904, "SELECT"=w3913, "Amps Hi?"=w3912, "Result In"=w3906) -> ("(FAIL) out"=w3908:cluster{"FAIL LO":dbl, "FAIL HI":dbl}, "(DISP) out"=w3911:T4, "T-RISE"=w3905:cluster{"T-RISE (L)":dbl, "T-RISE (N)":dbl}, "Result Out"=w3907:bool, "file error"=w3910:errorcluster)  [unwired: 10 in]
                    n2344 = local write "TEMP RISE LAB04-2"(w3905) -> ()
                    n2345 = local write "FAIL LAB04-2"(w3908) -> ()
                    n2346 = local write "DISP LAB04-2"(w3911) -> ()
                    n2347 = local write "RESULT LAB04-2"(w3907) -> ()
                    n2348 = local write "data file error"(w3910) -> ()
                  }
                }
              }
              frame #8 {
                # "LAB05-1"
                n2349 = case shown="True" w3921 {
                  tunnel: w3923 -> [_ w3936]
                  tunnel: w3920 -> [_ w3933]
                  tunnel: w3922 -> [_ w3932]
                  frame False {
                  }
                  frame True {
                    n2350 = local read "TEMP START LAB05-1"() -> (w3938:cluster{"TL":dbl, "TN":dbl})
                    n2351 = local read "FAIL LAB05-1"() -> (w3929:cluster{"LO":dbl, "HI":dbl})
                    n2352 = local read "TDMS LAB05-1"() -> (w3937:refnum<k34>)
                    n2353 = local read "SET LAB05-1"() -> (w3934:T5)
                    n2354 = local read "DISP LAB05-1"() -> (w3935:T4)
                    n2355 = local read "SIG LAB05-1"() -> (w3939:T2)
                    n2356 = local read "RESULT LAB05-1"() -> (w3926:bool)
                    n2357 = Bundle("FAIL LAB05-1"=w3929, "SIG LAB05-1"=w3939, "TEMP START LAB05-1"=w3938, "DISP LAB05-1"=w3935, "SET LAB05-1"=w3934, "TDMS LAB05-1"=w3937) -> (w3924:T34)  [unwired: 1 in]
                    n2358 = call "sub vi - cycle&temp fail v6.vi"("Amps Lo?"=w3936, "Input Cluster"=w3924, "SELECT"=w3933, "Amps Hi?"=w3932, "Result In"=w3926) -> ("(FAIL) out"=w3928:cluster{"FAIL LO":dbl, "FAIL HI":dbl}, "(DISP) out"=w3931:T4, "T-RISE"=w3925:cluster{"T-RISE (L)":dbl, "T-RISE (N)":dbl}, "Result Out"=w3927:bool, "file error"=w3930:errorcluster)  [unwired: 10 in]
                    n2359 = local write "TEMP RISE LAB05-1"(w3925) -> ()
                    n2360 = local write "FAIL LAB05-1"(w3928) -> ()
                    n2361 = local write "DISP LAB05-1"(w3931) -> ()
                    n2362 = local write "RESULT LAB05-1"(w3927) -> ()
                    n2363 = local write "data file error"(w3930) -> ()
                  }
                }
              }
              frame #9 {
                # "LAB05-2"
                n2364 = case shown="True" w3941 {
                  tunnel: w3943 -> [_ w3956]
                  tunnel: w3940 -> [_ w3953]
                  tunnel: w3942 -> [_ w3952]
                  frame False {
                  }
                  frame True {
                    n2365 = local read "TEMP START LAB05-2"() -> (w3958:cluster{"TL":dbl, "TN":dbl})
                    n2366 = local read "FAIL LAB05-2"() -> (w3949:cluster{"LO":dbl, "HI":dbl})
                    n2367 = local read "TDMS LAB05-2"() -> (w3957:refnum<k34>)
                    n2368 = local read "SET LAB05-2"() -> (w3954:T5)
                    n2369 = local read "DISP LAB05-2"() -> (w3955:T4)
                    n2370 = local read "SIG LAB05-2"() -> (w3959:T2)
                    n2371 = local read "RESULT LAB05-2"() -> (w3946:bool)
                    n2372 = Bundle("FAIL LAB05-2"=w3949, "SIG LAB05-2"=w3959, "TEMP START LAB05-2"=w3958, "DISP LAB05-2"=w3955, "SET LAB05-2"=w3954, "TDMS LAB05-2"=w3957) -> (w3944:T35)  [unwired: 1 in]
                    n2373 = call "sub vi - cycle&temp fail v6.vi"("Amps Lo?"=w3956, "Input Cluster"=w3944, "SELECT"=w3953, "Amps Hi?"=w3952, "Result In"=w3946) -> ("(FAIL) out"=w3948:cluster{"FAIL LO":dbl, "FAIL HI":dbl}, "(DISP) out"=w3951:T4, "T-RISE"=w3945:cluster{"T-RISE (L)":dbl, "T-RISE (N)":dbl}, "Result Out"=w3947:bool, "file error"=w3950:errorcluster)  [unwired: 10 in]
                    n2374 = local write "TEMP RISE LAB05-2"(w3945) -> ()
                    n2375 = local write "FAIL LAB05-2"(w3948) -> ()
                    n2376 = local write "DISP LAB05-2"(w3951) -> ()
                    n2377 = local write "RESULT LAB05-2"(w3947) -> ()
                    n2378 = local write "data file error"(w3950) -> ()
                  }
                }
              }
            }
          }
          frame #15 {
            # "run calibration routine"
            n2379 = local read "CALIBRATE"() -> (w3960:bool)
            n2380 = case shown="True" w3960 {
              frame False {
              }
              frame True {
                n2381 = stacked-sequence {
                  seq-local: [w3961 _ _] -> [_ w3963 _]
                  frame #0 {
                    n2382 = call "CALIBRATION PASSWORD"() -> ("PASSWORD"=w3961:string)  [unwired: 17 in, 2 out]
                  }
                  frame #1 {
                    n2383 = Equal?(x=w3963, y="7777") -> (x = y?=w3962:bool)
                    n2384 = case shown="True" w3962 {
                      frame False {
                      }
                      frame True {
                        n2385 = stacked-sequence {
                          frame #0 {
                            n2386 = call "sub vi - calibration v1.vi"() -> ()  [unwired: 12 in]
                          }
                          frame #1 {
                            n2387 = call "sub vi - get calibration values v1.vi"() -> ("LAB01 (CAL)"=w3969:T7, "LAB02 (CAL)"=w3968:T8, "LAB03 (CAL)"=w3967:T7, "LAB04 (CAL)"=w3966:T7, "calibration file error out"=w3970:errorcluster, "LAB05 (CAL)"=w3965:T7)  [unwired: 10 in]
                            n2388 = local write "calibration file error out"(w3970) -> ()
                            n2389 = local write "CAL LAB04"(w3966) -> ()
                            n2390 = local write "CAL LAB05"(w3965) -> ()
                            n2391 = local write "CAL LAB01"(w3969) -> ()
                            n2392 = local write "CAL LAB02"(w3968) -> ()
                            n2393 = local write "CAL LAB03"(w3967) -> ()
                          }
                        }
                      }
                    }
                  }
                  frame #2 {
                    n2394 = local write "CALIBRATE"(FALSE) -> ()
                  }
                }
              }
            }
          }
          frame #16 {
            # "save certain settings to file"
            n2395 = String To Path(string="c:\\crabtree\\Set Up\\") -> (path=w3973:path)
            n2396 = Build Path(base path=w3973, name or relative path="settings.bin") -> (appended path=w3975:path)
            n2397 = Build Path(base path=w3973, name or relative path="mail.bin") -> (appended path=w3972:path)
            n2398 = Create Folder(path (use dialog)=w3973) -> (error out=w3978:errorcluster)  [unwired: 2 in, 2 out]
            n2399 = call <vilib>:"Clear Errors.vi"("error in (no error)"=w3978) -> ()  [unwired: 6 in, 1 out]
            n2400 = stacked-sequence {
              seq-local: [w3980 _] -> [_ w3993]
              tunnel: w3975 -> [_ w3994]
              tunnel: w3972 -> [_ w3992]
              frame #0 {
                n2401 = local read "C drive data root dir"() -> (w3979:path)
                n2402 = local read "Network Directory"() -> (w3985:path)
                n2403 = local read "SET LAB05-2"() -> (w3984:T5)
                n2404 = local read "SET LAB05-1"() -> (w3983:T5)
                n2405 = local read "SET LAB04-2"() -> (w3982:T5)
                n2406 = local read "SET LAB03-2"() -> (w3986:T5)
                n2407 = local read "SET LAB04-1"() -> (w3981:T5)
                n2408 = local read "SET LAB03-1"() -> (w3987:T5)
                n2409 = local read "SET LAB02-2"() -> (w3988:T5)
                n2410 = local read "SET LAB02-1"() -> (w3989:T5)
                n2411 = local read "SET LAB01-2"() -> (w3990:T5)
                n2412 = local read "SET LAB01-1"() -> (w3991:T5)
                n2413 = Bundle("SET LAB01-1"=w3991, "SET LAB01-2"=w3990, "SET LAB02-1"=w3989, "SET LAB02-2"=w3988, "SET LAB03-1"=w3987, "SET LAB03-2"=w3986, "SET LAB04-1"=w3981, "SET LAB04-2"=w3982, "SET LAB05-1"=w3983, "SET LAB05-2"=w3984, "Network Directory"=w3985, "C drive data root dir"=w3979) -> (w3980:T18)  [unwired: 1 in]
              }
              frame #1 {
                n2414 = event shown="[1] \"SET LAB01-1\", \"SET LAB01-2\", \"SET LAB02-1\", \"SET LAB02-2\", \"SET LAB03-1\", \"SET LAB03-2\", \"SET LAB04-1\", \"SET LAB04-2\", \"SET LAB05-1\", \"SET LAB05-2\", \"Network Directory\", \"C drive data root dir\": Value Change" {
                  selector: _ -> [_ _ _]
                  dyn-events: _ -> [_ _ _]
                  timeout: 10.0 -> [_ _ _]
                  tunnel: w3994 -> [_ w3996 _]
                  tunnel: w3993 -> [_ w3997 _]
                  tunnel: w3992 -> [_ _ w4008]
                  event Timeout {
                    n2415 = event-data() -> ()  [unwired: 1 in, 3 out]
                  }
                  event "SET LAB01-1", "SET LAB01-2", "SET LAB02-1", "SET LAB02-2", "SET LAB03-1", "SET LAB03-2", "SET LAB04-1", "SET LAB04-2", "SET LAB05-1", "SET LAB05-2", "Network Directory", "C drive data root dir": Value Change {
                    n2416 = event-data() -> ()  [unwired: 1 in, 6 out]
                    n2417 = Open/Create/Replace File(file path (use dialog)=w3996, operation (0:open)=T17."replace or create") -> (refnum out=w4002:refnum<file>, error out=w4001:errorcluster)  [unwired: 4 in, 1 out]
                    n2418 = Write to Binary File(file (use dialog)=w4002, data=w3997, error in=w4001) -> (refnum out=w4000:refnum<file>, error out=w3999:errorcluster)  [unwired: 3 in, 1 out]
                    n2419 = Close File(refnum=w4000, error in=w3999) -> (error out=w3998:errorcluster)  [unwired: 1 out]
                    n2420 = local write "data file error"(w3998) -> ()
                  }
                  event "MAIL SETTINGS.OUT SERVER ADDRESS", "MAIL SETTINGS.FROM ACCOUNT", "MAIL SETTINGS.USER NAME", "MAIL SETTINGS.PASSWORD", "Auto Mail Send", "TO (string):": Value Change {
                    n2421 = event-data() -> ()  [unwired: 1 in, 6 out]
                    n2422 = local read "MAIL SETTINGS"() -> (w4007:T6)
                    n2423 = local read "Auto Mail Send"() -> (w4005:bool)
                    n2424 = local read "TO (string):"() -> (w4004:string)
                    n2425 = Open/Create/Replace File(file path (use dialog)=w4008, operation (0:open)=T17."replace or create") -> (refnum out=w4013:refnum<file>, error out=w4012:errorcluster)  [unwired: 4 in, 1 out]
                    n2426 = Bundle("MAIL SETTINGS"=w4007, "Auto Mail Send"=w4005, "TO (string):"=w4004) -> (w4006:T36)  [unwired: 1 in]
                    n2427 = Write to Binary File(file (use dialog)=w4013, data=w4006, error in=w4012) -> (refnum out=w4011:refnum<file>, error out=w4010:errorcluster)  [unwired: 3 in, 1 out]
                    n2428 = Close File(refnum=w4011, error in=w4010) -> (error out=w4009:errorcluster)  [unwired: 1 out]
                    n2429 = local write "data file error"(w4009) -> ()
                  }
                }
              }
            }
          }
          frame #17 {
            # "mail control"
            n2430 = local read "MAIL SETTINGS"() -> (w4030:T6)
            n2431 = local read "Auto Mail Send"() -> (w4016:bool)
            n2432 = Unbundle(w4030) -> ("OUT SERVER ADDRESS"=w4029:string, "FROM ACCOUNT"=w4028:string, "TEST MAIL"=w4027:bool)  [unwired: 4 out]
            n2433 = stacked-sequence {
              tunnel: "TO (string):" -> [_ w4069]
              tunnel: w4030 -> [w4035 w4068]
              tunnel: w4029 -> [w4034 w4067]
              tunnel: w4028 -> [w4033 w4066]
              tunnel: w4027 -> [w4032 _]
              tunnel: w4016 -> [_ w4065]
              tunnel: w4026 -> [_ w4064]
              tunnel: w4025 -> [_ w4063]
              tunnel: w4024 -> [_ w4062]
              tunnel: w4023 -> [_ w4061]
              tunnel: w4022 -> [_ w4060]
              tunnel: w4021 -> [_ w4059]
              tunnel: w4020 -> [_ w4058]
              tunnel: w4019 -> [_ w4057]
              tunnel: w4018 -> [_ w4056]
              tunnel: w4017 -> [_ w4055]
              tunnel: "TO (string):" -> [w4031 _]
              frame #0 {
                # "mail test"
                n2434 = case shown="True" w4032 {
                  tunnel: w4035 -> [_ w4039]
                  tunnel: w4031 -> [_ w4038]
                  tunnel: w4034 -> [_ w4037]
                  tunnel: w4033 -> [_ w4036]
                  frame False {
                  }
                  frame True {
                    n2435 = stacked-sequence {
                      seq-local: [_ _ w4049 _] -> [_ _ _ w4050]
                      tunnel: w4039 -> [w4042 _ _ w4054]
                      tunnel: w4038 -> [_ _ w4047 _]
                      tunnel: w4037 -> [_ _ w4045 _]
                      tunnel: w4036 -> [_ _ w4046 _]
                      frame #0 {
                        n2436 = Bundle(cluster=w4042, "TEST MAIL STATUS"="TEST START") -> (w4040:T6)  [unwired: 6 in]
                        n2437 = local write "MAIL SETTINGS"(w4040) -> ()
                      }
                      frame #1 {
                        n2438 = Wait (ms)(milliseconds to wait=500) -> ()  [unwired: 1 out]
                      }
                      frame #2 {
                        n2439 = call "sub vi - send mail with attach v5.vi"("TO:"=w4047, "subject"="MAIL TEST FROM LAB PANEL", "from"=w4046, "out going server"=w4045, "message"="TEST MESSAGE") -> ("error out"=w4049:errorcluster)  [unwired: 10 in]
                      }
                      frame #3 {
                        n2440 = Bundle(cluster=w4054, "TEST MAIL"=FALSE, "TEST MAIL STATUS"="TEST END", "mail error"=w4050) -> (w4052:T6)  [unwired: 4 in]
                        n2441 = local write "MAIL SETTINGS"(w4052) -> ()
                      }
                    }
                  }
                }
              }
              frame #1 {
                # "mail report"
                n2442 = stacked-sequence {
                  seq-local: [_ w4134 _ _] -> [_ _ _ w4302]
                  seq-local: [_ _ w4215 _] -> [_ _ _ w4292]
                  seq-local: [w4079 _ _ _] -> [_ w4128 _ _]
                  seq-local: [w4078 _ _ _] -> [_ w4127 _ _]
                  seq-local: [w4076 _ _ _] -> [_ w4125 _ _]
                  seq-local: [w4077 _ _ _] -> [_ w4126 _ _]
                  seq-local: [w4075 _ _ _] -> [_ w4124 _ _]
                  seq-local: [w4074 _ _ _] -> [_ w4119 _ _]
                  seq-local: [w4073 _ _ _] -> [_ w4120 _ _]
                  seq-local: [w4072 _ _ _] -> [_ w4121 _ _]
                  seq-local: [w4071 _ _ _] -> [_ w4122 _ _]
                  seq-local: [w4070 _ _ _] -> [_ w4123 _ _]
                  tunnel: w4069 -> [_ _ _ w4303]
                  tunnel: w4068 -> [_ _ _ w4286]
                  tunnel: w4067 -> [_ _ _ w4300]
                  tunnel: w4066 -> [_ _ _ w4299]
                  tunnel: w4065 -> [w4110 _ _ w4294]
                  tunnel: w4064 -> [_ _ w4245 _]
                  tunnel: w4063 -> [_ _ w4242 _]
                  tunnel: w4062 -> [_ _ w4241 _]
                  tunnel: w4061 -> [_ _ w4240 _]
                  tunnel: w4060 -> [_ _ w4239 _]
                  tunnel: w4059 -> [_ _ w4238 _]
                  tunnel: w4058 -> [_ _ w4237 _]
                  tunnel: w4057 -> [_ _ w4236 _]
                  tunnel: w4056 -> [_ _ w4235 _]
                  tunnel: w4055 -> [_ _ w4234 _]
                  frame #0 {
                    n2443 = case shown="False" w4110 {
                      frame False {
                        n2444 = local write "mail control"("") -> ()
                      }
                      frame True {
                      }
                    }
                    n2445 = local read "SET LAB01-1"() -> (w4109:T5)
                    n2446 = local read "SET LAB01-2"() -> (w4108:T5)
                    n2447 = local read "SET LAB02-1"() -> (w4107:T5)
                    n2448 = local read "SET LAB02-2"() -> (w4106:T5)
                    n2449 = local read "SET LAB03-1"() -> (w4105:T5)
                    n2450 = local read "SET LAB04-1"() -> (w4103:T5)
                    n2451 = local read "SET LAB05-1"() -> (w4101:T5)
                    n2452 = local read "SET LAB03-2"() -> (w4104:T5)
                    n2453 = local read "SET LAB04-2"() -> (w4102:T5)
                    n2454 = local read "SET LAB05-2"() -> (w4100:T5)
                    n2455 = Unbundle(w4105) -> ("DESCRIPTION"=w4085:string)  [unwired: 4 out]
                    n2456 = Unbundle(w4104) -> ("DESCRIPTION"=w4084:string)  [unwired: 4 out]
                    n2457 = Unbundle(w4103) -> ("DESCRIPTION"=w4083:string)  [unwired: 4 out]
                    n2458 = Unbundle(w4100) -> ("DESCRIPTION"=w4080:string)  [unwired: 4 out]
                    n2459 = Unbundle(w4106) -> ("DESCRIPTION"=w4086:string)  [unwired: 4 out]
                    n2460 = Unbundle(w4102) -> ("DESCRIPTION"=w4082:string)  [unwired: 4 out]
                    n2461 = Unbundle(w4109) -> ("DESCRIPTION"=w4098:string)  [unwired: 4 out]
                    n2462 = Unbundle(w4107) -> ("DESCRIPTION"=w4087:string)  [unwired: 4 out]
                    n2463 = Unbundle(w4101) -> ("DESCRIPTION"=w4081:string)  [unwired: 4 out]
                    n2464 = Unbundle(w4108) -> ("DESCRIPTION"=w4088:string)  [unwired: 4 out]
                    n2465 = Concatenate Strings("[LAB05-1/", w4080) -> (w4070:string)
                    n2466 = Concatenate Strings("[LAB05-2/", w4081) -> (w4071:string)
                    n2467 = Concatenate Strings("[LAB04-2/", w4082) -> (w4072:string)
                    n2468 = Concatenate Strings("[LAB03-2/", w4084) -> (w4074:string)
                    n2469 = Concatenate Strings("[LAB04-1/", w4083) -> (w4073:string)
                    n2470 = Concatenate Strings("[LAB03-1/", w4085) -> (w4075:string)
                    n2471 = Concatenate Strings("[LAB01-2/", w4088) -> (w4078:string)
                    n2472 = Concatenate Strings("[LAB02-2/", w4086) -> (w4076:string)
                    n2473 = Concatenate Strings("[LAB01-1/", w4098) -> (w4079:string)
                    n2474 = Concatenate Strings("[LAB02-1/", w4087) -> (w4077:string)
                  }
                  frame #1 {
                    w4132 = "/"
                    w4133 = 2.0
                    n2475 = local read "DISP LAB01-2"() -> (w4213:T4)
                    n2476 = local read "DISP LAB01-1"() -> (w4214:T4)
                    n2477 = local read "DISP LAB02-1"() -> (w4212:T4)
                    n2478 = local read "DISP LAB03-2"() -> (w4209:T4)
                    n2479 = local read "DISP LAB02-2"() -> (w4211:T4)
                    n2480 = local read "DISP LAB03-1"() -> (w4210:T4)
                    n2481 = local read "DISP LAB04-2"() -> (w4207:T4)
                    n2482 = local read "DISP LAB04-1"() -> (w4208:T4)
                    n2483 = local read "DISP LAB05-1"() -> (w4206:T4)
                    n2484 = local read "DISP LAB05-2"() -> (w4205:T4)
                    n2485 = Unbundle(w4213) -> ("CYCLE"=w4197:dbl, "MINS"=w4196:dbl, "STATUS"=w4193:string)
                    n2486 = Unbundle(w4214) -> ("CYCLE"=w4202:dbl, "MINS"=w4201:dbl, "STATUS"=w4198:string)
                    n2487 = Unbundle(w4212) -> ("CYCLE"=w4190:dbl, "MINS"=w4189:dbl, "STATUS"=w4188:string)
                    n2488 = Unbundle(w4209) -> ("CYCLE"=w4177:dbl, "MINS"=w4176:dbl, "STATUS"=w4173:string)
                    n2489 = Unbundle(w4210) -> ("CYCLE"=w4182:dbl, "MINS"=w4181:dbl, "STATUS"=w4178:string)
                    n2490 = Unbundle(w4211) -> ("CYCLE"=w4187:dbl, "MINS"=w4186:dbl, "STATUS"=w4183:string)
                    n2491 = Unbundle(w4208) -> ("CYCLE"=w4172:dbl, "MINS"=w4171:dbl, "STATUS"=w4168:string)
                    n2492 = Unbundle(w4207) -> ("CYCLE"=w4167:dbl, "MINS"=w4166:dbl, "STATUS"=w4163:string)
                    n2493 = Unbundle(w4206) -> ("CYCLE"=w4162:dbl, "MINS"=w4161:dbl, "STATUS"=w4158:string)
                    n2494 = Unbundle(w4205) -> ("CYCLE"=w4204:dbl, "MINS"=w4203:dbl, "STATUS"=w4155:string)
                    n2495 = Number To Decimal String(number=w4190) -> (decimal integer string=w4192:string)  [unwired: 1 in]
                    n2496 = Number To Decimal String(number=w4187) -> (decimal integer string=w4185:string)  [unwired: 1 in]
                    n2497 = Number To Decimal String(number=w4182) -> (decimal integer string=w4180:string)  [unwired: 1 in]
                    n2498 = Number To Decimal String(number=w4197) -> (decimal integer string=w4195:string)  [unwired: 1 in]
                    n2499 = Number To Decimal String(number=w4177) -> (decimal integer string=w4175:string)  [unwired: 1 in]
                    n2500 = Number To Decimal String(number=w4202) -> (decimal integer string=w4200:string)  [unwired: 1 in]
                    n2501 = Number To Decimal String(number=w4204) -> (decimal integer string=w4157:string)  [unwired: 1 in]
                    n2502 = Number To Decimal String(number=w4172) -> (decimal integer string=w4170:string)  [unwired: 1 in]
                    n2503 = Number To Decimal String(number=w4167) -> (decimal integer string=w4165:string)  [unwired: 1 in]
                    n2504 = Number To Decimal String(number=w4162) -> (decimal integer string=w4160:string)  [unwired: 1 in]
                    n2505 = Number To Fractional String(number=w4189, precision (6)=w4133) -> (F-format string=w4191:string)  [unwired: 2 in]
                    n2506 = Number To Fractional String(number=w4176, precision (6)=w4133) -> (F-format string=w4174:string)  [unwired: 2 in]
                    n2507 = Number To Fractional String(number=w4186, precision (6)=w4133) -> (F-format string=w4184:string)  [unwired: 2 in]
                    n2508 = Number To Fractional String(number=w4181, precision (6)=w4133) -> (F-format string=w4179:string)  [unwired: 2 in]
                    n2509 = Number To Fractional String(number=w4166, precision (6)=w4133) -> (F-format string=w4164:string)  [unwired: 2 in]
                    n2510 = Number To Fractional String(number=w4171, precision (6)=w4133) -> (F-format string=w4169:string)  [unwired: 2 in]
                    n2511 = Number To Fractional String(number=w4196, precision (6)=w4133) -> (F-format string=w4194:string)  [unwired: 2 in]
                    n2512 = Number To Fractional String(number=w4161, precision (6)=w4133) -> (F-format string=w4159:string)  [unwired: 2 in]
                    n2513 = Number To Fractional String(number=w4201, precision (6)=w4133) -> (F-format string=w4199:string)  [unwired: 2 in]
                    n2514 = Number To Fractional String(number=w4203, precision (6)=w4133) -> (F-format string=w4156:string)  [unwired: 2 in]
                    n2515 = Concatenate Strings(w4132, w4175, w4132, w4174, w4132, w4173) -> (w4149:string)
                    n2516 = Concatenate Strings(w4132, w4170, w4132, w4169, w4132, w4168) -> (w4148:string)
                    n2517 = Concatenate Strings(w4132, w4165, w4132, w4164, w4132, w4163) -> (w4147:string)
                    n2518 = Concatenate Strings(w4132, w4160, w4132, w4159, w4132, w4158) -> (w4146:string)
                    n2519 = Concatenate Strings(w4132, w4157, w4132, w4156, w4132, w4155) -> (w4145:string)
                    n2520 = Concatenate Strings(w4132, w4200, w4132, w4199, w4132, w4198) -> (w4154:string)
                    n2521 = Concatenate Strings(w4132, w4180, w4132, w4179, w4132, w4178) -> (w4150:string)
                    n2522 = Concatenate Strings(w4132, w4195, w4132, w4194, w4132, w4193) -> (w4153:string)
                    n2523 = Concatenate Strings(w4132, w4192, w4132, w4191, w4132, w4188) -> (w4152:string)
                    n2524 = Concatenate Strings(w4132, w4185, w4132, w4184, w4132, w4183) -> (w4151:string)
                    n2525 = Concatenate Strings("]", "\r") -> (w4129:string)
                    n2526 = Concatenate Strings(w4124, w4150, w4129) -> (w4140:string)
                    n2527 = Concatenate Strings(w4126, w4152, w4129) -> (w4142:string)
                    n2528 = Concatenate Strings(w4125, w4151, w4129) -> (w4141:string)
                    n2529 = Concatenate Strings(w4121, w4147, w4129) -> (w4137:string)
                    n2530 = Concatenate Strings(w4122, w4146, w4129) -> (w4138:string)
                    n2531 = Concatenate Strings(w4120, w4148, w4129) -> (w4136:string)
                    n2532 = Concatenate Strings(w4119, w4149, w4129) -> (w4135:string)
                    n2533 = Concatenate Strings(w4123, w4145, w4129) -> (w4139:string)
                    n2534 = Concatenate Strings(w4127, w4153, w4129) -> (w4143:string)
                    n2535 = Concatenate Strings(w4128, w4154, w4129) -> (w4144:string)
                    n2536 = Concatenate Strings(w4144, w4143, w4142, w4141, w4140, w4135, w4136, w4137, w4138, w4139) -> (w4112:string)
                    n2537 = Concatenate Strings("[PANEL/", "DESC/", "CYCLES/", "MINS/", "STATUS]", "\r", w4112) -> (w4134:string)
                    "MAIL REPORT" <- w4134
                  }
                  frame #2 {
                    w4243 = "END"
                    n2538 = local read "mail control"() -> (w4244:string)
                    n2539 = case shown="False" w4239 {
                      tunnel: w4244 -> [w4268 _]
                      tunnel: w4243 -> [w4267 _]
                      tunnel: [w4266 FALSE] -> w4229
                      frame False {
                        n2540 = Equal?(x=w4268, y=w4267) -> (x = y?=w4266:bool)
                      }
                      frame True {
                      }
                    }
                    n2541 = case shown="False" w4245 {
                      tunnel: w4244 -> [w4284 _]
                      tunnel: w4243 -> [w4283 _]
                      tunnel: [w4282 FALSE] -> w4233
                      frame False {
                        n2542 = Equal?(x=w4284, y=w4283) -> (x = y?=w4282:bool)
                      }
                      frame True {
                      }
                    }
                    n2543 = case shown="False" w4242 {
                      tunnel: w4244 -> [w4280 _]
                      tunnel: w4243 -> [w4279 _]
                      tunnel: [w4278 FALSE] -> w4232
                      frame False {
                        n2544 = Equal?(x=w4280, y=w4279) -> (x = y?=w4278:bool)
                      }
                      frame True {
                      }
                    }
                    n2545 = case shown="False" w4240 {
                      tunnel: w4244 -> [w4272 _]
                      tunnel: w4243 -> [w4271 _]
                      tunnel: [w4270 FALSE] -> w4230
                      frame False {
                        n2546 = Equal?(x=w4272, y=w4271) -> (x = y?=w4270:bool)
                      }
                      frame True {
                      }
                    }
                    n2547 = case shown="False" w4241 {
                      tunnel: w4244 -> [w4276 _]
                      tunnel: w4243 -> [w4275 _]
                      tunnel: [w4274 FALSE] -> w4231
                      frame False {
                        n2548 = Equal?(x=w4276, y=w4275) -> (x = y?=w4274:bool)
                      }
                      frame True {
                      }
                    }
                    n2549 = Or(x=w4231, y=w4230) -> (x .or. y?=w4222:bool)
                    n2550 = Or(x=w4233, y=w4232) -> (x .or. y?=w4223:bool)
                    n2551 = Or(x=w4223, y=w4222) -> (x .or. y?=w4218:bool)
                    n2552 = case shown="False" w4235 {
                      tunnel: w4244 -> [w4252 _]
                      tunnel: w4243 -> [w4251 _]
                      tunnel: [w4250 FALSE] -> w4224
                      frame False {
                        n2553 = Equal?(x=w4252, y=w4251) -> (x = y?=w4250:bool)
                      }
                      frame True {
                      }
                    }
                    n2554 = case shown="False" w4234 {
                      tunnel: w4244 -> [w4248 _]
                      tunnel: w4243 -> [w4247 _]
                      tunnel: [w4246 FALSE] -> w4228
                      frame False {
                        n2555 = Equal?(x=w4248, y=w4247) -> (x = y?=w4246:bool)
                      }
                      frame True {
                      }
                    }
                    n2556 = case shown="False" w4236 {
                      tunnel: w4244 -> [w4256 _]
                      tunnel: w4243 -> [w4255 _]
                      tunnel: [w4254 FALSE] -> w4225
                      frame False {
                        n2557 = Equal?(x=w4256, y=w4255) -> (x = y?=w4254:bool)
                      }
                      frame True {
                      }
                    }
                    n2558 = case shown="False" w4238 {
                      tunnel: w4244 -> [w4264 _]
                      tunnel: w4243 -> [w4263 _]
                      tunnel: [w4262 FALSE] -> w4227
                      frame False {
                        n2559 = Equal?(x=w4264, y=w4263) -> (x = y?=w4262:bool)
                      }
                      frame True {
                      }
                    }
                    n2560 = case shown="False" w4237 {
                      tunnel: w4244 -> [w4260 _]
                      tunnel: w4243 -> [w4259 _]
                      tunnel: [w4258 FALSE] -> w4226
                      frame False {
                        n2561 = Equal?(x=w4260, y=w4259) -> (x = y?=w4258:bool)
                      }
                      frame True {
                      }
                    }
                    n2562 = Or(x=w4227, y=w4226) -> (x .or. y?=w4221:bool)
                    n2563 = Or(x=w4225, y=w4224) -> (x .or. y?=w4220:bool)
                    n2564 = Or(x=w4228, y=w4229) -> (x .or. y?=w4216:bool)
                    n2565 = Or(x=w4221, y=w4220) -> (x .or. y?=w4219:bool)
                    n2566 = Or(x=w4218, y=w4219) -> (x .or. y?=w4217:bool)
                    n2567 = Or(x=w4217, y=w4216) -> (x .or. y?=w4215:bool)
                  }
                  frame #3 {
                    n2568 = local read "on loops"() -> (w4298:dbl)
                    n2569 = local read "jig cycle"() -> (w4295:dbl)
                    n2570 = local read "Send Mail Now"() -> (w4289:bool)
                    n2571 = Add(x=w4298, y=3.0) -> (x+y=w4296:dbl)
                    n2572 = Equal?(x=w4295, y=w4296) -> (x = y?=w4290:bool)
                    n2573 = And(x=w4290, y=w4289) -> (x .and. y?=w4288:bool)
                    n2574 = And(x=w4294, y=w4290) -> (x .and. y?=w4293:bool)
                    n2575 = And(x=w4293, y=w4292) -> (x .and. y?=w4291:bool)
                    n2576 = Or(x=w4291, y=w4288) -> (x .or. y?=w4287:bool)
                    n2577 = case shown="True" w4287 {
                      tunnel: w4303 -> [_ w4309]
                      tunnel: w4302 -> [_ w4308]
                      tunnel: "Lab Panel Test Status" -> [_ w4307]
                      tunnel: w4300 -> [_ w4306]
                      tunnel: w4299 -> [_ w4305]
                      tunnel: w4286 -> [_ w4304]
                      frame False {
                      }
                      frame True {
                        n2578 = stacked-sequence {
                          tunnel: w4309 -> [w4317 _]
                          tunnel: w4308 -> [w4316 _]
                          tunnel: w4307 -> [w4315 _]
                          tunnel: w4306 -> [w4314 _]
                          tunnel: w4305 -> [w4313 _]
                          tunnel: w4304 -> [w4312 _]
                          frame #0 {
                            n2579 = call "sub vi - send mail with attach v5.vi"("TO:"=w4317, "subject"=w4315, "from"=w4313, "out going server"=w4314, "message"=w4316) -> ("error out"=w4311:errorcluster)  [unwired: 10 in]
                            n2580 = Bundle(cluster=w4312, "mail error"=w4311) -> (w4310:T6)  [unwired: 6 in]
                            n2581 = local write "MAIL SETTINGS"(w4310) -> ()
                          }
                          frame #1 {
                            n2582 = local write "mail control"("") -> ()
                            n2583 = local write "Send Mail Now"(FALSE) -> ()
                          }
                        }
                      }
                    }
                  }
                }
              }
            }
          }
        }
        n2584 = node-c288() -> ()  [unwired: 1 in, 1 out]
        "loops" <- w161
        "stop2" <- "stop"
      }
      n2585 = node-c288(w138) -> ()  [unwired: 1 out]
    }
  }
